vi "Dresden New Recipe(in).vi"() -> (0 "OKTO":bool, 1 "Data":string[][](array[string]))   [LabVIEW 2009]
uses:
  kernel32.dll
panel:
  out "Calculated_total_length_cmb":dbl
  out "Calculated_total_length_rf":dbl
  in  "Single_RF_power_power_tab":enum32{"Page 1", "Page 2"}(tab)
  in  "R Single RF  Step1 Coating Power":dbl caption="Watt"
  in  "R Single RF Step1 Coating Power Active":bool
  in  "R Single RF Step2 Coating Power":dbl caption="Watt"
  in  "R Single RF Step2 Coating Power Active":bool
  in  "R Single RF Step3 Coating Power":dbl caption="Watt"
  in  "R Single RF Step3 Coating Power Active":bool
  in  "R Single RF Step4 Coating Power":dbl caption="Watt"
  in  "R Single RF Step4 Coating Power Active":bool
  in  "R Single RF Step5 Coating Power":dbl caption="Watt"
  in  "R Single RF Step5 Coating Power Active":bool
  in  "R Single RF Interval length":dbl
  in  "R Single RF Interval length2":dbl
  in  "R Single RF Interval length3":dbl
  in  "R Single RF Interval length4":dbl
  in  "R Single RF Interval length5":dbl
  in  "R Single RF Step6 Coating Power":dbl caption="Watt"
  in  "R Single RF Step6 Coating Power Active":bool
  in  "R Single RF Interval length6":dbl
  in  "R Single RF Step7 Coating Power":dbl caption="Watt"
  in  "R Single RF Step7 Coating Power Active":bool
  in  "R Single RF Interval length7":dbl
  in  "R Single RF Step8 Coating Power":dbl caption="Watt"
  in  "R Single RF Step8 Coating Power Active":bool
  in  "R Single RF Interval length8":dbl
  in  "R Single RF Step9 Coating Power":dbl caption="Watt"
  in  "R Single RF Step9 Coating Power Active":bool
  in  "R Single RF Interval length9":dbl
  in  "R Single RF Step10 Coating Power":dbl caption="Watt"
  in  "R Single RF Step10 Coating Power Active":bool
  in  "R Single RF Interval length10":dbl
  in  "Single_DC_power_power_tab":enum32{"Page 1", "Page 2"}(tab)
  in  "R Single DC Interval length1":dbl
  in  "R Single DC Step1 Coating Power Active":bool
  in  "R Single DC Step1 Coating Power":dbl caption="Watt"
  in  "R Single DC Interval length2":dbl
  in  "R Single DC Step2 Coating Power Active":bool
  in  "R Single DC Step2 Coating Power":dbl caption="Watt"
  in  "R Single DC Step3 Coating Power Active":bool
  in  "R Single DC Step3 Coating Power":dbl caption="Watt"
  in  "R Single DC Interval length3":dbl
  in  "R Single DC Step4 Coating Power Active":bool
  in  "R Single DC Step4 Coating Power":dbl caption="Watt"
  in  "R Single DC Interval length4":dbl
  in  "R Single DC Step5 Coating Power Active":bool
  in  "R Single DC Step5 Coating Power":dbl caption="Watt"
  in  "R Single DC Interval length5":dbl
  in  "R Single DC Step6 Coating Power Active":bool
  in  "R Single DC Step6 Coating Power":dbl caption="Watt"
  in  "R Single DC Interval length6":dbl
  in  "R Single DC Step7 Coating Power Active":bool
  in  "R Single DC Step7 Coating Power":dbl caption="Watt"
  in  "R Single DC Interval length7":dbl
  in  "R Single DC Step8 Coating Power Active":bool
  in  "R Single DC Step8 Coating Power":dbl caption="Watt"
  in  "R Single DC Interval length8":dbl
  in  "R Single DC Step9 Coating Power Active":bool
  in  "R Single DC Step9 Coating Power":dbl caption="Watt"
  in  "R Single DC Interval length9":dbl
  in  "R Single DC Step10 Coating Power Active":bool
  in  "R Single DC Step10 Coating Power":dbl caption="Watt"
  in  "R Single DC Interval length10":dbl
  in  "Multilayer_power_tab":enum32{"Page 1", "Page 2"}(tab)
  in  "R Cmb Interval length 1":dbl
  in  "R Cmb Ch3 Step1 Coating Power":dbl caption="Watt"
  in  "R Cmb Step1 Coating Power Active":bool
  in  "R Cmb Ch2 Step1 Coating Power":dbl caption="Watt"
  in  "R Cmb Interval length 2":dbl
  in  "R Cmb Ch3 Step2 Coating Power":dbl caption="Watt"
  in  "R Cmb Step2 Coating Power Active":bool
  in  "R Cmb Ch2 Step2 Coating Power":dbl caption="Watt"
  in  "R Cmb Interval length 3":dbl
  in  "R Cmb Ch3 Step3 Coating Power":dbl caption="Watt"
  in  "R Cmb Step3 Coating Power Active":bool
  in  "R Cmb Ch2 Step3 Coating Power":dbl caption="Watt"
  in  "R Cmb Interval length 4":dbl
  in  "R Cmb Ch3 Step4 Coating Power":dbl caption="Watt"
  in  "R Cmb Step4 Coating Power Active":bool
  in  "R Cmb Ch2 Step4 Coating Power":dbl caption="Watt"
  in  "R Cmb Interval length 5":dbl
  in  "R Cmb Ch3 Step5 Coating Power":dbl caption="Watt"
  in  "R Cmb Step5 Coating Power Active":bool
  in  "R Cmb Ch2 Step5 Coating Power":dbl caption="Watt"
  in  "R Cmb Interval length 6":dbl
  in  "R Cmb Ch3 Step6 Coating Power":dbl caption="Watt"
  in  "R Cmb Step6 Coating Power Active":bool
  in  "R Cmb Ch2 Step6 Coating Power":dbl caption="Watt"
  in  "R Cmb Interval length 7":dbl
  in  "R Cmb Ch3 Step7 Coating Power":dbl caption="Watt"
  in  "R Cmb Step7 Coating Power Active":bool
  in  "R Cmb Ch2 Step7 Coating Power":dbl caption="Watt"
  in  "R Cmb Interval length 8":dbl
  in  "R Cmb Ch3 Step8 Coating Power":dbl caption="Watt"
  in  "R Cmb Step8 Coating Power Active":bool
  in  "R Cmb Ch2 Step8 Coating Power":dbl caption="Watt"
  in  "R Cmb Interval length 9":dbl
  in  "R Cmb Ch3 Step9 Coating Power":dbl caption="Watt"
  in  "R Cmb Step9 Coating Power Active":bool
  in  "R Cmb Ch2 Step9 Coating Power":dbl caption="Watt"
  in  "R Cmb Interval length 10":dbl
  in  "R Cmb Ch3 Step10 Coating Power":dbl caption="Watt"
  in  "R Cmb Step10 Coating Power Active":bool
  in  "R Cmb Ch2 Step10 Coating Power":dbl caption="Watt"
  out "error out":errorcluster
  out "Calculated_total_length_dc":dbl
  in  "Diameter":dbl
  out "Lap":dbl
  in  "R General_tab":enum32{"Page 1", "Page 2"}(tab)
  in  "Cancel":bool
  in  "Thickness_Monitor_Active":bool
  in  "Recipe_selection tab":T1(tab)
  in  "R_Simple_Coating Type Selection":T2(radio)
  in  "R_Single_Coating Type Selection_tab":T3(tab)
  in  "R_Single Microwave Time":dbl caption="sec"
  in  "R_Single Microwave Power":dbl=600.0 caption="Watt"
  in  "R Single Pass Number":dbl
  in  "R_Single DC_Material ok":bool
  in  "R_Single DC_Mat_sel":u64(ring) items=["Other", "Ag", "AgBr", "AgCl", "Al", "Al2O3", "As", "Au", "B", "Ba", "Be", "Bi", "Bi2O3", "C (Diamond)", "C (Graphite)", "Ca", "CaF", "Cd", "CdS", "CdSe", "CdTe", "CeF3", "CeO", "Cr", "Cr2O3", "Co", "Cu", "Cu2S (A)", "Cu2S (B)", "CuS", "Dy", "Er", "Fe", "Ga", "GaAs", "Gd", "Ge", "Hf", "HfO2", "Hg", "Ho", "In", "InSb", "In2O3", "Ir", "KCl", "La", "LaF3", "LaO3", "Li", "LiF", "Mg", "MgF2", "MgO", "Mn", "MnS", "Mo", "Na", "NaCl", "NdF3", "Nd2O3", "Ni", "Nb", "Nb2O5", "Pb", "PbS", "Pd", "Pt", "Re", "Rh", "Rb", "S", "Sb", "Sc", "Se", "Si", "SiO", "SiO2", "Sm", "Sn", "Ta", "Ta2O5", "Te", "Tb", "ThF4", "Ti", "TiO2", "TiO", "Tl", "U", "V", "W", "WC", "Y", "Y2O3", "Yb", "Zn", "ZnO", "ZnSe", "ZnS", "Zr", "ZrO2", "Si3N4", "ITO", "PbI2"]
  in  "R Single DC Target material":string
  in  "R_DC_Chamber_selection":enum32{"Chamber II", "Chamber III"}(radio)
  in  "Power_singledc_list_open":bool
  in  "R_Single RF Material ok":bool
  in  "R_Single RF_Mat_sel":u64(ring) items=["Other", "Ag", "AgBr", "AgCl", "Al", "Al2O3", "As", "Au", "B", "Ba", "Be", "Bi", "Bi2O3", "C (Diamond)", "C (Graphite)", "Ca", "CaF", "Cd", "CdS", "CdSe", "CdTe", "CeF3", "CeO", "Cr", "Cr2O3", "Co", "Cu", "Cu2S (A)", "Cu2S (B)", "CuS", "Dy", "Er", "Fe", "Ga", "GaAs", "Gd", "Ge", "Hf", "HfO2", "Hg", "Ho", "In", "InSb", "In2O3", "Ir", "KCl", "La", "LaF3", "LaO3", "Li", "LiF", "Mg", "MgF2", "MgO", "Mn", "MnS", "Mo", "Na", "NaCl", "NdF3", "Nd2O3", "Ni", "Nb", "Nb2O5", "Pb", "PbS", "Pd", "Pt", "Re", "Rh", "Rb", "S", "Sb", "Sc", "Se", "Si", "SiO", "SiO2", "Sm", "Sn", "Ta", "Ta2O5", "Te", "Tb", "ThF4", "Ti", "TiO2", "TiO", "Tl", "U", "V", "W", "WC", "Y", "Y2O3", "Yb", "Zn", "ZnO", "ZnSe", "ZnS", "Zr", "ZrO2", "Si3N4", "ITO", "PbI2"]
  in  "R Single RF Target material":string
  in  "R Single RF Ramp down":bool
  in  "R Single RF Ramp down Time":dbl caption="sec"
  in  "R Single RF Ramp up Time":dbl caption="sec"
  in  "R Single RF Ramp up":bool
  in  "Power_single_rf_list_open":bool
  in  "Power_list_open_multi":bool
  in  "R Cmb Ch3 Material ok":bool
  in  "R Cmb Ch3 Mat_sel":u64(ring) items=["Other", "Ag", "AgBr", "AgCl", "Al", "Al2O3", "As", "Au", "B", "Ba", "Be", "Bi", "Bi2O3", "C (Diamond)", "C (Graphite)", "Ca", "CaF", "Cd", "CdS", "CdSe", "CdTe", "CeF3", "CeO", "Cr", "Cr2O3", "Co", "Cu", "Cu2S (A)", "Cu2S (B)", "CuS", "Dy", "Er", "Fe", "Ga", "GaAs", "Gd", "Ge", "Hf", "HfO2", "Hg", "Ho", "In", "InSb", "In2O3", "Ir", "KCl", "La", "LaF3", "LaO3", "Li", "LiF", "Mg", "MgF2", "MgO", "Mn", "MnS", "Mo", "Na", "NaCl", "NdF3", "Nd2O3", "Ni", "Nb", "Nb2O5", "Pb", "PbS", "Pd", "Pt", "Re", "Rh", "Rb", "S", "Sb", "Sc", "Se", "Si", "SiO", "SiO2", "Sm", "Sn", "Ta", "Ta2O5", "Te", "Tb", "ThF4", "Ti", "TiO2", "TiO", "Tl", "U", "V", "W", "WC", "Y", "Y2O3", "Yb", "Zn", "ZnO", "ZnSe", "ZnS", "Zr", "ZrO2", "Si3N4", "ITO", "PbI2"]
  in  "R Cmb Ch3 Target material":string
  in  "R_Cmb Ch2_Material ok":bool
  in  "R_Cmb Ch2_Mat_sel":u64(ring) items=["Other", "Ag", "AgBr", "AgCl", "Al", "Al2O3", "As", "Au", "B", "Ba", "Be", "Bi", "Bi2O3", "C (Diamond)", "C (Graphite)", "Ca", "CaF", "Cd", "CdS", "CdSe", "CdTe", "CeF3", "CeO", "Cr", "Cr2O3", "Co", "Cu", "Cu2S (A)", "Cu2S (B)", "CuS", "Dy", "Er", "Fe", "Ga", "GaAs", "Gd", "Ge", "Hf", "HfO2", "Hg", "Ho", "In", "InSb", "In2O3", "Ir", "KCl", "La", "LaF3", "LaO3", "Li", "LiF", "Mg", "MgF2", "MgO", "Mn", "MnS", "Mo", "Na", "NaCl", "NdF3", "Nd2O3", "Ni", "Nb", "Nb2O5", "Pb", "PbS", "Pd", "Pt", "Re", "Rh", "Rb", "S", "Sb", "Sc", "Se", "Si", "SiO", "SiO2", "Sm", "Sn", "Ta", "Ta2O5", "Te", "Tb", "ThF4", "Ti", "TiO2", "TiO", "Tl", "U", "V", "W", "WC", "Y", "Y2O3", "Yb", "Zn", "ZnO", "ZnSe", "ZnS", "Zr", "ZrO2", "Si3N4", "ITO", "PbI2"]
  in  "R Cmb Ch2 Target material":string
  in  "R Cmb Number of cycle":dbl
  in  "R_First_stop_selection":enum32{"Chamber II", "Chamber III"}(radio)=enum."Chamber III"
  in  "R_Cmb_Ch2_Web_speed":dbl
  in  "R_Cmb_Ch3_Web_speed":dbl
  in  "Substrate Material":string
  in  "Recipe Name":string
  in  "R_Recipe_type_selection":enum32{"Single Recipe", "Combination Sputter"}(radio)
  in  "R_Web_selection":enum32{"Web", "Other"}(radio)=enum."Other"
  in  "Web_selection_tab":T4(tab)
  in  "R Web thickness":dbl
  in  "R Maximum diameter":dbl format="%.1f"
  in  "R Minimum diameter":dbl=93.0 format="%.1f"
  in  "R Web speed(cm/min)":dbl
  in  "R Tension Value":dbl=7.0
  out "R  Total length":dbl caption="cm" format="%.1f"
  in  "Calculate":bool
  in  "R_Thickness Selection":enum32{"Thickness", "Time"}(radio)
  in  "R_Target Thickness Value":dbl format="%.2f"
  in  "R_Duration":dbl caption="%"
  in  "R Argon Flow sccm":dbl caption="sccm"
  in  "R Z_factor":dbl format="%_3f"
  in  "R Material_density":dbl caption="g/cm3" format="%_3f"
  in  "OK":bool caption="OK2"
  in  "R Toooling_factor":dbl caption="%"
  in  "R Set Pressure mtorr":dbl=0.004 caption="mbar" format="%.1e"
  in  "Tab Control":enum32{"Page 1", "Page 2"}(tab)
  out "Process_flow":string
  in  "Tab Control 2":enum32{"Page 1", "Page 2"}(tab)
  out "Process_flow 2":string
  # "dc max:3000"
  # "rf max:2000"
  # "Steps List"
  # "Power(Watt)"
  # "Interval Length(cm)"
  # "Step 1    :"
  # "cm"
  # "Step 2    :"
  # "cm"
  # "Step 3    :"
  # "cm"
  # "Step 4    :"
  # "cm"
  # "Step 5    :"
  # "cm"
  # "Step 6    :"
  # "cm"
  # "Step 7    :"
  # "cm"
  # "Step 8    :"
  # "cm"
  # "Step 9    :"
  # "cm"
  # "Step 10  :"
  # "cm"
  # "Steps List"
  # "Power(Watt)"
  # "Interval Length(cm)"
  # "Step 1            :"
  # "cm"
  # "Step 2            :"
  # "cm"
  # "Step 3            :"
  # "cm"
  # "Step 4            :"
  # "cm"
  # "Step 5            :"
  # "cm"
  # "Step 6            :"
  # "cm"
  # "cm"
  # "Step 7            :"
  # "cm"
  # "Step 8            :"
  # "cm"
  # "Step 9            :"
  # "cm"
  # "Step 10          :"
  # "Steps List"
  # "CH2-Power(Watt)"
  # "CH3-Power(Watt)"
  # "Interval Length(cm)"
  # "Step 1:"
  # "cm"
  # "Step 2:"
  # "cm"
  # "Step 3:"
  # "cm"
  # "Step 4:"
  # "cm"
  # "Step 5:"
  # "cm"
  # "Step 6:"
  # "cm"
  # "cm"
  # "Step 7:"
  # "cm"
  # "Step 8:"
  # "cm"
  # "Step 9:"
  # "cm"
  # "Step 10:"
  # "Recipe  Selection"
  # "Web  Selection"
  # "Pressure Control Parameters"
  # "Thickness Monitor Parameters"
  # "Material Density       :"
  # "Argon Flow         :"
  # "Z factor                    :"
  # "Set Pressure        :"
  # "Tooling Factor         :"
  # "Single Process Selection"
  # "Power Value     :"
  # "Watt"
  # "Duration           :"
  # "sec"
  # "Pass Number    :"
  # "DCPS Parameters"
  # "Target material          :"
  # "RFPS Parameters"
  # "Target material          :"
  # "Ramp Up Time           :"
  # "Ramp Down Time      :"
  # "DCPS Parameters"
  # "Chamber II"
  # "Chamber III"
  # "Target material         :"
  # "Target material          :"
  # "Web Speed                :"
  # "cm/sec"
  # "Web Speed               :"
  # "cm/sec"
  # "Number of cycle:"
  # "First Stop :"
  # "Roll  Parameters"
  # "Minimum Diameter     :"
  # "mm"
  # "Web Speed              :"
  # "cm / min"
  # "Tension Value         :"
  # "Maximum Diameter     :"
  # "mm"
  # "N"
  # "Web Thickness            :"
  # "µm"
  # "Total Length           :"
  # "Other Parameters"
  # "Thickness Selection         :"
  # "Target Thickness Value   :"
  # "kA"
  # "min"
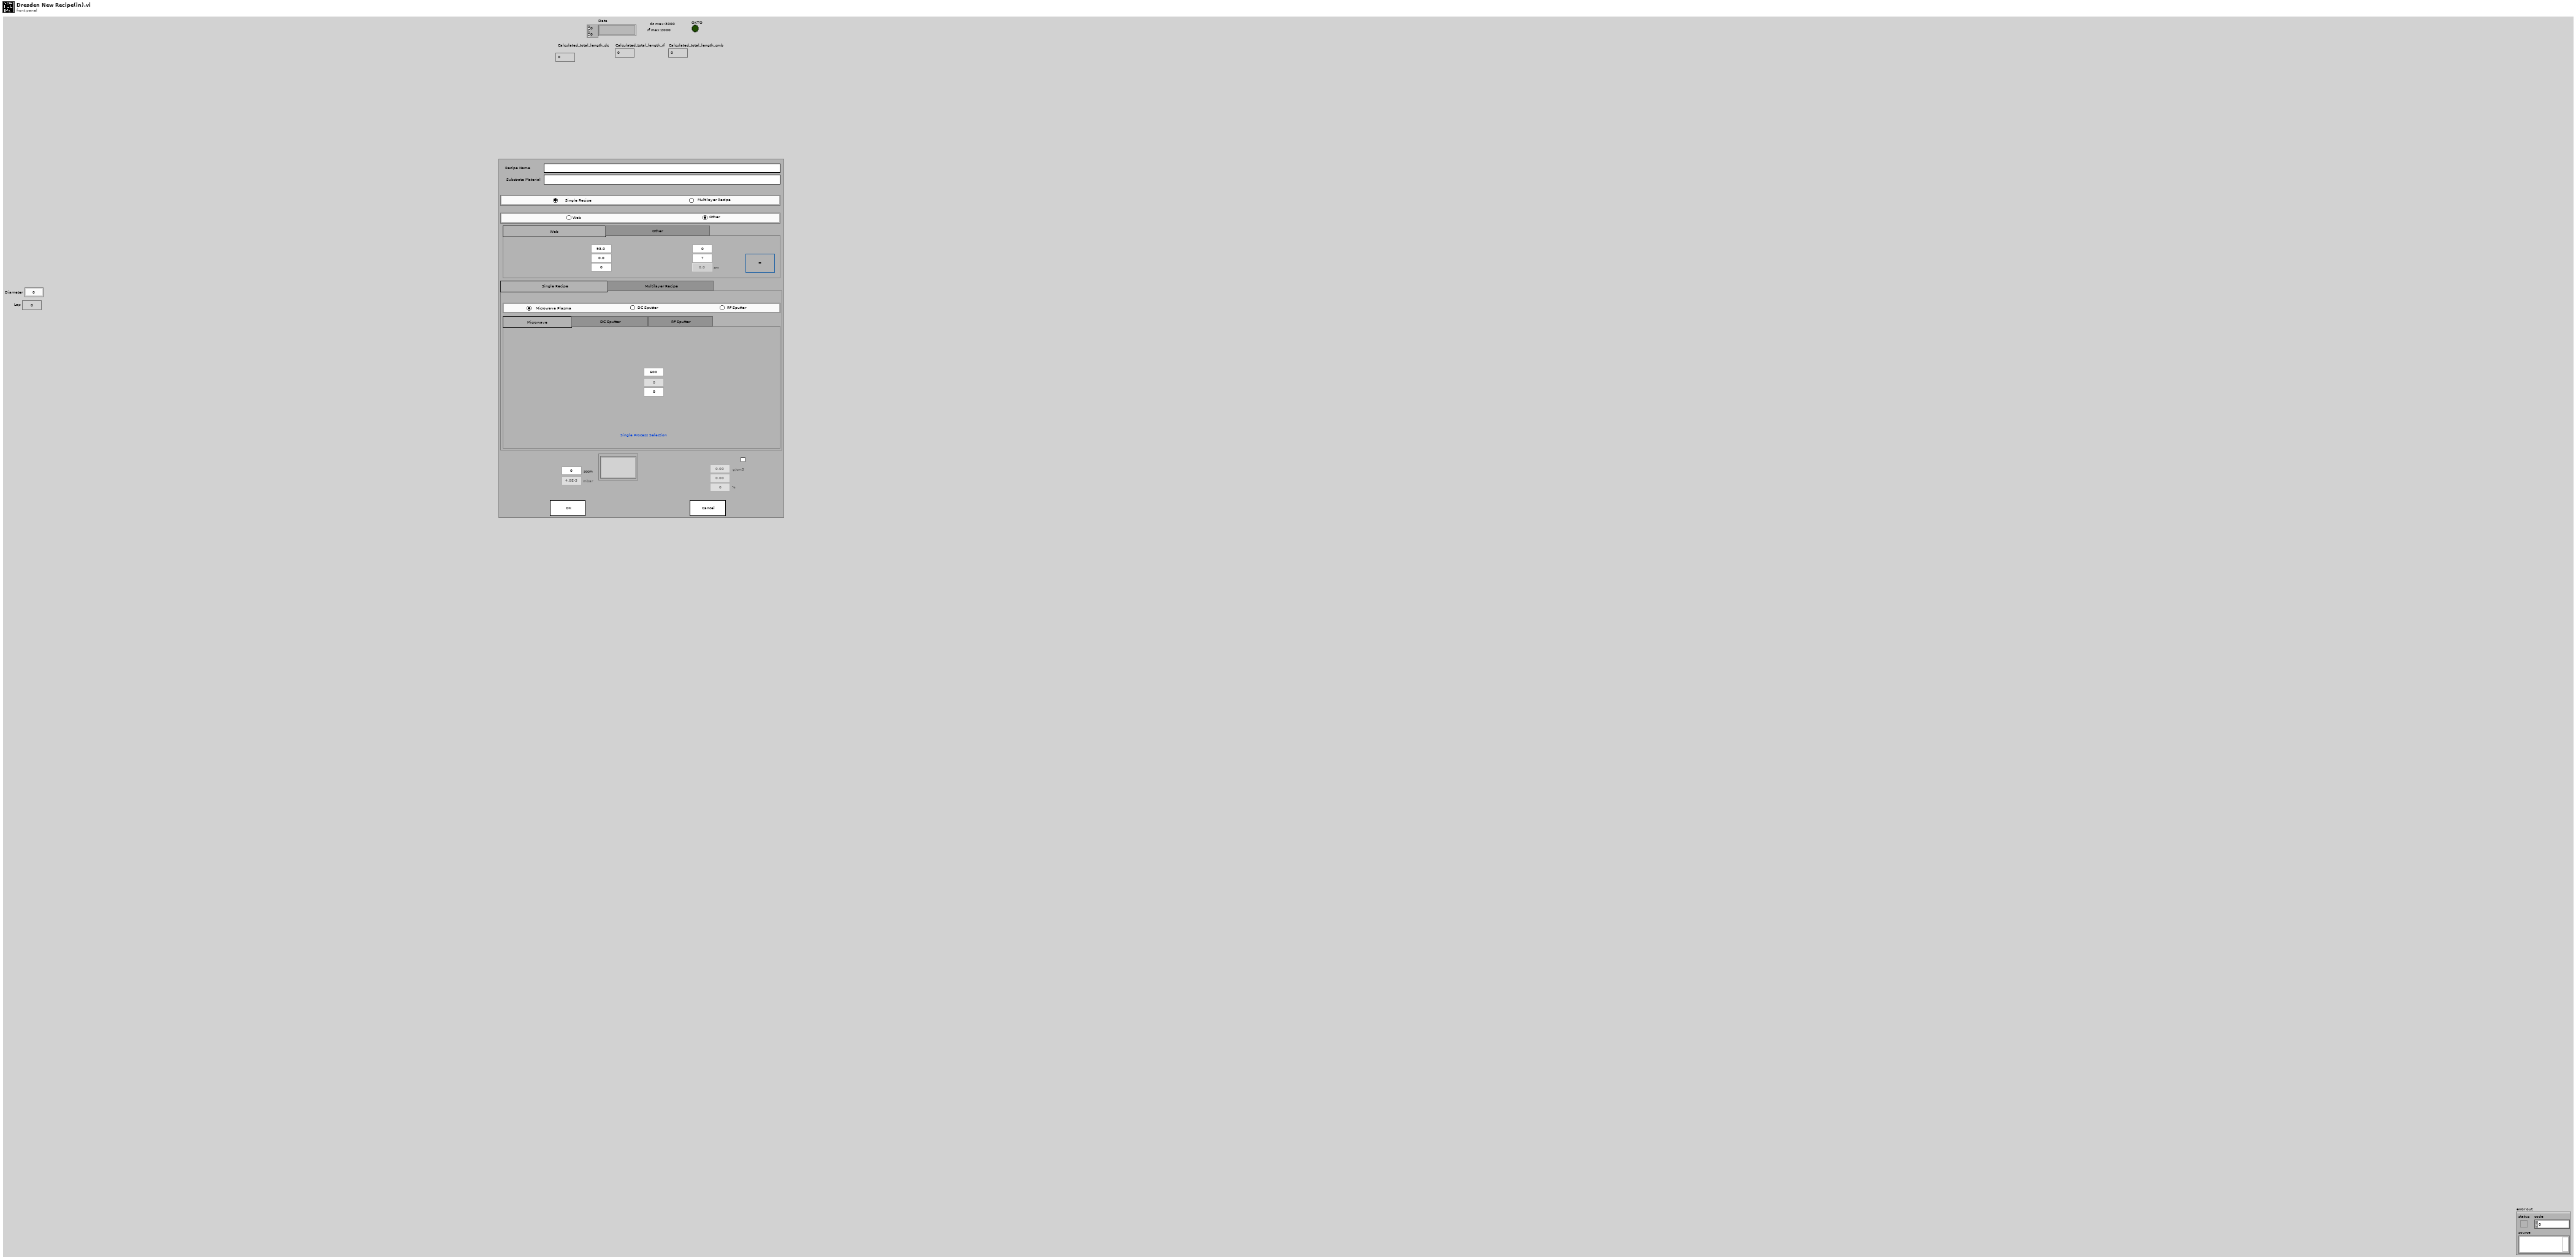
[diagram p1: front panel]
types:
  T1 = enum32{"Single Recipe                                                                         ", "Multilayer Recipe                                                                  "}
  T2 = enum32{"Microwave Plasma", "DC Sputter", "RF Sputter"}
  T3 = enum32{"Microwave                                          ", "DC Sputter                                                 ", "RF Sputter                                       "}
  T4 = enum32{"Web                                                                                    ", "Other                                                                                    "}
  T5 = enum8{"Enabled", "Disabled", "Disabled and Grayed Out"}
  T6 = enum16{"open", "replace", "create", "open or create", "replace or create", "replace or create with confirmation"}
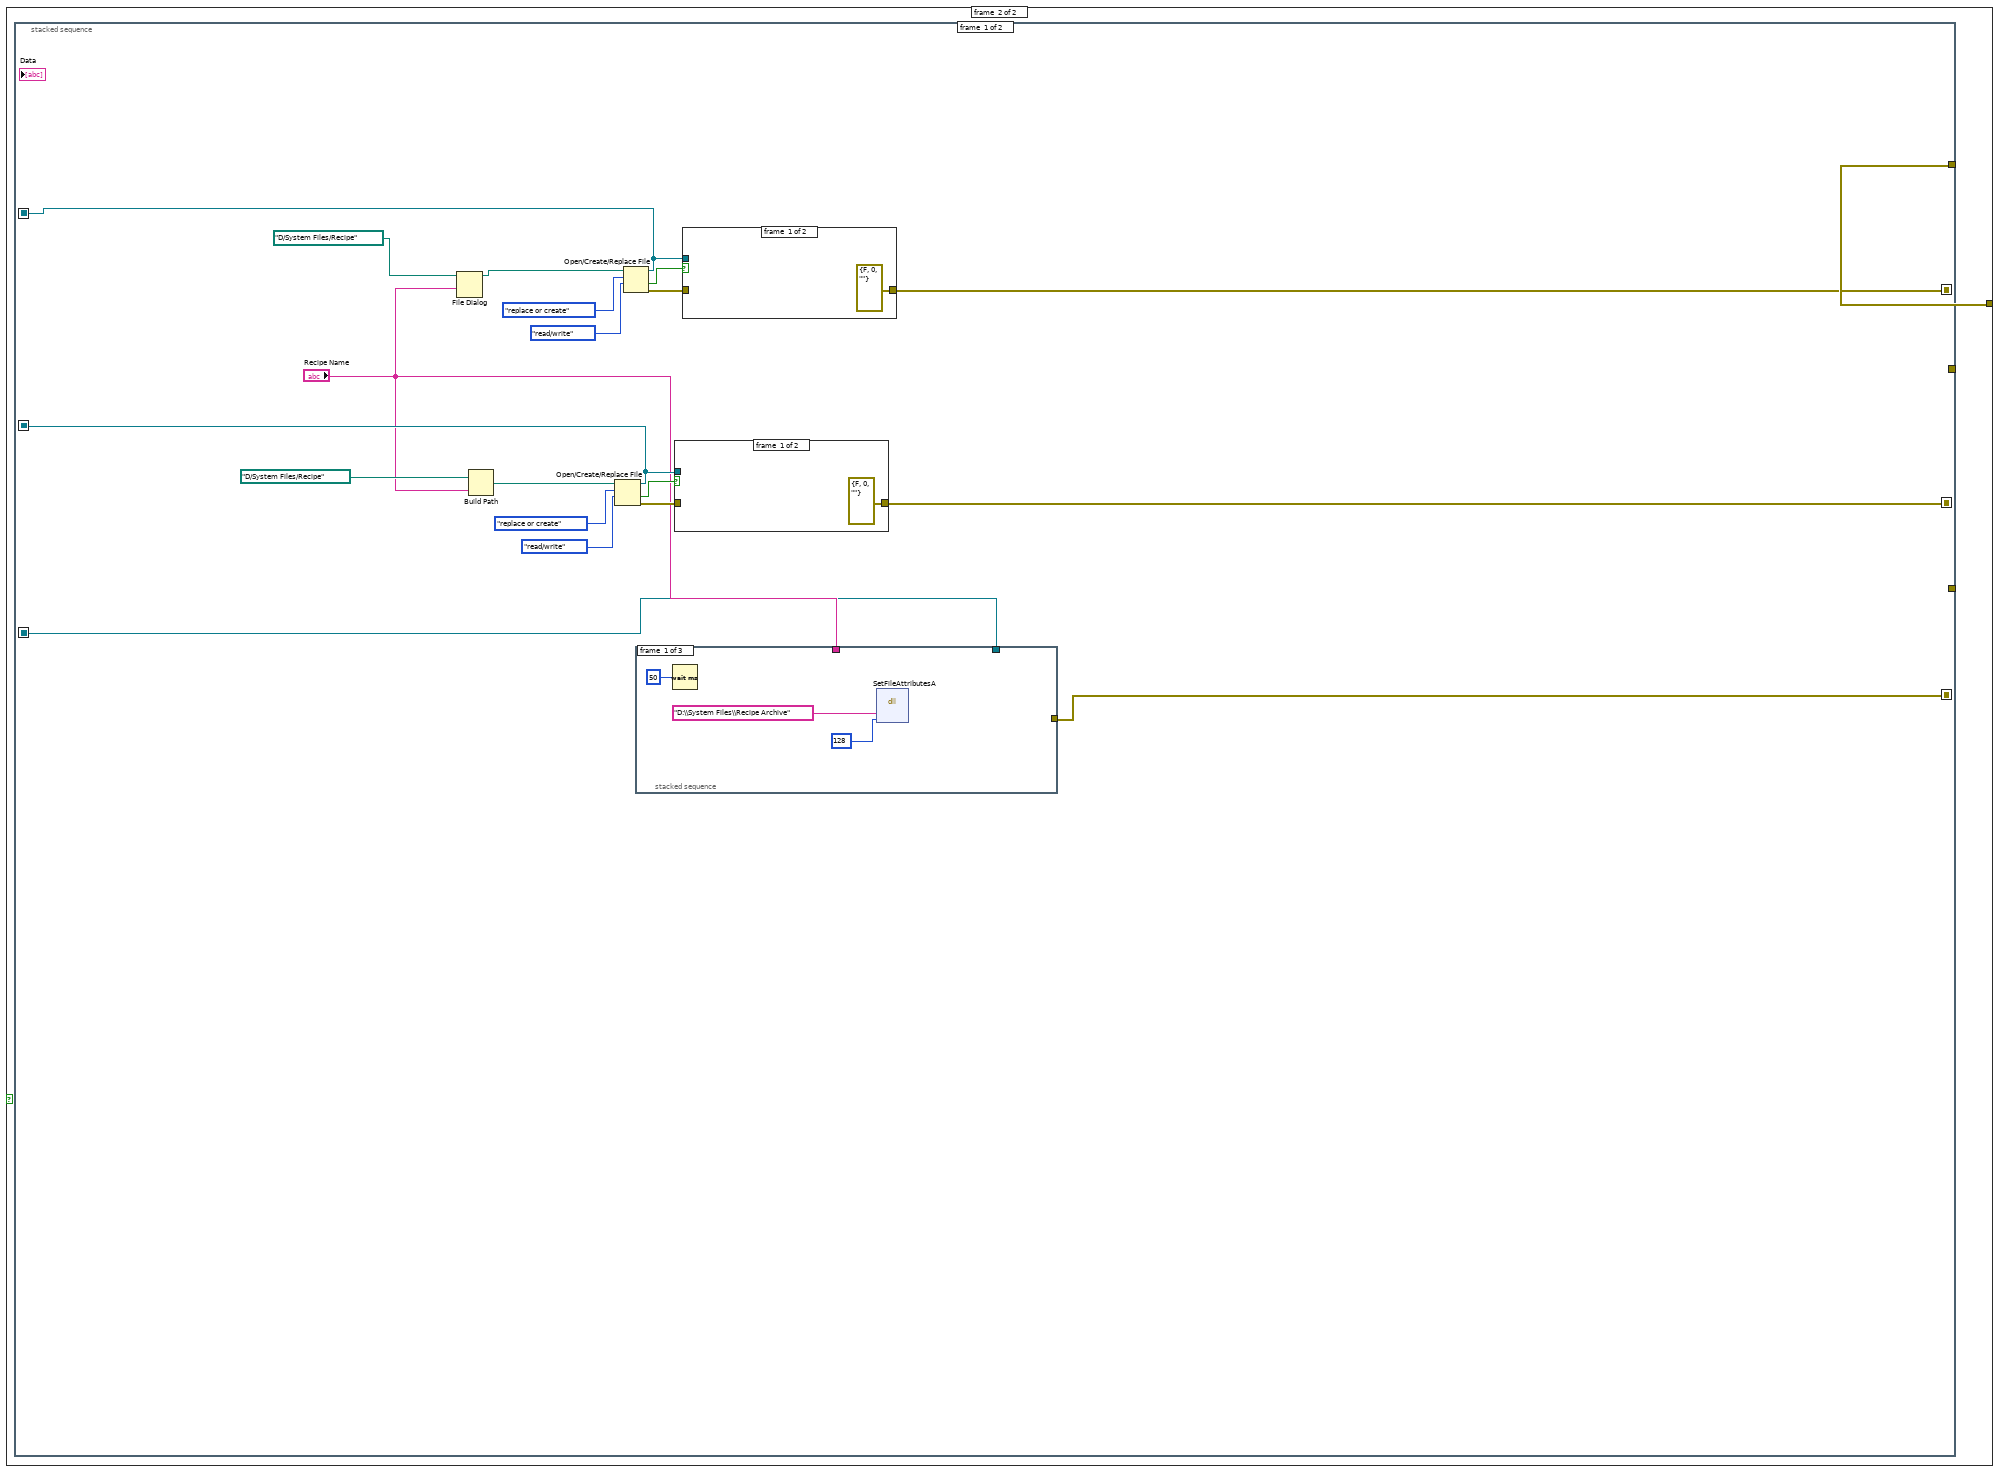
[diagram p2: hidden frame]
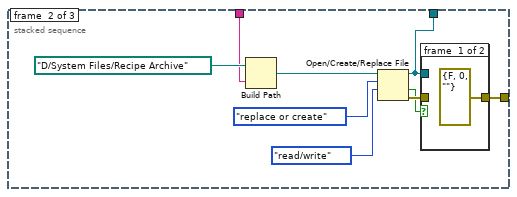
[diagram p3: hidden frame]
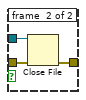
[diagram p4: hidden frame]
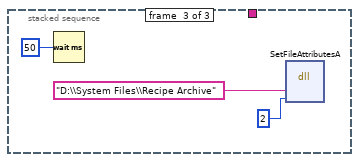
[diagram p5: hidden frame]
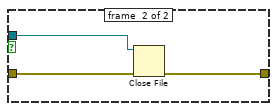
[diagram p6: hidden frame]
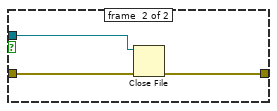
[diagram p7: hidden frame]
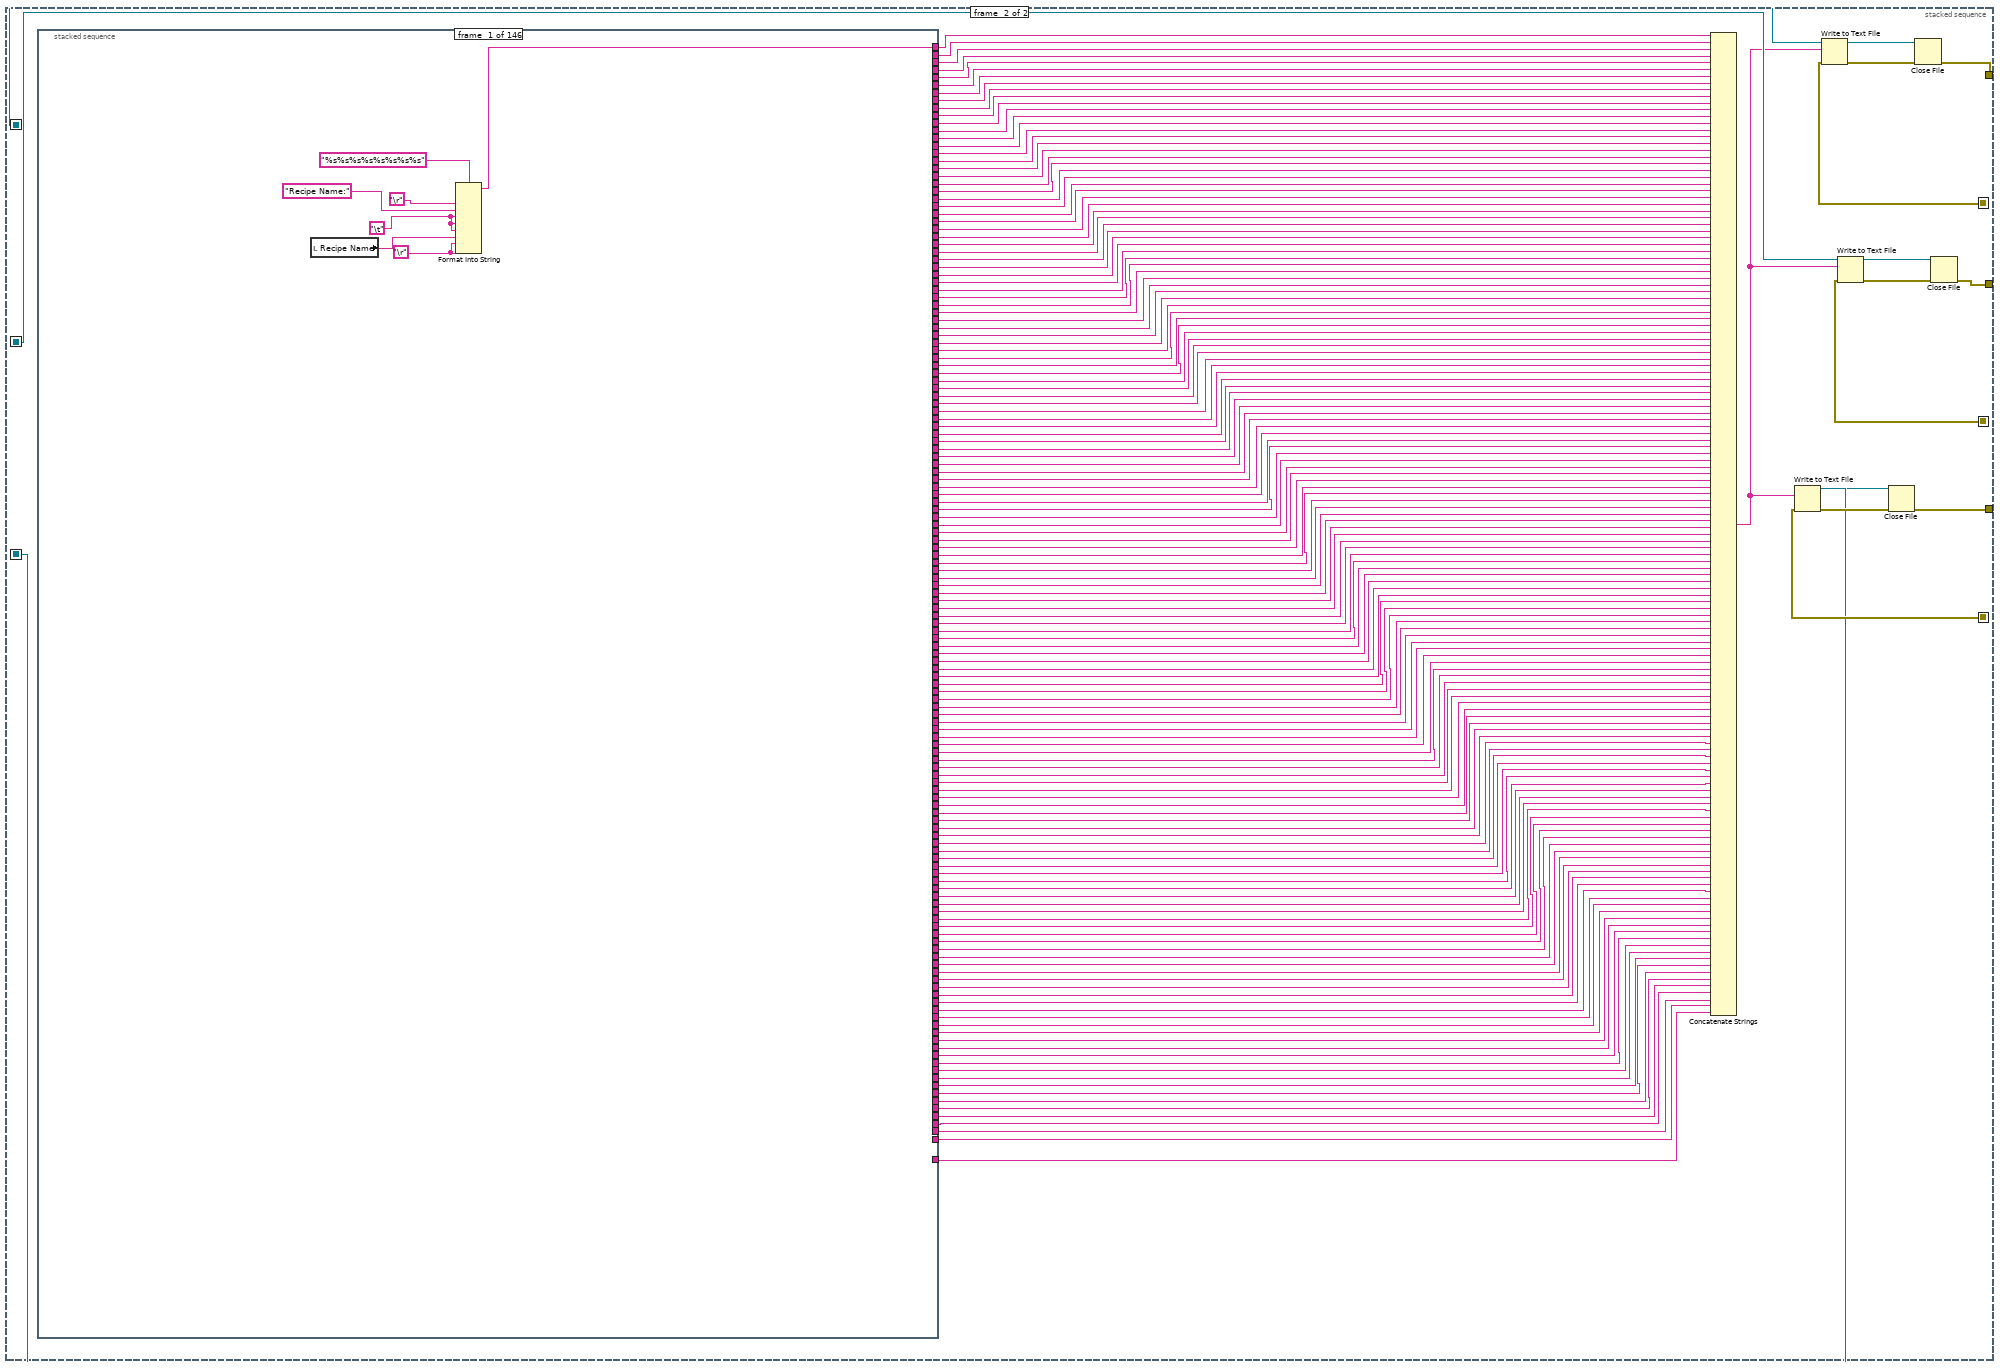
[diagram p8: hidden frame]
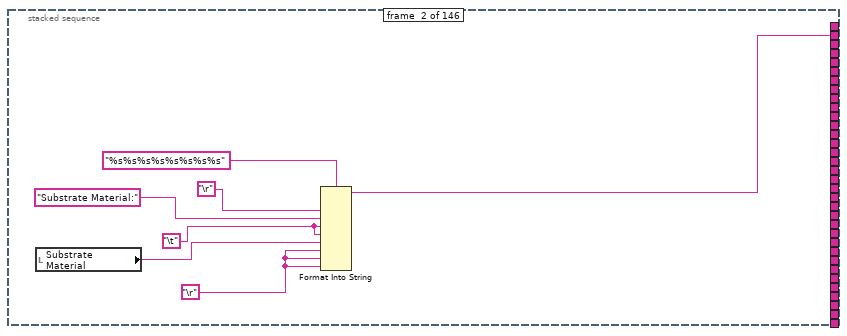
[diagram p9: hidden frame]
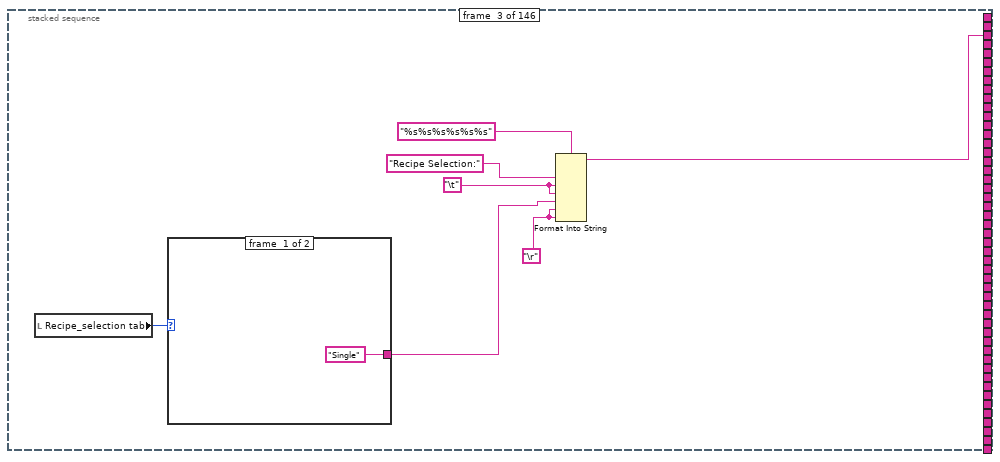
[diagram p10: hidden frame]
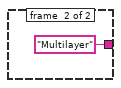
[diagram p11: hidden frame]
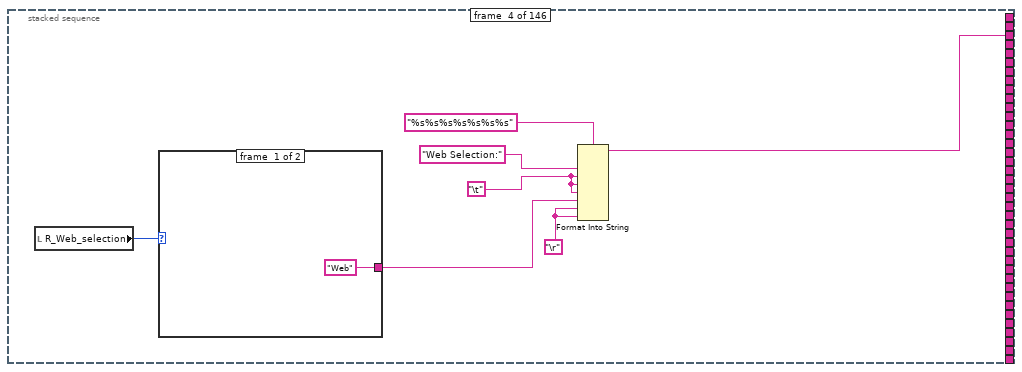
[diagram p12: hidden frame]
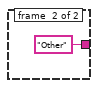
[diagram p13: hidden frame]
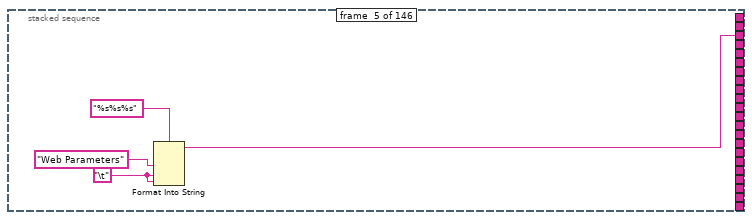
[diagram p14: hidden frame]
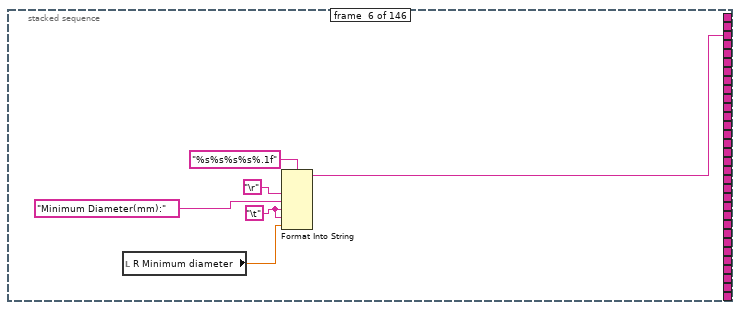
[diagram p15: hidden frame]
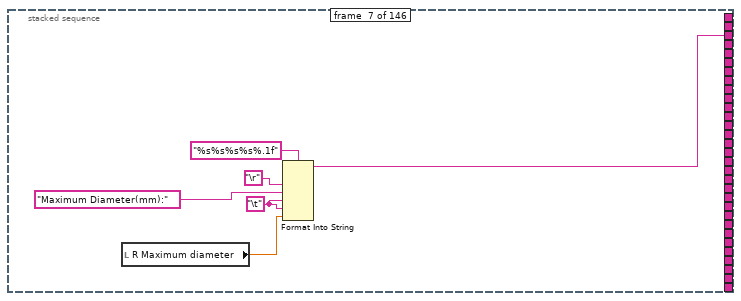
[diagram p16: hidden frame]
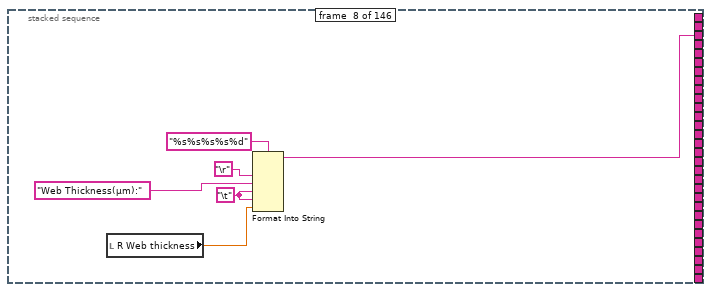
[diagram p17: hidden frame]
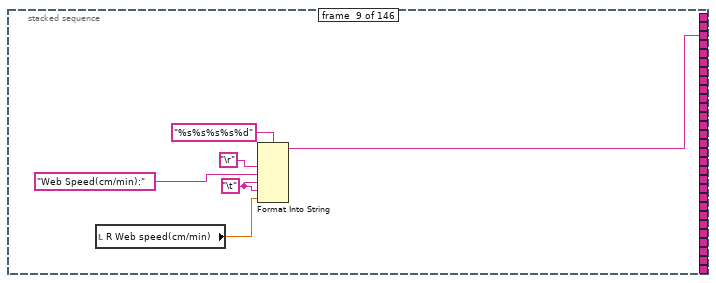
[diagram p18: hidden frame]
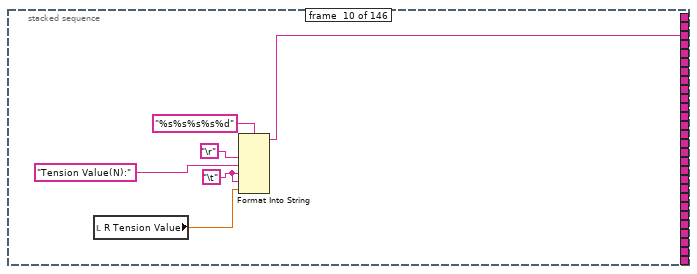
[diagram p19: hidden frame]
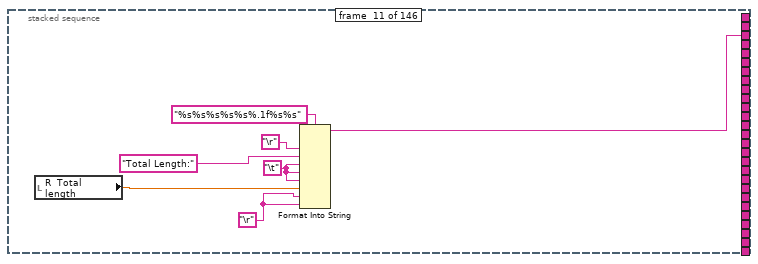
[diagram p20: hidden frame]
diagram:
  n1 = while {
    tunnel: [w36] -> w2
    stop <- w36 stop-if-true
    n2 = local read "R Single DC Step1 Coating Power Active"() -> (w35:bool)
    n3 = local read "R Single RF Step4 Coating Power Active"() -> (w23:bool)
    n4 = local read "R Single DC Step4 Coating Power Active"() -> (w32:bool)
    n5 = local read "R Single DC Step2 Coating Power Active"() -> (w34:bool)
    n6 = local read "R Single RF Step3 Coating Power Active"() -> (w24:bool)
    n7 = local read "R Single RF Step1 Coating Power Active"() -> (w26:bool)
    n8 = local read "R Single DC Step3 Coating Power Active"() -> (w33:bool)
    n9 = local read "R Single RF Step5 Coating Power Active"() -> (w22:bool)
    n10 = local read "R Single RF Step9 Coating Power Active"() -> (w21:bool)
    n11 = local read "R_Recipe_type_selection"() -> (w8:enum32{"Single Recipe", "Combination Sputter"})
    n12 = local read "R Single RF Step2 Coating Power Active"() -> (w25:bool)
    n13 = case shown="\"Combination Sputter\"" w8 {
      frame #0 {
        n14 = local read "Web_selection_tab"() -> (w204:T4)
        n15 = Equal?(x=w204, y=0) -> (x = y?=w203:bool)
        n16 = case shown="True" w203 {
          frame #0 {
          }
          frame #1 {
            w206 = T5."Enabled" ("Disabled")
            n17 = property on="R Minimum diameter" class="DigNum (strict)"("DisabledEnum"=w206) -> ()  [unwired: 2 in, 2 out]
            n18 = property on="R Maximum diameter" class="DigNum (strict)"("DisabledEnum"=w206) -> ()  [unwired: 2 in, 2 out]
            n19 = property on="R Web thickness" class="DigNum (strict)"("DisabledEnum"=w206) -> ()  [unwired: 2 in, 2 out]
            n20 = property on="R Web speed(cm/min)" class="DigNum (strict)"("DisabledEnum"=w206) -> ()  [unwired: 2 in, 2 out]
            n21 = property on="R Tension Value" class="DigNum (strict)"("DisabledEnum"=w206) -> ()  [unwired: 2 in, 2 out]
            n22 = property on="R_Single Microwave Time" class="DigNum (strict)"("DisabledEnum"=T5."Disabled and Grayed Out" ("Disabled")) -> ()  [unwired: 2 in, 2 out]
          }
        }
      }
      frame #1 {
        n23 = local read "R_Web_selection"() -> (w209:enum32{"Web", "Other"})
        n24 = Equal?(x=w209, y=0) -> (x = y?=w210:bool)
        n25 = case shown="True" w210 {
          frame #0 {
          }
          frame #1 {
            w212 = T5."Enabled" ("Disabled")
            n26 = local write "R Web speed(cm/min)"(0.0 ("R Web speed(cm/min)")) -> ()
            n27 = property on="R Tension Value" class="DigNum (strict)"("DisabledEnum"=w212) -> ()  [unwired: 2 in, 2 out]
            n28 = property on="R Minimum diameter" class="DigNum (strict)"("DisabledEnum"=w212) -> ()  [unwired: 2 in, 2 out]
            n29 = property on="R Maximum diameter" class="DigNum (strict)"("DisabledEnum"=w212) -> ()  [unwired: 2 in, 2 out]
            n30 = property on="R Web thickness" class="DigNum (strict)"("DisabledEnum"=w212) -> ()  [unwired: 2 in, 2 out]
            n31 = property on="R Web speed(cm/min)" class="DigNum (strict)"("DisabledEnum"=T5."Disabled and Grayed Out" ("Disabled")) -> ()  [unwired: 2 in, 2 out]
          }
        }
      }
    }
    n32 = case shown="True" w35 {
      frame #0 {
      }
      frame #1 {
        n33 = local read "R Single DC Step2 Coating Power Active"() -> (w342:bool)
        n34 = case shown="False" w342 {
          frame #0 {
            w343 = 0.0 ("Target Clean Power")
            w344 = T5."Disabled and Grayed Out" ("Disabled")
            n35 = local write "R Single DC Step2 Coating Power"(w343) -> ()
            n36 = local write "R Single DC Interval length2"(w343) -> ()
            n37 = property on="R Single DC Interval length2" class="DigNum (strict)"("DisabledEnum"=w344) -> ()  [unwired: 2 in, 2 out]
            n38 = property on="R Single DC Step2 Coating Power" class="DigNum (strict)"("DisabledEnum"=w344) -> ()  [unwired: 2 in, 2 out]
          }
          frame #1 {
            w345 = T5."Enabled" ("Disabled")
            n39 = property on="R Single DC Step2 Coating Power" class="DigNum (strict)"("DisabledEnum"=w345) -> ()  [unwired: 2 in, 2 out]
            n40 = property on="R Single DC Interval length2" class="DigNum (strict)"("DisabledEnum"=w345) -> ()  [unwired: 2 in, 2 out]
          }
        }
      }
    }
    n41 = local read "R_Recipe_type_selection"() -> (w174:enum32{"Single Recipe", "Combination Sputter"})
    n42 = case shown="False" w23 {
      frame #0 {
        w283 = FALSE ("R Single RF Step3 Coating Power Active")
        n43 = local write "R Single RF Step5 Coating Power Active"(w283) -> ()
        n44 = local write "R Single RF Step6 Coating Power Active"(w283) -> ()
        n45 = local write "R Single RF Step7 Coating Power Active"(w283) -> ()
        n46 = local write "R Single RF Step8 Coating Power Active"(w283) -> ()
        n47 = local write "R Single RF Step9 Coating Power Active"(w283) -> ()
        n48 = local write "R Single RF Step10 Coating Power Active"(w283) -> ()
      }
      frame #1 {
        n49 = local read "R Single RF Step5 Coating Power Active"() -> (w284:bool)
        n50 = case shown="False" w284 {
          frame #0 {
            w286 = T5."Disabled and Grayed Out" ("Disabled")
            w285 = 0.0 ("Target Clean Power")
            n51 = local write "R Single RF Step5 Coating Power"(w285) -> ()
            n52 = local write "R Single RF Interval length5"(w285) -> ()
            n53 = property on="R Single RF Interval length5" class="DigNum (strict)"("DisabledEnum"=w286) -> ()  [unwired: 2 in, 2 out]
            n54 = property on="R Single RF Step5 Coating Power" class="DigNum (strict)"("DisabledEnum"=w286) -> ()  [unwired: 2 in, 2 out]
          }
          frame #1 {
            w287 = T5."Enabled" ("Disabled")
            n55 = property on="R Single RF Step5 Coating Power" class="DigNum (strict)"("DisabledEnum"=w287) -> ()  [unwired: 2 in, 2 out]
            n56 = property on="R Single RF Interval length5" class="DigNum (strict)"("DisabledEnum"=w287) -> ()  [unwired: 2 in, 2 out]
          }
        }
      }
    }
    n57 = local read "R_Recipe_type_selection"() -> (w43:enum32{"Single Recipe", "Combination Sputter"})
    n58 = case shown="False" w24 {
      frame #0 {
        w288 = FALSE ("R Single RF Step3 Coating Power Active")
        n59 = local write "R Single RF Step4 Coating Power Active"(w288) -> ()
        n60 = local write "R Single RF Step5 Coating Power Active"(w288) -> ()
        n61 = local write "R Single RF Step6 Coating Power Active"(w288) -> ()
        n62 = local write "R Single RF Step7 Coating Power Active"(w288) -> ()
        n63 = local write "R Single RF Step8 Coating Power Active"(w288) -> ()
        n64 = local write "R Single RF Step9 Coating Power Active"(w288) -> ()
        n65 = local write "R Single RF Step10 Coating Power Active"(w288) -> ()
      }
      frame #1 {
        n66 = local read "R Single RF Step4 Coating Power Active"() -> (w289:bool)
        n67 = case shown="False" w289 {
          frame #0 {
            w291 = T5."Disabled and Grayed Out" ("Disabled")
            w290 = 0.0 ("Target Clean Power")
            n68 = local write "R Single RF Interval length4"(w290) -> ()
            n69 = local write "R Single RF Step4 Coating Power"(w290) -> ()
            n70 = property on="R Single RF Step4 Coating Power" class="DigNum (strict)"("DisabledEnum"=w291) -> ()  [unwired: 2 in, 2 out]
            n71 = property on="R Single RF Interval length4" class="DigNum (strict)"("DisabledEnum"=w291) -> ()  [unwired: 2 in, 2 out]
          }
          frame #1 {
            w292 = T5."Enabled" ("Disabled")
            n72 = property on="R Single RF Step4 Coating Power" class="DigNum (strict)"("DisabledEnum"=w292) -> ()  [unwired: 2 in, 2 out]
            n73 = property on="R Single RF Interval length4" class="DigNum (strict)"("DisabledEnum"=w292) -> ()  [unwired: 2 in, 2 out]
          }
        }
      }
    }
    n74 = case shown="False" w34 {
      frame #0 {
        w337 = FALSE ("R Single DC Step8 Coating Power Active")
        n75 = local write "R Single DC Step7 Coating Power Active"(w337) -> ()
        n76 = local write "R Single DC Step8 Coating Power Active"(w337) -> ()
        n77 = local write "R Single DC Step9 Coating Power Active"(w337) -> ()
        n78 = local write "R Single DC Step10 Coating Power Active"(w337) -> ()
        n79 = local write "R Single DC Step6 Coating Power Active"(w337) -> ()
        n80 = local write "R Single DC Step3 Coating Power Active"(w337) -> ()
        n81 = local write "R Single DC Step4 Coating Power Active"(w337) -> ()
        n82 = local write "R Single DC Step5 Coating Power Active"(w337) -> ()
      }
      frame #1 {
        n83 = local read "R Single DC Step3 Coating Power Active"() -> (w338:bool)
        n84 = case shown="False" w338 {
          frame #0 {
            w339 = 0.0 ("Target Clean Power")
            w340 = T5."Disabled and Grayed Out" ("Disabled")
            n85 = local write "R Single DC Step3 Coating Power"(w339) -> ()
            n86 = local write "R Single DC Interval length3"(w339) -> ()
            n87 = property on="R Single DC Interval length3" class="DigNum (strict)"("DisabledEnum"=w340) -> ()  [unwired: 2 in, 2 out]
            n88 = property on="R Single DC Step3 Coating Power" class="DigNum (strict)"("DisabledEnum"=w340) -> ()  [unwired: 2 in, 2 out]
          }
          frame #1 {
            w341 = T5."Enabled" ("Disabled")
            n89 = property on="R Single DC Step3 Coating Power" class="DigNum (strict)"("DisabledEnum"=w341) -> ()  [unwired: 2 in, 2 out]
            n90 = property on="R Single DC Interval length3" class="DigNum (strict)"("DisabledEnum"=w341) -> ()  [unwired: 2 in, 2 out]
          }
        }
      }
    }
    n91 = case shown="False" w32 {
      frame #0 {
        w327 = FALSE ("R Single DC Step8 Coating Power Active")
        n92 = local write "R Single DC Step7 Coating Power Active"(w327) -> ()
        n93 = local write "R Single DC Step8 Coating Power Active"(w327) -> ()
        n94 = local write "R Single DC Step9 Coating Power Active"(w327) -> ()
        n95 = local write "R Single DC Step10 Coating Power Active"(w327) -> ()
        n96 = local write "R Single DC Step5 Coating Power Active"(w327) -> ()
        n97 = local write "R Single DC Step6 Coating Power Active"(w327) -> ()
      }
      frame #1 {
        n98 = local read "R Single DC Step5 Coating Power Active"() -> (w328:bool)
        n99 = case shown="False" w328 {
          frame #0 {
            w329 = 0.0 ("Target Clean Power")
            w330 = T5."Disabled and Grayed Out" ("Disabled")
            n100 = local write "R Single DC Step5 Coating Power"(w329) -> ()
            n101 = local write "R Single DC Interval length5"(w329) -> ()
            n102 = property on="R Single DC Step5 Coating Power" class="DigNum (strict)"("DisabledEnum"=w330) -> ()  [unwired: 2 in, 2 out]
            n103 = property on="R Single DC Interval length5" class="DigNum (strict)"("DisabledEnum"=w330) -> ()  [unwired: 2 in, 2 out]
          }
          frame #1 {
            w331 = T5."Enabled" ("Disabled")
            n104 = property on="R Single DC Step5 Coating Power" class="DigNum (strict)"("DisabledEnum"=w331) -> ()  [unwired: 2 in, 2 out]
            n105 = property on="R Single DC Interval length5" class="DigNum (strict)"("DisabledEnum"=w331) -> ()  [unwired: 2 in, 2 out]
          }
        }
      }
    }
    n106 = case shown="False" w33 {
      frame #0 {
        w332 = FALSE ("R Single DC Step8 Coating Power Active")
        n107 = local write "R Single DC Step7 Coating Power Active"(w332) -> ()
        n108 = local write "R Single DC Step8 Coating Power Active"(w332) -> ()
        n109 = local write "R Single DC Step9 Coating Power Active"(w332) -> ()
        n110 = local write "R Single DC Step10 Coating Power Active"(w332) -> ()
        n111 = local write "R Single DC Step6 Coating Power Active"(w332) -> ()
        n112 = local write "R Single DC Step5 Coating Power Active"(w332) -> ()
        n113 = local write "R Single DC Step4 Coating Power Active"(w332) -> ()
      }
      frame #1 {
        n114 = local read "R Single DC Step4 Coating Power Active"() -> (w333:bool)
        n115 = case shown="False" w333 {
          frame #0 {
            w334 = 0.0 ("Target Clean Power")
            w335 = T5."Disabled and Grayed Out" ("Disabled")
            n116 = local write "R Single DC Step4 Coating Power"(w334) -> ()
            n117 = local write "R Single DC Interval length4"(w334) -> ()
            n118 = property on="R Single DC Step4 Coating Power" class="DigNum (strict)"("DisabledEnum"=w335) -> ()  [unwired: 2 in, 2 out]
            n119 = property on="R Single DC Interval length4" class="DigNum (strict)"("DisabledEnum"=w335) -> ()  [unwired: 2 in, 2 out]
          }
          frame #1 {
            w336 = T5."Enabled" ("Disabled")
            n120 = property on="R Single DC Step4 Coating Power" class="DigNum (strict)"("DisabledEnum"=w336) -> ()  [unwired: 2 in, 2 out]
            n121 = property on="R Single DC Interval length4" class="DigNum (strict)"("DisabledEnum"=w336) -> ()  [unwired: 2 in, 2 out]
          }
        }
      }
    }
    n122 = case shown="True" w26 {
      frame #0 {
      }
      frame #1 {
        n123 = local read "R Single RF Step2 Coating Power Active"() -> (w298:bool)
        n124 = case shown="False" w298 {
          frame #0 {
            w300 = T5."Disabled and Grayed Out" ("Disabled")
            w299 = 0.0 ("Target Clean Power")
            n125 = local write "R Single RF Step2 Coating Power"(w299) -> ()
            n126 = local write "R Single RF Interval length2"(w299) -> ()
            n127 = property on="R Single RF Step2 Coating Power" class="DigNum (strict)"("DisabledEnum"=w300) -> ()  [unwired: 2 in, 2 out]
            n128 = property on="R Single RF Interval length2" class="DigNum (strict)"("DisabledEnum"=w300) -> ()  [unwired: 2 in, 2 out]
          }
          frame #1 {
            w301 = T5."Enabled" ("Disabled")
            n129 = property on="R Single RF Step2 Coating Power" class="DigNum (strict)"("DisabledEnum"=w301) -> ()  [unwired: 2 in, 2 out]
            n130 = property on="R Single RF Interval length2" class="DigNum (strict)"("DisabledEnum"=w301) -> ()  [unwired: 2 in, 2 out]
          }
        }
      }
    }
    n131 = local read "R Single RF Step1 Coating Power Active"() -> (w182:bool)
    n132 = case shown="False" w25 {
      frame #0 {
        w293 = FALSE ("R Single RF Step3 Coating Power Active")
        n133 = local write "R Single RF Step3 Coating Power Active"(w293) -> ()
        n134 = local write "R Single RF Step4 Coating Power Active"(w293) -> ()
        n135 = local write "R Single RF Step5 Coating Power Active"(w293) -> ()
        n136 = local write "R Single RF Step6 Coating Power Active"(w293) -> ()
        n137 = local write "R Single RF Step7 Coating Power Active"(w293) -> ()
        n138 = local write "R Single RF Step8 Coating Power Active"(w293) -> ()
        n139 = local write "R Single RF Step9 Coating Power Active"(w293) -> ()
        n140 = local write "R Single RF Step10 Coating Power Active"(w293) -> ()
      }
      frame #1 {
        n141 = local read "R Single RF Step3 Coating Power Active"() -> (w294:bool)
        n142 = case shown="False" w294 {
          frame #0 {
            w296 = T5."Disabled and Grayed Out" ("Disabled")
            w295 = 0.0 ("Target Clean Power")
            n143 = local write "R Single RF Step3 Coating Power"(w295) -> ()
            n144 = local write "R Single RF Interval length3"(w295) -> ()
            n145 = property on="R Single RF Step3 Coating Power" class="DigNum (strict)"("DisabledEnum"=w296) -> ()  [unwired: 2 in, 2 out]
            n146 = property on="R Single RF Interval length3" class="DigNum (strict)"("DisabledEnum"=w296) -> ()  [unwired: 2 in, 2 out]
          }
          frame #1 {
            w297 = T5."Enabled" ("Disabled")
            n147 = property on="R Single RF Step3 Coating Power" class="DigNum (strict)"("DisabledEnum"=w297) -> ()  [unwired: 2 in, 2 out]
            n148 = property on="R Single RF Interval length3" class="DigNum (strict)"("DisabledEnum"=w297) -> ()  [unwired: 2 in, 2 out]
          }
        }
      }
    }
    n149 = case shown="False" w22 {
      frame #0 {
        w278 = FALSE ("R Single RF Step3 Coating Power Active")
        n150 = local write "R Single RF Step6 Coating Power Active"(w278) -> ()
        n151 = local write "R Single RF Step7 Coating Power Active"(w278) -> ()
        n152 = local write "R Single RF Step8 Coating Power Active"(w278) -> ()
        n153 = local write "R Single RF Step9 Coating Power Active"(w278) -> ()
        n154 = local write "R Single RF Step10 Coating Power Active"(w278) -> ()
      }
      frame #1 {
        n155 = local read "R Single RF Step6 Coating Power Active"() -> (w279:bool)
        n156 = case shown="False" w279 {
          frame #0 {
            w280 = 0.0 ("Target Clean Power")
            w281 = T5."Disabled and Grayed Out" ("Disabled")
            n157 = property on="R Single RF Interval length6" class="DigNum (strict)"("DisabledEnum"=w281) -> ()  [unwired: 2 in, 2 out]
            n158 = property on="R Single RF Step6 Coating Power" class="DigNum (strict)"("DisabledEnum"=w281) -> ()  [unwired: 2 in, 2 out]
            n159 = local write "R Single RF Step6 Coating Power"(w280) -> ()
            n160 = local write "R Single RF Interval length6"(w280) -> ()
          }
          frame #1 {
            w282 = T5."Enabled" ("Disabled")
            n161 = property on="R Single RF Step6 Coating Power" class="DigNum (strict)"("DisabledEnum"=w282) -> ()  [unwired: 2 in, 2 out]
            n162 = property on="R Single RF Interval length6" class="DigNum (strict)"("DisabledEnum"=w282) -> ()  [unwired: 2 in, 2 out]
          }
        }
      }
    }
    n163 = case shown="False" w21 {
      frame #0 {
        n164 = local write "R Single RF Step10 Coating Power Active"(FALSE ("R Single RF Step3 Coating Power Active")) -> ()
      }
      frame #1 {
        n165 = local read "R Single RF Step10 Coating Power Active"() -> (w274:bool)
        n166 = case shown="False" w274 {
          frame #0 {
            w275 = 0.0 ("Target Clean Power")
            w276 = T5."Disabled and Grayed Out" ("Disabled")
            n167 = local write "R Single RF Step10 Coating Power"(w275) -> ()
            n168 = local write "R Single RF Interval length10"(w275) -> ()
            n169 = property on="R Single RF Step10 Coating Power" class="DigNum (strict)"("DisabledEnum"=w276) -> ()  [unwired: 2 in, 2 out]
            n170 = property on="R Single RF Interval length10" class="DigNum (strict)"("DisabledEnum"=w276) -> ()  [unwired: 2 in, 2 out]
          }
          frame #1 {
            w277 = T5."Enabled" ("Disabled")
            n171 = property on="R Single RF Step10 Coating Power" class="DigNum (strict)"("DisabledEnum"=w277) -> ()  [unwired: 2 in, 2 out]
            n172 = property on="R Single RF Interval length10" class="DigNum (strict)"("DisabledEnum"=w277) -> ()  [unwired: 2 in, 2 out]
          }
        }
      }
    }
    n173 = local read "R_Simple_Coating Type Selection"() -> (w190:T2)
    n174 = local read "R Single DC Step1 Coating Power Active"() -> (w183:bool)
    n175 = local read "R_Web_selection"() -> (w195:enum32{"Web", "Other"})
    n176 = local read "R_Recipe_type_selection"() -> (w191:enum32{"Single Recipe", "Combination Sputter"})
    n177 = Wait Until Next ms Multiple(millisecond multiple=u32 50) -> ()  [unwired: 1 out]
    n178 = local read "R Single DC Step1 Coating Power Active"() -> (w166:bool)
    n179 = local read "R Single DC Step4 Coating Power Active"() -> (w158:bool)
    n180 = local read "R Single DC Step3 Coating Power Active"() -> (w160:bool)
    n181 = local read "R Single DC Step2 Coating Power Active"() -> (w164:bool)
    n182 = local read "R Single DC Step5 Coating Power Active"() -> (w150:bool)
    n183 = local read "R Single DC Step6 Coating Power Active"() -> (w149:bool)
    n184 = local read "R Single DC Step7 Coating Power Active"() -> (w148:bool)
    n185 = local read "R Single DC Step10 Coating Power Active"() -> (w145:bool)
    n186 = local read "R Single RF Step7 Coating Power Active"() -> (w110:bool)
    n187 = local read "R Single DC Step8 Coating Power Active"() -> (w147:bool)
    n188 = local read "R Single DC Step9 Coating Power Active"() -> (w146:bool)
    n189 = local read "R Single RF Step9 Coating Power Active"() -> (w108:bool)
    n190 = local read "R Single RF Step10 Coating Power Active"() -> (w107:bool)
    n191 = local read "R Single RF Ramp up"() -> (w180:bool)
    n192 = local read "R Single RF Step1 Coating Power Active"() -> (w125:bool)
    n193 = local read "R Single RF Step2 Coating Power Active"() -> (w115:bool)
    n194 = local read "R Single RF Step3 Coating Power Active"() -> (w114:bool)
    n195 = local read "R Single RF Step4 Coating Power Active"() -> (w113:bool)
    n196 = local read "R Single RF Step5 Coating Power Active"() -> (w112:bool)
    n197 = local read "R Single RF Step6 Coating Power Active"() -> (w111:bool)
    n198 = local read "R Single RF Step8 Coating Power Active"() -> (w109:bool)
    n199 = local read "R Single RF Ramp down"() -> (w181:bool)
    n200 = Equal?(x=w174, y=0) -> (x = y?=w44:bool)
    n201 = Equal?(x=w43, y=1) -> (x = y?=w41:bool)
    n202 = case shown="True" "OK" {
      tunnel: [FALSE w495] -> w38
      frame #0 {
      }
      frame #1 {
        # "TENSION IS NOT LOWER THAN 5\nTENSION IS NOT BIGGER THAN10"
        # "92"
        # "91"
        # "2"
        # "1"
        n203 = local read "R_Web_selection"() -> (w491:enum32{"Web", "Other"})
        n204 = local read "R_Recipe_type_selection"() -> (w513:enum32{"Single Recipe", "Combination Sputter"})
        n205 = local read "R_Recipe_type_selection"() -> (w528:enum32{"Single Recipe", "Combination Sputter"})
        n206 = local read "R_Recipe_type_selection"() -> (w525:enum32{"Single Recipe", "Combination Sputter"})
        n207 = local read "Substrate Material"() -> (w533:string)
        n208 = local read "Recipe Name"() -> (w532:string)
        n209 = Equal?(x=w491, y=1) -> (x = y?=w489:bool)
        n210 = Equal?(x=w533, y="") -> (x = y?=w499:bool)
        n211 = Equal?(x=w513, y=0) -> (x = y?=w515:bool)
        n212 = Equal?(x=w532, y="") -> (x = y?=w534:bool)
        n213 = Equal?(x=w528, y=0) -> (x = y?=w527:bool)
        n214 = Equal?(x=w525, y=0) -> (x = y?=w523:bool)
        n215 = case shown="True" w489 {
          tunnel: [FALSE w724] -> w488
          frame #0 {
          }
          frame #1 {
            n216 = local read "R_Simple_Coating Type Selection"() -> (w725:T2)
            n217 = Equal?(x=w725, y=0) -> (x = y?=w724:bool)
          }
        }
        n218 = case shown="True" w515 {
          tunnel: [FALSE w825] -> w516
          frame #0 {
          }
          frame #1 {
            n219 = local read "R_Simple_Coating Type Selection"() -> (w826:T2)
            n220 = Equal?(x=w826, y=2) -> (x = y?=w825:bool)
          }
        }
        n221 = case shown="True" w527 {
          tunnel: [FALSE w876] -> w526
          frame #0 {
          }
          frame #1 {
            n222 = local read "R_Simple_Coating Type Selection"() -> (w877:T2)
            n223 = Equal?(x=w877, y=0) -> (x = y?=w876:bool)
          }
        }
        n224 = case shown="True" w523 {
          tunnel: [FALSE w866] -> w522
          frame #0 {
          }
          frame #1 {
            n225 = local read "R_Simple_Coating Type Selection"() -> (w867:T2)
            n226 = Equal?(x=w867, y=1) -> (x = y?=w866:bool)
          }
        }
        n227 = local read "R Single RF Step1 Coating Power Active"() -> (w511:bool)
        n228 = local read "R Single RF Step4 Coating Power Active"() -> (w493:bool)
        n229 = local read "R Single RF Step2 Coating Power Active"() -> (w510:bool)
        n230 = local read "R Single DC Step6 Coating Power Active"() -> (w487:bool)
        n231 = local read "R Single DC Step5 Coating Power Active"() -> (w517:bool)
        n232 = local read "R Single DC Step8 Coating Power Active"() -> (w485:bool)
        n233 = local read "R Single RF Step3 Coating Power Active"() -> (w494:bool)
        n234 = local read "R Single DC Step2 Coating Power Active"() -> (w520:bool)
        n235 = local read "R Single DC Step4 Coating Power Active"() -> (w518:bool)
        n236 = local read "R Single DC Step1 Coating Power Active"() -> (w521:bool)
        n237 = local read "R Single DC Step7 Coating Power Active"() -> (w486:bool)
        n238 = local read "R Single DC Step10 Coating Power Active"() -> (w363:bool)
        n239 = local read "R Single RF Step6 Coating Power Active"() -> (w483:bool)
        n240 = local read "R Single RF Step7 Coating Power Active"() -> (w482:bool)
        n241 = local read "R Single DC Step3 Coating Power Active"() -> (w519:bool)
        n242 = local read "R Single RF Step5 Coating Power Active"() -> (w509:bool)
        n243 = local read "R Single DC Step9 Coating Power Active"() -> (w484:bool)
        n244 = local read "R Single RF Step8 Coating Power Active"() -> (w481:bool)
        n245 = local read "R Single RF Ramp up"() -> (w512:bool)
        n246 = case shown="True" w517 {
          tunnel: [FALSE w833] -> w454
          tunnel: [FALSE w830] -> w453
          frame #0 {
          }
          frame #1 {
            # "17"
            # "16"
            n247 = local read "R Single DC Step5 Coating Power"() -> (w832:dbl)
            n248 = local read "R Single DC Interval length5"() -> (w831:dbl)
            n249 = Equal To 0?(x=w832) -> (x = 0?=w833:bool)
            n250 = Equal To 0?(x=w831) -> (x = 0?=w830:bool)
          }
        }
        n251 = case shown="True" w484 {
          tunnel: [FALSE w701] -> w446
          tunnel: [FALSE w700] -> w445
          frame #0 {
          }
          frame #1 {
            # "25"
            # "24"
            n252 = local read "R Single DC Step9 Coating Power"() -> (w699:dbl)
            n253 = local read "R Single DC Interval length9"() -> (w698:dbl)
            n254 = Equal To 0?(x=w699) -> (x = 0?=w701:bool)
            n255 = Equal To 0?(x=w698) -> (x = 0?=w700:bool)
          }
        }
        n256 = case shown="True" w518 {
          tunnel: [FALSE w839] -> w456
          tunnel: [FALSE w836] -> w455
          frame #0 {
          }
          frame #1 {
            # "15"
            # "14"
            n257 = local read "R Single DC Step4 Coating Power"() -> (w838:dbl)
            n258 = local read "R Single DC Interval length4"() -> (w837:dbl)
            n259 = Equal To 0?(x=w838) -> (x = 0?=w839:bool)
            n260 = Equal To 0?(x=w837) -> (x = 0?=w836:bool)
          }
        }
        n261 = case shown="True" w487 {
          tunnel: [FALSE w718] -> w452
          tunnel: [FALSE w716] -> w451
          frame #0 {
          }
          frame #1 {
            # "19"
            # "18"
            n262 = local read "R Single DC Step6 Coating Power"() -> (w719:dbl)
            n263 = local read "R Single DC Interval length6"() -> (w717:dbl)
            n264 = Equal To 0?(x=w719) -> (x = 0?=w718:bool)
            n265 = Equal To 0?(x=w717) -> (x = 0?=w716:bool)
          }
        }
        n266 = case shown="True" w511 {
          tunnel: [FALSE w813] -> w436
          tunnel: [FALSE w810] -> w435
          frame #0 {
          }
          frame #1 {
            # "32"
            # "31"
            n267 = local read "R Single RF  Step1 Coating Power"() -> (w812:dbl)
            n268 = local read "R Single RF Interval length"() -> (w811:dbl)
            n269 = Equal To 0?(x=w811) -> (x = 0?=w810:bool)
            n270 = Equal To 0?(x=w812) -> (x = 0?=w813:bool)
          }
        }
        n271 = case shown="True" w510 {
          tunnel: [FALSE w807] -> w434
          tunnel: [FALSE w804] -> w433
          frame #0 {
          }
          frame #1 {
            # "34"
            # "33"
            n272 = local read "R Single RF Step2 Coating Power"() -> (w806:dbl)
            n273 = local read "R Single RF Interval length2"() -> (w805:dbl)
            n274 = Equal To 0?(x=w806) -> (x = 0?=w807:bool)
            n275 = Equal To 0?(x=w805) -> (x = 0?=w804:bool)
          }
        }
        n276 = case shown="True" w493 {
          tunnel: [FALSE w795] -> w430
          tunnel: [FALSE w792] -> w429
          frame #0 {
          }
          frame #1 {
            # "38"
            # "37"
            n277 = local read "R Single RF Step4 Coating Power"() -> (w794:dbl)
            n278 = local read "R Single RF Interval length4"() -> (w793:dbl)
            n279 = Equal To 0?(x=w794) -> (x = 0?=w795:bool)
            n280 = Equal To 0?(x=w793) -> (x = 0?=w792:bool)
          }
        }
        n281 = case shown="True" w483 {
          tunnel: [FALSE w687] -> w426
          tunnel: [FALSE w686] -> w425
          frame #0 {
          }
          frame #1 {
            # "42"
            # "41"
            n282 = local read "R Single RF Step6 Coating Power"() -> (w689:dbl)
            n283 = local read "R Single RF Interval length6"() -> (w688:dbl)
            n284 = Equal To 0?(x=w689) -> (x = 0?=w687:bool)
            n285 = Equal To 0?(x=w688) -> (x = 0?=w686:bool)
          }
        }
        n286 = case shown="True" w482 {
          tunnel: [FALSE w681] -> w424
          tunnel: [FALSE w680] -> w422
          frame #0 {
          }
          frame #1 {
            # "44"
            # "43"
            n287 = local read "R Single RF Step7 Coating Power"() -> (w683:dbl)
            n288 = local read "R Single RF Interval length7"() -> (w682:dbl)
            n289 = Equal To 0?(x=w683) -> (x = 0?=w681:bool)
            n290 = Equal To 0?(x=w682) -> (x = 0?=w680:bool)
          }
        }
        n291 = case shown="True" w481 {
          tunnel: [FALSE w675] -> w423
          tunnel: [FALSE w674] -> _
          frame #0 {
          }
          frame #1 {
            # "46"
            # "45"
            n292 = local read "R Single RF Step8 Coating Power"() -> (w677:dbl)
            n293 = local read "R Single RF Interval length8"() -> (w676:dbl)
            n294 = Equal To 0?(x=w677) -> (x = 0?=w675:bool)
            n295 = Equal To 0?(x=w676) -> (x = 0?=w674:bool)
          }
        }
        n296 = case shown="True" w521 {
          tunnel: [FALSE w857] -> w462
          tunnel: [FALSE w854] -> w461
          frame #0 {
          }
          frame #1 {
            # "9"
            # "8"
            n297 = local read "R Single DC Step1 Coating Power"() -> (w856:dbl)
            n298 = local read "R Single DC Interval length1"() -> (w855:dbl)
            n299 = Equal To 0?(x=w856) -> (x = 0?=w857:bool)
            n300 = Equal To 0?(x=w855) -> (x = 0?=w854:bool)
          }
        }
        n301 = case shown="True" w520 {
          tunnel: [FALSE w851] -> w460
          tunnel: [FALSE w848] -> w459
          frame #0 {
          }
          frame #1 {
            # "11"
            # "10"
            n302 = local read "R Single DC Step2 Coating Power"() -> (w850:dbl)
            n303 = local read "R Single DC Interval length2"() -> (w849:dbl)
            n304 = Equal To 0?(x=w849) -> (x = 0?=w848:bool)
            n305 = Equal To 0?(x=w850) -> (x = 0?=w851:bool)
          }
        }
        n306 = case shown="True" w485 {
          tunnel: [FALSE w705] -> w448
          tunnel: [FALSE w704] -> w447
          frame #0 {
          }
          frame #1 {
            # "23"
            # "22"
            n307 = local read "R Single DC Step8 Coating Power"() -> (w707:dbl)
            n308 = local read "R Single DC Interval length8"() -> (w706:dbl)
            n309 = Equal To 0?(x=w707) -> (x = 0?=w705:bool)
            n310 = Equal To 0?(x=w706) -> (x = 0?=w704:bool)
          }
        }
        n311 = case shown="True" w509 {
          tunnel: [FALSE w789] -> w428
          tunnel: [FALSE w786] -> w427
          frame #0 {
          }
          frame #1 {
            # "40"
            # "39"
            n312 = local read "R Single RF Step5 Coating Power"() -> (w788:dbl)
            n313 = local read "R Single RF Interval length5"() -> (w787:dbl)
            n314 = Equal To 0?(x=w788) -> (x = 0?=w789:bool)
            n315 = Equal To 0?(x=w787) -> (x = 0?=w786:bool)
          }
        }
        n316 = case shown="True" w519 {
          tunnel: [FALSE w845] -> w458
          tunnel: [FALSE w843] -> w457
          frame #0 {
          }
          frame #1 {
            # "13"
            # "12"
            n317 = local read "R Single DC Step3 Coating Power"() -> (w844:dbl)
            n318 = local read "R Single DC Interval length3"() -> (w842:dbl)
            n319 = Equal To 0?(x=w844) -> (x = 0?=w845:bool)
            n320 = Equal To 0?(x=w842) -> (x = 0?=w843:bool)
          }
        }
        n321 = case shown="True" w486 {
          tunnel: [FALSE w713] -> w450
          tunnel: [FALSE w712] -> w449
          frame #0 {
          }
          frame #1 {
            # "21"
            # "20"
            n322 = local read "R Single DC Step7 Coating Power"() -> (w711:dbl)
            n323 = local read "R Single DC Interval length7"() -> (w710:dbl)
            n324 = Equal To 0?(x=w711) -> (x = 0?=w713:bool)
            n325 = Equal To 0?(x=w710) -> (x = 0?=w712:bool)
          }
        }
        n326 = case shown="True" w494 {
          tunnel: [FALSE w801] -> w432
          tunnel: [FALSE w798] -> w431
          frame #0 {
          }
          frame #1 {
            # "36"
            # "35"
            n327 = local read "R Single RF Step3 Coating Power"() -> (w800:dbl)
            n328 = local read "R Single RF Interval length3"() -> (w799:dbl)
            n329 = Equal To 0?(x=w799) -> (x = 0?=w798:bool)
            n330 = Equal To 0?(x=w800) -> (x = 0?=w801:bool)
          }
        }
        n331 = case shown="True" w512 {
          tunnel: [FALSE w816] -> w437
          frame #0 {
          }
          frame #1 {
            # "30"
            n332 = local read "R Single RF Ramp up Time"() -> (w815:dbl)
            n333 = Equal To 0?(x=w815) -> (x = 0?=w816:bool)
          }
        }
        n334 = case shown="True" w363 {
          tunnel: [FALSE w693] -> w444
          tunnel: [FALSE w692] -> w443
          frame #0 {
          }
          frame #1 {
            # "27"
            # "26"
            n335 = local read "R Single DC Step10 Coating Power"() -> (w695:dbl)
            n336 = local read "R Single DC Interval length10"() -> (w694:dbl)
            n337 = Equal To 0?(x=w695) -> (x = 0?=w693:bool)
            n338 = Equal To 0?(x=w694) -> (x = 0?=w692:bool)
          }
        }
        n339 = case shown="True" w516 {
          tunnel: [FALSE w823] -> w442
          tunnel: [FALSE w819] -> w441
          frame #0 {
          }
          frame #1 {
            # "29"
            # "28"
            n340 = local read "R Single RF Target material"() -> (w821:string)
            n341 = local read "Power_single_rf_list_open"() -> (w820:bool)
            n342 = Not(x=w820) -> (.not. x?=w819:bool)
            n343 = Equal?(x=w821, y="") -> (x = y?=w823:bool)
          }
        }
        n344 = case shown="True" w526 {
          tunnel: [FALSE w873] -> w502
          tunnel: [FALSE w871] -> w501
          frame #0 {
          }
          frame #1 {
            # "4"
            # "3"
            n345 = local read "R_Single Microwave Power"() -> (w874:dbl)
            n346 = local read "R Single Pass Number"() -> (w872:dbl)
            n347 = Equal To 0?(x=w874) -> (x = 0?=w873:bool)
            n348 = Equal To 0?(x=w872) -> (x = 0?=w871:bool)
          }
        }
        n349 = case shown="True" w488 {
          tunnel: [FALSE w721] -> w492
          frame #0 {
          }
          frame #1 {
            # "5"
            n350 = local read "R_Single Microwave Time"() -> (w722:dbl)
            n351 = Equal To 0?(x=w722) -> (x = 0?=w721:bool)
          }
        }
        n352 = case shown="True" w522 {
          tunnel: [FALSE w863] -> w500
          tunnel: [FALSE ("Power_singledc_list_open") w860] -> w463
          frame #0 {
            (unwired) FALSE
          }
          frame #1 {
            # "7"
            # "6"
            n353 = local read "R Single DC Target material"() -> (w864:string)
            n354 = local read "Power_singledc_list_open"() -> (w861:bool)
            n355 = Not(x=w861) -> (.not. x?=w860:bool)
            n356 = Equal?(x=w864, y="") -> (x = y?=w863:bool)
          }
        }
        n357 = local read "R_Recipe_type_selection"() -> (w467:enum32{"Single Recipe", "Combination Sputter"})
        n358 = local read "R_Recipe_type_selection"() -> (w347:enum32{"Single Recipe", "Combination Sputter"})
        n359 = Equal?(x=w467, y=0) -> (x = y?=w465:bool)
        n360 = case shown="True" w465 {
          tunnel: [FALSE w585] -> w361
          frame #0 {
          }
          frame #1 {
            n361 = local read "R_Simple_Coating Type Selection"() -> (w586:T2)
            n362 = Equal?(x=w586, y=1) -> (x = y?=w585:bool)
          }
        }
        n363 = local read "R_Web_selection"() -> (w350:enum32{"Web", "Other"})
        n364 = local read "R_Web_selection"() -> (w531:enum32{"Web", "Other"})
        n365 = local read "Web_selection_tab"() -> (w359:T4)
        n366 = local read "Web_selection_tab"() -> (w357:T4)
        n367 = Equal?(x=w347, y=0) -> (x = y?=w348:bool)
        n368 = Equal?(x=w350, y=0) -> (x = y?=w349:bool)
        n369 = Equal?(x=w531, y=0) -> (x = y?=w354:bool)
        n370 = case shown="True" w348 {
          tunnel: [FALSE w552] -> w352
          frame #0 {
          }
          frame #1 {
            n371 = local read "R_Web_selection"() -> (w551:enum32{"Web", "Other"})
            n372 = Equal?(x=w551, y=0) -> (x = y?=w552:bool)
          }
        }
        n373 = Equal?(x=w359, y=0) -> (x = y?=w358:bool)
        n374 = Equal?(x=w357, y=0) -> (x = y?=w355:bool)
        n375 = local read "R_Web_selection"() -> (w496:enum32{"Web", "Other"})
        n376 = local read "R Single RF Step9 Coating Power Active"() -> (w480:bool)
        n377 = case shown="True" w354 {
          tunnel: [FALSE w559] -> w373
          tunnel: [FALSE w558] -> w372
          frame #0 {
          }
          frame #1 {
            # "96"
            # "95"
            n378 = local read "R Maximum diameter"() -> (w556:dbl)
            n379 = local read "R Minimum diameter"() -> (w557:dbl)
            n380 = Equal To 0?(x=w557) -> (x = 0?=w559:bool)
            n381 = Equal To 0?(x=w556) -> (x = 0?=w558:bool)
          }
        }
        n382 = local read "R Single RF Step10 Coating Power Active"() -> (w479:bool)
        n383 = local read "R Cmb Step1 Coating Power Active"() -> (w477:bool)
        n384 = local read "R Cmb Step4 Coating Power Active"() -> (w474:bool)
        n385 = local read "R Cmb Step3 Coating Power Active"() -> (w475:bool)
        n386 = local read "R Cmb Step2 Coating Power Active"() -> (w476:bool)
        n387 = local read "R Cmb Step5 Coating Power Active"() -> (w473:bool)
        n388 = local read "R Cmb Step7 Coating Power Active"() -> (w471:bool)
        n389 = local read "R Cmb Step6 Coating Power Active"() -> (w472:bool)
        n390 = local read "R Cmb Step10 Coating Power Active"() -> (w468:bool)
        n391 = local read "R Cmb Step8 Coating Power Active"() -> (w470:bool)
        n392 = local read "R_Recipe_type_selection"() -> (w478:enum32{"Single Recipe", "Combination Sputter"})
        n393 = local read "R Cmb Step9 Coating Power Active"() -> (w469:bool)
        n394 = case shown="True" w358 {
          tunnel: [FALSE w567] -> w364
          frame #0 {
          }
          frame #1 {
            n395 = local read "R_Simple_Coating Type Selection"() -> (w565:T2)
            n396 = Equal?(x=w565, y=2) -> (x = y?=w567:bool)
          }
        }
        n397 = case shown="False" w355 {
          tunnel: [FALSE w561] -> w464
          frame #0 {
          }
          frame #1 {
            n398 = local read "R_Recipe_type_selection"() -> (w563:enum32{"Single Recipe", "Combination Sputter"})
            n399 = Equal?(x=w563, y=1) -> (x = y?=w561:bool)
          }
        }
        n400 = case shown="True" w361 {
          tunnel: [FALSE w569] -> w362
          frame #0 {
          }
          frame #1 {
            n401 = local read "Web_selection_tab"() -> (w570:T4)
            n402 = Equal?(x=w570, y=0) -> (x = y?=w569:bool)
          }
        }
        n403 = local read "R Single RF Ramp down"() -> (w508:bool)
        n404 = local read "Thickness_Monitor_Active"() -> (w505:bool)
        n405 = Equal?(x=w496, y=1) -> (x = y?=w498:bool)
        n406 = case shown="True" w498 {
          tunnel: [FALSE w730] -> w375
          tunnel: [FALSE w729] -> w374
          frame #0 {
          }
          frame #1 {
            # "94"
            # "93"
            n407 = local read "R_Thickness Selection"() -> (w736:enum32{"Thickness", "Time"})
            n408 = local read "R_Thickness Selection"() -> (w733:enum32{"Thickness", "Time"})
            n409 = Equal?(x=w736, y=0) -> (x = y?=w732:bool)
            n410 = Equal?(x=w733, y=1) -> (x = y?=w731:bool)
            n411 = case shown="True" w732 {
              tunnel: [FALSE w741] -> w730
              frame #0 {
              }
              frame #1 {
                n412 = local read "R_Target Thickness Value"() -> (w742:dbl)
                n413 = Equal To 0?(x=w742) -> (x = 0?=w741:bool)
              }
            }
            n414 = case shown="True" w731 {
              tunnel: [FALSE w738] -> w729
              frame #0 {
              }
              frame #1 {
                n415 = local read "R_Duration"() -> (w739:dbl)
                n416 = Equal To 0?(x=w739) -> (x = 0?=w738:bool)
              }
            }
          }
        }
        n417 = case shown="True" w352 {
          tunnel: [FALSE w549] -> w371
          frame #0 {
          }
          frame #1 {
            # "97"
            n418 = local read "R Web speed(cm/min)"() -> (w548:dbl)
            n419 = Equal To 0?(x=w548) -> (x = 0?=w549:bool)
          }
        }
        n420 = case shown="True" w349 {
          tunnel: [FALSE w546] -> w370
          tunnel: [FALSE w545] -> w369
          tunnel: [FALSE w544] -> w368
          frame #0 {
          }
          frame #1 {
            # "100"
            # "99"
            # "98"
            n421 = local read "R Web thickness"() -> (w541:dbl)
            n422 = local read "R Tension Value"() -> (w543:dbl)
            n423 = local read "R  Total length"() -> (w542:dbl)
            n424 = Equal To 0?(x=w541) -> (x = 0?=w546:bool)
            n425 = Equal To 0?(x=w543) -> (x = 0?=w545:bool)
            n426 = Equal To 0?(x=w542) -> (x = 0?=w544:bool)
          }
        }
        n427 = Equal?(x=w478, y=1) -> (x = y?=w506:bool)
        n428 = case shown="True" w470 {
          tunnel: [FALSE w614] -> w389
          tunnel: [FALSE w613] -> w388
          tunnel: [FALSE w612] -> w387
          frame #0 {
          }
          frame #1 {
            # "81"
            # "80"
            # "79"
            n429 = local read "R Cmb Ch2 Step8 Coating Power"() -> (w611:dbl)
            n430 = local read "R Cmb Ch3 Step8 Coating Power"() -> (w610:dbl)
            n431 = local read "R Cmb Interval length 8"() -> (w609:dbl)
            n432 = Equal To 0?(x=w611) -> (x = 0?=w614:bool)
            n433 = Equal To 0?(x=w610) -> (x = 0?=w613:bool)
            n434 = Equal To 0?(x=w609) -> (x = 0?=w612:bool)
          }
        }
        n435 = case shown="True" w506 {
          tunnel: [FALSE w776] -> w416
          tunnel: [FALSE w775] -> w414
          tunnel: [FALSE w772] -> w415
          tunnel: [FALSE w771] -> w413
          tunnel: [FALSE w769] -> w411
          tunnel: [FALSE ("Power_list_open") w767] -> w412
          frame #0 {
          }
          frame #1 {
            # "57"
            # "56"
            # "55"
            # "54"
            # "53"
            # "52"
            n436 = local read "R Cmb Ch2 Target material"() -> (w779:string)
            n437 = local read "R Cmb Ch3 Target material"() -> (w777:string)
            n438 = local read "R Cmb Number of cycle"() -> (w770:dbl)
            n439 = local read "R_Cmb_Ch2_Web_speed"() -> (w774:dbl)
            n440 = local read "R_Cmb_Ch3_Web_speed"() -> (w773:dbl)
            n441 = local read "Power_list_open_multi"() -> (w768:bool)
            n442 = Equal?(x=w777, y="") -> (x = y?=w775:bool)
            n443 = Equal?(x=w779, y="") -> (x = y?=w776:bool)
            n444 = Equal To 0?(x=w774) -> (x = 0?=w772:bool)
            n445 = Equal To 0?(x=w773) -> (x = 0?=w771:bool)
            n446 = Equal To 0?(x=w770) -> (x = 0?=w769:bool)
            n447 = Not(x=w768) -> (.not. x?=w767:bool)
          }
        }
        n448 = case shown="True" w480 {
          tunnel: [FALSE w670] -> w421
          tunnel: [FALSE w668] -> w420
          frame #0 {
          }
          frame #1 {
            # "48"
            # "47"
            n449 = local read "R Single RF Step9 Coating Power"() -> (w671:dbl)
            n450 = local read "R Single RF Interval length9"() -> (w669:dbl)
            n451 = Equal To 0?(x=w669) -> (x = 0?=w668:bool)
            n452 = Equal To 0?(x=w671) -> (x = 0?=w670:bool)
          }
        }
        n453 = case shown="True" w479 {
          tunnel: [FALSE w663] -> w419
          tunnel: [FALSE w662] -> w418
          frame #0 {
          }
          frame #1 {
            # "50"
            # "49"
            n454 = local read "R Single RF Step10 Coating Power"() -> (w665:dbl)
            n455 = local read "R Single RF Interval length10"() -> (w664:dbl)
            n456 = Equal To 0?(x=w664) -> (x = 0?=w662:bool)
            n457 = Equal To 0?(x=w665) -> (x = 0?=w663:bool)
          }
        }
        n458 = case shown="True" w508 {
          tunnel: [FALSE w782] -> w417
          frame #0 {
          }
          frame #1 {
            # "51"
            n459 = local read "R Single RF Ramp down Time"() -> (w783:dbl)
            n460 = Equal To 0?(x=w783) -> (x = 0?=w782:bool)
          }
        }
        n461 = case shown="True" w468 {
          tunnel: [FALSE w596] -> w383
          tunnel: [FALSE w595] -> w382
          tunnel: [FALSE w594] -> w381
          frame #0 {
          }
          frame #1 {
            # "87"
            # "86"
            # "85"
            n462 = local read "R Cmb Ch2 Step10 Coating Power"() -> (w593:dbl)
            n463 = local read "R Cmb Ch3 Step10 Coating Power"() -> (w592:dbl)
            n464 = local read "R Cmb Interval length 10"() -> (w591:dbl)
            n465 = Equal To 0?(x=w593) -> (x = 0?=w596:bool)
            n466 = Equal To 0?(x=w592) -> (x = 0?=w595:bool)
            n467 = Equal To 0?(x=w591) -> (x = 0?=w594:bool)
          }
        }
        n468 = case shown="True" w472 {
          tunnel: [FALSE w632] -> w395
          tunnel: [FALSE w631] -> w394
          tunnel: [FALSE w630] -> w393
          frame #0 {
          }
          frame #1 {
            # "75"
            # "74"
            # "73"
            n469 = local read "R Cmb Ch2 Step6 Coating Power"() -> (w629:dbl)
            n470 = local read "R Cmb Ch3 Step6 Coating Power"() -> (w628:dbl)
            n471 = local read "R Cmb Interval length 6"() -> (w627:dbl)
            n472 = Equal To 0?(x=w629) -> (x = 0?=w632:bool)
            n473 = Equal To 0?(x=w628) -> (x = 0?=w631:bool)
            n474 = Equal To 0?(x=w627) -> (x = 0?=w630:bool)
          }
        }
        n475 = case shown="True" w469 {
          tunnel: [FALSE w605] -> w386
          tunnel: [FALSE w604] -> w385
          tunnel: [FALSE w603] -> w384
          frame #0 {
          }
          frame #1 {
            # "84"
            # "83"
            # "82"
            n476 = local read "R Cmb Ch2 Step9 Coating Power"() -> (w602:dbl)
            n477 = local read "R Cmb Ch3 Step9 Coating Power"() -> (w601:dbl)
            n478 = local read "R Cmb Interval length 9"() -> (w600:dbl)
            n479 = Equal To 0?(x=w602) -> (x = 0?=w605:bool)
            n480 = Equal To 0?(x=w601) -> (x = 0?=w604:bool)
            n481 = Equal To 0?(x=w600) -> (x = 0?=w603:bool)
          }
        }
        n482 = case shown="True" w471 {
          tunnel: [FALSE w623] -> w392
          tunnel: [FALSE w622] -> w391
          tunnel: [FALSE w621] -> w390
          frame #0 {
          }
          frame #1 {
            # "78"
            # "77"
            # "76"
            n483 = local read "R Cmb Ch2 Step7 Coating Power"() -> (w620:dbl)
            n484 = local read "R Cmb Ch3 Step7 Coating Power"() -> (w619:dbl)
            n485 = local read "R Cmb Interval length 7"() -> (w618:dbl)
            n486 = Equal To 0?(x=w620) -> (x = 0?=w623:bool)
            n487 = Equal To 0?(x=w619) -> (x = 0?=w622:bool)
            n488 = Equal To 0?(x=w618) -> (x = 0?=w621:bool)
          }
        }
        n489 = case shown="True" w477 {
          tunnel: [FALSE w760] -> w410
          tunnel: [FALSE w759] -> w409
          tunnel: [FALSE w758] -> w408
          frame #0 {
          }
          frame #1 {
            # "60"
            # "59"
            # "58"
            n490 = local read "R Cmb Ch2 Step1 Coating Power"() -> (w756:dbl)
            n491 = local read "R Cmb Ch3 Step1 Coating Power"() -> (w755:dbl)
            n492 = local read "R Cmb Interval length 1"() -> (w757:dbl)
            n493 = Equal To 0?(x=w756) -> (x = 0?=w760:bool)
            n494 = Equal To 0?(x=w755) -> (x = 0?=w759:bool)
            n495 = Equal To 0?(x=w757) -> (x = 0?=w758:bool)
          }
        }
        n496 = case shown="True" w476 {
          tunnel: [FALSE w751] -> w407
          tunnel: [FALSE w750] -> w406
          tunnel: [FALSE w749] -> w405
          frame #0 {
          }
          frame #1 {
            # "63"
            # "62"
            # "61"
            n497 = local read "R Cmb Ch2 Step2 Coating Power"() -> (w748:dbl)
            n498 = local read "R Cmb Ch3 Step2 Coating Power"() -> (w747:dbl)
            n499 = local read "R Cmb Interval length 2"() -> (w746:dbl)
            n500 = Equal To 0?(x=w748) -> (x = 0?=w751:bool)
            n501 = Equal To 0?(x=w747) -> (x = 0?=w750:bool)
            n502 = Equal To 0?(x=w746) -> (x = 0?=w749:bool)
          }
        }
        n503 = case shown="True" w475 {
          tunnel: [FALSE w659] -> w404
          tunnel: [FALSE w658] -> w403
          tunnel: [FALSE w657] -> w402
          frame #0 {
          }
          frame #1 {
            # "66"
            # "65"
            # "64"
            n504 = local read "R Cmb Ch3 Step3 Coating Power"() -> (w655:dbl)
            n505 = local read "R Cmb Ch2 Step3 Coating Power"() -> (w656:dbl)
            n506 = local read "R Cmb Interval length 3"() -> (w654:dbl)
            n507 = Equal To 0?(x=w656) -> (x = 0?=w659:bool)
            n508 = Equal To 0?(x=w655) -> (x = 0?=w658:bool)
            n509 = Equal To 0?(x=w654) -> (x = 0?=w657:bool)
          }
        }
        n510 = case shown="True" w474 {
          tunnel: [FALSE w650] -> w401
          tunnel: [FALSE w649] -> w400
          tunnel: [FALSE w648] -> w399
          frame #0 {
          }
          frame #1 {
            # "69"
            # "68"
            # "67"
            n511 = local read "R Cmb Ch3 Step4 Coating Power"() -> (w646:dbl)
            n512 = local read "R Cmb Ch2 Step4 Coating Power"() -> (w647:dbl)
            n513 = local read "R Cmb Interval length 4"() -> (w645:dbl)
            n514 = Equal To 0?(x=w647) -> (x = 0?=w650:bool)
            n515 = Equal To 0?(x=w646) -> (x = 0?=w649:bool)
            n516 = Equal To 0?(x=w645) -> (x = 0?=w648:bool)
          }
        }
        n517 = case shown="True" w473 {
          tunnel: [FALSE w641] -> w398
          tunnel: [FALSE w640] -> w397
          tunnel: [FALSE w639] -> w396
          frame #0 {
          }
          frame #1 {
            # "72"
            # "71"
            # "70"
            n518 = local read "R Cmb Ch2 Step5 Coating Power"() -> (w638:dbl)
            n519 = local read "R Cmb Ch3 Step5 Coating Power"() -> (w637:dbl)
            n520 = local read "R Cmb Interval length 5"() -> (w636:dbl)
            n521 = Equal To 0?(x=w638) -> (x = 0?=w641:bool)
            n522 = Equal To 0?(x=w637) -> (x = 0?=w640:bool)
            n523 = Equal To 0?(x=w636) -> (x = 0?=w639:bool)
          }
        }
        n524 = case shown="True" w505 {
          tunnel: [FALSE w885] -> w380
          tunnel: [FALSE w884] -> w379
          tunnel: [FALSE w882] -> w378
          frame #0 {
          }
          frame #1 {
            # "90"
            # "89"
            # "88"
            n525 = local read "R Toooling_factor"() -> (w883:dbl)
            n526 = local read "R Material_density"() -> (w887:dbl)
            n527 = local read "R Z_factor"() -> (w886:dbl)
            n528 = Equal To 0?(x=w883) -> (x = 0?=w882:bool)
            n529 = Equal To 0?(x=w886) -> (x = 0?=w884:bool)
            n530 = Equal To 0?(x=w887) -> (x = 0?=w885:bool)
          }
        }
        n531 = local read "R Set Pressure mtorr"() -> (w503:dbl)
        n532 = local read "R Argon Flow sccm"() -> (w504:dbl)
        n533 = case shown="True" w362 {
          tunnel: [FALSE w581] -> w367
          frame #0 {
          }
          frame #1 {
            # "101"
            n534 = local read "Calculated_total_length_dc"() -> (w583:dbl)
            n535 = local read "R  Total length"() -> (w582:dbl)
            n536 = Less?(x=w582, y=w583) -> (x < y?=w581:bool)
          }
        }
        n537 = case shown="True" w464 {
          tunnel: [FALSE w573] -> w365
          frame #0 {
          }
          frame #1 {
            # "103"
            n538 = local read "Calculated_total_length_cmb"() -> (w575:dbl)
            n539 = local read "R  Total length"() -> (w574:dbl)
            n540 = Less?(x=w574, y=w575) -> (x < y?=w573:bool)
          }
        }
        n541 = case shown="True" w364 {
          tunnel: [FALSE w577] -> w366
          frame #0 {
          }
          frame #1 {
            # "102"
            n542 = local read "Calculated_total_length_rf"() -> (w579:dbl)
            n543 = local read "R  Total length"() -> (w578:dbl)
            n544 = Less?(x=w578, y=w579) -> (x < y?=w577:bool)
          }
        }
        n545 = Equal To 0?(x=w503) -> (x = 0?=w376:bool)
        n546 = Equal To 0?(x=w504) -> (x = 0?=w377:bool)
        n547 = Build Array(FALSE, w534, w499, w502, w501, w492, w500, w463, w462, w461, w460, w459, w458, w457, w456, w455, w454, w453, w452, w451, w450, w449, w448, w447, w446, w445, w444, w443, w442, w441, w437, w436, w435, w434, w433, w432, w431, w430, w429, w428, w427, w426, w425, w424, w423, w422, w421, w420, w419, w418, w417, w416, w415, w414, w413, w412, w411, w410, w409, w408, w407, w406, w405, w404, w403, w402, w401, w400, w399, w398, w397, w396, w395, w394, w393, w392, w391, w390, w389, w388, w387, w386, w385, w384, w383, w382, w381, w380, w379, w378, w377, w376, w375, w374, w373, w372, w371, w370, w369, w368, w367, w366, w365) -> (w440:bool[])
        n548 = Boolean To (0,1)(Boolean=w440) -> (0, 1=w439:i16[])
        n549 = Array Max & Min(array=w439) -> (max index (indices)=w438:i32)  [unwired: 3 out]
        n550 = case shown="91" w438 {
          tunnel: [TRUE FALSE FALSE FALSE FALSE FALSE FALSE FALSE FALSE FALSE FALSE FALSE FALSE FALSE FALSE FALSE FALSE FALSE FALSE FALSE FALSE FALSE FALSE FALSE FALSE FALSE FALSE FALSE FALSE FALSE FALSE FALSE FALSE FALSE FALSE FALSE FALSE FALSE FALSE FALSE FALSE FALSE FALSE FALSE FALSE FALSE FALSE FALSE FALSE FALSE FALSE FALSE FALSE FALSE FALSE FALSE FALSE FALSE FALSE FALSE FALSE FALSE FALSE FALSE FALSE FALSE FALSE FALSE FALSE FALSE FALSE FALSE FALSE FALSE FALSE FALSE FALSE FALSE FALSE FALSE FALSE FALSE FALSE FALSE FALSE FALSE FALSE FALSE FALSE FALSE FALSE TRUE FALSE FALSE FALSE FALSE FALSE FALSE FALSE FALSE FALSE FALSE FALSE FALSE] -> w495
          frame #0 {
          }
          frame #1 {
            n551 = One Button Dialog(message="Please enter the Recipe name !") -> ()  [unwired: 1 in, 1 out]
          }
          frame #2 {
            n552 = One Button Dialog(message="Please enter the Substrate Material name !") -> ()  [unwired: 1 in, 1 out]
          }
          frame #3 {
            n553 = One Button Dialog(message="Please enter Microwave Power!") -> ()  [unwired: 1 in, 1 out]
          }
          frame #4 {
            n554 = One Button Dialog(message="Please enter Pass Number !") -> ()  [unwired: 1 in, 1 out]
          }
          frame #5 {
            n555 = One Button Dialog(message="Please enter Microwave Duration !") -> ()  [unwired: 1 in, 1 out]
          }
          frame #6 {
            n556 = One Button Dialog(message="Please enter DC Target Material name !") -> ()  [unwired: 1 in, 1 out]
          }
          frame #7 {
            n557 = One Button Dialog(message="Please click Process List!") -> ()  [unwired: 1 in, 1 out]
          }
          frame #8 {
            n558 = One Button Dialog(message="Please enter DC Coating Power!") -> ()  [unwired: 1 in, 1 out]
          }
          frame #9 {
            n559 = One Button Dialog(message="Please enter interval length!") -> ()  [unwired: 1 in, 1 out]
          }
          frame #10 {
            n560 = One Button Dialog(message="Please enter DC Coating Power!") -> ()  [unwired: 1 in, 1 out]
          }
          frame #11 {
            n561 = One Button Dialog(message="Please enter interval length!") -> ()  [unwired: 1 in, 1 out]
          }
          frame #12 {
            n562 = One Button Dialog(message="Please enter DC Coating Power !") -> ()  [unwired: 1 in, 1 out]
          }
          frame #13 {
            n563 = One Button Dialog(message="Please enter interval length!") -> ()  [unwired: 1 in, 1 out]
          }
          frame #14 {
            n564 = One Button Dialog(message="Please enter DC Coating Power!") -> ()  [unwired: 1 in, 1 out]
          }
          frame #15 {
            n565 = One Button Dialog(message="Please enter interval length!") -> ()  [unwired: 1 in, 1 out]
          }
          frame #16 {
            n566 = One Button Dialog(message="Please enter DC Coating Power !") -> ()  [unwired: 1 in, 1 out]
          }
          frame #17 {
            n567 = One Button Dialog(message="Please enter interval length!") -> ()  [unwired: 1 in, 1 out]
          }
          frame #18 {
            n568 = One Button Dialog(message="Please enter DC Coating Power !") -> ()  [unwired: 1 in, 1 out]
          }
          frame #19 {
            n569 = One Button Dialog(message="Please enter interval length!") -> ()  [unwired: 1 in, 1 out]
          }
          frame #20 {
            n570 = One Button Dialog(message="Please enter DC Coating Power !") -> ()  [unwired: 1 in, 1 out]
          }
          frame #21 {
            n571 = One Button Dialog(message="Please enter interval length!") -> ()  [unwired: 1 in, 1 out]
          }
          frame #22 {
            n572 = One Button Dialog(message="Please enter DC Coating Power !") -> ()  [unwired: 1 in, 1 out]
          }
          frame #23 {
            n573 = One Button Dialog(message="Please enter interval length!") -> ()  [unwired: 1 in, 1 out]
          }
          frame #24 {
            n574 = One Button Dialog(message="Please enter DC Coating Power !") -> ()  [unwired: 1 in, 1 out]
          }
          frame #25 {
            n575 = One Button Dialog(message="Please enter interval length!") -> ()  [unwired: 1 in, 1 out]
          }
          frame #26 {
            n576 = One Button Dialog(message="Please enter DC Coating Power !") -> ()  [unwired: 1 in, 1 out]
          }
          frame #27 {
            n577 = One Button Dialog(message="Please enter interval length!") -> ()  [unwired: 1 in, 1 out]
          }
          frame #28 {
            n578 = One Button Dialog(message="Please enter RF Target Material !") -> ()  [unwired: 1 in, 1 out]
          }
          frame #29 {
            n579 = One Button Dialog(message="Please click Process List!") -> ()  [unwired: 1 in, 1 out]
          }
          frame #30 {
            n580 = One Button Dialog(message="Please enter RF Ramp Up Time!") -> ()  [unwired: 1 in, 1 out]
          }
          frame #31 {
            n581 = One Button Dialog(message="Please enter RF Coating Power  !") -> ()  [unwired: 1 in, 1 out]
          }
          frame #32 {
            n582 = One Button Dialog(message="Please enter interval length !") -> ()  [unwired: 1 in, 1 out]
          }
          frame #33 {
            n583 = One Button Dialog(message="Please enter RF Coating Power  !") -> ()  [unwired: 1 in, 1 out]
          }
          frame #34 {
            n584 = One Button Dialog(message="Please enter interval length!") -> ()  [unwired: 1 in, 1 out]
          }
          frame #35 {
            n585 = One Button Dialog(message="Please enter RF Coating Power  !") -> ()  [unwired: 1 in, 1 out]
          }
          frame #36 {
            n586 = One Button Dialog(message="Please enter interval length!") -> ()  [unwired: 1 in, 1 out]
          }
          frame #37 {
            n587 = One Button Dialog(message="Please enter RF Coating Power !") -> ()  [unwired: 1 in, 1 out]
          }
          frame #38 {
            n588 = One Button Dialog(message="Please enter interval length!") -> ()  [unwired: 1 in, 1 out]
          }
          frame #39 {
            n589 = One Button Dialog(message="Please enter RF Coating Power !") -> ()  [unwired: 1 in, 1 out]
          }
          frame #40 {
            n590 = One Button Dialog(message="Please enter interval length!") -> ()  [unwired: 1 in, 1 out]
          }
          frame #41 {
            n591 = One Button Dialog(message="Please enter RF Coating Power !") -> ()  [unwired: 1 in, 1 out]
          }
          frame #42 {
            n592 = One Button Dialog(message="Please enter interval length!") -> ()  [unwired: 1 in, 1 out]
          }
          frame #43 {
            n593 = One Button Dialog(message="Please enter RF Coating Power !") -> ()  [unwired: 1 in, 1 out]
          }
          frame #44 {
            n594 = One Button Dialog(message="Please enter interval length!") -> ()  [unwired: 1 in, 1 out]
          }
          frame #45 {
            n595 = One Button Dialog(message="Please enter RF Coating Power !") -> ()  [unwired: 1 in, 1 out]
          }
          frame #46 {
            n596 = One Button Dialog(message="Please enter interval length!") -> ()  [unwired: 1 in, 1 out]
          }
          frame #47 {
            n597 = One Button Dialog(message="Please enter RF Coating Power !") -> ()  [unwired: 1 in, 1 out]
          }
          frame #48 {
            n598 = One Button Dialog(message="Please enter interval length!") -> ()  [unwired: 1 in, 1 out]
          }
          frame #49 {
            n599 = One Button Dialog(message="Please enter RF Coating Power !") -> ()  [unwired: 1 in, 1 out]
          }
          frame #50 {
            n600 = One Button Dialog(message="Please enter interval length!") -> ()  [unwired: 1 in, 1 out]
          }
          frame #51 {
            n601 = One Button Dialog(message="Please enter RF Ramp Down Time  !") -> ()  [unwired: 1 in, 1 out]
          }
          frame #52 {
            n602 = One Button Dialog(message="Please enter Chamber II\nTarget Material name!") -> ()  [unwired: 1 in, 1 out]
          }
          frame #53 {
            n603 = One Button Dialog(message="Please enter web speed!") -> ()  [unwired: 1 in, 1 out]
          }
          frame #54 {
            n604 = One Button Dialog(message="Please enter Chamber III Target Material \nName !") -> ()  [unwired: 1 in, 1 out]
          }
          frame #55 {
            n605 = One Button Dialog(message="Please enter Web Speed !") -> ()  [unwired: 1 in, 1 out]
          }
          frame #56 {
            n606 = One Button Dialog(message="Please click process list !") -> ()  [unwired: 1 in, 1 out]
          }
          frame #57 {
            n607 = One Button Dialog(message="Please enter Number of Cycle !") -> ()  [unwired: 1 in, 1 out]
          }
          frame #58 {
            n608 = One Button Dialog(message="Please enter Chamber II  Coating Power !") -> ()  [unwired: 1 in, 1 out]
          }
          frame #59 {
            n609 = One Button Dialog(message="Please enter Chamber III  Coating Power !") -> ()  [unwired: 1 in, 1 out]
          }
          frame #60 {
            n610 = One Button Dialog(message="Please enter interval length!") -> ()  [unwired: 1 in, 1 out]
          }
          frame #61 {
            n611 = One Button Dialog(message="Please enter Chamber II  Coating Power !") -> ()  [unwired: 1 in, 1 out]
          }
          frame #62 {
            n612 = One Button Dialog(message="Please enter Chamber III  Coating Power !") -> ()  [unwired: 1 in, 1 out]
          }
          frame #63 {
            n613 = One Button Dialog(message="Please enter interval length!") -> ()  [unwired: 1 in, 1 out]
          }
          frame #64 {
            n614 = One Button Dialog(message="Please enter Chamber II  Coating Power !") -> ()  [unwired: 1 in, 1 out]
          }
          frame #65 {
            n615 = One Button Dialog(message="Please enter Chamber III Coating Power !") -> ()  [unwired: 1 in, 1 out]
          }
          frame #66 {
            n616 = One Button Dialog(message="Please enter interval length!") -> ()  [unwired: 1 in, 1 out]
          }
          frame #67 {
            n617 = One Button Dialog(message="Please enter Chamber II  Coating Power !") -> ()  [unwired: 1 in, 1 out]
          }
          frame #68 {
            n618 = One Button Dialog(message="Please enter Chamber III  Coating Power !") -> ()  [unwired: 1 in, 1 out]
          }
          frame #69 {
            n619 = One Button Dialog(message="Please enter interval length!") -> ()  [unwired: 1 in, 1 out]
          }
          frame #70 {
            n620 = One Button Dialog(message="Please enter Chamber II  Coating Power !") -> ()  [unwired: 1 in, 1 out]
          }
          frame #71 {
            n621 = One Button Dialog(message="Please enter Chamber III  Coating Power !") -> ()  [unwired: 1 in, 1 out]
          }
          frame #72 {
            n622 = One Button Dialog(message="Please enter interval length!") -> ()  [unwired: 1 in, 1 out]
          }
          frame #73 {
            n623 = One Button Dialog(message="Please enter Chamber II  Coating Power !") -> ()  [unwired: 1 in, 1 out]
          }
          frame #74 {
            n624 = One Button Dialog(message="Please enter Chamber III  Coating Power !") -> ()  [unwired: 1 in, 1 out]
          }
          frame #75 {
            n625 = One Button Dialog(message="Please enter interval length!") -> ()  [unwired: 1 in, 1 out]
          }
          frame #76 {
            n626 = One Button Dialog(message="Please enter Chamber II  Coating Power !") -> ()  [unwired: 1 in, 1 out]
          }
          frame #77 {
            n627 = One Button Dialog(message="Please enter Chamber III  Coating Power !") -> ()  [unwired: 1 in, 1 out]
          }
          frame #78 {
            n628 = One Button Dialog(message="Please enter interval length!") -> ()  [unwired: 1 in, 1 out]
          }
          frame #79 {
            n629 = One Button Dialog(message="Please enter Chamber II  Coating Power !") -> ()  [unwired: 1 in, 1 out]
          }
          frame #80 {
            n630 = One Button Dialog(message="Please enter Chamber III  Coating Power !") -> ()  [unwired: 1 in, 1 out]
          }
          frame #81 {
            n631 = One Button Dialog(message="Please enter interval length!") -> ()  [unwired: 1 in, 1 out]
          }
          frame #82 {
            n632 = One Button Dialog(message="Please enter Chamber II  Coating Power !") -> ()  [unwired: 1 in, 1 out]
          }
          frame #83 {
            n633 = One Button Dialog(message="Please enter Chamber III  Coating Power !") -> ()  [unwired: 1 in, 1 out]
          }
          frame #84 {
            n634 = One Button Dialog(message="Please enter interval length!") -> ()  [unwired: 1 in, 1 out]
          }
          frame #85 {
            n635 = One Button Dialog(message="Please enter Chamber II  Coating Power !") -> ()  [unwired: 1 in, 1 out]
          }
          frame #86 {
            n636 = One Button Dialog(message="Please enter Chamber III  Coating Power !") -> ()  [unwired: 1 in, 1 out]
          }
          frame #87 {
            n637 = One Button Dialog(message="Please enter interval length!") -> ()  [unwired: 1 in, 1 out]
          }
          frame #88 {
            n638 = One Button Dialog(message="Please enter Material Density !") -> ()  [unwired: 1 in, 1 out]
          }
          frame #89 {
            n639 = One Button Dialog(message="Please enter Z factor !") -> ()  [unwired: 1 in, 1 out]
          }
          frame #90 {
            n640 = One Button Dialog(message="Please enter Tooling Factor !") -> ()  [unwired: 1 in, 1 out]
          }
          frame #91 {
            n641 = disable-structure shown="Disabled" {
              frame #0 {
                n642 = One Button Dialog(message="Please enter Argon Flow !") -> ()  [unwired: 1 in, 1 out]
              }
              frame #1 {
              }
            }
          }
          frame #92 {
            n643 = One Button Dialog(message="Please enter Set Pressure !") -> ()  [unwired: 1 in, 1 out]
          }
          frame #93 {
            n644 = One Button Dialog(message="Please enter Target thickness Value!") -> ()  [unwired: 1 in, 1 out]
          }
          frame #94 {
            n645 = One Button Dialog(message="Please enter Duration!") -> ()  [unwired: 1 in, 1 out]
          }
          frame #95 {
            n646 = One Button Dialog(message="Please enter Minimum Diameter !") -> ()  [unwired: 1 in, 1 out]
          }
          frame #96 {
            n647 = One Button Dialog(message="Please enter Maximum Diameter !") -> ()  [unwired: 1 in, 1 out]
          }
          frame #97 {
            n648 = One Button Dialog(message="Please enter Web Speed !") -> ()  [unwired: 1 in, 1 out]
          }
          frame #98 {
            n649 = One Button Dialog(message="Please enter Web Thickness !") -> ()  [unwired: 1 in, 1 out]
          }
          frame #99 {
            n650 = One Button Dialog(message="Please enter Tension Value !") -> ()  [unwired: 1 in, 1 out]
          }
          frame #100 {
            n651 = One Button Dialog(message="Please click equal sign!") -> ()  [unwired: 1 in, 1 out]
          }
          frame #101 {
            n652 = One Button Dialog(message="Total length is not enough for process !") -> ()  [unwired: 1 in, 1 out]
          }
          frame #102 {
            n653 = One Button Dialog(message="Total length is not enough for process !") -> ()  [unwired: 1 in, 1 out]
          }
          frame #103 {
            n654 = One Button Dialog(message="Total length is not enough for process !") -> ()  [unwired: 1 in, 1 out]
          }
        }
      }
    }
    n655 = case shown="True" w44 {
      frame #0 {
      }
      frame #1 {
        n656 = local read "R_Thickness Selection"() -> (w1100:enum32{"Thickness", "Time"})
        n657 = case shown="\"Thickness\", Default" w1100 {
          frame #0 {
            n658 = local write "R_Duration"(0.0 ("R_Duration")) -> ()
            n659 = property on="R_Target Thickness Value" class="DigNum (strict)"("DisabledEnum"=T5."Enabled" ("Disabled")) -> ()  [unwired: 2 in, 2 out]
            n660 = property on="R_Duration" class="DigNum (strict)"("DisabledEnum"=T5."Disabled and Grayed Out" ("Disabled")) -> ()  [unwired: 2 in, 2 out]
          }
          frame #1 {
            n661 = local write "R_Target Thickness Value"(0.0 ("R_Target Thickness Value")) -> ()
            n662 = property on="R_Target Thickness Value" class="DigNum (strict)"("DisabledEnum"=T5."Disabled and Grayed Out" ("Disabled")) -> ()  [unwired: 2 in, 2 out]
            n663 = property on="R_Duration" class="DigNum (strict)"("DisabledEnum"=T5."Enabled" ("Disabled")) -> ()  [unwired: 2 in, 2 out]
          }
        }
      }
    }
    n664 = case shown="True" w41 {
      frame #0 {
        n665 = property on="R_Thickness Selection" class="RadioBtnsControl (strict)"("DisabledEnum"=T5."Enabled" ("Disabled")) -> ()  [unwired: 2 in, 2 out]
      }
      frame #1 {
        w1098 = T5."Disabled and Grayed Out" ("Disabled")
        n666 = local write "R_Duration"(0.0 ("R_Duration")) -> ()
        n667 = local write "R_Target Thickness Value"(0.0 ("R_Target Thickness Value")) -> ()
        n668 = property on="R_Target Thickness Value" class="DigNum (strict)"("DisabledEnum"=T5."Disabled and Grayed Out" ("Disabled")) -> ()  [unwired: 2 in, 2 out]
        n669 = property on="R_Thickness Selection" class="RadioBtnsControl (strict)"("DisabledEnum"=w1098) -> ()  [unwired: 2 in, 2 out]
        n670 = property on="R_Duration" class="DigNum (strict)"("DisabledEnum"=w1098) -> ()  [unwired: 2 in, 2 out]
      }
    }
    n671 = case shown="False" w181 {
      frame #0 {
        n672 = local write "R Single RF Ramp down Time"(0.0 ("Target Clean Power")) -> ()
        n673 = property on="R Single RF Ramp down Time" class="DigNum (strict)"("DisabledEnum"=T5."Disabled and Grayed Out" ("Disabled")) -> ()  [unwired: 2 in, 2 out]
      }
      frame #1 {
        n674 = property on="R Single RF Ramp down Time" class="DigNum (strict)"("DisabledEnum"=T5."Enabled" ("Disabled")) -> ()  [unwired: 2 in, 2 out]
      }
    }
    n675 = case shown="\"Combination Sputter\"" w191 {
      frame #0 {
        n676 = local write "Recipe_selection tab"(0) -> ()
      }
      frame #1 {
        n677 = local write "Recipe_selection tab"(1) -> ()
      }
    }
    n678 = case shown="\"Other\"" w195 {
      frame #0 {
        n679 = local write "Web_selection_tab"(0) -> ()
      }
      frame #1 {
        n680 = local write "Web_selection_tab"(1) -> ()
      }
    }
    n681 = case shown="\"RF Sputter\"" w190 {
      frame #0 {
        n682 = local write "R_Single_Coating Type Selection_tab"(0) -> ()
      }
      frame #1 {
        n683 = local write "R_Single_Coating Type Selection_tab"(1) -> ()
      }
      frame #2 {
        n684 = local write "R_Single_Coating Type Selection_tab"(2) -> ()
      }
    }
    n685 = case shown="False" w182 {
      frame #0 {
        w1643 = T5."Disabled and Grayed Out" ("Disabled")
        w1642 = 0.0 ("Target Clean Power")
        n686 = local write "R Single RF  Step1 Coating Power"(w1642) -> ()
        n687 = local write "R Single RF Interval length"(w1642) -> ()
        n688 = property on="R Single RF  Step1 Coating Power" class="DigNum (strict)"("DisabledEnum"=w1643) -> ()  [unwired: 2 in, 2 out]
        n689 = property on="R Single RF Interval length" class="DigNum (strict)"("DisabledEnum"=w1643) -> ()  [unwired: 2 in, 2 out]
      }
      frame #1 {
        w1644 = T5."Enabled" ("Disabled")
        n690 = property on="R Single RF  Step1 Coating Power" class="DigNum (strict)"("DisabledEnum"=w1644) -> ()  [unwired: 2 in, 2 out]
        n691 = property on="R Single RF Interval length" class="DigNum (strict)"("DisabledEnum"=w1644) -> ()  [unwired: 2 in, 2 out]
      }
    }
    n692 = case shown="True" w180 {
      frame #0 {
        n693 = local write "R Single RF Ramp up Time"(0.0 ("Target Clean Power")) -> ()
        n694 = property on="R Single RF Ramp up Time" class="DigNum (strict)"("DisabledEnum"=T5."Disabled and Grayed Out" ("Disabled")) -> ()  [unwired: 2 in, 2 out]
      }
      frame #1 {
        n695 = property on="R Single RF Ramp up Time" class="DigNum (strict)"("DisabledEnum"=T5."Enabled" ("Disabled")) -> ()  [unwired: 2 in, 2 out]
      }
    }
    n696 = case shown="False" w183 {
      frame #0 {
        w1648 = 0.0 ("Ramp up Time")
        w1649 = T5."Disabled and Grayed Out" ("Disabled")
        n697 = local write "R Single DC Step1 Coating Power"(w1648) -> ()
        n698 = local write "R Single DC Interval length1"(w1648) -> ()
        n699 = property on="R Single DC Step1 Coating Power" class="DigNum (strict)"("DisabledEnum"=w1649) -> ()  [unwired: 2 in, 2 out]
        n700 = property on="R Single DC Interval length1" class="DigNum (strict)"("DisabledEnum"=w1649) -> ()  [unwired: 2 in, 2 out]
      }
      frame #1 {
        w1650 = T5."Enabled" ("Disabled")
        n701 = property on="R Single DC Interval length1" class="DigNum (strict)"("DisabledEnum"=w1650) -> ()  [unwired: 2 in, 2 out]
        n702 = property on="R Single DC Step1 Coating Power" class="DigNum (strict)"("DisabledEnum"=w1650) -> ()  [unwired: 2 in, 2 out]
      }
    }
    n703 = local read "R Single DC Interval length1"() -> (w144:dbl)
    n704 = Boolean To (0,1)(Boolean=w158) -> (0, 1=w157:i16)
    n705 = Boolean To (0,1)(Boolean=w166) -> (0, 1=w165:i16)
    n706 = Boolean To (0,1)(Boolean=w164) -> (0, 1=w163:i16)
    n707 = local read "R Single DC Interval length2"() -> (w143:dbl)
    n708 = Boolean To (0,1)(Boolean=w150) -> (0, 1=w156:i16)
    n709 = Boolean To (0,1)(Boolean=w149) -> (0, 1=w155:i16)
    n710 = Boolean To (0,1)(Boolean=w160) -> (0, 1=w159:i16)
    n711 = local read "R Single DC Interval length3"() -> (w142:dbl)
    n712 = Boolean To (0,1)(Boolean=w148) -> (0, 1=w154:i16)
    n713 = Boolean To (0,1)(Boolean=w147) -> (0, 1=w153:i16)
    n714 = local read "R Single DC Interval length4"() -> (w141:dbl)
    n715 = local read "R Single DC Interval length5"() -> (w140:dbl)
    n716 = Boolean To (0,1)(Boolean=w146) -> (0, 1=w152:i16)
    n717 = local read "R Single DC Interval length6"() -> (w139:dbl)
    n718 = local read "R Single DC Interval length8"() -> (w137:dbl)
    n719 = local read "R Single DC Interval length7"() -> (w138:dbl)
    n720 = Boolean To (0,1)(Boolean=w145) -> (0, 1=w151:i16)
    n721 = local read "R Single DC Interval length9"() -> (w136:dbl)
    n722 = local read "R Single DC Interval length10"() -> (w135:dbl)
    n723 = local read "R Single RF Interval length2"() -> (w105:dbl)
    n724 = local read "R Single RF Interval length3"() -> (w104:dbl)
    n725 = local read "R Single RF Interval length"() -> (w106:dbl)
    n726 = Boolean To (0,1)(Boolean=w115) -> (0, 1=w124:i16)
    n727 = local read "R Single RF Interval length4"() -> (w103:dbl)
    n728 = Boolean To (0,1)(Boolean=w112) -> (0, 1=w121:i16)
    n729 = Boolean To (0,1)(Boolean=w111) -> (0, 1=w120:i16)
    n730 = Boolean To (0,1)(Boolean=w110) -> (0, 1=w119:i16)
    n731 = Boolean To (0,1)(Boolean=w114) -> (0, 1=w123:i16)
    n732 = local read "R Single RF Interval length5"() -> (w102:dbl)
    n733 = local read "R Single RF Interval length8"() -> (w99:dbl)
    n734 = Boolean To (0,1)(Boolean=w113) -> (0, 1=w122:i16)
    n735 = Boolean To (0,1)(Boolean=w108) -> (0, 1=w117:i16)
    n736 = Boolean To (0,1)(Boolean=w109) -> (0, 1=w118:i16)
    n737 = local read "R Single RF Interval length7"() -> (w100:dbl)
    n738 = Boolean To (0,1)(Boolean=w107) -> (0, 1=w116:i16)
    n739 = local read "R Single RF Interval length10"() -> (w97:dbl)
    n740 = local read "R Single RF Interval length6"() -> (w101:dbl)
    n741 = Boolean To (0,1)(Boolean=w125) -> (0, 1=w126:i16)
    n742 = local read "R Single RF Interval length9"() -> (w98:dbl)
    n743 = Multiply(x=w165, y=w144) -> (x*y=w162:dbl)
    n744 = Multiply(x=w163, y=w143) -> (x*y=w161:dbl)
    n745 = Multiply(x=w159, y=w142) -> (x*y=w134:dbl)
    n746 = Multiply(x=w157, y=w141) -> (x*y=w133:dbl)
    n747 = Multiply(x=w156, y=w140) -> (x*y=w132:dbl)
    n748 = Multiply(x=w155, y=w139) -> (x*y=w130:dbl)
    n749 = Multiply(x=w154, y=w138) -> (x*y=w131:dbl)
    n750 = Multiply(x=w153, y=w137) -> (x*y=w129:dbl)
    n751 = Multiply(x=w124, y=w105) -> (x*y=w95:dbl)
    n752 = Multiply(x=w121, y=w102) -> (x*y=w92:dbl)
    n753 = Multiply(x=w120, y=w101) -> (x*y=w91:dbl)
    n754 = Multiply(x=w119, y=w100) -> (x*y=w90:dbl)
    n755 = Multiply(x=w123, y=w104) -> (x*y=w94:dbl)
    n756 = Multiply(x=w152, y=w136) -> (x*y=w128:dbl)
    n757 = Multiply(x=w122, y=w103) -> (x*y=w93:dbl)
    n758 = Multiply(x=w117, y=w98) -> (x*y=w88:dbl)
    n759 = Multiply(x=w118, y=w99) -> (x*y=w89:dbl)
    n760 = Multiply(x=w116, y=w97) -> (x*y=w87:dbl)
    n761 = Multiply(x=w151, y=w135) -> (x*y=w127:dbl)
    n762 = Multiply(x=w126, y=w106) -> (x*y=w96:dbl)
    n763 = local read "R_Simple_Coating Type Selection"() -> (w189:T2)
    n764 = local read "R_Simple_Coating Type Selection"() -> (w188:T2)
    n765 = Compound Arithmetic op=ADD(w162, w161, w134, w133, w132, w130, w131, w129, w128, w127) -> (→"Calculated_total_length_dc":dbl)
    n766 = Compound Arithmetic op=ADD(w96, w95, w94, w93, w92, w91, w90, w89, w88, w87) -> (→"Calculated_total_length_rf":dbl)
    n767 = local read "R Single DC Step9 Coating Power Active"() -> (w27:bool)
    n768 = local read "R Single DC Step8 Coating Power Active"() -> (w28:bool)
    n769 = local read "R Cmb Step1 Coating Power Active"() -> (w75:bool)
    n770 = local read "R_Simple_Coating Type Selection"() -> (w187:T2)
    n771 = local read "R_Recipe_type_selection"() -> (w186:enum32{"Single Recipe", "Combination Sputter"})
    n772 = Equal?(x=w189, y=0) -> (x = y?=w201:bool)
    n773 = Equal?(x=w187, y=2) -> (x = y?=w196:bool)
    n774 = Equal?(x=w188, y=1) -> (x = y?=w198:bool)
    n775 = local read "Thickness_Monitor_Active"() -> (w173:bool)
    n776 = local read "R Cmb Step2 Coating Power Active"() -> (w73:bool)
    n777 = local read "R Cmb Step3 Coating Power Active"() -> (w71:bool)
    n778 = local read "R Cmb Step4 Coating Power Active"() -> (w70:bool)
    n779 = local read "R Cmb Step5 Coating Power Active"() -> (w69:bool)
    n780 = local read "R Cmb Step6 Coating Power Active"() -> (w68:bool)
    n781 = local read "R Cmb Step7 Coating Power Active"() -> (w67:bool)
    n782 = local read "R Cmb Step8 Coating Power Active"() -> (w66:bool)
    n783 = local read "R Cmb Step9 Coating Power Active"() -> (w65:bool)
    n784 = local read "R Cmb Step10 Coating Power Active"() -> (w64:bool)
    n785 = local read "R Single RF Step6 Coating Power Active"() -> (w20:bool)
    n786 = local read "R Cmb Interval length 1"() -> (w74:dbl)
    n787 = Equal?(x=w186, y=1) -> (x = y?=w184:bool)
    n788 = case shown="True" w184 {
      frame #0 {
        w1651 = T5."Disabled and Grayed Out" ("Disabled")
        w1652 = 0.0 ("R Cmb Ch2 DC Ignition Power")
        w1653 = FALSE ("R Cmb Ch2 DC Target Clean Power Active")
        w1654 = ""
        n789 = local write "R Cmb Number of cycle"(w1652) -> ()
        n790 = local write "R Cmb Interval length 6"(w1652) -> ()
        n791 = local write "R Cmb Interval length 7"(w1652) -> ()
        n792 = local write "R Cmb Interval length 8"(w1652) -> ()
        n793 = local write "R Cmb Interval length 9"(w1652) -> ()
        n794 = local write "R Cmb Interval length 10"(w1652) -> ()
        n795 = local write "R Cmb Ch2 Step6 Coating Power"(w1652) -> ()
        n796 = local write "R Cmb Ch2 Step7 Coating Power"(w1652) -> ()
        n797 = local write "R Cmb Ch2 Step8 Coating Power"(w1652) -> ()
        n798 = local write "R Cmb Ch2 Step9 Coating Power"(w1652) -> ()
        n799 = local write "R Cmb Ch2 Step10 Coating Power"(w1652) -> ()
        n800 = local write "R Cmb Interval length 6"(w1652) -> ()
        n801 = local write "R Cmb Interval length 7"(w1652) -> ()
        n802 = local write "R Cmb Interval length 8"(w1652) -> ()
        n803 = local write "R Cmb Interval length 9"(w1652) -> ()
        n804 = local write "R Cmb Interval length 10"(w1652) -> ()
        n805 = local write "R Cmb Interval length 1"(w1652) -> ()
        n806 = local write "R Cmb Interval length 2"(w1652) -> ()
        n807 = local write "R Cmb Interval length 3"(w1652) -> ()
        n808 = local write "R Cmb Interval length 4"(w1652) -> ()
        n809 = local write "R Cmb Interval length 5"(w1652) -> ()
        n810 = local write "R Cmb Interval length 2"(w1652) -> ()
        n811 = local write "R Cmb Interval length 3"(w1652) -> ()
        n812 = local write "R Cmb Interval length 4"(w1652) -> ()
        n813 = local write "R Cmb Interval length 5"(w1652) -> ()
        n814 = local write "R Cmb Ch2 Step1 Coating Power"(w1652) -> ()
        n815 = local write "R Cmb Ch2 Step2 Coating Power"(w1652) -> ()
        n816 = local write "R Cmb Ch2 Step3 Coating Power"(w1652) -> ()
        n817 = local write "R Cmb Ch2 Step4 Coating Power"(w1652) -> ()
        n818 = local write "R Cmb Ch2 Step5 Coating Power"(w1652) -> ()
        n819 = local write "R Cmb Ch3 Step1 Coating Power"(w1652) -> ()
        n820 = local write "R Cmb Step6 Coating Power Active"(w1653) -> ()
        n821 = local write "R Cmb Step7 Coating Power Active"(w1653) -> ()
        n822 = local write "R Cmb Step8 Coating Power Active"(w1653) -> ()
        n823 = local write "R Cmb Step9 Coating Power Active"(w1653) -> ()
        n824 = local write "R Cmb Step10 Coating Power Active"(w1653) -> ()
        n825 = local write "R Cmb Step1 Coating Power Active"(w1653) -> ()
        n826 = local write "R Cmb Step2 Coating Power Active"(w1653) -> ()
        n827 = local write "R Cmb Step3 Coating Power Active"(w1653) -> ()
        n828 = local write "R Cmb Step4 Coating Power Active"(w1653) -> ()
        n829 = local write "R Cmb Step5 Coating Power Active"(w1653) -> ()
        n830 = local write "R Cmb Ch2 Target material"(w1654) -> ()
        n831 = local write "R Cmb Ch3 Target material"(w1654) -> ()
        n832 = property on="R Cmb Number of cycle" class="DigNum (strict)"("DisabledEnum"=w1651) -> ()  [unwired: 2 in, 2 out]
        n833 = property on="R Cmb Ch2 Step1 Coating Power" class="DigNum (strict)"("DisabledEnum"=w1651) -> ()  [unwired: 2 in, 2 out]
        n834 = property on="R Cmb Ch2 Step2 Coating Power" class="DigNum (strict)"("DisabledEnum"=w1651) -> ()  [unwired: 2 in, 2 out]
        n835 = property on="R Cmb Ch2 Step3 Coating Power" class="DigNum (strict)"("DisabledEnum"=w1651) -> ()  [unwired: 2 in, 2 out]
        n836 = property on="R Cmb Ch2 Step4 Coating Power" class="DigNum (strict)"("DisabledEnum"=w1651) -> ()  [unwired: 2 in, 2 out]
        n837 = property on="R Cmb Ch2 Step5 Coating Power" class="DigNum (strict)"("DisabledEnum"=w1651) -> ()  [unwired: 2 in, 2 out]
        n838 = property on="R Cmb Ch2 Step6 Coating Power" class="DigNum (strict)"("DisabledEnum"=w1651) -> ()  [unwired: 2 in, 2 out]
        n839 = property on="R Cmb Ch2 Step7 Coating Power" class="DigNum (strict)"("DisabledEnum"=w1651) -> ()  [unwired: 2 in, 2 out]
        n840 = property on="R Cmb Ch2 Step8 Coating Power" class="DigNum (strict)"("DisabledEnum"=w1651) -> ()  [unwired: 2 in, 2 out]
        n841 = property on="R Cmb Ch2 Step9 Coating Power" class="DigNum (strict)"("DisabledEnum"=w1651) -> ()  [unwired: 2 in, 2 out]
        n842 = property on="R Cmb Ch2 Step10 Coating Power" class="DigNum (strict)"("DisabledEnum"=w1651) -> ()  [unwired: 2 in, 2 out]
        n843 = property on="R Cmb Ch3 Step1 Coating Power" class="DigNum (strict)"("DisabledEnum"=w1651) -> ()  [unwired: 2 in, 2 out]
        n844 = property on="R Cmb Ch3 Step2 Coating Power" class="DigNum (strict)"("DisabledEnum"=w1651) -> ()  [unwired: 2 in, 2 out]
        n845 = property on="R Cmb Ch3 Step3 Coating Power" class="DigNum (strict)"("DisabledEnum"=w1651) -> ()  [unwired: 2 in, 2 out]
        n846 = property on="R Cmb Ch3 Step4 Coating Power" class="DigNum (strict)"("DisabledEnum"=w1651) -> ()  [unwired: 2 in, 2 out]
        n847 = property on="R Cmb Ch3 Step5 Coating Power" class="DigNum (strict)"("DisabledEnum"=w1651) -> ()  [unwired: 2 in, 2 out]
        n848 = property on="R Cmb Ch3 Step6 Coating Power" class="DigNum (strict)"("DisabledEnum"=w1651) -> ()  [unwired: 2 in, 2 out]
        n849 = property on="R Cmb Ch3 Step7 Coating Power" class="DigNum (strict)"("DisabledEnum"=w1651) -> ()  [unwired: 2 in, 2 out]
        n850 = property on="R Cmb Ch3 Step8 Coating Power" class="DigNum (strict)"("DisabledEnum"=w1651) -> ()  [unwired: 2 in, 2 out]
        n851 = property on="R Cmb Ch3 Step9 Coating Power" class="DigNum (strict)"("DisabledEnum"=w1651) -> ()  [unwired: 2 in, 2 out]
        n852 = property on="R Cmb Ch3 Step10 Coating Power" class="DigNum (strict)"("DisabledEnum"=w1651) -> ()  [unwired: 2 in, 2 out]
        n853 = property on="R Cmb Interval length 10" class="DigNum (strict)"("DisabledEnum"=w1651) -> ()  [unwired: 2 in, 2 out]
        n854 = property on="R Cmb Interval length 6" class="DigNum (strict)"("DisabledEnum"=w1651) -> ()  [unwired: 2 in, 2 out]
        n855 = property on="R Cmb Interval length 7" class="DigNum (strict)"("DisabledEnum"=w1651) -> ()  [unwired: 2 in, 2 out]
        n856 = property on="R Cmb Interval length 8" class="DigNum (strict)"("DisabledEnum"=w1651) -> ()  [unwired: 2 in, 2 out]
        n857 = property on="R Cmb Interval length 9" class="DigNum (strict)"("DisabledEnum"=w1651) -> ()  [unwired: 2 in, 2 out]
        n858 = property on="R Cmb Interval length 1" class="DigNum (strict)"("DisabledEnum"=w1651) -> ()  [unwired: 2 in, 2 out]
        n859 = property on="R Cmb Interval length 2" class="DigNum (strict)"("DisabledEnum"=w1651) -> ()  [unwired: 2 in, 2 out]
        n860 = property on="R Cmb Interval length 3" class="DigNum (strict)"("DisabledEnum"=w1651) -> ()  [unwired: 2 in, 2 out]
        n861 = property on="R Cmb Interval length 4" class="DigNum (strict)"("DisabledEnum"=w1651) -> ()  [unwired: 2 in, 2 out]
        n862 = property on="R Cmb Interval length 5" class="DigNum (strict)"("DisabledEnum"=w1651) -> ()  [unwired: 2 in, 2 out]
      }
      frame #1 {
        w1656 = T5."Disabled and Grayed Out" ("Disabled")
        n863 = property on="R Single DC Interval length1" class="DigNum (strict)"("DisabledEnum"=w1656) -> ()  [unwired: 2 in, 2 out]
        n864 = property on="R Single DC Step1 Coating Power" class="DigNum (strict)"("DisabledEnum"=w1656) -> ()  [unwired: 2 in, 2 out]
        n865 = property on="R Cmb Number of cycle" class="DigNum (strict)"("DisabledEnum"=T5."Enabled" ("Disabled")) -> ()  [unwired: 2 in, 2 out]
        n866 = local write "R Single DC Step1 Coating Power Active"(FALSE ("R Single DC Step1 Coating Power Active")) -> ()
        n867 = local write "R Cmb Step1 Coating Power Active"(TRUE ("R Cmb Ch2 Step1 Coating Power Active")) -> ()
        n868 = property on="R Single DC Target material" class="Str"("DisabledEnum"=T5."Disabled and Grayed Out" ("Disabled")) -> ()  [unwired: 2 in, 2 out]
      }
    }
    n869 = case shown="True" w196 {
      frame #0 {
        w1681 = T5."Disabled and Grayed Out" ("Disabled")
        w1680 = 0.0 ("R DC Ignition Power")
        w1679 = FALSE ("R DC Target Clean")
        n870 = local write "R Single RF Interval length10"(w1680) -> ()
        n871 = local write "R Single RF Interval length"(w1680) -> ()
        n872 = local write "R Single RF Ramp up Time"(w1680) -> ()
        n873 = local write "R Single RF  Step1 Coating Power"(w1680) -> ()
        n874 = local write "R Single RF Step2 Coating Power"(w1680) -> ()
        n875 = local write "R Single RF Step3 Coating Power"(w1680) -> ()
        n876 = local write "R Single RF Step4 Coating Power"(w1680) -> ()
        n877 = local write "R Single RF Step5 Coating Power"(w1680) -> ()
        n878 = local write "R Single RF Ramp down Time"(w1680) -> ()
        n879 = local write "R Single RF Interval length9"(w1680) -> ()
        n880 = local write "R Single RF Interval length6"(w1680) -> ()
        n881 = local write "R Single RF Target material"("") -> ()
        n882 = local write "R Single RF Ramp up"(w1679) -> ()
        n883 = local write "R Single RF Ramp down"(w1679) -> ()
        n884 = local write "R Single RF Step1 Coating Power Active"(w1679) -> ()
        n885 = local write "R Single RF Step2 Coating Power Active"(w1679) -> ()
        n886 = local write "R Single RF Step3 Coating Power Active"(w1679) -> ()
        n887 = local write "R Single RF Step4 Coating Power Active"(w1679) -> ()
        n888 = local write "R Single RF Step5 Coating Power Active"(w1679) -> ()
        n889 = local write "R Single RF Interval length8"(w1680) -> ()
        n890 = local write "R Single RF Interval length7"(w1680) -> ()
        n891 = local write "R Single RF Step6 Coating Power"(w1680) -> ()
        n892 = local write "R Single RF Step7 Coating Power"(w1680) -> ()
        n893 = local write "R Single RF Step8 Coating Power"(w1680) -> ()
        n894 = local write "R Single RF Step9 Coating Power"(w1680) -> ()
        n895 = local write "R Single RF Step10 Coating Power"(w1680) -> ()
        n896 = local write "R Single RF Interval length2"(w1680) -> ()
        n897 = local write "R Single RF Interval length3"(w1680) -> ()
        n898 = local write "R Single RF Interval length4"(w1680) -> ()
        n899 = local write "R Single RF Interval length5"(w1680) -> ()
        n900 = local write "R Single RF Step6 Coating Power Active"(w1679) -> ()
        n901 = local write "R Single RF Step7 Coating Power Active"(w1679) -> ()
        n902 = local write "R Single RF Step8 Coating Power Active"(w1679) -> ()
        n903 = local write "R Single RF Step9 Coating Power Active"(w1679) -> ()
        n904 = local write "R Single RF Step10 Coating Power Active"(w1679) -> ()
        n905 = property on="R Single RF Interval length" class="DigNum (strict)"("DisabledEnum"=w1681) -> ()  [unwired: 2 in, 2 out]
        n906 = property on="R Single RF Step6 Coating Power" class="DigNum (strict)"("DisabledEnum"=w1681) -> ()  [unwired: 2 in, 2 out]
        n907 = property on="R Single RF Step7 Coating Power" class="DigNum (strict)"("DisabledEnum"=w1681) -> ()  [unwired: 2 in, 2 out]
        n908 = property on="R Single RF Step8 Coating Power" class="DigNum (strict)"("DisabledEnum"=w1681) -> ()  [unwired: 2 in, 2 out]
        n909 = property on="R Single RF Step9 Coating Power" class="DigNum (strict)"("DisabledEnum"=w1681) -> ()  [unwired: 2 in, 2 out]
        n910 = property on="R Single RF Step10 Coating Power" class="DigNum (strict)"("DisabledEnum"=w1681) -> ()  [unwired: 2 in, 2 out]
        n911 = property on="R Single RF Interval length2" class="DigNum (strict)"("DisabledEnum"=w1681) -> ()  [unwired: 2 in, 2 out]
        n912 = property on="R Single RF Interval length3" class="DigNum (strict)"("DisabledEnum"=w1681) -> ()  [unwired: 2 in, 2 out]
        n913 = property on="R Single RF Interval length4" class="DigNum (strict)"("DisabledEnum"=w1681) -> ()  [unwired: 2 in, 2 out]
        n914 = property on="R Single RF Interval length5" class="DigNum (strict)"("DisabledEnum"=w1681) -> ()  [unwired: 2 in, 2 out]
        n915 = property on="R Single RF Interval length6" class="DigNum (strict)"("DisabledEnum"=w1681) -> ()  [unwired: 2 in, 2 out]
        n916 = property on="R Single RF Ramp up Time" class="DigNum (strict)"("DisabledEnum"=w1681) -> ()  [unwired: 2 in, 2 out]
        n917 = property on="R Single RF  Step1 Coating Power" class="DigNum (strict)"("DisabledEnum"=w1681) -> ()  [unwired: 2 in, 2 out]
        n918 = property on="R Single RF Step2 Coating Power" class="DigNum (strict)"("DisabledEnum"=w1681) -> ()  [unwired: 2 in, 2 out]
        n919 = property on="R Single RF Step3 Coating Power" class="DigNum (strict)"("DisabledEnum"=w1681) -> ()  [unwired: 2 in, 2 out]
        n920 = property on="R Single RF Step4 Coating Power" class="DigNum (strict)"("DisabledEnum"=w1681) -> ()  [unwired: 2 in, 2 out]
        n921 = property on="R Single RF Step5 Coating Power" class="DigNum (strict)"("DisabledEnum"=w1681) -> ()  [unwired: 2 in, 2 out]
        n922 = property on="R Single RF Ramp down Time" class="DigNum (strict)"("DisabledEnum"=w1681) -> ()  [unwired: 2 in, 2 out]
        n923 = property on="R Single RF Interval length10" class="DigNum (strict)"("DisabledEnum"=w1681) -> ()  [unwired: 2 in, 2 out]
        n924 = property on="R Single RF Interval length9" class="DigNum (strict)"("DisabledEnum"=w1681) -> ()  [unwired: 2 in, 2 out]
        n925 = property on="R Single RF Interval length7" class="DigNum (strict)"("DisabledEnum"=w1681) -> ()  [unwired: 2 in, 2 out]
        n926 = property on="R Single RF Interval length8" class="DigNum (strict)"("DisabledEnum"=w1681) -> ()  [unwired: 2 in, 2 out]
      }
      frame #1 {
        n927 = local write "R Single RF Step1 Coating Power Active"(TRUE ("R Single RF Step1 Coating Power Active")) -> ()
        n928 = local write "R Set Pressure mtorr"(0.001 ("R Set Pressure mtorr")) -> ()
        n929 = property on="Tab Control 2" class="TabCtl (strict)"("Visible"=FALSE) -> ()  [unwired: 2 in, 2 out]
        n930 = property on="Tab Control" class="TabCtl (strict)"("Visible"=TRUE) -> ()  [unwired: 2 in, 2 out]
      }
    }
    n931 = local read "R Single DC Step5 Coating Power Active"() -> (w31:bool)
    n932 = case shown="True" w201 {
      frame #0 {
        w1687 = 0.0 ("R_Microwave Power")
        w1688 = T5."Enabled" ("Disabled")
        n933 = property on="R Argon Flow sccm" class="DigNum (strict)"("DisabledEnum"=w1688) -> ()  [unwired: 2 in, 2 out]
        n934 = property on="R Set Pressure mtorr" class="DigNum (strict)"("DisabledEnum"=w1688) -> ()  [unwired: 2 in, 2 out]
        n935 = local write "R_Single Microwave Power"(w1687) -> ()
        n936 = local write "R_Single Microwave Time"(w1687) -> ()
        n937 = property on="R_Single Microwave Power" class="DigNum (strict)"("DisabledEnum"=T5."Disabled and Grayed Out" ("Disabled")) -> ()  [unwired: 2 in, 2 out]
        n938 = local write "R Single Pass Number"(w1687) -> ()
      }
      frame #1 {
        n939 = property on="R Set Pressure mtorr" class="DigNum (strict)"("DisabledEnum"=T5."Disabled and Grayed Out" ("Disabled")) -> ()  [unwired: 2 in, 2 out]
        n940 = local write "R Argon Flow sccm"(200.0 ("R Argon Flow sccm")) -> ()
        n941 = property on="R_Single Microwave Power" class="DigNum (strict)"("DisabledEnum"=T5."Enabled" ("Disabled")) -> ()  [unwired: 2 in, 2 out]
        n942 = local read "R Single Pass Number"() -> (w1698:dbl)
        n943 = property on="Tab Control" class="TabCtl (strict)"("Visible"=FALSE) -> ()  [unwired: 2 in, 2 out]
        n944 = Less Or Equal?(x=w1698, y=1.5) -> (x <= y?=w1696:bool)
        n945 = local write "R Set Pressure mtorr"(0.0 ("R Set Pressure mtorr")) -> ()
        n946 = Select(t=1, s=w1696, f=2) -> (s? t:f=w1693:i32)
        n947 = property on="Tab Control 2" class="TabCtl (strict)"("Visible"=TRUE) -> ()  [unwired: 2 in, 2 out]
        n948 = local write "R Single Pass Number"(w1693) -> ()
      }
    }
    n949 = case shown="True" w198 {
      frame #0 {
        w1672 = T5."Disabled and Grayed Out" ("Disabled")
        w1673 = 0.0 ("R DC Ignition Power")
        w1674 = FALSE ("R DC Target Clean")
        n950 = local write "R Single DC Step1 Coating Power Active"(w1674) -> ()
        n951 = local write "R Single DC Step2 Coating Power Active"(w1674) -> ()
        n952 = local write "R Single DC Step3 Coating Power Active"(w1674) -> ()
        n953 = local write "R Single DC Step4 Coating Power Active"(w1674) -> ()
        n954 = local write "R Single DC Step5 Coating Power Active"(w1674) -> ()
        n955 = local write "R Single DC Step6 Coating Power Active"(w1674) -> ()
        n956 = local write "R Single DC Step7 Coating Power Active"(w1674) -> ()
        n957 = local write "R Single DC Step8 Coating Power Active"(w1674) -> ()
        n958 = local write "R Single DC Step9 Coating Power Active"(w1674) -> ()
        n959 = local write "R Single DC Step10 Coating Power Active"(w1674) -> ()
        n960 = local write "R_Single DC_Material ok"(w1674) -> ()
        n961 = local write "R Single DC Target material"("") -> ()
        n962 = local write "R Single DC Interval length1"(w1673) -> ()
        n963 = local write "R Single DC Step1 Coating Power"(w1673) -> ()
        n964 = local write "R Single DC Step2 Coating Power"(w1673) -> ()
        n965 = local write "R Single DC Step3 Coating Power"(w1673) -> ()
        n966 = local write "R Single DC Step4 Coating Power"(w1673) -> ()
        n967 = local write "R Single DC Step5 Coating Power"(w1673) -> ()
        n968 = local write "R Single DC Interval length2"(w1673) -> ()
        n969 = local write "R Single DC Interval length3"(w1673) -> ()
        n970 = local write "R Single DC Interval length4"(w1673) -> ()
        n971 = local write "R Single DC Interval length5"(w1673) -> ()
        n972 = local write "R Single DC Interval length6"(w1673) -> ()
        n973 = local write "R Single DC Interval length7"(w1673) -> ()
        n974 = local write "R Single DC Interval length8"(w1673) -> ()
        n975 = local write "R Single DC Interval length9"(w1673) -> ()
        n976 = local write "R Single DC Interval length10"(w1673) -> ()
        n977 = property on="R Single DC Step6 Coating Power" class="DigNum (strict)"("DisabledEnum"=w1672) -> ()  [unwired: 2 in, 2 out]
        n978 = property on="R Single DC Step7 Coating Power" class="DigNum (strict)"("DisabledEnum"=w1672) -> ()  [unwired: 2 in, 2 out]
        n979 = property on="R Single DC Interval length6" class="DigNum (strict)"("DisabledEnum"=w1672) -> ()  [unwired: 2 in, 2 out]
        n980 = property on="R Single DC Step1 Coating Power" class="DigNum (strict)"("DisabledEnum"=w1672) -> ()  [unwired: 2 in, 2 out]
        n981 = property on="R Single DC Step2 Coating Power" class="DigNum (strict)"("DisabledEnum"=w1672) -> ()  [unwired: 2 in, 2 out]
        n982 = property on="R Single DC Step3 Coating Power" class="DigNum (strict)"("DisabledEnum"=w1672) -> ()  [unwired: 2 in, 2 out]
        n983 = property on="R Single DC Step4 Coating Power" class="DigNum (strict)"("DisabledEnum"=w1672) -> ()  [unwired: 2 in, 2 out]
        n984 = property on="R Single DC Step5 Coating Power" class="DigNum (strict)"("DisabledEnum"=w1672) -> ()  [unwired: 2 in, 2 out]
        n985 = property on="R Single DC Interval length1" class="DigNum (strict)"("DisabledEnum"=w1672) -> ()  [unwired: 2 in, 2 out]
        n986 = property on="R Single DC Step8 Coating Power" class="DigNum (strict)"("DisabledEnum"=w1672) -> ()  [unwired: 2 in, 2 out]
        n987 = property on="R Single DC Step9 Coating Power" class="DigNum (strict)"("DisabledEnum"=w1672) -> ()  [unwired: 2 in, 2 out]
        n988 = property on="R Single DC Step10 Coating Power" class="DigNum (strict)"("DisabledEnum"=w1672) -> ()  [unwired: 2 in, 2 out]
        n989 = property on="R Single DC Interval length2" class="DigNum (strict)"("DisabledEnum"=w1672) -> ()  [unwired: 2 in, 2 out]
        n990 = property on="R Single DC Interval length3" class="DigNum (strict)"("DisabledEnum"=w1672) -> ()  [unwired: 2 in, 2 out]
        n991 = property on="R Single DC Interval length4" class="DigNum (strict)"("DisabledEnum"=w1672) -> ()  [unwired: 2 in, 2 out]
        n992 = property on="R Single DC Interval length5" class="DigNum (strict)"("DisabledEnum"=w1672) -> ()  [unwired: 2 in, 2 out]
        n993 = property on="R Single DC Interval length7" class="DigNum (strict)"("DisabledEnum"=w1672) -> ()  [unwired: 2 in, 2 out]
        n994 = property on="R Single DC Interval length6" class="DigNum (strict)"("DisabledEnum"=w1672) -> ()  [unwired: 2 in, 2 out]
        n995 = property on="R Single DC Interval length8" class="DigNum (strict)"("DisabledEnum"=w1672) -> ()  [unwired: 2 in, 2 out]
        n996 = property on="R Single DC Interval length9" class="DigNum (strict)"("DisabledEnum"=w1672) -> ()  [unwired: 2 in, 2 out]
        n997 = property on="R Single DC Interval length10" class="DigNum (strict)"("DisabledEnum"=w1672) -> ()  [unwired: 2 in, 2 out]
      }
      frame #1 {
        n998 = local write "R Single DC Step1 Coating Power Active"(TRUE ("R Single DC Step1 Coating Power Active")) -> ()
        n999 = local write "R Set Pressure mtorr"(0.004 ("R Set Pressure mtorr")) -> ()
        n1000 = property on="Tab Control" class="TabCtl (strict)"("Visible"=TRUE) -> ()  [unwired: 2 in, 2 out]
      }
    }
    n1001 = local read "R Single RF Step7 Coating Power Active"() -> (w19:bool)
    n1002 = local read "R Single DC Step6 Coating Power Active"() -> (w30:bool)
    n1003 = stacked-sequence {
      frame #0 {
      }
    }
    n1004 = Boolean To (0,1)(Boolean=w75) -> (0, 1=w85:i16)
    n1005 = case shown="False" w27 {
      frame #0 {
        n1006 = local write "R Single DC Step10 Coating Power Active"(FALSE ("R Single DC Step8 Coating Power Active")) -> ()
      }
      frame #1 {
        n1007 = local read "R Single DC Step10 Coating Power Active"() -> (w303:bool)
        n1008 = case shown="False" w303 {
          frame #0 {
            w304 = 0.0 ("R Single DC Step10 Coating Power")
            w305 = T5."Disabled and Grayed Out" ("Disabled")
            n1009 = local write "R Single DC Step10 Coating Power"(w304) -> ()
            n1010 = local write "R Single DC Interval length10"(w304) -> ()
            n1011 = property on="R Single DC Step10 Coating Power" class="DigNum (strict)"("DisabledEnum"=w305) -> ()  [unwired: 2 in, 2 out]
            n1012 = property on="R Single DC Interval length10" class="DigNum (strict)"("DisabledEnum"=w305) -> ()  [unwired: 2 in, 2 out]
          }
          frame #1 {
            w306 = T5."Enabled" ("Disabled")
            n1013 = property on="R Single DC Step10 Coating Power" class="DigNum (strict)"("DisabledEnum"=w306) -> ()  [unwired: 2 in, 2 out]
            n1014 = property on="R Single DC Interval length10" class="DigNum (strict)"("DisabledEnum"=w306) -> ()  [unwired: 2 in, 2 out]
          }
        }
      }
    }
    n1015 = case shown="False" w28 {
      frame #0 {
        w307 = FALSE ("R Single DC Step8 Coating Power Active")
        n1016 = local write "R Single DC Step10 Coating Power Active"(w307) -> ()
        n1017 = local write "R Single DC Step9 Coating Power Active"(w307) -> ()
      }
      frame #1 {
        n1018 = local read "R Single DC Step9 Coating Power Active"() -> (w308:bool)
        n1019 = case shown="False" w308 {
          frame #0 {
            w309 = 0.0 ("R Single DC Step9 Coating Power")
            w310 = T5."Disabled and Grayed Out" ("Disabled")
            n1020 = property on="R Single DC Step9 Coating Power" class="DigNum (strict)"("DisabledEnum"=w310) -> ()  [unwired: 2 in, 2 out]
            n1021 = property on="R Single DC Interval length9" class="DigNum (strict)"("DisabledEnum"=w310) -> ()  [unwired: 2 in, 2 out]
            n1022 = local write "R Single DC Step9 Coating Power"(w309) -> ()
            n1023 = local write "R Single DC Interval length9"(w309) -> ()
          }
          frame #1 {
            w311 = T5."Enabled" ("Disabled")
            n1024 = property on="R Single DC Interval length9" class="DigNum (strict)"("DisabledEnum"=w311) -> ()  [unwired: 2 in, 2 out]
            n1025 = property on="R Single DC Step9 Coating Power" class="DigNum (strict)"("DisabledEnum"=w311) -> ()  [unwired: 2 in, 2 out]
          }
        }
      }
    }
    n1026 = local read "R Cmb Interval length 9"() -> (w57:dbl)
    n1027 = local read "R Cmb Interval length 3"() -> (w63:dbl)
    n1028 = local read "R Cmb Interval length 4"() -> (w62:dbl)
    n1029 = local read "R Cmb Interval length 10"() -> (w56:dbl)
    n1030 = local read "R Cmb Interval length 2"() -> (w72:dbl)
    n1031 = local read "R Cmb Interval length 5"() -> (w61:dbl)
    n1032 = case shown="True" w173 {
      frame #0 {
        w1136 = T5."Disabled and Grayed Out" ("Disabled")
        n1033 = property on="R Material_density" class="DigNum (strict)"("DisabledEnum"=w1136) -> ()  [unwired: 2 in, 2 out]
        n1034 = property on="R Z_factor" class="DigNum (strict)"("DisabledEnum"=w1136) -> ()  [unwired: 2 in, 2 out]
        n1035 = property on="R Toooling_factor" class="DigNum (strict)"("DisabledEnum"=w1136) -> ()  [unwired: 2 in, 2 out]
      }
      frame #1 {
        w1137 = T5."Enabled" ("Disabled")
        n1036 = property on="R Material_density" class="DigNum (strict)"("DisabledEnum"=w1137) -> ()  [unwired: 2 in, 2 out]
        n1037 = property on="R Z_factor" class="DigNum (strict)"("DisabledEnum"=w1137) -> ()  [unwired: 2 in, 2 out]
        n1038 = property on="R Toooling_factor" class="DigNum (strict)"("DisabledEnum"=w1137) -> ()  [unwired: 2 in, 2 out]
      }
    }
    n1039 = local read "R Cmb Interval length 6"() -> (w59:dbl)
    n1040 = local read "R Cmb Interval length 8"() -> (w58:dbl)
    n1041 = local read "R Cmb Interval length 7"() -> (w60:dbl)
    n1042 = Multiply(x=w85, y=w74) -> (x*y=w54:dbl)
    n1043 = local read "R Single DC Step7 Coating Power Active"() -> (w29:bool)
    n1044 = Boolean To (0,1)(Boolean=w73) -> (0, 1=w84:i16)
    n1045 = Boolean To (0,1)(Boolean=w71) -> (0, 1=w83:i16)
    n1046 = Boolean To (0,1)(Boolean=w70) -> (0, 1=w82:i16)
    n1047 = Boolean To (0,1)(Boolean=w68) -> (0, 1=w80:i16)
    n1048 = Boolean To (0,1)(Boolean=w66) -> (0, 1=w78:i16)
    n1049 = Boolean To (0,1)(Boolean=w69) -> (0, 1=w81:i16)
    n1050 = Boolean To (0,1)(Boolean=w65) -> (0, 1=w77:i16)
    n1051 = Boolean To (0,1)(Boolean=w64) -> (0, 1=w76:i16)
    n1052 = Boolean To (0,1)(Boolean=w67) -> (0, 1=w79:i16)
    n1053 = case shown="False" w20 {
      frame #0 {
        w268 = FALSE ("R Single RF Step3 Coating Power Active")
        n1054 = local write "R Single RF Step7 Coating Power Active"(w268) -> ()
        n1055 = local write "R Single RF Step8 Coating Power Active"(w268) -> ()
        n1056 = local write "R Single RF Step9 Coating Power Active"(w268) -> ()
        n1057 = local write "R Single RF Step10 Coating Power Active"(w268) -> ()
      }
      frame #1 {
        n1058 = local read "R Single RF Step7 Coating Power Active"() -> (w269:bool)
        n1059 = case shown="False" w269 {
          frame #0 {
            w270 = 0.0 ("Target Clean Power")
            w271 = T5."Disabled and Grayed Out" ("Disabled")
            n1060 = local write "R Single RF Step7 Coating Power"(w270) -> ()
            n1061 = local write "R Single RF Interval length7"(w270) -> ()
            n1062 = property on="R Single RF Step7 Coating Power" class="DigNum (strict)"("DisabledEnum"=w271) -> ()  [unwired: 2 in, 2 out]
            n1063 = property on="R Single RF Interval length7" class="DigNum (strict)"("DisabledEnum"=w271) -> ()  [unwired: 2 in, 2 out]
          }
          frame #1 {
            w272 = T5."Enabled" ("Disabled")
            n1064 = property on="R Single RF Step7 Coating Power" class="DigNum (strict)"("DisabledEnum"=w272) -> ()  [unwired: 2 in, 2 out]
            n1065 = property on="R Single RF Interval length7" class="DigNum (strict)"("DisabledEnum"=w272) -> ()  [unwired: 2 in, 2 out]
          }
        }
      }
    }
    n1066 = Multiply(x=w84, y=w72) -> (x*y=w53:dbl)
    n1067 = Multiply(x=w83, y=w63) -> (x*y=w52:dbl)
    n1068 = Multiply(x=w82, y=w62) -> (x*y=w51:dbl)
    n1069 = case shown="False" w19 {
      frame #0 {
        w263 = FALSE ("R Single RF Step3 Coating Power Active")
        n1070 = local write "R Single RF Step8 Coating Power Active"(w263) -> ()
        n1071 = local write "R Single RF Step9 Coating Power Active"(w263) -> ()
        n1072 = local write "R Single RF Step10 Coating Power Active"(w263) -> ()
      }
      frame #1 {
        n1073 = local read "R Single RF Step8 Coating Power Active"() -> (w264:bool)
        n1074 = case shown="False" w264 {
          frame #0 {
            w265 = 0.0 ("Target Clean Power")
            w266 = T5."Disabled and Grayed Out" ("Disabled")
            n1075 = local write "R Single RF Step8 Coating Power"(w265) -> ()
            n1076 = local write "R Single RF Interval length8"(w265) -> ()
            n1077 = property on="R Single RF Step8 Coating Power" class="DigNum (strict)"("DisabledEnum"=w266) -> ()  [unwired: 2 in, 2 out]
            n1078 = property on="R Single RF Interval length8" class="DigNum (strict)"("DisabledEnum"=w266) -> ()  [unwired: 2 in, 2 out]
          }
          frame #1 {
            w267 = T5."Enabled" ("Disabled")
            n1079 = property on="R Single RF Step8 Coating Power" class="DigNum (strict)"("DisabledEnum"=w267) -> ()  [unwired: 2 in, 2 out]
            n1080 = property on="R Single RF Interval length8" class="DigNum (strict)"("DisabledEnum"=w267) -> ()  [unwired: 2 in, 2 out]
          }
        }
      }
    }
    n1081 = Multiply(x=w80, y=w59) -> (x*y=w49:dbl)
    n1082 = Multiply(x=w78, y=w58) -> (x*y=w47:dbl)
    n1083 = Multiply(x=w81, y=w61) -> (x*y=w50:dbl)
    n1084 = Multiply(x=w77, y=w57) -> (x*y=w46:dbl)
    n1085 = case shown="False" w31 {
      frame #0 {
        w322 = FALSE ("R Single DC Step8 Coating Power Active")
        n1086 = local write "R Single DC Step7 Coating Power Active"(w322) -> ()
        n1087 = local write "R Single DC Step8 Coating Power Active"(w322) -> ()
        n1088 = local write "R Single DC Step9 Coating Power Active"(w322) -> ()
        n1089 = local write "R Single DC Step10 Coating Power Active"(w322) -> ()
        n1090 = local write "R Single DC Step6 Coating Power Active"(w322) -> ()
      }
      frame #1 {
        n1091 = local read "R Single DC Step6 Coating Power Active"() -> (w323:bool)
        n1092 = case shown="False" w323 {
          frame #0 {
            w324 = 0.0 ("Target Clean Power")
            w325 = T5."Disabled and Grayed Out" ("Disabled")
            n1093 = local write "R Single DC Step6 Coating Power"(w324) -> ()
            n1094 = local write "R Single DC Interval length6"(w324) -> ()
            n1095 = property on="R Single DC Step6 Coating Power" class="DigNum (strict)"("DisabledEnum"=w325) -> ()  [unwired: 2 in, 2 out]
            n1096 = property on="R Single DC Interval length6" class="DigNum (strict)"("DisabledEnum"=w325) -> ()  [unwired: 2 in, 2 out]
          }
          frame #1 {
            w326 = T5."Enabled" ("Disabled")
            n1097 = property on="R Single DC Step6 Coating Power" class="DigNum (strict)"("DisabledEnum"=w326) -> ()  [unwired: 2 in, 2 out]
            n1098 = property on="R Single DC Interval length6" class="DigNum (strict)"("DisabledEnum"=w326) -> ()  [unwired: 2 in, 2 out]
          }
        }
      }
    }
    n1099 = Multiply(x=w76, y=w56) -> (x*y=w45:dbl)
    n1100 = Multiply(x=w79, y=w60) -> (x*y=w48:dbl)
    n1101 = case shown="False" w30 {
      frame #0 {
        w317 = FALSE ("R Single DC Step8 Coating Power Active")
        n1102 = local write "R Single DC Step10 Coating Power Active"(w317) -> ()
        n1103 = local write "R Single DC Step9 Coating Power Active"(w317) -> ()
        n1104 = local write "R Single DC Step8 Coating Power Active"(w317) -> ()
        n1105 = local write "R Single DC Step7 Coating Power Active"(w317) -> ()
      }
      frame #1 {
        n1106 = local read "R Single DC Step7 Coating Power Active"() -> (w318:bool)
        n1107 = case shown="False" w318 {
          frame #0 {
            w319 = 0.0 ("Target Clean Power")
            w320 = T5."Disabled and Grayed Out" ("Disabled")
            n1108 = local write "R Single DC Step7 Coating Power"(w319) -> ()
            n1109 = local write "R Single DC Interval length7"(w319) -> ()
            n1110 = property on="R Single DC Step7 Coating Power" class="DigNum (strict)"("DisabledEnum"=w320) -> ()  [unwired: 2 in, 2 out]
            n1111 = property on="R Single DC Interval length7" class="DigNum (strict)"("DisabledEnum"=w320) -> ()  [unwired: 2 in, 2 out]
          }
          frame #1 {
            w321 = T5."Enabled" ("Disabled")
            n1112 = property on="R Single DC Step7 Coating Power" class="DigNum (strict)"("DisabledEnum"=w321) -> ()  [unwired: 2 in, 2 out]
            n1113 = property on="R Single DC Interval length7" class="DigNum (strict)"("DisabledEnum"=w321) -> ()  [unwired: 2 in, 2 out]
          }
        }
      }
    }
    n1114 = Compound Arithmetic op=ADD(w54, w53, w52, w51, w50, w49, w48, w47, w46, w45) -> (→"Calculated_total_length_cmb":dbl)
    n1115 = case shown="False" w29 {
      frame #0 {
        w312 = FALSE ("R Single DC Step8 Coating Power Active")
        n1116 = local write "R Single DC Step10 Coating Power Active"(w312) -> ()
        n1117 = local write "R Single DC Step9 Coating Power Active"(w312) -> ()
        n1118 = local write "R Single DC Step8 Coating Power Active"(w312) -> ()
      }
      frame #1 {
        n1119 = local read "R Single DC Step8 Coating Power Active"() -> (w313:bool)
        n1120 = case shown="False" w313 {
          frame #0 {
            w314 = 0.0 ("R Single DC Step8 Coating Power")
            w315 = T5."Disabled and Grayed Out" ("Disabled")
            n1121 = local write "R Single DC Step8 Coating Power"(w314) -> ()
            n1122 = local write "R Single DC Interval length8"(w314) -> ()
            n1123 = property on="R Single DC Step8 Coating Power" class="DigNum (strict)"("DisabledEnum"=w315) -> ()  [unwired: 2 in, 2 out]
            n1124 = property on="R Single DC Interval length8" class="DigNum (strict)"("DisabledEnum"=w315) -> ()  [unwired: 2 in, 2 out]
          }
          frame #1 {
            w316 = T5."Enabled" ("Disabled")
            n1125 = property on="R Single DC Step8 Coating Power" class="DigNum (strict)"("DisabledEnum"=w316) -> ()  [unwired: 2 in, 2 out]
            n1126 = property on="R Single DC Interval length8" class="DigNum (strict)"("DisabledEnum"=w316) -> ()  [unwired: 2 in, 2 out]
          }
        }
      }
    }
    n1127 = stacked-sequence {
      frame #0 {
      }
    }
    n1128 = case shown="True" "Power_list_open_multi" {
      frame #0 {
        n1129 = property on="Multilayer_power_tab" class="TabCtl (strict)"("Visible"=FALSE) -> ()  [unwired: 2 in, 2 out]
      }
      frame #1 {
        n1130 = property on="Multilayer_power_tab" class="TabCtl (strict)"("Visible"=TRUE) -> ()  [unwired: 2 in, 2 out]
      }
    }
    n1131 = stacked-sequence {
      frame #0 {
        # "Thickness Monitor Parameters Set"
        n1132 = local read "R_Single DC_Material ok"() -> (w1145:bool)
        n1133 = local read "R_Single RF Material ok"() -> (w1144:bool)
        n1134 = local read "R_Cmb Ch2_Material ok"() -> (w1143:bool)
        n1135 = local read "R Cmb Ch3 Material ok"() -> (w1142:bool)
        n1136 = Build Array(FALSE, w1145, w1144, w1143, w1142) -> (w1163:bool[])
        n1137 = Boolean Array To Number(Boolean array=w1163) -> (number=w1162:u32)
        n1138 = Mantissa & Exponent(0:w1162) -> (2:w1160:dbl)  [unwired: 1 out]
        n1139 = case shown="0, Default" w1160 {
          tunnel: ["" ("Evs_1_mat") w1215 w1217 w1219 w1221] -> w1153
          frame #0 {
          }
          frame #1 {
            n1140 = local read "R Single DC Target material"() -> (w1215:string)
            n1141 = local write "R_Single DC_Material ok"(FALSE ("R_Single DC_Material ok")) -> ()
          }
          frame #2 {
            n1142 = local read "R Single RF Target material"() -> (w1217:string)
            n1143 = local write "R_Single RF Material ok"(FALSE ("R_Single RF Material ok")) -> ()
          }
          frame #3 {
            n1144 = local read "R Cmb Ch2 Target material"() -> (w1219:string)
            n1145 = local write "R_Cmb Ch2_Material ok"(FALSE ("R_Cmb Ch2_Material ok")) -> ()
          }
          frame #4 {
            n1146 = local read "R Cmb Ch3 Target material"() -> (w1221:string)
            n1147 = local write "R Cmb Ch3 Material ok"(FALSE ("R Cmb Ch3 Material ok")) -> ()
          }
        }
        n1148 = local read "R_Single DC_Material ok"() -> (w1141:bool)
        n1149 = local read "R_Single RF Material ok"() -> (w1140:bool)
        n1150 = local read "R_Cmb Ch2_Material ok"() -> (w1139:bool)
        n1151 = local read "R Cmb Ch3 Material ok"() -> (w1138:bool)
        n1152 = Read from Text File(file (use dialog)=path "D:/VK1701/Material Data/Material Properties.txt") -> (text=w1158:string)  [unwired: 3 in, 3 out]
        n1153 = Match Pattern(string=w1158, regular expression=w1153) -> (after substring=w1159:string)  [unwired: 1 in, 3 out]
        n1154 = String Length(string=w1153) -> (length=w1154:i32)
        n1155 = Build Array(FALSE, w1141, w1140, w1139, w1138) -> (w1150:bool[])
        n1156 = Match Pattern(string=w1159, regular expression="=") -> (after substring=w1157:string)  [unwired: 1 in, 3 out]
        n1157 = Boolean Array To Number(Boolean array=w1150) -> (number=w1151:u32)
        n1158 = Not Equal To 0?(x=w1154) -> (x != 0?=w1148:bool)
        n1159 = Match Pattern(string=w1157, regular expression="***") -> (before substring=w1147:string)  [unwired: 1 in, 3 out]
        n1160 = Mantissa & Exponent(0:w1151) -> (2:w1146:dbl)  [unwired: 1 out]
        n1161 = case shown="True" w1148 {
          tunnel: w1147 -> [_ w1164]
          tunnel: w1146 -> [_ w1165]
          frame #0 {
          }
          frame #1 {
            n1162 = case shown="3" w1165 {
              tunnel: w1164 -> [_ w1166 w1178 w1190 w1202]
              frame #0 {
              }
              frame #1 {
                n1163 = String Subset(string=w1166, offset (0)=4, length (rest)=5 ("length (rest)")) -> (substring=w1177:string)
                n1164 = String Subset(string=w1166, offset (0)=0, length (rest)=4 ("length (rest)")) -> (substring=w1175:string)
                n1165 = Scan Value(string=w1177, format string="%.3f") -> (value=w1167:dbl)  [unwired: 1 in, 1 out]
                n1166 = Scan Value(string=w1175, format string="%.2f") -> (value=w1169:dbl)  [unwired: 1 in, 1 out]
                n1167 = local write "R Z_factor"(w1167) -> ()
                n1168 = local write "R Material_density"(w1169) -> ()
                n1169 = local write "R Toooling_factor"(0.0 ("R Toooling_factor")) -> ()
              }
              frame #2 {
                n1170 = String Subset(string=w1178, offset (0)=4, length (rest)=5 ("length (rest)")) -> (substring=w1189:string)
                n1171 = String Subset(string=w1178, offset (0)=0, length (rest)=4 ("length (rest)")) -> (substring=w1187:string)
                n1172 = Scan Value(string=w1189, format string="%.3f") -> (value=w1179:dbl)  [unwired: 1 in, 1 out]
                n1173 = Scan Value(string=w1187, format string="%.2f") -> (value=w1181:dbl)  [unwired: 1 in, 1 out]
                n1174 = local write "R Z_factor"(w1179) -> ()
                n1175 = local write "R Material_density"(w1181) -> ()
                n1176 = local write "R Toooling_factor"(0.0 ("R Toooling_factor")) -> ()
              }
              frame #3 {
                n1177 = String Subset(string=w1190, offset (0)=4, length (rest)=5 ("length (rest)")) -> (substring=w1201:string)
                n1178 = String Subset(string=w1190, offset (0)=0, length (rest)=4 ("length (rest)")) -> (substring=w1199:string)
                n1179 = Scan Value(string=w1201, format string="%.3f") -> (value=w1191:dbl)  [unwired: 1 in, 1 out]
                n1180 = Scan Value(string=w1199, format string="%.2f") -> (value=w1193:dbl)  [unwired: 1 in, 1 out]
                n1181 = local write "R Z_factor"(w1191) -> ()
                n1182 = local write "R Material_density"(w1193) -> ()
                n1183 = local write "R Toooling_factor"(0.0 ("R Toooling_factor")) -> ()
              }
              frame #4 {
                n1184 = String Subset(string=w1202, offset (0)=4, length (rest)=5 ("length (rest)")) -> (substring=w1213:string)
                n1185 = String Subset(string=w1202, offset (0)=0, length (rest)=4 ("length (rest)")) -> (substring=w1211:string)
                n1186 = Scan Value(string=w1213, format string="%.3f") -> (value=w1203:dbl)  [unwired: 1 in, 1 out]
                n1187 = Scan Value(string=w1211, format string="%.2f") -> (value=w1205:dbl)  [unwired: 1 in, 1 out]
                n1188 = local write "R Z_factor"(w1203) -> ()
                n1189 = local write "R Material_density"(w1205) -> ()
                n1190 = local write "R Toooling_factor"(0.0 ("R Toooling_factor")) -> ()
              }
            }
          }
        }
      }
    }
    n1191 = local read "R Cmb Step2 Coating Power Active"() -> (w16:bool)
    n1192 = local read "R Cmb Step1 Coating Power Active"() -> (w17:bool)
    n1193 = local read "R Cmb Step4 Coating Power Active"() -> (w14:bool)
    n1194 = local read "Recipe_selection tab"() -> (w171:T1)
    n1195 = local read "R Cmb Step3 Coating Power Active"() -> (w15:bool)
    n1196 = case shown="100" "R_Single DC_Mat_sel" {
      frame #0 {
      }
      frame #1 {
        n1197 = local write "R Single DC Target material"("Ag" ("R DC Target material")) -> ()
      }
      frame #2 {
        n1198 = local write "R Single DC Target material"("AgBr" ("R DC Target material")) -> ()
      }
      frame #3 {
        n1199 = local write "R Single DC Target material"("AgCl" ("R DC Target material")) -> ()
      }
      frame #4 {
        n1200 = local write "R Single DC Target material"("Al" ("R DC Target material")) -> ()
      }
      frame #5 {
        n1201 = local write "R Single DC Target material"("Al2O3" ("R DC Target material")) -> ()
      }
      frame #6 {
        n1202 = local write "R Single DC Target material"("As" ("R DC Target material")) -> ()
      }
      frame #7 {
        n1203 = local write "R Single DC Target material"("Au" ("R DC Target material")) -> ()
      }
      frame #8 {
        n1204 = local write "R Single DC Target material"("B" ("R DC Target material")) -> ()
      }
      frame #9 {
        n1205 = local write "R Single DC Target material"("Ba" ("R DC Target material")) -> ()
      }
      frame #10 {
        n1206 = local write "R Single DC Target material"("Be" ("R DC Target material")) -> ()
      }
      frame #11 {
        n1207 = local write "R Single DC Target material"("Bi" ("R DC Target material")) -> ()
      }
      frame #12 {
        n1208 = local write "R Single DC Target material"("Bi2O3" ("R DC Target material")) -> ()
      }
      frame #13 {
        n1209 = local write "R Single DC Target material"("C (Diamond)" ("R DC Target material")) -> ()
      }
      frame #14 {
        n1210 = local write "R Single DC Target material"("C (Graphite)" ("R DC Target material")) -> ()
      }
      frame #15 {
        n1211 = local write "R Single DC Target material"("Ca" ("R DC Target material")) -> ()
      }
      frame #16 {
        n1212 = local write "R Single DC Target material"("CaF" ("R DC Target material")) -> ()
      }
      frame #17 {
        n1213 = local write "R Single DC Target material"("Cd" ("R DC Target material")) -> ()
      }
      frame #18 {
        n1214 = local write "R Single DC Target material"("CdS" ("R DC Target material")) -> ()
      }
      frame #19 {
        n1215 = local write "R Single DC Target material"("CdSe" ("R DC Target material")) -> ()
      }
      frame #20 {
        n1216 = local write "R Single DC Target material"("CdTe" ("R DC Target material")) -> ()
      }
      frame #21 {
        n1217 = local write "R Single DC Target material"("CeF3" ("R DC Target material")) -> ()
      }
      frame #22 {
        n1218 = local write "R Single DC Target material"("CeO" ("R DC Target material")) -> ()
      }
      frame #23 {
        n1219 = local write "R Single DC Target material"("Cr" ("R DC Target material")) -> ()
      }
      frame #24 {
        n1220 = local write "R Single DC Target material"("Cr2O3" ("R DC Target material")) -> ()
      }
      frame #25 {
        n1221 = local write "R Single DC Target material"("Co" ("R DC Target material")) -> ()
      }
      frame #26 {
        n1222 = local write "R Single DC Target material"("Cu" ("R DC Target material")) -> ()
      }
      frame #27 {
        n1223 = local write "R Single DC Target material"("Cu2S (A)" ("R DC Target material")) -> ()
      }
      frame #28 {
        n1224 = local write "R Single DC Target material"("Cu2S (B)" ("R DC Target material")) -> ()
      }
      frame #29 {
        n1225 = local write "R Single DC Target material"("CuS" ("R DC Target material")) -> ()
      }
      frame #30 {
        n1226 = local write "R Single DC Target material"("Dy" ("R DC Target material")) -> ()
      }
      frame #31 {
        n1227 = local write "R Single DC Target material"("Er" ("R DC Target material")) -> ()
      }
      frame #32 {
        n1228 = local write "R Single DC Target material"("Fe" ("R DC Target material")) -> ()
      }
      frame #33 {
        n1229 = local write "R Single DC Target material"("Ga" ("R DC Target material")) -> ()
      }
      frame #34 {
        n1230 = local write "R Single DC Target material"("GaAs" ("R DC Target material")) -> ()
      }
      frame #35 {
        n1231 = local write "R Single DC Target material"("Gd" ("R DC Target material")) -> ()
      }
      frame #36 {
        n1232 = local write "R Single DC Target material"("Ge" ("R DC Target material")) -> ()
      }
      frame #37 {
        n1233 = local write "R Single DC Target material"("Hf" ("R DC Target material")) -> ()
      }
      frame #38 {
        n1234 = local write "R Single DC Target material"("HfO2" ("R DC Target material")) -> ()
      }
      frame #39 {
        n1235 = local write "R Single DC Target material"("Hg" ("R DC Target material")) -> ()
      }
      frame #40 {
        n1236 = local write "R Single DC Target material"("Ho" ("R DC Target material")) -> ()
      }
      frame #41 {
        n1237 = local write "R Single DC Target material"("In" ("R DC Target material")) -> ()
      }
      frame #42 {
        n1238 = local write "R Single DC Target material"("InSb" ("R DC Target material")) -> ()
      }
      frame #43 {
        n1239 = local write "R Single DC Target material"("In2O3" ("R DC Target material")) -> ()
      }
      frame #44 {
        n1240 = local write "R Single DC Target material"("Ir" ("R DC Target material")) -> ()
      }
      frame #45 {
        n1241 = local write "R Single DC Target material"("KCl" ("R DC Target material")) -> ()
      }
      frame #46 {
        n1242 = local write "R Single DC Target material"("La" ("R DC Target material")) -> ()
      }
      frame #47 {
        n1243 = local write "R Single DC Target material"("LaF3" ("R DC Target material")) -> ()
      }
      frame #48 {
        n1244 = local write "R Single DC Target material"("LaO3" ("R DC Target material")) -> ()
      }
      frame #49 {
        n1245 = local write "R Single DC Target material"("Li" ("R DC Target material")) -> ()
      }
      frame #50 {
        n1246 = local write "R Single DC Target material"("LiF" ("R DC Target material")) -> ()
      }
      frame #51 {
        n1247 = local write "R Single DC Target material"("Mg" ("R DC Target material")) -> ()
      }
      frame #52 {
        n1248 = local write "R Single DC Target material"("MgF2" ("R DC Target material")) -> ()
      }
      frame #53 {
        n1249 = local write "R Single DC Target material"("MgO" ("R DC Target material")) -> ()
      }
      frame #54 {
        n1250 = local write "R Single DC Target material"("Mn" ("R DC Target material")) -> ()
      }
      frame #55 {
        n1251 = local write "R Single DC Target material"("MnS" ("R DC Target material")) -> ()
      }
      frame #56 {
        n1252 = local write "R Single DC Target material"("Mo" ("R DC Target material")) -> ()
      }
      frame #57 {
        n1253 = local write "R Single DC Target material"("Na" ("R DC Target material")) -> ()
      }
      frame #58 {
        n1254 = local write "R Single DC Target material"("NaCl" ("R DC Target material")) -> ()
      }
      frame #59 {
        n1255 = local write "R Single DC Target material"("NdF3" ("R DC Target material")) -> ()
      }
      frame #60 {
        n1256 = local write "R Single DC Target material"("Nd2O3" ("R DC Target material")) -> ()
      }
      frame #61 {
        n1257 = local write "R Single DC Target material"("Ni" ("R DC Target material")) -> ()
      }
      frame #62 {
        n1258 = local write "R Single DC Target material"("Nb" ("R DC Target material")) -> ()
      }
      frame #63 {
        n1259 = local write "R Single DC Target material"("Nb2O5" ("R DC Target material")) -> ()
      }
      frame #64 {
        n1260 = local write "R Single DC Target material"("Pb" ("R DC Target material")) -> ()
      }
      frame #65 {
        n1261 = local write "R Single DC Target material"("PbS" ("R DC Target material")) -> ()
      }
      frame #66 {
        n1262 = local write "R Single DC Target material"("Pd" ("R DC Target material")) -> ()
      }
      frame #67 {
        n1263 = local write "R Single DC Target material"("Pt" ("R DC Target material")) -> ()
      }
      frame #68 {
        n1264 = local write "R Single DC Target material"("Re" ("R DC Target material")) -> ()
      }
      frame #69 {
        n1265 = local write "R Single DC Target material"("Rh" ("R DC Target material")) -> ()
      }
      frame #70 {
        n1266 = local write "R Single DC Target material"("Rb" ("R DC Target material")) -> ()
      }
      frame #71 {
        n1267 = local write "R Single DC Target material"("S" ("R DC Target material")) -> ()
      }
      frame #72 {
        n1268 = local write "R Single DC Target material"("Sb" ("R DC Target material")) -> ()
      }
      frame #73 {
        n1269 = local write "R Single DC Target material"("Sc" ("R DC Target material")) -> ()
      }
      frame #74 {
        n1270 = local write "R Single DC Target material"("Se" ("R DC Target material")) -> ()
      }
      frame #75 {
        n1271 = local write "R Single DC Target material"("Si" ("R DC Target material")) -> ()
      }
      frame #76 {
        n1272 = local write "R Single DC Target material"("SiO" ("R DC Target material")) -> ()
      }
      frame #77 {
        n1273 = local write "R Single DC Target material"("SiO2" ("R DC Target material")) -> ()
      }
      frame #78 {
        n1274 = local write "R Single DC Target material"("Sm" ("R DC Target material")) -> ()
      }
      frame #79 {
        n1275 = local write "R Single DC Target material"("Sn" ("R DC Target material")) -> ()
      }
      frame #80 {
        n1276 = local write "R Single DC Target material"("Ta" ("R DC Target material")) -> ()
      }
      frame #81 {
        n1277 = local write "R Single DC Target material"("Ta2O5" ("R DC Target material")) -> ()
      }
      frame #82 {
        n1278 = local write "R Single DC Target material"("Te" ("R DC Target material")) -> ()
      }
      frame #83 {
        n1279 = local write "R Single DC Target material"("Tb" ("R DC Target material")) -> ()
      }
      frame #84 {
        n1280 = local write "R Single DC Target material"("ThF4" ("R DC Target material")) -> ()
      }
      frame #85 {
        n1281 = local write "R Single DC Target material"("Ti" ("R DC Target material")) -> ()
      }
      frame #86 {
        n1282 = local write "R Single DC Target material"("TiO2" ("R DC Target material")) -> ()
      }
      frame #87 {
        n1283 = local write "R Single DC Target material"("TiO" ("R DC Target material")) -> ()
      }
      frame #88 {
        n1284 = local write "R Single DC Target material"("Tl" ("R DC Target material")) -> ()
      }
      frame #89 {
        n1285 = local write "R Single DC Target material"("U" ("R DC Target material")) -> ()
      }
      frame #90 {
        n1286 = local write "R Single DC Target material"("V" ("R DC Target material")) -> ()
      }
      frame #91 {
        n1287 = local write "R Single DC Target material"("W" ("R DC Target material")) -> ()
      }
      frame #92 {
        n1288 = local write "R Single DC Target material"("WC" ("R DC Target material")) -> ()
      }
      frame #93 {
        n1289 = local write "R Single DC Target material"("Y" ("R DC Target material")) -> ()
      }
      frame #94 {
        n1290 = local write "R Single DC Target material"("Y2O3" ("R DC Target material")) -> ()
      }
      frame #95 {
        n1291 = local write "R Single DC Target material"("Yb" ("R DC Target material")) -> ()
      }
      frame #96 {
        n1292 = local write "R Single DC Target material"("Zn" ("R DC Target material")) -> ()
      }
      frame #97 {
        n1293 = local write "R Single DC Target material"("ZnO" ("R DC Target material")) -> ()
      }
      frame #98 {
        n1294 = local write "R Single DC Target material"("ZnSe" ("R DC Target material")) -> ()
      }
      frame #99 {
        n1295 = local write "R Single DC Target material"("ZnS" ("R DC Target material")) -> ()
      }
      frame #100 {
        n1296 = local write "R Single DC Target material"("Zr" ("R DC Target material")) -> ()
      }
      frame #101 {
        n1297 = local write "R Single DC Target material"("ZrO2" ("R DC Target material")) -> ()
      }
      frame #102 {
        n1298 = local write "R Single DC Target material"("Si3N4" ("R DC Target material")) -> ()
      }
      frame #103 {
        n1299 = local write "R Single DC Target material"("ITO" ("R DC Target material")) -> ()
      }
      frame #104 {
        n1300 = local write "R Single DC Target material"("PbI2" ("R DC Target material")) -> ()
      }
    }
    n1301 = case shown="1" "R_Cmb Ch2_Mat_sel" {
      frame #0 {
      }
      frame #1 {
        n1302 = local write "R Cmb Ch2 Target material"("Ag" ("R DC Target material")) -> ()
      }
      frame #2 {
        n1303 = local write "R Cmb Ch2 Target material"("AgBr" ("R DC Target material")) -> ()
      }
      frame #3 {
        n1304 = local write "R Cmb Ch2 Target material"("AgCl" ("R DC Target material")) -> ()
      }
      frame #4 {
        n1305 = local write "R Cmb Ch2 Target material"("Al" ("R DC Target material")) -> ()
      }
      frame #5 {
        n1306 = local write "R Cmb Ch2 Target material"("Al2O3" ("R DC Target material")) -> ()
      }
      frame #6 {
        n1307 = local write "R Cmb Ch2 Target material"("As" ("R DC Target material")) -> ()
      }
      frame #7 {
        n1308 = local write "R Cmb Ch2 Target material"("Au" ("R DC Target material")) -> ()
      }
      frame #8 {
        n1309 = local write "R Single DC Target material"("B" ("R DC Target material")) -> ()
      }
      frame #9 {
        n1310 = local write "R Cmb Ch2 Target material"("Ba" ("R DC Target material")) -> ()
      }
      frame #10 {
        n1311 = local write "R Cmb Ch2 Target material"("Be" ("R DC Target material")) -> ()
      }
      frame #11 {
        n1312 = local write "R Cmb Ch2 Target material"("Bi" ("R DC Target material")) -> ()
      }
      frame #12 {
        n1313 = local write "R Cmb Ch2 Target material"("Bi2O3" ("R DC Target material")) -> ()
      }
      frame #13 {
        n1314 = local write "R Cmb Ch2 Target material"("C (Diamond)" ("R DC Target material")) -> ()
      }
      frame #14 {
        n1315 = local write "R Cmb Ch2 Target material"("C (Graphite)" ("R DC Target material")) -> ()
      }
      frame #15 {
        n1316 = local write "R Cmb Ch2 Target material"("Ca" ("R DC Target material")) -> ()
      }
      frame #16 {
        n1317 = local write "R Cmb Ch2 Target material"("CaF" ("R DC Target material")) -> ()
      }
      frame #17 {
        n1318 = local write "R Cmb Ch2 Target material"("Cd" ("R DC Target material")) -> ()
      }
      frame #18 {
        n1319 = local write "R Cmb Ch2 Target material"("CdS" ("R DC Target material")) -> ()
      }
      frame #19 {
        n1320 = local write "R Cmb Ch2 Target material"("CdSe" ("R DC Target material")) -> ()
      }
      frame #20 {
        n1321 = local write "R Cmb Ch2 Target material"("CdTe" ("R DC Target material")) -> ()
      }
      frame #21 {
        n1322 = local write "R Cmb Ch2 Target material"("CeF3" ("R DC Target material")) -> ()
      }
      frame #22 {
        n1323 = local write "R Cmb Ch2 Target material"("CeO" ("R DC Target material")) -> ()
      }
      frame #23 {
        n1324 = local write "R Cmb Ch2 Target material"("Cr" ("R DC Target material")) -> ()
      }
      frame #24 {
        n1325 = local write "R Cmb Ch2 Target material"("Cr2O3" ("R DC Target material")) -> ()
      }
      frame #25 {
        n1326 = local write "R Cmb Ch2 Target material"("Co" ("R DC Target material")) -> ()
      }
      frame #26 {
        n1327 = local write "R Cmb Ch2 Target material"("Cu" ("R DC Target material")) -> ()
      }
      frame #27 {
        n1328 = local write "R Cmb Ch2 Target material"("Cu2S (A)" ("R DC Target material")) -> ()
      }
      frame #28 {
        n1329 = local write "R Cmb Ch2 Target material"("Cu2S (B)" ("R DC Target material")) -> ()
      }
      frame #29 {
        n1330 = local write "R Cmb Ch2 Target material"("CuS" ("R DC Target material")) -> ()
      }
      frame #30 {
        n1331 = local write "R Cmb Ch2 Target material"("Dy" ("R DC Target material")) -> ()
      }
      frame #31 {
        n1332 = local write "R Cmb Ch2 Target material"("Er" ("R DC Target material")) -> ()
      }
      frame #32 {
        n1333 = local write "R Cmb Ch2 Target material"("Fe" ("R DC Target material")) -> ()
      }
      frame #33 {
        n1334 = local write "R Cmb Ch2 Target material"("Ga" ("R DC Target material")) -> ()
      }
      frame #34 {
        n1335 = local write "R Cmb Ch2 Target material"("GaAs" ("R DC Target material")) -> ()
      }
      frame #35 {
        n1336 = local write "R Cmb Ch2 Target material"("Gd" ("R DC Target material")) -> ()
      }
      frame #36 {
        n1337 = local write "R Cmb Ch2 Target material"("Ge" ("R DC Target material")) -> ()
      }
      frame #37 {
        n1338 = local write "R Cmb Ch2 Target material"("Hf" ("R DC Target material")) -> ()
      }
      frame #38 {
        n1339 = local write "R Cmb Ch2 Target material"("HfO2" ("R DC Target material")) -> ()
      }
      frame #39 {
        n1340 = local write "R Cmb Ch2 Target material"("Hg" ("R DC Target material")) -> ()
      }
      frame #40 {
        n1341 = local write "R Cmb Ch2 Target material"("Ho" ("R DC Target material")) -> ()
      }
      frame #41 {
        n1342 = local write "R Cmb Ch2 Target material"("In" ("R DC Target material")) -> ()
      }
      frame #42 {
        n1343 = local write "R Cmb Ch2 Target material"("InSb" ("R DC Target material")) -> ()
      }
      frame #43 {
        n1344 = local write "R Cmb Ch2 Target material"("In2O3" ("R DC Target material")) -> ()
      }
      frame #44 {
        n1345 = local write "R Cmb Ch2 Target material"("Ir" ("R DC Target material")) -> ()
      }
      frame #45 {
        n1346 = local write "R Cmb Ch2 Target material"("KCl" ("R DC Target material")) -> ()
      }
      frame #46 {
        n1347 = local write "R Cmb Ch2 Target material"("La" ("R DC Target material")) -> ()
      }
      frame #47 {
        n1348 = local write "R Cmb Ch2 Target material"("LaF3" ("R DC Target material")) -> ()
      }
      frame #48 {
        n1349 = local write "R Cmb Ch2 Target material"("LaO3" ("R DC Target material")) -> ()
      }
      frame #49 {
        n1350 = local write "R Cmb Ch2 Target material"("Li" ("R DC Target material")) -> ()
      }
      frame #50 {
        n1351 = local write "R Cmb Ch2 Target material"("LiF" ("R DC Target material")) -> ()
      }
      frame #51 {
        n1352 = local write "R Cmb Ch2 Target material"("Mg" ("R DC Target material")) -> ()
      }
      frame #52 {
        n1353 = local write "R Cmb Ch2 Target material"("MgF2" ("R DC Target material")) -> ()
      }
      frame #53 {
        n1354 = local write "R Cmb Ch2 Target material"("MgO" ("R DC Target material")) -> ()
      }
      frame #54 {
        n1355 = local write "R Cmb Ch2 Target material"("Mn" ("R DC Target material")) -> ()
      }
      frame #55 {
        n1356 = local write "R Cmb Ch2 Target material"("MnS" ("R DC Target material")) -> ()
      }
      frame #56 {
        n1357 = local write "R Cmb Ch2 Target material"("Mo" ("R DC Target material")) -> ()
      }
      frame #57 {
        n1358 = local write "R Cmb Ch2 Target material"("Na" ("R DC Target material")) -> ()
      }
      frame #58 {
        n1359 = local write "R Cmb Ch2 Target material"("NaCl" ("R DC Target material")) -> ()
      }
      frame #59 {
        n1360 = local write "R Cmb Ch2 Target material"("NdF3" ("R DC Target material")) -> ()
      }
      frame #60 {
        n1361 = local write "R Cmb Ch2 Target material"("Nd2O3" ("R DC Target material")) -> ()
      }
      frame #61 {
        n1362 = local write "R Cmb Ch2 Target material"("Ni" ("R DC Target material")) -> ()
      }
      frame #62 {
        n1363 = local write "R Cmb Ch2 Target material"("Nb" ("R DC Target material")) -> ()
      }
      frame #63 {
        n1364 = local write "R Cmb Ch2 Target material"("Nb2O5" ("R DC Target material")) -> ()
      }
      frame #64 {
        n1365 = local write "R Cmb Ch2 Target material"("Pb" ("R DC Target material")) -> ()
      }
      frame #65 {
        n1366 = local write "R Cmb Ch2 Target material"("PbS" ("R DC Target material")) -> ()
      }
      frame #66 {
        n1367 = local write "R Cmb Ch2 Target material"("Pd" ("R DC Target material")) -> ()
      }
      frame #67 {
        n1368 = local write "R Cmb Ch2 Target material"("Pt" ("R DC Target material")) -> ()
      }
      frame #68 {
        n1369 = local write "R Cmb Ch2 Target material"("Re" ("R DC Target material")) -> ()
      }
      frame #69 {
        n1370 = local write "R Cmb Ch2 Target material"("Rh" ("R DC Target material")) -> ()
      }
      frame #70 {
        n1371 = local write "R Cmb Ch2 Target material"("Rb" ("R DC Target material")) -> ()
      }
      frame #71 {
        n1372 = local write "R Cmb Ch2 Target material"("S" ("R DC Target material")) -> ()
      }
      frame #72 {
        n1373 = local write "R Cmb Ch2 Target material"("Sb" ("R DC Target material")) -> ()
      }
      frame #73 {
        n1374 = local write "R Cmb Ch2 Target material"("Sc" ("R DC Target material")) -> ()
      }
      frame #74 {
        n1375 = local write "R Cmb Ch2 Target material"("Se" ("R DC Target material")) -> ()
      }
      frame #75 {
        n1376 = local write "R Cmb Ch2 Target material"("Si" ("R DC Target material")) -> ()
      }
      frame #76 {
        n1377 = local write "R Cmb Ch2 Target material"("SiO" ("R DC Target material")) -> ()
      }
      frame #77 {
        n1378 = local write "R Cmb Ch2 Target material"("SiO2" ("R DC Target material")) -> ()
      }
      frame #78 {
        n1379 = local write "R Cmb Ch2 Target material"("Sm" ("R DC Target material")) -> ()
      }
      frame #79 {
        n1380 = local write "R Cmb Ch2 Target material"("Sn" ("R DC Target material")) -> ()
      }
      frame #80 {
        n1381 = local write "R Cmb Ch2 Target material"("Ta" ("R DC Target material")) -> ()
      }
      frame #81 {
        n1382 = local write "R Cmb Ch2 Target material"("Ta2O5" ("R DC Target material")) -> ()
      }
      frame #82 {
        n1383 = local write "R Cmb Ch2 Target material"("Te" ("R DC Target material")) -> ()
      }
      frame #83 {
        n1384 = local write "R Cmb Ch2 Target material"("Tb" ("R DC Target material")) -> ()
      }
      frame #84 {
        n1385 = local write "R Cmb Ch2 Target material"("ThF4" ("R DC Target material")) -> ()
      }
      frame #85 {
        n1386 = local write "R Cmb Ch2 Target material"("Ti" ("R DC Target material")) -> ()
      }
      frame #86 {
        n1387 = local write "R Cmb Ch2 Target material"("TiO2" ("R DC Target material")) -> ()
      }
      frame #87 {
        n1388 = local write "R Cmb Ch2 Target material"("TiO" ("R DC Target material")) -> ()
      }
      frame #88 {
        n1389 = local write "R Cmb Ch2 Target material"("Tl" ("R DC Target material")) -> ()
      }
      frame #89 {
        n1390 = local write "R Cmb Ch2 Target material"("U" ("R DC Target material")) -> ()
      }
      frame #90 {
        n1391 = local write "R Cmb Ch2 Target material"("V" ("R DC Target material")) -> ()
      }
      frame #91 {
        n1392 = local write "R Cmb Ch2 Target material"("W" ("R DC Target material")) -> ()
      }
      frame #92 {
        n1393 = local write "R Cmb Ch2 Target material"("WC" ("R DC Target material")) -> ()
      }
      frame #93 {
        n1394 = local write "R Cmb Ch2 Target material"("Y" ("R DC Target material")) -> ()
      }
      frame #94 {
        n1395 = local write "R Cmb Ch2 Target material"("Y2O3" ("R DC Target material")) -> ()
      }
      frame #95 {
        n1396 = local write "R Cmb Ch2 Target material"("Yb" ("R DC Target material")) -> ()
      }
      frame #96 {
        n1397 = local write "R Cmb Ch2 Target material"("Zn" ("R DC Target material")) -> ()
      }
      frame #97 {
        n1398 = local write "R Cmb Ch2 Target material"("ZnO" ("R DC Target material")) -> ()
      }
      frame #98 {
        n1399 = local write "R Cmb Ch2 Target material"("ZnSe" ("R DC Target material")) -> ()
      }
      frame #99 {
        n1400 = local write "R Cmb Ch2 Target material"("ZnS" ("R DC Target material")) -> ()
      }
      frame #100 {
        n1401 = local write "R Cmb Ch2 Target material"("Zr" ("R DC Target material")) -> ()
      }
      frame #101 {
        n1402 = local write "R Cmb Ch2 Target material"("ZrO2" ("R DC Target material")) -> ()
      }
      frame #102 {
        n1403 = local write "R Cmb Ch2 Target material"("Si3N4" ("R DC Target material")) -> ()
      }
      frame #103 {
        n1404 = local write "R Cmb Ch2 Target material"("ITO" ("R DC Target material")) -> ()
      }
      frame #104 {
        n1405 = local write "R Cmb Ch2 Target material"("PbI2" ("R DC Target material")) -> ()
      }
    }
    n1406 = local read "Web_selection_tab"() -> (w194:T4)
    n1407 = case shown="\"Multilayer Recipe                                                                  \"" w171 {
      frame #0 {
      }
      frame #1 {
        n1408 = local write "R_Simple_Coating Type Selection"(T2."DC Sputter" ("R_Simple_Coating Type Selection")) -> ()
      }
    }
    n1409 = local read "R Single RF Step8 Coating Power Active"() -> (w18:bool)
    n1410 = case shown="True" w17 {
      frame #0 {
      }
      frame #1 {
        n1411 = local read "R Cmb Step2 Coating Power Active"() -> (w254:bool)
        n1412 = case shown="False" w254 {
          frame #0 {
            w255 = 0.0 ("R Cmb Ch2 Step2 Coating Power")
            w256 = T5."Disabled and Grayed Out" ("Disabled")
            n1413 = local write "R Cmb Ch3 Step2 Coating Power"(w255) -> ()
            n1414 = local write "R Cmb Ch2 Step2 Coating Power"(w255) -> ()
            n1415 = local write "R Cmb Interval length 2"(w255) -> ()
            n1416 = property on="R Cmb Ch2 Step2 Coating Power" class="DigNum (strict)"("DisabledEnum"=w256) -> ()  [unwired: 2 in, 2 out]
            n1417 = property on="R Cmb Ch3 Step2 Coating Power" class="DigNum (strict)"("DisabledEnum"=w256) -> ()  [unwired: 2 in, 2 out]
            n1418 = property on="R Cmb Interval length 2" class="DigNum (strict)"("DisabledEnum"=w256) -> ()  [unwired: 2 in, 2 out]
          }
          frame #1 {
            w257 = T5."Enabled" ("Disabled")
            n1419 = property on="R Cmb Ch2 Step2 Coating Power" class="DigNum (strict)"("DisabledEnum"=w257) -> ()  [unwired: 2 in, 2 out]
            n1420 = property on="R Cmb Ch3 Step2 Coating Power" class="DigNum (strict)"("DisabledEnum"=w257) -> ()  [unwired: 2 in, 2 out]
            n1421 = property on="R Cmb Interval length 2" class="DigNum (strict)"("DisabledEnum"=w257) -> ()  [unwired: 2 in, 2 out]
          }
        }
      }
    }
    n1422 = case shown="True" w16 {
      frame #0 {
        w249 = FALSE ("R Cmb Step3 Coating Power Active")
        n1423 = local write "R Cmb Step3 Coating Power Active"(w249) -> ()
        n1424 = local write "R Cmb Step4 Coating Power Active"(w249) -> ()
        n1425 = local write "R Cmb Step5 Coating Power Active"(w249) -> ()
        n1426 = local write "R Cmb Step6 Coating Power Active"(w249) -> ()
        n1427 = local write "R Cmb Step7 Coating Power Active"(w249) -> ()
        n1428 = local write "R Cmb Step8 Coating Power Active"(w249) -> ()
        n1429 = local write "R Cmb Step9 Coating Power Active"(w249) -> ()
        n1430 = local write "R Cmb Step10 Coating Power Active"(w249) -> ()
      }
      frame #1 {
        n1431 = local read "R Cmb Step3 Coating Power Active"() -> (w250:bool)
        n1432 = case shown="False" w250 {
          frame #0 {
            w251 = 0.0 ("R Cmb Ch2 Step3 Coating Power")
            w252 = T5."Disabled and Grayed Out" ("Disabled")
            n1433 = local write "R Cmb Ch2 Step3 Coating Power"(w251) -> ()
            n1434 = local write "R Cmb Ch3 Step3 Coating Power"(w251) -> ()
            n1435 = local write "R Cmb Interval length 3"(w251) -> ()
            n1436 = property on="R Cmb Ch3 Step3 Coating Power" class="DigNum (strict)"("DisabledEnum"=w252) -> ()  [unwired: 2 in, 2 out]
            n1437 = property on="R Cmb Interval length 3" class="DigNum (strict)"("DisabledEnum"=w252) -> ()  [unwired: 2 in, 2 out]
            n1438 = property on="R Cmb Ch2 Step3 Coating Power" class="DigNum (strict)"("DisabledEnum"=w252) -> ()  [unwired: 2 in, 2 out]
          }
          frame #1 {
            w253 = T5."Enabled" ("Disabled")
            n1439 = property on="R Cmb Ch3 Step3 Coating Power" class="DigNum (strict)"("DisabledEnum"=w253) -> ()  [unwired: 2 in, 2 out]
            n1440 = property on="R Cmb Interval length 3" class="DigNum (strict)"("DisabledEnum"=w253) -> ()  [unwired: 2 in, 2 out]
            n1441 = property on="R Cmb Ch2 Step3 Coating Power" class="DigNum (strict)"("DisabledEnum"=w253) -> ()  [unwired: 2 in, 2 out]
          }
        }
      }
    }
    n1442 = case shown="False" w14 {
      frame #0 {
        w239 = FALSE ("R Cmb Step3 Coating Power Active")
        n1443 = local write "R Cmb Step5 Coating Power Active"(w239) -> ()
        n1444 = local write "R Cmb Step6 Coating Power Active"(w239) -> ()
        n1445 = local write "R Cmb Step7 Coating Power Active"(w239) -> ()
        n1446 = local write "R Cmb Step8 Coating Power Active"(w239) -> ()
        n1447 = local write "R Cmb Step9 Coating Power Active"(w239) -> ()
        n1448 = local write "R Cmb Step10 Coating Power Active"(w239) -> ()
      }
      frame #1 {
        n1449 = local read "R Cmb Step5 Coating Power Active"() -> (w240:bool)
        n1450 = case shown="False" w240 {
          frame #0 {
            w241 = 0.0 ("R Cmb Ch2 Step5 Coating Power")
            w242 = T5."Disabled and Grayed Out" ("Disabled")
            n1451 = local write "R Cmb Ch2 Step5 Coating Power"(w241) -> ()
            n1452 = local write "R Cmb Ch3 Step5 Coating Power"(w241) -> ()
            n1453 = local write "R Cmb Interval length 5"(w241) -> ()
            n1454 = property on="R Cmb Ch3 Step5 Coating Power" class="DigNum (strict)"("DisabledEnum"=w242) -> ()  [unwired: 2 in, 2 out]
            n1455 = property on="R Cmb Interval length 5" class="DigNum (strict)"("DisabledEnum"=w242) -> ()  [unwired: 2 in, 2 out]
            n1456 = property on="R Cmb Ch2 Step5 Coating Power" class="DigNum (strict)"("DisabledEnum"=w242) -> ()  [unwired: 2 in, 2 out]
          }
          frame #1 {
            w243 = T5."Enabled" ("Disabled")
            n1457 = property on="R Cmb Ch3 Step5 Coating Power" class="DigNum (strict)"("DisabledEnum"=w243) -> ()  [unwired: 2 in, 2 out]
            n1458 = property on="R Cmb Interval length 5" class="DigNum (strict)"("DisabledEnum"=w243) -> ()  [unwired: 2 in, 2 out]
            n1459 = property on="R Cmb Ch2 Step5 Coating Power" class="DigNum (strict)"("DisabledEnum"=w243) -> ()  [unwired: 2 in, 2 out]
          }
        }
      }
    }
    n1460 = case shown="True" w15 {
      frame #0 {
        w244 = FALSE ("R Cmb Step3 Coating Power Active")
        n1461 = local write "R Cmb Step4 Coating Power Active"(w244) -> ()
        n1462 = local write "R Cmb Step5 Coating Power Active"(w244) -> ()
        n1463 = local write "R Cmb Step6 Coating Power Active"(w244) -> ()
        n1464 = local write "R Cmb Step7 Coating Power Active"(w244) -> ()
        n1465 = local write "R Cmb Step8 Coating Power Active"(w244) -> ()
        n1466 = local write "R Cmb Step9 Coating Power Active"(w244) -> ()
        n1467 = local write "R Cmb Step10 Coating Power Active"(w244) -> ()
      }
      frame #1 {
        n1468 = local read "R Cmb Step4 Coating Power Active"() -> (w245:bool)
        n1469 = case shown="False" w245 {
          frame #0 {
            w246 = 0.0 ("R Cmb Ch2 Step4 Coating Power")
            w247 = T5."Disabled and Grayed Out" ("Disabled")
            n1470 = local write "R Cmb Ch2 Step4 Coating Power"(w246) -> ()
            n1471 = local write "R Cmb Ch3 Step4 Coating Power"(w246) -> ()
            n1472 = local write "R Cmb Interval length 4"(w246) -> ()
            n1473 = property on="R Cmb Ch2 Step4 Coating Power" class="DigNum (strict)"("DisabledEnum"=w247) -> ()  [unwired: 2 in, 2 out]
            n1474 = property on="R Cmb Ch3 Step4 Coating Power" class="DigNum (strict)"("DisabledEnum"=w247) -> ()  [unwired: 2 in, 2 out]
            n1475 = property on="R Cmb Interval length 4" class="DigNum (strict)"("DisabledEnum"=w247) -> ()  [unwired: 2 in, 2 out]
          }
          frame #1 {
            w248 = T5."Enabled" ("Disabled")
            n1476 = property on="R Cmb Ch2 Step4 Coating Power" class="DigNum (strict)"("DisabledEnum"=w248) -> ()  [unwired: 2 in, 2 out]
            n1477 = property on="R Cmb Ch3 Step4 Coating Power" class="DigNum (strict)"("DisabledEnum"=w248) -> ()  [unwired: 2 in, 2 out]
            n1478 = property on="R Cmb Interval length 4" class="DigNum (strict)"("DisabledEnum"=w248) -> ()  [unwired: 2 in, 2 out]
          }
        }
      }
    }
    n1479 = local read "R Cmb Step1 Coating Power Active"() -> (w169:bool)
    n1480 = case shown="True" "Power_singledc_list_open" {
      frame #0 {
        n1481 = property on="Single_DC_power_power_tab" class="TabCtl (strict)"("Visible"=FALSE) -> ()  [unwired: 2 in, 2 out]
      }
      frame #1 {
        n1482 = property on="Single_DC_power_power_tab" class="TabCtl (strict)"("Visible"=TRUE) -> ()  [unwired: 2 in, 2 out]
      }
    }
    n1483 = Equal?(x=w194, y=1) -> (x = y?=w192:bool)
    n1484 = case shown="True" w192 {
      frame #0 {
        n1485 = property on="R_Single Microwave Time" class="DigNum (strict)"("DisabledEnum"=T5."Disabled and Grayed Out" ("Disabled")) -> ()  [unwired: 2 in, 2 out]
      }
      frame #1 {
        w1668 = 0.0 ("R Single DC Step2 Coating Power")
        w1666 = T5."Disabled and Grayed Out" ("Disabled")
        w1667 = FALSE ("R Single DC Step2 Coating Power Active")
        n1486 = local write "R Single RF Step2 Coating Power Active"(w1667) -> ()
        n1487 = local write "R Single RF Step3 Coating Power Active"(w1667) -> ()
        n1488 = local write "R Single RF Step4 Coating Power Active"(w1667) -> ()
        n1489 = local write "R Single RF Step5 Coating Power Active"(w1667) -> ()
        n1490 = local write "R Single RF Step6 Coating Power Active"(w1667) -> ()
        n1491 = local write "R Single RF Step7 Coating Power Active"(w1667) -> ()
        n1492 = local write "R Single RF Step8 Coating Power Active"(w1667) -> ()
        n1493 = local write "R Single RF Step9 Coating Power Active"(w1667) -> ()
        n1494 = local write "R Single RF Step10 Coating Power Active"(w1667) -> ()
        n1495 = local write "R Single DC Step2 Coating Power Active"(w1667) -> ()
        n1496 = local write "R Single DC Step3 Coating Power Active"(w1667) -> ()
        n1497 = local write "R Single DC Step4 Coating Power Active"(w1667) -> ()
        n1498 = local write "R Single DC Step5 Coating Power Active"(w1667) -> ()
        n1499 = local write "R Single DC Step6 Coating Power Active"(w1667) -> ()
        n1500 = local write "R Single DC Step7 Coating Power Active"(w1667) -> ()
        n1501 = local write "R Single DC Step8 Coating Power Active"(w1667) -> ()
        n1502 = local write "R Single DC Step9 Coating Power Active"(w1667) -> ()
        n1503 = local write "R Single DC Step10 Coating Power Active"(w1667) -> ()
        n1504 = local write "R Single DC Step2 Coating Power"(w1668) -> ()
        n1505 = local write "R Single DC Step3 Coating Power"(w1668) -> ()
        n1506 = local write "R Single DC Step4 Coating Power"(w1668) -> ()
        n1507 = local write "R Single DC Step5 Coating Power"(w1668) -> ()
        n1508 = local write "R Single RF Step2 Coating Power"(w1668) -> ()
        n1509 = local write "R Single RF Step3 Coating Power"(w1668) -> ()
        n1510 = local write "R Single RF Step4 Coating Power"(w1668) -> ()
        n1511 = local write "R Single RF Step5 Coating Power"(w1668) -> ()
        n1512 = local write "R Single DC Step6 Coating Power"(w1668) -> ()
        n1513 = local write "R Single DC Step7 Coating Power"(w1668) -> ()
        n1514 = local write "R Single DC Step8 Coating Power"(w1668) -> ()
        n1515 = local write "R Single DC Step9 Coating Power"(w1668) -> ()
        n1516 = local write "R Single DC Step10 Coating Power"(w1668) -> ()
        n1517 = local write "R Single RF Step6 Coating Power"(w1668) -> ()
        n1518 = local write "R Single RF Step7 Coating Power"(w1668) -> ()
        n1519 = local write "R Single RF Step8 Coating Power"(w1668) -> ()
        n1520 = local write "R Single RF Step9 Coating Power"(w1668) -> ()
        n1521 = local write "R Single RF Step10 Coating Power"(w1668) -> ()
        n1522 = property on="R_Single Microwave Time" class="DigNum (strict)"("DisabledEnum"=T5."Enabled" ("Disabled")) -> ()  [unwired: 2 in, 2 out]
        n1523 = property on="R Single DC Step2 Coating Power" class="DigNum (strict)"("DisabledEnum"=w1666) -> ()  [unwired: 2 in, 2 out]
        n1524 = property on="R Single DC Step3 Coating Power" class="DigNum (strict)"("DisabledEnum"=w1666) -> ()  [unwired: 2 in, 2 out]
        n1525 = property on="R Single DC Step4 Coating Power" class="DigNum (strict)"("DisabledEnum"=w1666) -> ()  [unwired: 2 in, 2 out]
        n1526 = property on="R Single DC Step5 Coating Power" class="DigNum (strict)"("DisabledEnum"=w1666) -> ()  [unwired: 2 in, 2 out]
        n1527 = property on="R Single RF Step2 Coating Power" class="DigNum (strict)"("DisabledEnum"=w1666) -> ()  [unwired: 2 in, 2 out]
        n1528 = property on="R Single RF Step3 Coating Power" class="DigNum (strict)"("DisabledEnum"=w1666) -> ()  [unwired: 2 in, 2 out]
        n1529 = property on="R Single RF Step4 Coating Power" class="DigNum (strict)"("DisabledEnum"=w1666) -> ()  [unwired: 2 in, 2 out]
        n1530 = property on="R Single RF Step5 Coating Power" class="DigNum (strict)"("DisabledEnum"=w1666) -> ()  [unwired: 2 in, 2 out]
        n1531 = property on="R Single RF Step6 Coating Power" class="DigNum (strict)"("DisabledEnum"=w1666) -> ()  [unwired: 2 in, 2 out]
        n1532 = property on="R Single RF Step7 Coating Power" class="DigNum (strict)"("DisabledEnum"=w1666) -> ()  [unwired: 2 in, 2 out]
        n1533 = property on="R Single RF Step8 Coating Power" class="DigNum (strict)"("DisabledEnum"=w1666) -> ()  [unwired: 2 in, 2 out]
        n1534 = property on="R Single RF Step9 Coating Power" class="DigNum (strict)"("DisabledEnum"=w1666) -> ()  [unwired: 2 in, 2 out]
        n1535 = property on="R Single RF Step10 Coating Power" class="DigNum (strict)"("DisabledEnum"=w1666) -> ()  [unwired: 2 in, 2 out]
        n1536 = local write "R Single DC Interval length2"(w1668) -> ()
        n1537 = local write "R Single DC Interval length3"(w1668) -> ()
        n1538 = local write "R Single DC Interval length4"(w1668) -> ()
        n1539 = local write "R Single DC Interval length5"(w1668) -> ()
        n1540 = local write "R Single DC Interval length6"(w1668) -> ()
        n1541 = local write "R Single DC Interval length7"(w1668) -> ()
        n1542 = local write "R Single DC Interval length8"(w1668) -> ()
        n1543 = local write "R Single DC Interval length9"(w1668) -> ()
        n1544 = local write "R Single DC Interval length10"(w1668) -> ()
        n1545 = local write "R Single RF Interval length2"(w1668) -> ()
        n1546 = local write "R Single RF Interval length3"(w1668) -> ()
        n1547 = local write "R Single RF Interval length4"(w1668) -> ()
        n1548 = local write "R Single RF Interval length5"(w1668) -> ()
        n1549 = local write "R Single RF Interval length6"(w1668) -> ()
        n1550 = local write "R Single RF Interval length7"(w1668) -> ()
        n1551 = local write "R Single RF Interval length8"(w1668) -> ()
        n1552 = local write "R Single RF Interval length9"(w1668) -> ()
        n1553 = local write "R Single RF Interval length10"(w1668) -> ()
        n1554 = property on="R Single DC Interval length6" class="DigNum (strict)"("DisabledEnum"=w1666) -> ()  [unwired: 2 in, 2 out]
        n1555 = property on="R Single DC Interval length7" class="DigNum (strict)"("DisabledEnum"=w1666) -> ()  [unwired: 2 in, 2 out]
        n1556 = property on="R Single DC Interval length8" class="DigNum (strict)"("DisabledEnum"=w1666) -> ()  [unwired: 2 in, 2 out]
        n1557 = property on="R Single DC Interval length9" class="DigNum (strict)"("DisabledEnum"=w1666) -> ()  [unwired: 2 in, 2 out]
        n1558 = property on="R Single DC Interval length10" class="DigNum (strict)"("DisabledEnum"=w1666) -> ()  [unwired: 2 in, 2 out]
        n1559 = property on="R Single RF Interval length2" class="DigNum (strict)"("DisabledEnum"=w1666) -> ()  [unwired: 2 in, 2 out]
        n1560 = property on="R Single RF Interval length3" class="DigNum (strict)"("DisabledEnum"=w1666) -> ()  [unwired: 2 in, 2 out]
        n1561 = property on="R Single RF Interval length4" class="DigNum (strict)"("DisabledEnum"=w1666) -> ()  [unwired: 2 in, 2 out]
        n1562 = property on="R Single RF Interval length5" class="DigNum (strict)"("DisabledEnum"=w1666) -> ()  [unwired: 2 in, 2 out]
        n1563 = property on="R Single RF Interval length6" class="DigNum (strict)"("DisabledEnum"=w1666) -> ()  [unwired: 2 in, 2 out]
        n1564 = property on="R Single RF Interval length7" class="DigNum (strict)"("DisabledEnum"=w1666) -> ()  [unwired: 2 in, 2 out]
        n1565 = property on="R Single RF Interval length8" class="DigNum (strict)"("DisabledEnum"=w1666) -> ()  [unwired: 2 in, 2 out]
        n1566 = property on="R Single RF Interval length9" class="DigNum (strict)"("DisabledEnum"=w1666) -> ()  [unwired: 2 in, 2 out]
        n1567 = property on="R Single RF Interval length10" class="DigNum (strict)"("DisabledEnum"=w1666) -> ()  [unwired: 2 in, 2 out]
        n1568 = property on="R Single DC Step6 Coating Power" class="DigNum (strict)"("DisabledEnum"=w1666) -> ()  [unwired: 2 in, 2 out]
        n1569 = property on="R Single DC Step7 Coating Power" class="DigNum (strict)"("DisabledEnum"=w1666) -> ()  [unwired: 2 in, 2 out]
        n1570 = property on="R Single DC Step8 Coating Power" class="DigNum (strict)"("DisabledEnum"=w1666) -> ()  [unwired: 2 in, 2 out]
        n1571 = property on="R Single DC Step9 Coating Power" class="DigNum (strict)"("DisabledEnum"=w1666) -> ()  [unwired: 2 in, 2 out]
        n1572 = property on="R Single DC Step10 Coating Power" class="DigNum (strict)"("DisabledEnum"=w1666) -> ()  [unwired: 2 in, 2 out]
        n1573 = property on="R Single DC Interval length2" class="DigNum (strict)"("DisabledEnum"=w1666) -> ()  [unwired: 2 in, 2 out]
        n1574 = property on="R Single DC Interval length3" class="DigNum (strict)"("DisabledEnum"=w1666) -> ()  [unwired: 2 in, 2 out]
        n1575 = property on="R Single DC Interval length4" class="DigNum (strict)"("DisabledEnum"=w1666) -> ()  [unwired: 2 in, 2 out]
        n1576 = property on="R Single DC Interval length5" class="DigNum (strict)"("DisabledEnum"=w1666) -> ()  [unwired: 2 in, 2 out]
      }
    }
    n1577 = case shown="False" w18 {
      frame #0 {
        w258 = FALSE ("R Single RF Step3 Coating Power Active")
        n1578 = local write "R Single RF Step9 Coating Power Active"(w258) -> ()
        n1579 = local write "R Single RF Step10 Coating Power Active"(w258) -> ()
      }
      frame #1 {
        n1580 = local read "R Single RF Step9 Coating Power Active"() -> (w259:bool)
        n1581 = case shown="False" w259 {
          frame #0 {
            w260 = 0.0 ("Target Clean Power")
            w261 = T5."Disabled and Grayed Out" ("Disabled")
            n1582 = local write "R Single RF Step9 Coating Power"(w260) -> ()
            n1583 = local write "R Single RF Interval length9"(w260) -> ()
            n1584 = property on="R Single RF Step9 Coating Power" class="DigNum (strict)"("DisabledEnum"=w261) -> ()  [unwired: 2 in, 2 out]
            n1585 = property on="R Single RF Interval length9" class="DigNum (strict)"("DisabledEnum"=w261) -> ()  [unwired: 2 in, 2 out]
          }
          frame #1 {
            w262 = T5."Enabled" ("Disabled")
            n1586 = property on="R Single RF Step9 Coating Power" class="DigNum (strict)"("DisabledEnum"=w262) -> ()  [unwired: 2 in, 2 out]
            n1587 = property on="R Single RF Interval length9" class="DigNum (strict)"("DisabledEnum"=w262) -> ()  [unwired: 2 in, 2 out]
          }
        }
      }
    }
    n1588 = stacked-sequence {
      frame #0 {
      }
    }
    n1589 = case shown="False" w169 {
      frame #0 {
        w1111 = 0.0 ("R Cmb Ch2 Step1 Coating Power")
        w1112 = T5."Disabled and Grayed Out" ("Disabled")
        n1590 = local write "R Cmb Ch2 Step1 Coating Power"(w1111) -> ()
        n1591 = local write "R Cmb Ch3 Step1 Coating Power"(w1111) -> ()
        n1592 = local write "R Cmb Interval length 1"(w1111) -> ()
        n1593 = property on="R Cmb Ch3 Step1 Coating Power" class="DigNum (strict)"("DisabledEnum"=w1112) -> ()  [unwired: 2 in, 2 out]
        n1594 = property on="R Cmb Ch2 Step1 Coating Power" class="DigNum (strict)"("DisabledEnum"=w1112) -> ()  [unwired: 2 in, 2 out]
        n1595 = property on="R Cmb Interval length 1" class="DigNum (strict)"("DisabledEnum"=w1112) -> ()  [unwired: 2 in, 2 out]
      }
      frame #1 {
        w1113 = T5."Enabled" ("Disabled")
        n1596 = property on="R Cmb Ch3 Step1 Coating Power" class="DigNum (strict)"("DisabledEnum"=w1113) -> ()  [unwired: 2 in, 2 out]
        n1597 = property on="R Cmb Ch2 Step1 Coating Power" class="DigNum (strict)"("DisabledEnum"=w1113) -> ()  [unwired: 2 in, 2 out]
        n1598 = property on="R Cmb Interval length 1" class="DigNum (strict)"("DisabledEnum"=w1113) -> ()  [unwired: 2 in, 2 out]
      }
    }
    n1599 = case shown="True" "Calculate" {
      frame #0 {
      }
      frame #1 {
        n1600 = stacked-sequence {
          frame #0 {
            w1117 = 0.0 ("Lap")
            n1601 = local read "R Minimum diameter"() -> (w1118:dbl)
            n1602 = local write "Diameter"(w1118) -> ()
            n1603 = local write "Lap"(w1117) -> ()
            n1604 = local write "R  Total length"(w1117) -> ()
          }
          frame #1 {
            n1605 = while {
              stop <- w1121 stop-if-true
              n1606 = local read "R Web thickness"() -> (w1131:dbl)
              n1607 = Wait Until Next ms Multiple(millisecond multiple=u32 10) -> ()  [unwired: 1 out]
              n1608 = Multiply(x=w1131, y=0.002) -> (x*y=w1130:dbl)
              n1609 = local read "Lap"() -> (w1134:dbl)
              n1610 = Increment(x=w1134) -> (x+1=→"Lap":dbl)
              n1611 = Add(x="Diameter", y=w1130) -> (x+y=w1129:dbl)
              n1612 = local write "Diameter"(w1129) -> ()
              n1613 = local read "R Maximum diameter"() -> (w1122:dbl)
              n1614 = local read "Diameter"() -> (w1119:dbl)
              n1615 = Greater Or Equal?(x=w1119, y=w1122) -> (x >= y?=w1121:bool)
              n1616 = local read "R  Total length"() -> (w1120:dbl)
              n1617 = Multiply(x=w1119, y=3.141592653589793) -> (x*y=w1128:dbl)
              n1618 = Divide(x=w1128, y=10.0) -> (x/y=w1125:dbl)
              n1619 = Add(x=w1125, y=w1120) -> (x+y=→"R  Total length":dbl)
            }
          }
        }
      }
    }
    n1620 = case shown="False" "Power_single_rf_list_open" {
      frame #0 {
        n1621 = property on="Single_RF_power_power_tab" class="TabCtl (strict)"("Visible"=FALSE) -> ()  [unwired: 2 in, 2 out]
      }
      frame #1 {
        n1622 = property on="Single_RF_power_power_tab" class="TabCtl (strict)"("Visible"=TRUE) -> ()  [unwired: 2 in, 2 out]
      }
    }
    n1623 = local read "R Cmb Step6 Coating Power Active"() -> (w12:bool)
    n1624 = local read "R Cmb Step5 Coating Power Active"() -> (w13:bool)
    n1625 = local read "R Cmb Step7 Coating Power Active"() -> (w11:bool)
    n1626 = case shown="23" "R_Single RF_Mat_sel" {
      frame #0 {
      }
      frame #1 {
        n1627 = local write "R Single RF Target material"("Ag" ("R DC Target material")) -> ()
      }
      frame #2 {
        n1628 = local write "R Single RF Target material"("AgBr" ("R DC Target material")) -> ()
      }
      frame #3 {
        n1629 = local write "R Single RF Target material"("AgCl" ("R DC Target material")) -> ()
      }
      frame #4 {
        n1630 = local write "R Single RF Target material"("Al" ("R DC Target material")) -> ()
      }
      frame #5 {
        n1631 = local write "R Single RF Target material"("Al2O3" ("R DC Target material")) -> ()
      }
      frame #6 {
        n1632 = local write "R Single RF Target material"("As" ("R DC Target material")) -> ()
      }
      frame #7 {
        n1633 = local write "R Single RF Target material"("Au" ("R DC Target material")) -> ()
      }
      frame #8 {
        n1634 = local write "R Single RF Target material"("B" ("R DC Target material")) -> ()
      }
      frame #9 {
        n1635 = local write "R Single RF Target material"("Ba" ("R DC Target material")) -> ()
      }
      frame #10 {
        n1636 = local write "R Single RF Target material"("Be" ("R DC Target material")) -> ()
      }
      frame #11 {
        n1637 = local write "R Single RF Target material"("Bi" ("R DC Target material")) -> ()
      }
      frame #12 {
        n1638 = local write "R Single RF Target material"("Bi2O3" ("R DC Target material")) -> ()
      }
      frame #13 {
        n1639 = local write "R Single RF Target material"("C (Diamond)" ("R DC Target material")) -> ()
      }
      frame #14 {
        n1640 = local write "R Single RF Target material"("C (Graphite)" ("R DC Target material")) -> ()
      }
      frame #15 {
        n1641 = local write "R Single RF Target material"("Ca" ("R DC Target material")) -> ()
      }
      frame #16 {
        n1642 = local write "R Single RF Target material"("CaF" ("R DC Target material")) -> ()
      }
      frame #17 {
        n1643 = local write "R Single RF Target material"("Cd" ("R DC Target material")) -> ()
      }
      frame #18 {
        n1644 = local write "R Single RF Target material"("CdS" ("R DC Target material")) -> ()
      }
      frame #19 {
        n1645 = local write "R Single RF Target material"("CdSe" ("R DC Target material")) -> ()
      }
      frame #20 {
        n1646 = local write "R Single RF Target material"("CdTe" ("R DC Target material")) -> ()
      }
      frame #21 {
        n1647 = local write "R Single RF Target material"("CeF3" ("R DC Target material")) -> ()
      }
      frame #22 {
        n1648 = local write "R Single RF Target material"("CeO" ("R DC Target material")) -> ()
      }
      frame #23 {
        n1649 = local write "R Single RF Target material"("Cr" ("R DC Target material")) -> ()
      }
      frame #24 {
        n1650 = local write "R Single RF Target material"("Cr2O3" ("R DC Target material")) -> ()
      }
      frame #25 {
        n1651 = local write "R Single RF Target material"("Co" ("R DC Target material")) -> ()
      }
      frame #26 {
        n1652 = local write "R Single RF Target material"("Cu" ("R DC Target material")) -> ()
      }
      frame #27 {
        n1653 = local write "R Single RF Target material"("Cu2S (A)" ("R DC Target material")) -> ()
      }
      frame #28 {
        n1654 = local write "R Single RF Target material"("Cu2S (B)" ("R DC Target material")) -> ()
      }
      frame #29 {
        n1655 = local write "R Single RF Target material"("CuS" ("R DC Target material")) -> ()
      }
      frame #30 {
        n1656 = local write "R Single RF Target material"("Dy" ("R DC Target material")) -> ()
      }
      frame #31 {
        n1657 = local write "R Single RF Target material"("Er" ("R DC Target material")) -> ()
      }
      frame #32 {
        n1658 = local write "R Single RF Target material"("Fe" ("R DC Target material")) -> ()
      }
      frame #33 {
        n1659 = local write "R Single RF Target material"("Ga" ("R DC Target material")) -> ()
      }
      frame #34 {
        n1660 = local write "R Single RF Target material"("GaAs" ("R DC Target material")) -> ()
      }
      frame #35 {
        n1661 = local write "R Single RF Target material"("Gd" ("R DC Target material")) -> ()
      }
      frame #36 {
        n1662 = local write "R Single RF Target material"("Ge" ("R DC Target material")) -> ()
      }
      frame #37 {
        n1663 = local write "R Single RF Target material"("Hf" ("R DC Target material")) -> ()
      }
      frame #38 {
        n1664 = local write "R Single RF Target material"("HfO2" ("R DC Target material")) -> ()
      }
      frame #39 {
        n1665 = local write "R Single RF Target material"("Hg" ("R DC Target material")) -> ()
      }
      frame #40 {
        n1666 = local write "R Single RF Target material"("Ho" ("R DC Target material")) -> ()
      }
      frame #41 {
        n1667 = local write "R Single RF Target material"("In" ("R DC Target material")) -> ()
      }
      frame #42 {
        n1668 = local write "R Single RF Target material"("InSb" ("R DC Target material")) -> ()
      }
      frame #43 {
        n1669 = local write "R Single RF Target material"("In2O3" ("R DC Target material")) -> ()
      }
      frame #44 {
        n1670 = local write "R Single RF Target material"("Ir" ("R DC Target material")) -> ()
      }
      frame #45 {
        n1671 = local write "R Single RF Target material"("KCl" ("R DC Target material")) -> ()
      }
      frame #46 {
        n1672 = local write "R Single RF Target material"("La" ("R DC Target material")) -> ()
      }
      frame #47 {
        n1673 = local write "R Single RF Target material"("LaF3" ("R DC Target material")) -> ()
      }
      frame #48 {
        n1674 = local write "R Single RF Target material"("LaO3" ("R DC Target material")) -> ()
      }
      frame #49 {
        n1675 = local write "R Single RF Target material"("Li" ("R DC Target material")) -> ()
      }
      frame #50 {
        n1676 = local write "R Single RF Target material"("LiF" ("R DC Target material")) -> ()
      }
      frame #51 {
        n1677 = local write "R Single RF Target material"("Mg" ("R DC Target material")) -> ()
      }
      frame #52 {
        n1678 = local write "R Single RF Target material"("MgF2" ("R DC Target material")) -> ()
      }
      frame #53 {
        n1679 = local write "R Single RF Target material"("MgO" ("R DC Target material")) -> ()
      }
      frame #54 {
        n1680 = local write "R Single RF Target material"("Mn" ("R DC Target material")) -> ()
      }
      frame #55 {
        n1681 = local write "R Single RF Target material"("MnS" ("R DC Target material")) -> ()
      }
      frame #56 {
        n1682 = local write "R Single RF Target material"("Mo" ("R DC Target material")) -> ()
      }
      frame #57 {
        n1683 = local write "R Single RF Target material"("Na" ("R DC Target material")) -> ()
      }
      frame #58 {
        n1684 = local write "R Single RF Target material"("NaCl" ("R DC Target material")) -> ()
      }
      frame #59 {
        n1685 = local write "R Single RF Target material"("NdF3" ("R DC Target material")) -> ()
      }
      frame #60 {
        n1686 = local write "R Single RF Target material"("Nd2O3" ("R DC Target material")) -> ()
      }
      frame #61 {
        n1687 = local write "R Single RF Target material"("Ni" ("R DC Target material")) -> ()
      }
      frame #62 {
        n1688 = local write "R Single RF Target material"("Nb" ("R DC Target material")) -> ()
      }
      frame #63 {
        n1689 = local write "R Single RF Target material"("Nb2O5" ("R DC Target material")) -> ()
      }
      frame #64 {
        n1690 = local write "R Single RF Target material"("Pb" ("R DC Target material")) -> ()
      }
      frame #65 {
        n1691 = local write "R Single RF Target material"("PbS" ("R DC Target material")) -> ()
      }
      frame #66 {
        n1692 = local write "R Single RF Target material"("Pd" ("R DC Target material")) -> ()
      }
      frame #67 {
        n1693 = local write "R Single RF Target material"("Pt" ("R DC Target material")) -> ()
      }
      frame #68 {
        n1694 = local write "R Single RF Target material"("Re" ("R DC Target material")) -> ()
      }
      frame #69 {
        n1695 = local write "R Single RF Target material"("Rh" ("R DC Target material")) -> ()
      }
      frame #70 {
        n1696 = local write "R Single RF Target material"("Rb" ("R DC Target material")) -> ()
      }
      frame #71 {
        n1697 = local write "R Single RF Target material"("S" ("R DC Target material")) -> ()
      }
      frame #72 {
        n1698 = local write "R Single RF Target material"("Sb" ("R DC Target material")) -> ()
      }
      frame #73 {
        n1699 = local write "R Single RF Target material"("Sc" ("R DC Target material")) -> ()
      }
      frame #74 {
        n1700 = local write "R Single RF Target material"("Se" ("R DC Target material")) -> ()
      }
      frame #75 {
        n1701 = local write "R Single RF Target material"("Si" ("R DC Target material")) -> ()
      }
      frame #76 {
        n1702 = local write "R Single RF Target material"("SiO" ("R DC Target material")) -> ()
      }
      frame #77 {
        n1703 = local write "R Single RF Target material"("SiO2" ("R DC Target material")) -> ()
      }
      frame #78 {
        n1704 = local write "R Single RF Target material"("Sm" ("R DC Target material")) -> ()
      }
      frame #79 {
        n1705 = local write "R Single RF Target material"("Sn" ("R DC Target material")) -> ()
      }
      frame #80 {
        n1706 = local write "R Single RF Target material"("Ta" ("R DC Target material")) -> ()
      }
      frame #81 {
        n1707 = local write "R Single RF Target material"("Ta2O5" ("R DC Target material")) -> ()
      }
      frame #82 {
        n1708 = local write "R Single RF Target material"("Te" ("R DC Target material")) -> ()
      }
      frame #83 {
        n1709 = local write "R Single RF Target material"("Tb" ("R DC Target material")) -> ()
      }
      frame #84 {
        n1710 = local write "R Single RF Target material"("ThF4" ("R DC Target material")) -> ()
      }
      frame #85 {
        n1711 = local write "R Single RF Target material"("Ti" ("R DC Target material")) -> ()
      }
      frame #86 {
        n1712 = local write "R Single RF Target material"("TiO2" ("R DC Target material")) -> ()
      }
      frame #87 {
        n1713 = local write "R Single RF Target material"("TiO" ("R DC Target material")) -> ()
      }
      frame #88 {
        n1714 = local write "R Single RF Target material"("Tl" ("R DC Target material")) -> ()
      }
      frame #89 {
        n1715 = local write "R Single RF Target material"("U" ("R DC Target material")) -> ()
      }
      frame #90 {
        n1716 = local write "R Single RF Target material"("V" ("R DC Target material")) -> ()
      }
      frame #91 {
        n1717 = local write "R Single RF Target material"("W" ("R DC Target material")) -> ()
      }
      frame #92 {
        n1718 = local write "R Single RF Target material"("WC" ("R DC Target material")) -> ()
      }
      frame #93 {
        n1719 = local write "R Single RF Target material"("Y" ("R DC Target material")) -> ()
      }
      frame #94 {
        n1720 = local write "R Single RF Target material"("Y2O3" ("R DC Target material")) -> ()
      }
      frame #95 {
        n1721 = local write "R Single RF Target material"("Yb" ("R DC Target material")) -> ()
      }
      frame #96 {
        n1722 = local write "R Single RF Target material"("Zn" ("R DC Target material")) -> ()
      }
      frame #97 {
        n1723 = local write "R Single RF Target material"("ZnO" ("R DC Target material")) -> ()
      }
      frame #98 {
        n1724 = local write "R Single RF Target material"("ZnSe" ("R DC Target material")) -> ()
      }
      frame #99 {
        n1725 = local write "R Single RF Target material"("ZnS" ("R DC Target material")) -> ()
      }
      frame #100 {
        n1726 = local write "R Single RF Target material"("Zr" ("R DC Target material")) -> ()
      }
      frame #101 {
        n1727 = local write "R Single RF Target material"("ZrO2" ("R DC Target material")) -> ()
      }
      frame #102 {
        n1728 = local write "R Single RF Target material"("Si3N4" ("R DC Target material")) -> ()
      }
      frame #103 {
        n1729 = local write "R Single RF Target material"("ITO" ("R DC Target material")) -> ()
      }
      frame #104 {
        n1730 = local write "R Single RF Target material"("PbI2" ("R DC Target material")) -> ()
      }
    }
    n1731 = case shown="104" "R Cmb Ch3 Mat_sel" {
      frame #0 {
      }
      frame #1 {
        n1732 = local write "R Cmb Ch3 Target material"("Ag" ("R DC Target material")) -> ()
      }
      frame #2 {
        n1733 = local write "R Cmb Ch3 Target material"("AgBr" ("R DC Target material")) -> ()
      }
      frame #3 {
        n1734 = local write "R Cmb Ch3 Target material"("AgCl" ("R DC Target material")) -> ()
      }
      frame #4 {
        n1735 = local write "R Cmb Ch3 Target material"("Al" ("R DC Target material")) -> ()
      }
      frame #5 {
        n1736 = local write "R Cmb Ch3 Target material"("Al2O3" ("R DC Target material")) -> ()
      }
      frame #6 {
        n1737 = local write "R Cmb Ch3 Target material"("As" ("R DC Target material")) -> ()
      }
      frame #7 {
        n1738 = local write "R Cmb Ch3 Target material"("Au" ("R DC Target material")) -> ()
      }
      frame #8 {
        n1739 = local write "R Cmb Ch3 Target material"("B" ("R DC Target material")) -> ()
      }
      frame #9 {
        n1740 = local write "R Cmb Ch3 Target material"("Ba" ("R DC Target material")) -> ()
      }
      frame #10 {
        n1741 = local write "R Cmb Ch3 Target material"("Be" ("R DC Target material")) -> ()
      }
      frame #11 {
        n1742 = local write "R Cmb Ch3 Target material"("Bi" ("R DC Target material")) -> ()
      }
      frame #12 {
        n1743 = local write "R Cmb Ch3 Target material"("Bi2O3" ("R DC Target material")) -> ()
      }
      frame #13 {
        n1744 = local write "R Cmb Ch3 Target material"("C (Diamond)" ("R DC Target material")) -> ()
      }
      frame #14 {
        n1745 = local write "R Cmb Ch3 Target material"("C (Graphite)" ("R DC Target material")) -> ()
      }
      frame #15 {
        n1746 = local write "R Cmb Ch3 Target material"("Ca" ("R DC Target material")) -> ()
      }
      frame #16 {
        n1747 = local write "R Cmb Ch3 Target material"("CaF" ("R DC Target material")) -> ()
      }
      frame #17 {
        n1748 = local write "R Cmb Ch3 Target material"("Cd" ("R DC Target material")) -> ()
      }
      frame #18 {
        n1749 = local write "R Cmb Ch3 Target material"("CdS" ("R DC Target material")) -> ()
      }
      frame #19 {
        n1750 = local write "R Cmb Ch3 Target material"("CdSe" ("R DC Target material")) -> ()
      }
      frame #20 {
        n1751 = local write "R Cmb Ch3 Target material"("CdTe" ("R DC Target material")) -> ()
      }
      frame #21 {
        n1752 = local write "R Cmb Ch3 Target material"("CeF3" ("R DC Target material")) -> ()
      }
      frame #22 {
        n1753 = local write "R Cmb Ch3 Target material"("CeO" ("R DC Target material")) -> ()
      }
      frame #23 {
        n1754 = local write "R Cmb Ch3 Target material"("Cr" ("R DC Target material")) -> ()
      }
      frame #24 {
        n1755 = local write "R Cmb Ch3 Target material"("Cr2O3" ("R DC Target material")) -> ()
      }
      frame #25 {
        n1756 = local write "R Cmb Ch3 Target material"("Co" ("R DC Target material")) -> ()
      }
      frame #26 {
        n1757 = local write "R Cmb Ch3 Target material"("Cu" ("R DC Target material")) -> ()
      }
      frame #27 {
        n1758 = local write "R Cmb Ch3 Target material"("Cu2S (A)" ("R DC Target material")) -> ()
      }
      frame #28 {
        n1759 = local write "R Cmb Ch3 Target material"("Cu2S (B)" ("R DC Target material")) -> ()
      }
      frame #29 {
        n1760 = local write "R Cmb Ch3 Target material"("CuS" ("R DC Target material")) -> ()
      }
      frame #30 {
        n1761 = local write "R Cmb Ch3 Target material"("Dy" ("R DC Target material")) -> ()
      }
      frame #31 {
        n1762 = local write "R Cmb Ch3 Target material"("Er" ("R DC Target material")) -> ()
      }
      frame #32 {
        n1763 = local write "R Cmb Ch3 Target material"("Fe" ("R DC Target material")) -> ()
      }
      frame #33 {
        n1764 = local write "R Cmb Ch3 Target material"("Ga" ("R DC Target material")) -> ()
      }
      frame #34 {
        n1765 = local write "R Cmb Ch3 Target material"("GaAs" ("R DC Target material")) -> ()
      }
      frame #35 {
        n1766 = local write "R Cmb Ch3 Target material"("Gd" ("R DC Target material")) -> ()
      }
      frame #36 {
        n1767 = local write "R Cmb Ch3 Target material"("Ge" ("R DC Target material")) -> ()
      }
      frame #37 {
        n1768 = local write "R Cmb Ch3 Target material"("Hf" ("R DC Target material")) -> ()
      }
      frame #38 {
        n1769 = local write "R Cmb Ch3 Target material"("HfO2" ("R DC Target material")) -> ()
      }
      frame #39 {
        n1770 = local write "R Cmb Ch3 Target material"("Hg" ("R DC Target material")) -> ()
      }
      frame #40 {
        n1771 = local write "R Cmb Ch3 Target material"("Ho" ("R DC Target material")) -> ()
      }
      frame #41 {
        n1772 = local write "R Cmb Ch3 Target material"("In" ("R DC Target material")) -> ()
      }
      frame #42 {
        n1773 = local write "R Cmb Ch3 Target material"("InSb" ("R DC Target material")) -> ()
      }
      frame #43 {
        n1774 = local write "R Cmb Ch3 Target material"("In2O3" ("R DC Target material")) -> ()
      }
      frame #44 {
        n1775 = local write "R Cmb Ch3 Target material"("Ir" ("R DC Target material")) -> ()
      }
      frame #45 {
        n1776 = local write "R Cmb Ch3 Target material"("KCl" ("R DC Target material")) -> ()
      }
      frame #46 {
        n1777 = local write "R Cmb Ch3 Target material"("La" ("R DC Target material")) -> ()
      }
      frame #47 {
        n1778 = local write "R Cmb Ch3 Target material"("LaF3" ("R DC Target material")) -> ()
      }
      frame #48 {
        n1779 = local write "R Cmb Ch3 Target material"("LaO3" ("R DC Target material")) -> ()
      }
      frame #49 {
        n1780 = local write "R Cmb Ch3 Target material"("Li" ("R DC Target material")) -> ()
      }
      frame #50 {
        n1781 = local write "R Cmb Ch3 Target material"("LiF" ("R DC Target material")) -> ()
      }
      frame #51 {
        n1782 = local write "R Cmb Ch3 Target material"("Mg" ("R DC Target material")) -> ()
      }
      frame #52 {
        n1783 = local write "R Cmb Ch3 Target material"("MgF2" ("R DC Target material")) -> ()
      }
      frame #53 {
        n1784 = local write "R Cmb Ch3 Target material"("MgO" ("R DC Target material")) -> ()
      }
      frame #54 {
        n1785 = local write "R Cmb Ch3 Target material"("Mn" ("R DC Target material")) -> ()
      }
      frame #55 {
        n1786 = local write "R Cmb Ch3 Target material"("MnS" ("R DC Target material")) -> ()
      }
      frame #56 {
        n1787 = local write "R Cmb Ch3 Target material"("Mo" ("R DC Target material")) -> ()
      }
      frame #57 {
        n1788 = local write "R Cmb Ch3 Target material"("Na" ("R DC Target material")) -> ()
      }
      frame #58 {
        n1789 = local write "R Cmb Ch3 Target material"("NaCl" ("R DC Target material")) -> ()
      }
      frame #59 {
        n1790 = local write "R Cmb Ch3 Target material"("NdF3" ("R DC Target material")) -> ()
      }
      frame #60 {
        n1791 = local write "R Cmb Ch3 Target material"("Nd2O3" ("R DC Target material")) -> ()
      }
      frame #61 {
        n1792 = local write "R Cmb Ch3 Target material"("Ni" ("R DC Target material")) -> ()
      }
      frame #62 {
        n1793 = local write "R Cmb Ch3 Target material"("Nb" ("R DC Target material")) -> ()
      }
      frame #63 {
        n1794 = local write "R Cmb Ch3 Target material"("Nb2O5" ("R DC Target material")) -> ()
      }
      frame #64 {
        n1795 = local write "R Cmb Ch3 Target material"("Pb" ("R DC Target material")) -> ()
      }
      frame #65 {
        n1796 = local write "R Cmb Ch3 Target material"("PbS" ("R DC Target material")) -> ()
      }
      frame #66 {
        n1797 = local write "R Cmb Ch3 Target material"("Pd" ("R DC Target material")) -> ()
      }
      frame #67 {
        n1798 = local write "R Cmb Ch3 Target material"("Pt" ("R DC Target material")) -> ()
      }
      frame #68 {
        n1799 = local write "R Cmb Ch3 Target material"("Re" ("R DC Target material")) -> ()
      }
      frame #69 {
        n1800 = local write "R Cmb Ch3 Target material"("Rh" ("R DC Target material")) -> ()
      }
      frame #70 {
        n1801 = local write "R Cmb Ch3 Target material"("Rb" ("R DC Target material")) -> ()
      }
      frame #71 {
        n1802 = local write "R Cmb Ch3 Target material"("S" ("R DC Target material")) -> ()
      }
      frame #72 {
        n1803 = local write "R Cmb Ch3 Target material"("Sb" ("R DC Target material")) -> ()
      }
      frame #73 {
        n1804 = local write "R Cmb Ch3 Target material"("Sc" ("R DC Target material")) -> ()
      }
      frame #74 {
        n1805 = local write "R Cmb Ch3 Target material"("Se" ("R DC Target material")) -> ()
      }
      frame #75 {
        n1806 = local write "R Cmb Ch3 Target material"("Si" ("R DC Target material")) -> ()
      }
      frame #76 {
        n1807 = local write "R Cmb Ch3 Target material"("SiO" ("R DC Target material")) -> ()
      }
      frame #77 {
        n1808 = local write "R Cmb Ch3 Target material"("SiO2" ("R DC Target material")) -> ()
      }
      frame #78 {
        n1809 = local write "R Cmb Ch3 Target material"("Sm" ("R DC Target material")) -> ()
      }
      frame #79 {
        n1810 = local write "R Cmb Ch3 Target material"("Sn" ("R DC Target material")) -> ()
      }
      frame #80 {
        n1811 = local write "R Cmb Ch3 Target material"("Ta" ("R DC Target material")) -> ()
      }
      frame #81 {
        n1812 = local write "R Cmb Ch3 Target material"("Ta2O5" ("R DC Target material")) -> ()
      }
      frame #82 {
        n1813 = local write "R Cmb Ch3 Target material"("Te" ("R DC Target material")) -> ()
      }
      frame #83 {
        n1814 = local write "R Cmb Ch3 Target material"("Tb" ("R DC Target material")) -> ()
      }
      frame #84 {
        n1815 = local write "R Cmb Ch3 Target material"("ThF4" ("R DC Target material")) -> ()
      }
      frame #85 {
        n1816 = local write "R Cmb Ch3 Target material"("Ti" ("R DC Target material")) -> ()
      }
      frame #86 {
        n1817 = local write "R Cmb Ch3 Target material"("TiO2" ("R DC Target material")) -> ()
      }
      frame #87 {
        n1818 = local write "R Cmb Ch3 Target material"("TiO" ("R DC Target material")) -> ()
      }
      frame #88 {
        n1819 = local write "R Cmb Ch3 Target material"("Tl" ("R DC Target material")) -> ()
      }
      frame #89 {
        n1820 = local write "R Cmb Ch3 Target material"("U" ("R DC Target material")) -> ()
      }
      frame #90 {
        n1821 = local write "R Cmb Ch3 Target material"("V" ("R DC Target material")) -> ()
      }
      frame #91 {
        n1822 = local write "R Cmb Ch3 Target material"("W" ("R DC Target material")) -> ()
      }
      frame #92 {
        n1823 = local write "R Cmb Ch3 Target material"("WC" ("R DC Target material")) -> ()
      }
      frame #93 {
        n1824 = local write "R Cmb Ch3 Target material"("Y" ("R DC Target material")) -> ()
      }
      frame #94 {
        n1825 = local write "R Cmb Ch3 Target material"("Y2O3" ("R DC Target material")) -> ()
      }
      frame #95 {
        n1826 = local write "R Cmb Ch3 Target material"("Yb" ("R DC Target material")) -> ()
      }
      frame #96 {
        n1827 = local write "R Cmb Ch3 Target material"("Zn" ("R DC Target material")) -> ()
      }
      frame #97 {
        n1828 = local write "R Cmb Ch3 Target material"("ZnO" ("R DC Target material")) -> ()
      }
      frame #98 {
        n1829 = local write "R Cmb Ch3 Target material"("ZnSe" ("R DC Target material")) -> ()
      }
      frame #99 {
        n1830 = local write "R Cmb Ch3 Target material"("ZnS" ("R DC Target material")) -> ()
      }
      frame #100 {
        n1831 = local write "R Cmb Ch3 Target material"("Zr" ("R DC Target material")) -> ()
      }
      frame #101 {
        n1832 = local write "R Cmb Ch3 Target material"("ZrO2" ("R DC Target material")) -> ()
      }
      frame #102 {
        n1833 = local write "R Cmb Ch3 Target material"("Si3N4" ("R DC Target material")) -> ()
      }
      frame #103 {
        n1834 = local write "R Cmb Ch3 Target material"("ITO" ("R DC Target material")) -> ()
      }
      frame #104 {
        n1835 = local write "R Cmb Ch3 Target material"("PbI2" ("R DC Target material")) -> ()
      }
    }
    n1836 = local read "R Cmb Step9 Coating Power Active"() -> (w9:bool)
    n1837 = local read "R Cmb Step8 Coating Power Active"() -> (w10:bool)
    n1838 = case shown="True" w12 {
      frame #0 {
        w229 = FALSE ("R Cmb Step3 Coating Power Active")
        n1839 = local write "R Cmb Step7 Coating Power Active"(w229) -> ()
        n1840 = local write "R Cmb Step8 Coating Power Active"(w229) -> ()
        n1841 = local write "R Cmb Step9 Coating Power Active"(w229) -> ()
        n1842 = local write "R Cmb Step10 Coating Power Active"(w229) -> ()
      }
      frame #1 {
        n1843 = local read "R Cmb Step7 Coating Power Active"() -> (w230:bool)
        n1844 = case shown="False" w230 {
          frame #0 {
            w231 = 0.0 ("R Cmb Ch2 Step7 Coating Power")
            w232 = T5."Disabled and Grayed Out" ("Disabled")
            n1845 = local write "R Cmb Ch3 Step7 Coating Power"(w231) -> ()
            n1846 = local write "R Cmb Ch2 Step7 Coating Power"(w231) -> ()
            n1847 = local write "R Cmb Interval length 7"(w231) -> ()
            n1848 = property on="R Cmb Ch3 Step7 Coating Power" class="DigNum (strict)"("DisabledEnum"=w232) -> ()  [unwired: 2 in, 2 out]
            n1849 = property on="R Cmb Interval length 7" class="DigNum (strict)"("DisabledEnum"=w232) -> ()  [unwired: 2 in, 2 out]
            n1850 = property on="R Cmb Ch2 Step7 Coating Power" class="DigNum (strict)"("DisabledEnum"=w232) -> ()  [unwired: 2 in, 2 out]
          }
          frame #1 {
            w233 = T5."Enabled" ("Disabled")
            n1851 = property on="R Cmb Ch3 Step7 Coating Power" class="DigNum (strict)"("DisabledEnum"=w233) -> ()  [unwired: 2 in, 2 out]
            n1852 = property on="R Cmb Interval length 7" class="DigNum (strict)"("DisabledEnum"=w233) -> ()  [unwired: 2 in, 2 out]
            n1853 = property on="R Cmb Ch2 Step7 Coating Power" class="DigNum (strict)"("DisabledEnum"=w233) -> ()  [unwired: 2 in, 2 out]
          }
        }
      }
    }
    n1854 = case shown="True" w11 {
      frame #0 {
        w224 = FALSE ("R Cmb Step3 Coating Power Active")
        n1855 = local write "R Cmb Step8 Coating Power Active"(w224) -> ()
        n1856 = local write "R Cmb Step9 Coating Power Active"(w224) -> ()
        n1857 = local write "R Cmb Step10 Coating Power Active"(w224) -> ()
      }
      frame #1 {
        n1858 = local read "R Cmb Step8 Coating Power Active"() -> (w225:bool)
        n1859 = case shown="False" w225 {
          frame #0 {
            w226 = 0.0 ("R Cmb Ch2 Step8 Coating Power")
            w227 = T5."Disabled and Grayed Out" ("Disabled")
            n1860 = local write "R Cmb Ch3 Step8 Coating Power"(w226) -> ()
            n1861 = local write "R Cmb Ch2 Step8 Coating Power"(w226) -> ()
            n1862 = local write "R Cmb Interval length 8"(w226) -> ()
            n1863 = property on="R Cmb Ch2 Step8 Coating Power" class="DigNum (strict)"("DisabledEnum"=w227) -> ()  [unwired: 2 in, 2 out]
            n1864 = property on="R Cmb Ch3 Step8 Coating Power" class="DigNum (strict)"("DisabledEnum"=w227) -> ()  [unwired: 2 in, 2 out]
            n1865 = property on="R Cmb Interval length 8" class="DigNum (strict)"("DisabledEnum"=w227) -> ()  [unwired: 2 in, 2 out]
          }
          frame #1 {
            w228 = T5."Enabled" ("Disabled")
            n1866 = property on="R Cmb Ch2 Step8 Coating Power" class="DigNum (strict)"("DisabledEnum"=w228) -> ()  [unwired: 2 in, 2 out]
            n1867 = property on="R Cmb Ch3 Step8 Coating Power" class="DigNum (strict)"("DisabledEnum"=w228) -> ()  [unwired: 2 in, 2 out]
            n1868 = property on="R Cmb Interval length 8" class="DigNum (strict)"("DisabledEnum"=w228) -> ()  [unwired: 2 in, 2 out]
          }
        }
      }
    }
    n1869 = case shown="True" w13 {
      frame #0 {
        w234 = FALSE ("R Cmb Step3 Coating Power Active")
        n1870 = local write "R Cmb Step6 Coating Power Active"(w234) -> ()
        n1871 = local write "R Cmb Step7 Coating Power Active"(w234) -> ()
        n1872 = local write "R Cmb Step8 Coating Power Active"(w234) -> ()
        n1873 = local write "R Cmb Step9 Coating Power Active"(w234) -> ()
        n1874 = local write "R Cmb Step10 Coating Power Active"(w234) -> ()
      }
      frame #1 {
        n1875 = local read "R Cmb Step6 Coating Power Active"() -> (w235:bool)
        n1876 = case shown="False" w235 {
          frame #0 {
            w236 = 0.0 ("R Cmb Ch2 Step6 Coating Power")
            w237 = T5."Disabled and Grayed Out" ("Disabled")
            n1877 = local write "R Cmb Ch2 Step6 Coating Power"(w236) -> ()
            n1878 = local write "R Cmb Ch3 Step6 Coating Power"(w236) -> ()
            n1879 = local write "R Cmb Interval length 6"(w236) -> ()
            n1880 = property on="R Cmb Ch2 Step6 Coating Power" class="DigNum (strict)"("DisabledEnum"=w237) -> ()  [unwired: 2 in, 2 out]
            n1881 = property on="R Cmb Ch3 Step6 Coating Power" class="DigNum (strict)"("DisabledEnum"=w237) -> ()  [unwired: 2 in, 2 out]
            n1882 = property on="R Cmb Interval length 6" class="DigNum (strict)"("DisabledEnum"=w237) -> ()  [unwired: 2 in, 2 out]
          }
          frame #1 {
            w238 = T5."Enabled" ("Disabled")
            n1883 = property on="R Cmb Ch2 Step6 Coating Power" class="DigNum (strict)"("DisabledEnum"=w238) -> ()  [unwired: 2 in, 2 out]
            n1884 = property on="R Cmb Ch3 Step6 Coating Power" class="DigNum (strict)"("DisabledEnum"=w238) -> ()  [unwired: 2 in, 2 out]
            n1885 = property on="R Cmb Interval length 6" class="DigNum (strict)"("DisabledEnum"=w238) -> ()  [unwired: 2 in, 2 out]
          }
        }
      }
    }
    n1886 = case shown="True" w9 {
      frame #0 {
        n1887 = local write "R Cmb Step10 Coating Power Active"(FALSE ("R Cmb Step3 Coating Power Active")) -> ()
      }
      frame #1 {
        n1888 = local read "R Cmb Step10 Coating Power Active"() -> (w220:bool)
        n1889 = case shown="False" w220 {
          frame #0 {
            w221 = 0.0 ("R Cmb Ch2 Step10 Coating Power")
            w222 = T5."Disabled and Grayed Out" ("Disabled")
            n1890 = local write "R Cmb Ch2 Step10 Coating Power"(w221) -> ()
            n1891 = local write "R Cmb Ch3 Step10 Coating Power"(w221) -> ()
            n1892 = local write "R Cmb Interval length 10"(w221) -> ()
            n1893 = property on="R Cmb Ch2 Step10 Coating Power" class="DigNum (strict)"("DisabledEnum"=w222) -> ()  [unwired: 2 in, 2 out]
            n1894 = property on="R Cmb Ch3 Step10 Coating Power" class="DigNum (strict)"("DisabledEnum"=w222) -> ()  [unwired: 2 in, 2 out]
            n1895 = property on="R Cmb Interval length 10" class="DigNum (strict)"("DisabledEnum"=w222) -> ()  [unwired: 2 in, 2 out]
          }
          frame #1 {
            w223 = T5."Enabled" ("Disabled")
            n1896 = property on="R Cmb Ch2 Step10 Coating Power" class="DigNum (strict)"("DisabledEnum"=w223) -> ()  [unwired: 2 in, 2 out]
            n1897 = property on="R Cmb Ch3 Step10 Coating Power" class="DigNum (strict)"("DisabledEnum"=w223) -> ()  [unwired: 2 in, 2 out]
            n1898 = property on="R Cmb Interval length 10" class="DigNum (strict)"("DisabledEnum"=w223) -> ()  [unwired: 2 in, 2 out]
          }
        }
      }
    }
    n1899 = case shown="True" w10 {
      frame #0 {
        w214 = FALSE ("R Cmb Step3 Coating Power Active")
        n1900 = local write "R Cmb Step9 Coating Power Active"(w214) -> ()
        n1901 = local write "R Cmb Step10 Coating Power Active"(w214) -> ()
      }
      frame #1 {
        n1902 = local read "R Cmb Step9 Coating Power Active"() -> (w215:bool)
        n1903 = case shown="False" w215 {
          frame #0 {
            w216 = 0.0 ("R Cmb Ch2 Step9 Coating Power")
            w217 = T5."Disabled and Grayed Out" ("Disabled")
            n1904 = local write "R Cmb Ch3 Step9 Coating Power"(w216) -> ()
            n1905 = local write "R Cmb Ch2 Step9 Coating Power"(w216) -> ()
            n1906 = local write "R Cmb Interval length 9"(w216) -> ()
            n1907 = property on="R Cmb Ch2 Step9 Coating Power" class="DigNum (strict)"("DisabledEnum"=w217) -> ()  [unwired: 2 in, 2 out]
            n1908 = property on="R Cmb Ch3 Step9 Coating Power" class="DigNum (strict)"("DisabledEnum"=w217) -> ()  [unwired: 2 in, 2 out]
            n1909 = property on="R Cmb Interval length 9" class="DigNum (strict)"("DisabledEnum"=w217) -> ()  [unwired: 2 in, 2 out]
          }
          frame #1 {
            w218 = T5."Enabled" ("Disabled")
            n1910 = property on="R Cmb Ch2 Step9 Coating Power" class="DigNum (strict)"("DisabledEnum"=w218) -> ()  [unwired: 2 in, 2 out]
            n1911 = property on="R Cmb Ch3 Step9 Coating Power" class="DigNum (strict)"("DisabledEnum"=w218) -> ()  [unwired: 2 in, 2 out]
            n1912 = property on="R Cmb Interval length 9" class="DigNum (strict)"("DisabledEnum"=w218) -> ()  [unwired: 2 in, 2 out]
          }
        }
      }
    }
    n1913 = Or(x=w38, y="Cancel") -> (x .or. y?=w36:bool)
    n1914 = stacked-sequence {
      frame #0 {
        # "Recipe Parameters"
      }
    }
    "Process_flow" <- "Recommended Ar  Value is  20 sccm !" ("Process_flow")
    "Process_flow 2" <- "Recommended Ar  Value is  200 sccm !" ("Process_flow")
  }
  "OKTO" <- w2
  n1915 = invoke class="VI" method="Default Vals.Reinit All"() -> (error out=w4:errorcluster)  [unwired: 3 in, 2 out]
  n1916 = property on="Recipe Name" class="Str"(error in=w4, "Key Focus"=TRUE) -> ()  [unwired: 1 in, 2 out]
  n1917 = case shown="True" w2 {
    tunnel: [errorcluster {"status"=FALSE, "code"=0, "source"=""} ("error out") w1703] -> w1
    frame #0 {
    }
    frame #1 {
      n1918 = stacked-sequence {
        seq-local: [w1710 _] -> [_ w1907]
        seq-local: [w1709 _] -> [_ w1903]
        seq-local: [w1708 _] -> [_ w1909]
        seq-local: [w1707 _] -> [_ w1904]
        seq-local: [w1705 _] -> [_ w1897]
        seq-local: [w1704 _] -> [_ w1900]
        tunnel: [_ w1908] -> w1703
        tunnel: [_ w1902] -> _
        tunnel: [_ w1899] -> _
        frame #0 {
          n1919 = File Dialog(9:"Recipe Name", 11:path "D:/System Files/Recipe" ("start path")) -> (3:w1717:path)  [unwired: 2 in, 6 out]
          n1920 = Build Path(base path=path "D:/System Files/Recipe" ("start path"), name or relative path="Recipe Name") -> (appended path=w1716:path)
          n1921 = Open/Create/Replace File(file path (use dialog)=w1716, operation (0:open)=T6."replace or create", access (0:read/write)=enum16{"read/write", "read-only", "write-only"}."read/write") -> (refnum out=w1707:refnum<file>, cancelled=w1714:bool, error out=w1712:errorcluster)  [unwired: 3 in]
          n1922 = Open/Create/Replace File(file path (use dialog)=w1717, operation (0:open)=T6."replace or create", access (0:read/write)=enum16{"read/write", "read-only", "write-only"}."read/write") -> (refnum out=w1708:refnum<file>, cancelled=w1720:bool, error out=w1722:errorcluster)  [unwired: 3 in]
          n1923 = stacked-sequence {
            tunnel: "Recipe Name" -> [_ w1728 _]
            tunnel: [_ w1727 _] -> w1705
            tunnel: [_ w1726 _] -> w1704
            frame #0 {
              n1924 = Wait (ms)(milliseconds to wait=u32 50) -> ()  [unwired: 1 out]
              n1925 = dll-call lib="kernel32.dll" fn="SetFileAttributesA"("lpFileName"="D:\\System Files\\Recipe Archive", "dwFileAttributes"=u32 128) -> ()  [unwired: 6 in, 2 out]
            }
            frame #1 {
              n1926 = Build Path(base path=path "D:/System Files/Recipe Archive" ("start path"), name or relative path=w1728) -> (appended path=w1729:path)
              n1927 = Open/Create/Replace File(file path (use dialog)=w1729, operation (0:open)=T6."replace or create", access (0:read/write)=enum16{"read/write", "read-only", "write-only"}."read/write") -> (refnum out=w1727:refnum<file>, cancelled=w1731:bool, error out=w1733:errorcluster)  [unwired: 3 in]
              n1928 = case shown="True" w1731 {
                tunnel: w1727 -> [_ w1738]
                tunnel: w1733 -> [_ w1737]
                tunnel: [errorcluster {"status"=FALSE, "code"=0, "source"=""} ("error out") w1736] -> w1726
                frame #0 {
                }
                frame #1 {
                  n1929 = Close File(refnum=w1738, error in=w1737) -> (error out=w1736:errorcluster)  [unwired: 1 out]
                }
              }
            }
            frame #2 {
              n1930 = Wait (ms)(milliseconds to wait=u32 50) -> ()  [unwired: 1 out]
              n1931 = dll-call lib="kernel32.dll" fn="SetFileAttributesA"("lpFileName"="D:\\System Files\\Recipe Archive", "dwFileAttributes"=u32 2) -> ()  [unwired: 6 in, 2 out]
            }
          }
          n1932 = case shown="False" w1714 {
            tunnel: w1707 -> [_ w1745]
            tunnel: w1712 -> [_ w1744]
            tunnel: [errorcluster {"status"=FALSE, "code"=0, "source"=""} ("error out") w1743] -> w1709
            frame #0 {
            }
            frame #1 {
              n1933 = Close File(refnum=w1745, error in=w1744) -> (error out=w1743:errorcluster)  [unwired: 1 out]
            }
          }
          n1934 = case shown="True" w1720 {
            tunnel: w1708 -> [_ w1749]
            tunnel: w1722 -> [_ w1748]
            tunnel: [errorcluster {"status"=FALSE, "code"=0, "source"=""} ("error out") w1747] -> w1710
            frame #0 {
            }
            frame #1 {
              n1935 = Close File(refnum=w1749, error in=w1748) -> (error out=w1747:errorcluster)  [unwired: 1 out]
            }
          }
        }
        frame #1 {
          n1936 = stacked-sequence {
            tunnel: [w1912 _ _ _ _ _ _ _ _ _ _ _ _ _ _ _ _ _ _ _ _ _ _ _ _ _ _ _ _ _ _ _ _ _ _ _ _ _ _ _ _ _ _ _ _ _ _ _ _ _ _ _ _ _ _ _ _ _ _ _ _ _ _ _ _ _ _ _ _ _ _ _ _ _ _ _ _ _ _ _ _ _ _ _ _ _ _ _ _ _ _ _ _ _ _ _ _ _ _ _ _ _ _ _ _ _ _ _ _ _ _ _ _ _ _ _ _ _ _ _ _ _ _ _ _ _ _ _ _ _ _ _ _ _ _ _ _ _ _ _ _ _ _ _ _ _] -> w1895
            tunnel: [_ w1919 _ _ _ _ _ _ _ _ _ _ _ _ _ _ _ _ _ _ _ _ _ _ _ _ _ _ _ _ _ _ _ _ _ _ _ _ _ _ _ _ _ _ _ _ _ _ _ _ _ _ _ _ _ _ _ _ _ _ _ _ _ _ _ _ _ _ _ _ _ _ _ _ _ _ _ _ _ _ _ _ _ _ _ _ _ _ _ _ _ _ _ _ _ _ _ _ _ _ _ _ _ _ _ _ _ _ _ _ _ _ _ _ _ _ _ _ _ _ _ _ _ _ _ _ _ _ _ _ _ _ _ _ _ _ _ _ _ _ _ _ _ _ _ _] -> w1894
            tunnel: [_ _ w1926 _ _ _ _ _ _ _ _ _ _ _ _ _ _ _ _ _ _ _ _ _ _ _ _ _ _ _ _ _ _ _ _ _ _ _ _ _ _ _ _ _ _ _ _ _ _ _ _ _ _ _ _ _ _ _ _ _ _ _ _ _ _ _ _ _ _ _ _ _ _ _ _ _ _ _ _ _ _ _ _ _ _ _ _ _ _ _ _ _ _ _ _ _ _ _ _ _ _ _ _ _ _ _ _ _ _ _ _ _ _ _ _ _ _ _ _ _ _ _ _ _ _ _ _ _ _ _ _ _ _ _ _ _ _ _ _ _ _ _ _ _ _ _] -> w1893
            tunnel: [_ _ _ w1935 _ _ _ _ _ _ _ _ _ _ _ _ _ _ _ _ _ _ _ _ _ _ _ _ _ _ _ _ _ _ _ _ _ _ _ _ _ _ _ _ _ _ _ _ _ _ _ _ _ _ _ _ _ _ _ _ _ _ _ _ _ _ _ _ _ _ _ _ _ _ _ _ _ _ _ _ _ _ _ _ _ _ _ _ _ _ _ _ _ _ _ _ _ _ _ _ _ _ _ _ _ _ _ _ _ _ _ _ _ _ _ _ _ _ _ _ _ _ _ _ _ _ _ _ _ _ _ _ _ _ _ _ _ _ _ _ _ _ _ _ _ _] -> w1892
            tunnel: [_ _ _ _ w1944 _ _ _ _ _ _ _ _ _ _ _ _ _ _ _ _ _ _ _ _ _ _ _ _ _ _ _ _ _ _ _ _ _ _ _ _ _ _ _ _ _ _ _ _ _ _ _ _ _ _ _ _ _ _ _ _ _ _ _ _ _ _ _ _ _ _ _ _ _ _ _ _ _ _ _ _ _ _ _ _ _ _ _ _ _ _ _ _ _ _ _ _ _ _ _ _ _ _ _ _ _ _ _ _ _ _ _ _ _ _ _ _ _ _ _ _ _ _ _ _ _ _ _ _ _ _ _ _ _ _ _ _ _ _ _ _ _ _ _ _ _] -> w1891
            tunnel: [_ _ _ _ _ w1948 _ _ _ _ _ _ _ _ _ _ _ _ _ _ _ _ _ _ _ _ _ _ _ _ _ _ _ _ _ _ _ _ _ _ _ _ _ _ _ _ _ _ _ _ _ _ _ _ _ _ _ _ _ _ _ _ _ _ _ _ _ _ _ _ _ _ _ _ _ _ _ _ _ _ _ _ _ _ _ _ _ _ _ _ _ _ _ _ _ _ _ _ _ _ _ _ _ _ _ _ _ _ _ _ _ _ _ _ _ _ _ _ _ _ _ _ _ _ _ _ _ _ _ _ _ _ _ _ _ _ _ _ _ _ _ _ _ _ _ _] -> w1890
            tunnel: [_ _ _ _ _ _ w1954 _ _ _ _ _ _ _ _ _ _ _ _ _ _ _ _ _ _ _ _ _ _ _ _ _ _ _ _ _ _ _ _ _ _ _ _ _ _ _ _ _ _ _ _ _ _ _ _ _ _ _ _ _ _ _ _ _ _ _ _ _ _ _ _ _ _ _ _ _ _ _ _ _ _ _ _ _ _ _ _ _ _ _ _ _ _ _ _ _ _ _ _ _ _ _ _ _ _ _ _ _ _ _ _ _ _ _ _ _ _ _ _ _ _ _ _ _ _ _ _ _ _ _ _ _ _ _ _ _ _ _ _ _ _ _ _ _ _ _] -> w1889
            tunnel: [_ _ _ _ _ _ _ w1960 _ _ _ _ _ _ _ _ _ _ _ _ _ _ _ _ _ _ _ _ _ _ _ _ _ _ _ _ _ _ _ _ _ _ _ _ _ _ _ _ _ _ _ _ _ _ _ _ _ _ _ _ _ _ _ _ _ _ _ _ _ _ _ _ _ _ _ _ _ _ _ _ _ _ _ _ _ _ _ _ _ _ _ _ _ _ _ _ _ _ _ _ _ _ _ _ _ _ _ _ _ _ _ _ _ _ _ _ _ _ _ _ _ _ _ _ _ _ _ _ _ _ _ _ _ _ _ _ _ _ _ _ _ _ _ _ _ _] -> w1888
            tunnel: [_ _ _ _ _ _ _ _ w1966 _ _ _ _ _ _ _ _ _ _ _ _ _ _ _ _ _ _ _ _ _ _ _ _ _ _ _ _ _ _ _ _ _ _ _ _ _ _ _ _ _ _ _ _ _ _ _ _ _ _ _ _ _ _ _ _ _ _ _ _ _ _ _ _ _ _ _ _ _ _ _ _ _ _ _ _ _ _ _ _ _ _ _ _ _ _ _ _ _ _ _ _ _ _ _ _ _ _ _ _ _ _ _ _ _ _ _ _ _ _ _ _ _ _ _ _ _ _ _ _ _ _ _ _ _ _ _ _ _ _ _ _ _ _ _ _ _] -> w1887
            tunnel: [_ _ _ _ _ _ _ _ _ w1972 _ _ _ _ _ _ _ _ _ _ _ _ _ _ _ _ _ _ _ _ _ _ _ _ _ _ _ _ _ _ _ _ _ _ _ _ _ _ _ _ _ _ _ _ _ _ _ _ _ _ _ _ _ _ _ _ _ _ _ _ _ _ _ _ _ _ _ _ _ _ _ _ _ _ _ _ _ _ _ _ _ _ _ _ _ _ _ _ _ _ _ _ _ _ _ _ _ _ _ _ _ _ _ _ _ _ _ _ _ _ _ _ _ _ _ _ _ _ _ _ _ _ _ _ _ _ _ _ _ _ _ _ _ _ _ _] -> w1886
            tunnel: [_ _ _ _ _ _ _ _ _ _ w1978 _ _ _ _ _ _ _ _ _ _ _ _ _ _ _ _ _ _ _ _ _ _ _ _ _ _ _ _ _ _ _ _ _ _ _ _ _ _ _ _ _ _ _ _ _ _ _ _ _ _ _ _ _ _ _ _ _ _ _ _ _ _ _ _ _ _ _ _ _ _ _ _ _ _ _ _ _ _ _ _ _ _ _ _ _ _ _ _ _ _ _ _ _ _ _ _ _ _ _ _ _ _ _ _ _ _ _ _ _ _ _ _ _ _ _ _ _ _ _ _ _ _ _ _ _ _ _ _ _ _ _ _ _ _ _] -> w1885
            tunnel: [_ _ _ _ _ _ _ _ _ _ _ w1985 _ _ _ _ _ _ _ _ _ _ _ _ _ _ _ _ _ _ _ _ _ _ _ _ _ _ _ _ _ _ _ _ _ _ _ _ _ _ _ _ _ _ _ _ _ _ _ _ _ _ _ _ _ _ _ _ _ _ _ _ _ _ _ _ _ _ _ _ _ _ _ _ _ _ _ _ _ _ _ _ _ _ _ _ _ _ _ _ _ _ _ _ _ _ _ _ _ _ _ _ _ _ _ _ _ _ _ _ _ _ _ _ _ _ _ _ _ _ _ _ _ _ _ _ _ _ _ _ _ _ _ _ _ _] -> w1884
            tunnel: [_ _ _ _ _ _ _ _ _ _ _ _ w1990 _ _ _ _ _ _ _ _ _ _ _ _ _ _ _ _ _ _ _ _ _ _ _ _ _ _ _ _ _ _ _ _ _ _ _ _ _ _ _ _ _ _ _ _ _ _ _ _ _ _ _ _ _ _ _ _ _ _ _ _ _ _ _ _ _ _ _ _ _ _ _ _ _ _ _ _ _ _ _ _ _ _ _ _ _ _ _ _ _ _ _ _ _ _ _ _ _ _ _ _ _ _ _ _ _ _ _ _ _ _ _ _ _ _ _ _ _ _ _ _ _ _ _ _ _ _ _ _ _ _ _ _ _] -> w1883
            tunnel: [_ _ _ _ _ _ _ _ _ _ _ _ _ w1998 _ _ _ _ _ _ _ _ _ _ _ _ _ _ _ _ _ _ _ _ _ _ _ _ _ _ _ _ _ _ _ _ _ _ _ _ _ _ _ _ _ _ _ _ _ _ _ _ _ _ _ _ _ _ _ _ _ _ _ _ _ _ _ _ _ _ _ _ _ _ _ _ _ _ _ _ _ _ _ _ _ _ _ _ _ _ _ _ _ _ _ _ _ _ _ _ _ _ _ _ _ _ _ _ _ _ _ _ _ _ _ _ _ _ _ _ _ _ _ _ _ _ _ _ _ _ _ _ _ _ _ _] -> w1882
            tunnel: [_ _ _ _ _ _ _ _ _ _ _ _ _ _ w2004 _ _ _ _ _ _ _ _ _ _ _ _ _ _ _ _ _ _ _ _ _ _ _ _ _ _ _ _ _ _ _ _ _ _ _ _ _ _ _ _ _ _ _ _ _ _ _ _ _ _ _ _ _ _ _ _ _ _ _ _ _ _ _ _ _ _ _ _ _ _ _ _ _ _ _ _ _ _ _ _ _ _ _ _ _ _ _ _ _ _ _ _ _ _ _ _ _ _ _ _ _ _ _ _ _ _ _ _ _ _ _ _ _ _ _ _ _ _ _ _ _ _ _ _ _ _ _ _ _ _ _] -> w1881
            tunnel: [_ _ _ _ _ _ _ _ _ _ _ _ _ _ _ w2011 _ _ _ _ _ _ _ _ _ _ _ _ _ _ _ _ _ _ _ _ _ _ _ _ _ _ _ _ _ _ _ _ _ _ _ _ _ _ _ _ _ _ _ _ _ _ _ _ _ _ _ _ _ _ _ _ _ _ _ _ _ _ _ _ _ _ _ _ _ _ _ _ _ _ _ _ _ _ _ _ _ _ _ _ _ _ _ _ _ _ _ _ _ _ _ _ _ _ _ _ _ _ _ _ _ _ _ _ _ _ _ _ _ _ _ _ _ _ _ _ _ _ _ _ _ _ _ _ _ _] -> w1880
            tunnel: [_ _ _ _ _ _ _ _ _ _ _ _ _ _ _ _ w2018 _ _ _ _ _ _ _ _ _ _ _ _ _ _ _ _ _ _ _ _ _ _ _ _ _ _ _ _ _ _ _ _ _ _ _ _ _ _ _ _ _ _ _ _ _ _ _ _ _ _ _ _ _ _ _ _ _ _ _ _ _ _ _ _ _ _ _ _ _ _ _ _ _ _ _ _ _ _ _ _ _ _ _ _ _ _ _ _ _ _ _ _ _ _ _ _ _ _ _ _ _ _ _ _ _ _ _ _ _ _ _ _ _ _ _ _ _ _ _ _ _ _ _ _ _ _ _ _ _] -> w1879
            tunnel: [_ _ _ _ _ _ _ _ _ _ _ _ _ _ _ _ _ w2026 _ _ _ _ _ _ _ _ _ _ _ _ _ _ _ _ _ _ _ _ _ _ _ _ _ _ _ _ _ _ _ _ _ _ _ _ _ _ _ _ _ _ _ _ _ _ _ _ _ _ _ _ _ _ _ _ _ _ _ _ _ _ _ _ _ _ _ _ _ _ _ _ _ _ _ _ _ _ _ _ _ _ _ _ _ _ _ _ _ _ _ _ _ _ _ _ _ _ _ _ _ _ _ _ _ _ _ _ _ _ _ _ _ _ _ _ _ _ _ _ _ _ _ _ _ _ _ _] -> w1878
            tunnel: [_ _ _ _ _ _ _ _ _ _ _ _ _ _ _ _ _ _ w2030 _ _ _ _ _ _ _ _ _ _ _ _ _ _ _ _ _ _ _ _ _ _ _ _ _ _ _ _ _ _ _ _ _ _ _ _ _ _ _ _ _ _ _ _ _ _ _ _ _ _ _ _ _ _ _ _ _ _ _ _ _ _ _ _ _ _ _ _ _ _ _ _ _ _ _ _ _ _ _ _ _ _ _ _ _ _ _ _ _ _ _ _ _ _ _ _ _ _ _ _ _ _ _ _ _ _ _ _ _ _ _ _ _ _ _ _ _ _ _ _ _ _ _ _ _ _ _] -> w1877
            tunnel: [_ _ _ _ _ _ _ _ _ _ _ _ _ _ _ _ _ _ _ w2036 _ _ _ _ _ _ _ _ _ _ _ _ _ _ _ _ _ _ _ _ _ _ _ _ _ _ _ _ _ _ _ _ _ _ _ _ _ _ _ _ _ _ _ _ _ _ _ _ _ _ _ _ _ _ _ _ _ _ _ _ _ _ _ _ _ _ _ _ _ _ _ _ _ _ _ _ _ _ _ _ _ _ _ _ _ _ _ _ _ _ _ _ _ _ _ _ _ _ _ _ _ _ _ _ _ _ _ _ _ _ _ _ _ _ _ _ _ _ _ _ _ _ _ _ _ _] -> w1876
            tunnel: [_ _ _ _ _ _ _ _ _ _ _ _ _ _ _ _ _ _ _ _ w2044 _ _ _ _ _ _ _ _ _ _ _ _ _ _ _ _ _ _ _ _ _ _ _ _ _ _ _ _ _ _ _ _ _ _ _ _ _ _ _ _ _ _ _ _ _ _ _ _ _ _ _ _ _ _ _ _ _ _ _ _ _ _ _ _ _ _ _ _ _ _ _ _ _ _ _ _ _ _ _ _ _ _ _ _ _ _ _ _ _ _ _ _ _ _ _ _ _ _ _ _ _ _ _ _ _ _ _ _ _ _ _ _ _ _ _ _ _ _ _ _ _ _ _ _ _] -> w1875
            tunnel: [_ _ _ _ _ _ _ _ _ _ _ _ _ _ _ _ _ _ _ _ _ w2049 _ _ _ _ _ _ _ _ _ _ _ _ _ _ _ _ _ _ _ _ _ _ _ _ _ _ _ _ _ _ _ _ _ _ _ _ _ _ _ _ _ _ _ _ _ _ _ _ _ _ _ _ _ _ _ _ _ _ _ _ _ _ _ _ _ _ _ _ _ _ _ _ _ _ _ _ _ _ _ _ _ _ _ _ _ _ _ _ _ _ _ _ _ _ _ _ _ _ _ _ _ _ _ _ _ _ _ _ _ _ _ _ _ _ _ _ _ _ _ _ _ _ _ _] -> w1874
            tunnel: [_ _ _ _ _ _ _ _ _ _ _ _ _ _ _ _ _ _ _ _ _ _ w2054 _ _ _ _ _ _ _ _ _ _ _ _ _ _ _ _ _ _ _ _ _ _ _ _ _ _ _ _ _ _ _ _ _ _ _ _ _ _ _ _ _ _ _ _ _ _ _ _ _ _ _ _ _ _ _ _ _ _ _ _ _ _ _ _ _ _ _ _ _ _ _ _ _ _ _ _ _ _ _ _ _ _ _ _ _ _ _ _ _ _ _ _ _ _ _ _ _ _ _ _ _ _ _ _ _ _ _ _ _ _ _ _ _ _ _ _ _ _ _ _ _ _ _] -> w1873
            tunnel: [_ _ _ _ _ _ _ _ _ _ _ _ _ _ _ _ _ _ _ _ _ _ _ w2064 _ _ _ _ _ _ _ _ _ _ _ _ _ _ _ _ _ _ _ _ _ _ _ _ _ _ _ _ _ _ _ _ _ _ _ _ _ _ _ _ _ _ _ _ _ _ _ _ _ _ _ _ _ _ _ _ _ _ _ _ _ _ _ _ _ _ _ _ _ _ _ _ _ _ _ _ _ _ _ _ _ _ _ _ _ _ _ _ _ _ _ _ _ _ _ _ _ _ _ _ _ _ _ _ _ _ _ _ _ _ _ _ _ _ _ _ _ _ _ _ _ _] -> w1872
            tunnel: [_ _ _ _ _ _ _ _ _ _ _ _ _ _ _ _ _ _ _ _ _ _ _ _ w2069 _ _ _ _ _ _ _ _ _ _ _ _ _ _ _ _ _ _ _ _ _ _ _ _ _ _ _ _ _ _ _ _ _ _ _ _ _ _ _ _ _ _ _ _ _ _ _ _ _ _ _ _ _ _ _ _ _ _ _ _ _ _ _ _ _ _ _ _ _ _ _ _ _ _ _ _ _ _ _ _ _ _ _ _ _ _ _ _ _ _ _ _ _ _ _ _ _ _ _ _ _ _ _ _ _ _ _ _ _ _ _ _ _ _ _ _ _ _ _ _ _] -> w1871
            tunnel: [_ _ _ _ _ _ _ _ _ _ _ _ _ _ _ _ _ _ _ _ _ _ _ _ _ w2078 _ _ _ _ _ _ _ _ _ _ _ _ _ _ _ _ _ _ _ _ _ _ _ _ _ _ _ _ _ _ _ _ _ _ _ _ _ _ _ _ _ _ _ _ _ _ _ _ _ _ _ _ _ _ _ _ _ _ _ _ _ _ _ _ _ _ _ _ _ _ _ _ _ _ _ _ _ _ _ _ _ _ _ _ _ _ _ _ _ _ _ _ _ _ _ _ _ _ _ _ _ _ _ _ _ _ _ _ _ _ _ _ _ _ _ _ _ _ _ _] -> w1870
            tunnel: [_ _ _ _ _ _ _ _ _ _ _ _ _ _ _ _ _ _ _ _ _ _ _ _ _ _ w2084 _ _ _ _ _ _ _ _ _ _ _ _ _ _ _ _ _ _ _ _ _ _ _ _ _ _ _ _ _ _ _ _ _ _ _ _ _ _ _ _ _ _ _ _ _ _ _ _ _ _ _ _ _ _ _ _ _ _ _ _ _ _ _ _ _ _ _ _ _ _ _ _ _ _ _ _ _ _ _ _ _ _ _ _ _ _ _ _ _ _ _ _ _ _ _ _ _ _ _ _ _ _ _ _ _ _ _ _ _ _ _ _ _ _ _ _ _ _ _] -> w1869
            tunnel: [_ _ _ _ _ _ _ _ _ _ _ _ _ _ _ _ _ _ _ _ _ _ _ _ _ _ _ w2090 _ _ _ _ _ _ _ _ _ _ _ _ _ _ _ _ _ _ _ _ _ _ _ _ _ _ _ _ _ _ _ _ _ _ _ _ _ _ _ _ _ _ _ _ _ _ _ _ _ _ _ _ _ _ _ _ _ _ _ _ _ _ _ _ _ _ _ _ _ _ _ _ _ _ _ _ _ _ _ _ _ _ _ _ _ _ _ _ _ _ _ _ _ _ _ _ _ _ _ _ _ _ _ _ _ _ _ _ _ _ _ _ _ _ _ _ _ _] -> w1868
            tunnel: [_ _ _ _ _ _ _ _ _ _ _ _ _ _ _ _ _ _ _ _ _ _ _ _ _ _ _ _ w2099 _ _ _ _ _ _ _ _ _ _ _ _ _ _ _ _ _ _ _ _ _ _ _ _ _ _ _ _ _ _ _ _ _ _ _ _ _ _ _ _ _ _ _ _ _ _ _ _ _ _ _ _ _ _ _ _ _ _ _ _ _ _ _ _ _ _ _ _ _ _ _ _ _ _ _ _ _ _ _ _ _ _ _ _ _ _ _ _ _ _ _ _ _ _ _ _ _ _ _ _ _ _ _ _ _ _ _ _ _ _ _ _ _ _ _ _ _] -> w1867
            tunnel: [_ _ _ _ _ _ _ _ _ _ _ _ _ _ _ _ _ _ _ _ _ _ _ _ _ _ _ _ _ w2105 _ _ _ _ _ _ _ _ _ _ _ _ _ _ _ _ _ _ _ _ _ _ _ _ _ _ _ _ _ _ _ _ _ _ _ _ _ _ _ _ _ _ _ _ _ _ _ _ _ _ _ _ _ _ _ _ _ _ _ _ _ _ _ _ _ _ _ _ _ _ _ _ _ _ _ _ _ _ _ _ _ _ _ _ _ _ _ _ _ _ _ _ _ _ _ _ _ _ _ _ _ _ _ _ _ _ _ _ _ _ _ _ _ _ _ _] -> w1866
            tunnel: [_ _ _ _ _ _ _ _ _ _ _ _ _ _ _ _ _ _ _ _ _ _ _ _ _ _ _ _ _ _ w2111 _ _ _ _ _ _ _ _ _ _ _ _ _ _ _ _ _ _ _ _ _ _ _ _ _ _ _ _ _ _ _ _ _ _ _ _ _ _ _ _ _ _ _ _ _ _ _ _ _ _ _ _ _ _ _ _ _ _ _ _ _ _ _ _ _ _ _ _ _ _ _ _ _ _ _ _ _ _ _ _ _ _ _ _ _ _ _ _ _ _ _ _ _ _ _ _ _ _ _ _ _ _ _ _ _ _ _ _ _ _ _ _ _ _ _] -> w1865
            tunnel: [_ _ _ _ _ _ _ _ _ _ _ _ _ _ _ _ _ _ _ _ _ _ _ _ _ _ _ _ _ _ _ w2121 _ _ _ _ _ _ _ _ _ _ _ _ _ _ _ _ _ _ _ _ _ _ _ _ _ _ _ _ _ _ _ _ _ _ _ _ _ _ _ _ _ _ _ _ _ _ _ _ _ _ _ _ _ _ _ _ _ _ _ _ _ _ _ _ _ _ _ _ _ _ _ _ _ _ _ _ _ _ _ _ _ _ _ _ _ _ _ _ _ _ _ _ _ _ _ _ _ _ _ _ _ _ _ _ _ _ _ _ _ _ _ _ _ _] -> w1864
            tunnel: [_ _ _ _ _ _ _ _ _ _ _ _ _ _ _ _ _ _ _ _ _ _ _ _ _ _ _ _ _ _ _ _ w2126 _ _ _ _ _ _ _ _ _ _ _ _ _ _ _ _ _ _ _ _ _ _ _ _ _ _ _ _ _ _ _ _ _ _ _ _ _ _ _ _ _ _ _ _ _ _ _ _ _ _ _ _ _ _ _ _ _ _ _ _ _ _ _ _ _ _ _ _ _ _ _ _ _ _ _ _ _ _ _ _ _ _ _ _ _ _ _ _ _ _ _ _ _ _ _ _ _ _ _ _ _ _ _ _ _ _ _ _ _ _ _ _ _] -> w1863
            tunnel: [_ _ _ _ _ _ _ _ _ _ _ _ _ _ _ _ _ _ _ _ _ _ _ _ _ _ _ _ _ _ _ _ _ w2132 _ _ _ _ _ _ _ _ _ _ _ _ _ _ _ _ _ _ _ _ _ _ _ _ _ _ _ _ _ _ _ _ _ _ _ _ _ _ _ _ _ _ _ _ _ _ _ _ _ _ _ _ _ _ _ _ _ _ _ _ _ _ _ _ _ _ _ _ _ _ _ _ _ _ _ _ _ _ _ _ _ _ _ _ _ _ _ _ _ _ _ _ _ _ _ _ _ _ _ _ _ _ _ _ _ _ _ _ _ _ _ _] -> w1862
            tunnel: [_ _ _ _ _ _ _ _ _ _ _ _ _ _ _ _ _ _ _ _ _ _ _ _ _ _ _ _ _ _ _ _ _ _ w2142 _ _ _ _ _ _ _ _ _ _ _ _ _ _ _ _ _ _ _ _ _ _ _ _ _ _ _ _ _ _ _ _ _ _ _ _ _ _ _ _ _ _ _ _ _ _ _ _ _ _ _ _ _ _ _ _ _ _ _ _ _ _ _ _ _ _ _ _ _ _ _ _ _ _ _ _ _ _ _ _ _ _ _ _ _ _ _ _ _ _ _ _ _ _ _ _ _ _ _ _ _ _ _ _ _ _ _ _ _ _ _] -> w1861
            tunnel: [_ _ _ _ _ _ _ _ _ _ _ _ _ _ _ _ _ _ _ _ _ _ _ _ _ _ _ _ _ _ _ _ _ _ _ w2147 _ _ _ _ _ _ _ _ _ _ _ _ _ _ _ _ _ _ _ _ _ _ _ _ _ _ _ _ _ _ _ _ _ _ _ _ _ _ _ _ _ _ _ _ _ _ _ _ _ _ _ _ _ _ _ _ _ _ _ _ _ _ _ _ _ _ _ _ _ _ _ _ _ _ _ _ _ _ _ _ _ _ _ _ _ _ _ _ _ _ _ _ _ _ _ _ _ _ _ _ _ _ _ _ _ _ _ _ _ _] -> w1860
            tunnel: [_ _ _ _ _ _ _ _ _ _ _ _ _ _ _ _ _ _ _ _ _ _ _ _ _ _ _ _ _ _ _ _ _ _ _ _ w2153 _ _ _ _ _ _ _ _ _ _ _ _ _ _ _ _ _ _ _ _ _ _ _ _ _ _ _ _ _ _ _ _ _ _ _ _ _ _ _ _ _ _ _ _ _ _ _ _ _ _ _ _ _ _ _ _ _ _ _ _ _ _ _ _ _ _ _ _ _ _ _ _ _ _ _ _ _ _ _ _ _ _ _ _ _ _ _ _ _ _ _ _ _ _ _ _ _ _ _ _ _ _ _ _ _ _ _ _ _] -> w1859
            tunnel: [_ _ _ _ _ _ _ _ _ _ _ _ _ _ _ _ _ _ _ _ _ _ _ _ _ _ _ _ _ _ _ _ _ _ _ _ _ w2163 _ _ _ _ _ _ _ _ _ _ _ _ _ _ _ _ _ _ _ _ _ _ _ _ _ _ _ _ _ _ _ _ _ _ _ _ _ _ _ _ _ _ _ _ _ _ _ _ _ _ _ _ _ _ _ _ _ _ _ _ _ _ _ _ _ _ _ _ _ _ _ _ _ _ _ _ _ _ _ _ _ _ _ _ _ _ _ _ _ _ _ _ _ _ _ _ _ _ _ _ _ _ _ _ _ _ _ _] -> w1858
            tunnel: [_ _ _ _ _ _ _ _ _ _ _ _ _ _ _ _ _ _ _ _ _ _ _ _ _ _ _ _ _ _ _ _ _ _ _ _ _ _ w2168 _ _ _ _ _ _ _ _ _ _ _ _ _ _ _ _ _ _ _ _ _ _ _ _ _ _ _ _ _ _ _ _ _ _ _ _ _ _ _ _ _ _ _ _ _ _ _ _ _ _ _ _ _ _ _ _ _ _ _ _ _ _ _ _ _ _ _ _ _ _ _ _ _ _ _ _ _ _ _ _ _ _ _ _ _ _ _ _ _ _ _ _ _ _ _ _ _ _ _ _ _ _ _ _ _ _ _] -> w1857
            tunnel: [_ _ _ _ _ _ _ _ _ _ _ _ _ _ _ _ _ _ _ _ _ _ _ _ _ _ _ _ _ _ _ _ _ _ _ _ _ _ _ w2174 _ _ _ _ _ _ _ _ _ _ _ _ _ _ _ _ _ _ _ _ _ _ _ _ _ _ _ _ _ _ _ _ _ _ _ _ _ _ _ _ _ _ _ _ _ _ _ _ _ _ _ _ _ _ _ _ _ _ _ _ _ _ _ _ _ _ _ _ _ _ _ _ _ _ _ _ _ _ _ _ _ _ _ _ _ _ _ _ _ _ _ _ _ _ _ _ _ _ _ _ _ _ _ _ _ _] -> w1856
            tunnel: [_ _ _ _ _ _ _ _ _ _ _ _ _ _ _ _ _ _ _ _ _ _ _ _ _ _ _ _ _ _ _ _ _ _ _ _ _ _ _ _ w2184 _ _ _ _ _ _ _ _ _ _ _ _ _ _ _ _ _ _ _ _ _ _ _ _ _ _ _ _ _ _ _ _ _ _ _ _ _ _ _ _ _ _ _ _ _ _ _ _ _ _ _ _ _ _ _ _ _ _ _ _ _ _ _ _ _ _ _ _ _ _ _ _ _ _ _ _ _ _ _ _ _ _ _ _ _ _ _ _ _ _ _ _ _ _ _ _ _ _ _ _ _ _ _ _ _] -> w1855
            tunnel: [_ _ _ _ _ _ _ _ _ _ _ _ _ _ _ _ _ _ _ _ _ _ _ _ _ _ _ _ _ _ _ _ _ _ _ _ _ _ _ _ _ w2189 _ _ _ _ _ _ _ _ _ _ _ _ _ _ _ _ _ _ _ _ _ _ _ _ _ _ _ _ _ _ _ _ _ _ _ _ _ _ _ _ _ _ _ _ _ _ _ _ _ _ _ _ _ _ _ _ _ _ _ _ _ _ _ _ _ _ _ _ _ _ _ _ _ _ _ _ _ _ _ _ _ _ _ _ _ _ _ _ _ _ _ _ _ _ _ _ _ _ _ _ _ _ _ _] -> w1854
            tunnel: [_ _ _ _ _ _ _ _ _ _ _ _ _ _ _ _ _ _ _ _ _ _ _ _ _ _ _ _ _ _ _ _ _ _ _ _ _ _ _ _ _ _ w2195 _ _ _ _ _ _ _ _ _ _ _ _ _ _ _ _ _ _ _ _ _ _ _ _ _ _ _ _ _ _ _ _ _ _ _ _ _ _ _ _ _ _ _ _ _ _ _ _ _ _ _ _ _ _ _ _ _ _ _ _ _ _ _ _ _ _ _ _ _ _ _ _ _ _ _ _ _ _ _ _ _ _ _ _ _ _ _ _ _ _ _ _ _ _ _ _ _ _ _ _ _ _ _] -> w1853
            tunnel: [_ _ _ _ _ _ _ _ _ _ _ _ _ _ _ _ _ _ _ _ _ _ _ _ _ _ _ _ _ _ _ _ _ _ _ _ _ _ _ _ _ _ _ w2205 _ _ _ _ _ _ _ _ _ _ _ _ _ _ _ _ _ _ _ _ _ _ _ _ _ _ _ _ _ _ _ _ _ _ _ _ _ _ _ _ _ _ _ _ _ _ _ _ _ _ _ _ _ _ _ _ _ _ _ _ _ _ _ _ _ _ _ _ _ _ _ _ _ _ _ _ _ _ _ _ _ _ _ _ _ _ _ _ _ _ _ _ _ _ _ _ _ _ _ _ _ _] -> w1852
            tunnel: [_ _ _ _ _ _ _ _ _ _ _ _ _ _ _ _ _ _ _ _ _ _ _ _ _ _ _ _ _ _ _ _ _ _ _ _ _ _ _ _ _ _ _ _ w2210 _ _ _ _ _ _ _ _ _ _ _ _ _ _ _ _ _ _ _ _ _ _ _ _ _ _ _ _ _ _ _ _ _ _ _ _ _ _ _ _ _ _ _ _ _ _ _ _ _ _ _ _ _ _ _ _ _ _ _ _ _ _ _ _ _ _ _ _ _ _ _ _ _ _ _ _ _ _ _ _ _ _ _ _ _ _ _ _ _ _ _ _ _ _ _ _ _ _ _ _ _] -> w1851
            tunnel: [_ _ _ _ _ _ _ _ _ _ _ _ _ _ _ _ _ _ _ _ _ _ _ _ _ _ _ _ _ _ _ _ _ _ _ _ _ _ _ _ _ _ _ _ _ w2216 _ _ _ _ _ _ _ _ _ _ _ _ _ _ _ _ _ _ _ _ _ _ _ _ _ _ _ _ _ _ _ _ _ _ _ _ _ _ _ _ _ _ _ _ _ _ _ _ _ _ _ _ _ _ _ _ _ _ _ _ _ _ _ _ _ _ _ _ _ _ _ _ _ _ _ _ _ _ _ _ _ _ _ _ _ _ _ _ _ _ _ _ _ _ _ _ _ _ _ _] -> w1850
            tunnel: [_ _ _ _ _ _ _ _ _ _ _ _ _ _ _ _ _ _ _ _ _ _ _ _ _ _ _ _ _ _ _ _ _ _ _ _ _ _ _ _ _ _ _ _ _ _ w2226 _ _ _ _ _ _ _ _ _ _ _ _ _ _ _ _ _ _ _ _ _ _ _ _ _ _ _ _ _ _ _ _ _ _ _ _ _ _ _ _ _ _ _ _ _ _ _ _ _ _ _ _ _ _ _ _ _ _ _ _ _ _ _ _ _ _ _ _ _ _ _ _ _ _ _ _ _ _ _ _ _ _ _ _ _ _ _ _ _ _ _ _ _ _ _ _ _ _ _] -> w1849
            tunnel: [_ _ _ _ _ _ _ _ _ _ _ _ _ _ _ _ _ _ _ _ _ _ _ _ _ _ _ _ _ _ _ _ _ _ _ _ _ _ _ _ _ _ _ _ _ _ _ w2231 _ _ _ _ _ _ _ _ _ _ _ _ _ _ _ _ _ _ _ _ _ _ _ _ _ _ _ _ _ _ _ _ _ _ _ _ _ _ _ _ _ _ _ _ _ _ _ _ _ _ _ _ _ _ _ _ _ _ _ _ _ _ _ _ _ _ _ _ _ _ _ _ _ _ _ _ _ _ _ _ _ _ _ _ _ _ _ _ _ _ _ _ _ _ _ _ _ _] -> w1848
            tunnel: [_ _ _ _ _ _ _ _ _ _ _ _ _ _ _ _ _ _ _ _ _ _ _ _ _ _ _ _ _ _ _ _ _ _ _ _ _ _ _ _ _ _ _ _ _ _ _ _ w2237 _ _ _ _ _ _ _ _ _ _ _ _ _ _ _ _ _ _ _ _ _ _ _ _ _ _ _ _ _ _ _ _ _ _ _ _ _ _ _ _ _ _ _ _ _ _ _ _ _ _ _ _ _ _ _ _ _ _ _ _ _ _ _ _ _ _ _ _ _ _ _ _ _ _ _ _ _ _ _ _ _ _ _ _ _ _ _ _ _ _ _ _ _ _ _ _ _] -> w1847
            tunnel: [_ _ _ _ _ _ _ _ _ _ _ _ _ _ _ _ _ _ _ _ _ _ _ _ _ _ _ _ _ _ _ _ _ _ _ _ _ _ _ _ _ _ _ _ _ _ _ _ _ w2246 _ _ _ _ _ _ _ _ _ _ _ _ _ _ _ _ _ _ _ _ _ _ _ _ _ _ _ _ _ _ _ _ _ _ _ _ _ _ _ _ _ _ _ _ _ _ _ _ _ _ _ _ _ _ _ _ _ _ _ _ _ _ _ _ _ _ _ _ _ _ _ _ _ _ _ _ _ _ _ _ _ _ _ _ _ _ _ _ _ _ _ _ _ _ _ _] -> w1846
            tunnel: [_ _ _ _ _ _ _ _ _ _ _ _ _ _ _ _ _ _ _ _ _ _ _ _ _ _ _ _ _ _ _ _ _ _ _ _ _ _ _ _ _ _ _ _ _ _ _ _ _ _ w2252 _ _ _ _ _ _ _ _ _ _ _ _ _ _ _ _ _ _ _ _ _ _ _ _ _ _ _ _ _ _ _ _ _ _ _ _ _ _ _ _ _ _ _ _ _ _ _ _ _ _ _ _ _ _ _ _ _ _ _ _ _ _ _ _ _ _ _ _ _ _ _ _ _ _ _ _ _ _ _ _ _ _ _ _ _ _ _ _ _ _ _ _ _ _ _] -> w1845
            tunnel: [_ _ _ _ _ _ _ _ _ _ _ _ _ _ _ _ _ _ _ _ _ _ _ _ _ _ _ _ _ _ _ _ _ _ _ _ _ _ _ _ _ _ _ _ _ _ _ _ _ _ _ w2258 _ _ _ _ _ _ _ _ _ _ _ _ _ _ _ _ _ _ _ _ _ _ _ _ _ _ _ _ _ _ _ _ _ _ _ _ _ _ _ _ _ _ _ _ _ _ _ _ _ _ _ _ _ _ _ _ _ _ _ _ _ _ _ _ _ _ _ _ _ _ _ _ _ _ _ _ _ _ _ _ _ _ _ _ _ _ _ _ _ _ _ _ _ _] -> w1844
            tunnel: [_ _ _ _ _ _ _ _ _ _ _ _ _ _ _ _ _ _ _ _ _ _ _ _ _ _ _ _ _ _ _ _ _ _ _ _ _ _ _ _ _ _ _ _ _ _ _ _ _ _ _ _ w2268 _ _ _ _ _ _ _ _ _ _ _ _ _ _ _ _ _ _ _ _ _ _ _ _ _ _ _ _ _ _ _ _ _ _ _ _ _ _ _ _ _ _ _ _ _ _ _ _ _ _ _ _ _ _ _ _ _ _ _ _ _ _ _ _ _ _ _ _ _ _ _ _ _ _ _ _ _ _ _ _ _ _ _ _ _ _ _ _ _ _ _ _ _] -> w1843
            tunnel: [_ _ _ _ _ _ _ _ _ _ _ _ _ _ _ _ _ _ _ _ _ _ _ _ _ _ _ _ _ _ _ _ _ _ _ _ _ _ _ _ _ _ _ _ _ _ _ _ _ _ _ _ _ w2273 _ _ _ _ _ _ _ _ _ _ _ _ _ _ _ _ _ _ _ _ _ _ _ _ _ _ _ _ _ _ _ _ _ _ _ _ _ _ _ _ _ _ _ _ _ _ _ _ _ _ _ _ _ _ _ _ _ _ _ _ _ _ _ _ _ _ _ _ _ _ _ _ _ _ _ _ _ _ _ _ _ _ _ _ _ _ _ _ _ _ _ _] -> w1842
            tunnel: [_ _ _ _ _ _ _ _ _ _ _ _ _ _ _ _ _ _ _ _ _ _ _ _ _ _ _ _ _ _ _ _ _ _ _ _ _ _ _ _ _ _ _ _ _ _ _ _ _ _ _ _ _ _ w2280 _ _ _ _ _ _ _ _ _ _ _ _ _ _ _ _ _ _ _ _ _ _ _ _ _ _ _ _ _ _ _ _ _ _ _ _ _ _ _ _ _ _ _ _ _ _ _ _ _ _ _ _ _ _ _ _ _ _ _ _ _ _ _ _ _ _ _ _ _ _ _ _ _ _ _ _ _ _ _ _ _ _ _ _ _ _ _ _ _ _ _] -> w1841
            tunnel: [_ _ _ _ _ _ _ _ _ _ _ _ _ _ _ _ _ _ _ _ _ _ _ _ _ _ _ _ _ _ _ _ _ _ _ _ _ _ _ _ _ _ _ _ _ _ _ _ _ _ _ _ _ _ _ w2284 _ _ _ _ _ _ _ _ _ _ _ _ _ _ _ _ _ _ _ _ _ _ _ _ _ _ _ _ _ _ _ _ _ _ _ _ _ _ _ _ _ _ _ _ _ _ _ _ _ _ _ _ _ _ _ _ _ _ _ _ _ _ _ _ _ _ _ _ _ _ _ _ _ _ _ _ _ _ _ _ _ _ _ _ _ _ _ _ _ _] -> w1840
            tunnel: [_ _ _ _ _ _ _ _ _ _ _ _ _ _ _ _ _ _ _ _ _ _ _ _ _ _ _ _ _ _ _ _ _ _ _ _ _ _ _ _ _ _ _ _ _ _ _ _ _ _ _ _ _ _ _ _ w2290 _ _ _ _ _ _ _ _ _ _ _ _ _ _ _ _ _ _ _ _ _ _ _ _ _ _ _ _ _ _ _ _ _ _ _ _ _ _ _ _ _ _ _ _ _ _ _ _ _ _ _ _ _ _ _ _ _ _ _ _ _ _ _ _ _ _ _ _ _ _ _ _ _ _ _ _ _ _ _ _ _ _ _ _ _ _ _ _ _] -> w1839
            tunnel: [_ _ _ _ _ _ _ _ _ _ _ _ _ _ _ _ _ _ _ _ _ _ _ _ _ _ _ _ _ _ _ _ _ _ _ _ _ _ _ _ _ _ _ _ _ _ _ _ _ _ _ _ _ _ _ _ _ w2299 _ _ _ _ _ _ _ _ _ _ _ _ _ _ _ _ _ _ _ _ _ _ _ _ _ _ _ _ _ _ _ _ _ _ _ _ _ _ _ _ _ _ _ _ _ _ _ _ _ _ _ _ _ _ _ _ _ _ _ _ _ _ _ _ _ _ _ _ _ _ _ _ _ _ _ _ _ _ _ _ _ _ _ _ _ _ _ _] -> w1838
            tunnel: [_ _ _ _ _ _ _ _ _ _ _ _ _ _ _ _ _ _ _ _ _ _ _ _ _ _ _ _ _ _ _ _ _ _ _ _ _ _ _ _ _ _ _ _ _ _ _ _ _ _ _ _ _ _ _ _ _ _ w2305 _ _ _ _ _ _ _ _ _ _ _ _ _ _ _ _ _ _ _ _ _ _ _ _ _ _ _ _ _ _ _ _ _ _ _ _ _ _ _ _ _ _ _ _ _ _ _ _ _ _ _ _ _ _ _ _ _ _ _ _ _ _ _ _ _ _ _ _ _ _ _ _ _ _ _ _ _ _ _ _ _ _ _ _ _ _ _] -> w1837
            tunnel: [_ _ _ _ _ _ _ _ _ _ _ _ _ _ _ _ _ _ _ _ _ _ _ _ _ _ _ _ _ _ _ _ _ _ _ _ _ _ _ _ _ _ _ _ _ _ _ _ _ _ _ _ _ _ _ _ _ _ _ w2314 _ _ _ _ _ _ _ _ _ _ _ _ _ _ _ _ _ _ _ _ _ _ _ _ _ _ _ _ _ _ _ _ _ _ _ _ _ _ _ _ _ _ _ _ _ _ _ _ _ _ _ _ _ _ _ _ _ _ _ _ _ _ _ _ _ _ _ _ _ _ _ _ _ _ _ _ _ _ _ _ _ _ _ _ _ _] -> w1836
            tunnel: [_ _ _ _ _ _ _ _ _ _ _ _ _ _ _ _ _ _ _ _ _ _ _ _ _ _ _ _ _ _ _ _ _ _ _ _ _ _ _ _ _ _ _ _ _ _ _ _ _ _ _ _ _ _ _ _ _ _ _ _ w2320 _ _ _ _ _ _ _ _ _ _ _ _ _ _ _ _ _ _ _ _ _ _ _ _ _ _ _ _ _ _ _ _ _ _ _ _ _ _ _ _ _ _ _ _ _ _ _ _ _ _ _ _ _ _ _ _ _ _ _ _ _ _ _ _ _ _ _ _ _ _ _ _ _ _ _ _ _ _ _ _ _ _ _ _ _] -> w1835
            tunnel: [_ _ _ _ _ _ _ _ _ _ _ _ _ _ _ _ _ _ _ _ _ _ _ _ _ _ _ _ _ _ _ _ _ _ _ _ _ _ _ _ _ _ _ _ _ _ _ _ _ _ _ _ _ _ _ _ _ _ _ _ _ w2326 _ _ _ _ _ _ _ _ _ _ _ _ _ _ _ _ _ _ _ _ _ _ _ _ _ _ _ _ _ _ _ _ _ _ _ _ _ _ _ _ _ _ _ _ _ _ _ _ _ _ _ _ _ _ _ _ _ _ _ _ _ _ _ _ _ _ _ _ _ _ _ _ _ _ _ _ _ _ _ _ _ _ _ _] -> w1834
            tunnel: [_ _ _ _ _ _ _ _ _ _ _ _ _ _ _ _ _ _ _ _ _ _ _ _ _ _ _ _ _ _ _ _ _ _ _ _ _ _ _ _ _ _ _ _ _ _ _ _ _ _ _ _ _ _ _ _ _ _ _ _ _ _ w2336 _ _ _ _ _ _ _ _ _ _ _ _ _ _ _ _ _ _ _ _ _ _ _ _ _ _ _ _ _ _ _ _ _ _ _ _ _ _ _ _ _ _ _ _ _ _ _ _ _ _ _ _ _ _ _ _ _ _ _ _ _ _ _ _ _ _ _ _ _ _ _ _ _ _ _ _ _ _ _ _ _ _ _] -> w1833
            tunnel: [_ _ _ _ _ _ _ _ _ _ _ _ _ _ _ _ _ _ _ _ _ _ _ _ _ _ _ _ _ _ _ _ _ _ _ _ _ _ _ _ _ _ _ _ _ _ _ _ _ _ _ _ _ _ _ _ _ _ _ _ _ _ _ w2341 _ _ _ _ _ _ _ _ _ _ _ _ _ _ _ _ _ _ _ _ _ _ _ _ _ _ _ _ _ _ _ _ _ _ _ _ _ _ _ _ _ _ _ _ _ _ _ _ _ _ _ _ _ _ _ _ _ _ _ _ _ _ _ _ _ _ _ _ _ _ _ _ _ _ _ _ _ _ _ _ _ _] -> w1832
            tunnel: [_ _ _ _ _ _ _ _ _ _ _ _ _ _ _ _ _ _ _ _ _ _ _ _ _ _ _ _ _ _ _ _ _ _ _ _ _ _ _ _ _ _ _ _ _ _ _ _ _ _ _ _ _ _ _ _ _ _ _ _ _ _ _ _ w2347 _ _ _ _ _ _ _ _ _ _ _ _ _ _ _ _ _ _ _ _ _ _ _ _ _ _ _ _ _ _ _ _ _ _ _ _ _ _ _ _ _ _ _ _ _ _ _ _ _ _ _ _ _ _ _ _ _ _ _ _ _ _ _ _ _ _ _ _ _ _ _ _ _ _ _ _ _ _ _ _ _] -> w1831
            tunnel: [_ _ _ _ _ _ _ _ _ _ _ _ _ _ _ _ _ _ _ _ _ _ _ _ _ _ _ _ _ _ _ _ _ _ _ _ _ _ _ _ _ _ _ _ _ _ _ _ _ _ _ _ _ _ _ _ _ _ _ _ _ _ _ _ _ w2357 _ _ _ _ _ _ _ _ _ _ _ _ _ _ _ _ _ _ _ _ _ _ _ _ _ _ _ _ _ _ _ _ _ _ _ _ _ _ _ _ _ _ _ _ _ _ _ _ _ _ _ _ _ _ _ _ _ _ _ _ _ _ _ _ _ _ _ _ _ _ _ _ _ _ _ _ _ _ _ _] -> w1830
            tunnel: [_ _ _ _ _ _ _ _ _ _ _ _ _ _ _ _ _ _ _ _ _ _ _ _ _ _ _ _ _ _ _ _ _ _ _ _ _ _ _ _ _ _ _ _ _ _ _ _ _ _ _ _ _ _ _ _ _ _ _ _ _ _ _ _ _ _ w2362 _ _ _ _ _ _ _ _ _ _ _ _ _ _ _ _ _ _ _ _ _ _ _ _ _ _ _ _ _ _ _ _ _ _ _ _ _ _ _ _ _ _ _ _ _ _ _ _ _ _ _ _ _ _ _ _ _ _ _ _ _ _ _ _ _ _ _ _ _ _ _ _ _ _ _ _ _ _ _] -> w1829
            tunnel: [_ _ _ _ _ _ _ _ _ _ _ _ _ _ _ _ _ _ _ _ _ _ _ _ _ _ _ _ _ _ _ _ _ _ _ _ _ _ _ _ _ _ _ _ _ _ _ _ _ _ _ _ _ _ _ _ _ _ _ _ _ _ _ _ _ _ _ w2368 _ _ _ _ _ _ _ _ _ _ _ _ _ _ _ _ _ _ _ _ _ _ _ _ _ _ _ _ _ _ _ _ _ _ _ _ _ _ _ _ _ _ _ _ _ _ _ _ _ _ _ _ _ _ _ _ _ _ _ _ _ _ _ _ _ _ _ _ _ _ _ _ _ _ _ _ _ _] -> w1828
            tunnel: [_ _ _ _ _ _ _ _ _ _ _ _ _ _ _ _ _ _ _ _ _ _ _ _ _ _ _ _ _ _ _ _ _ _ _ _ _ _ _ _ _ _ _ _ _ _ _ _ _ _ _ _ _ _ _ _ _ _ _ _ _ _ _ _ _ _ _ _ w2378 _ _ _ _ _ _ _ _ _ _ _ _ _ _ _ _ _ _ _ _ _ _ _ _ _ _ _ _ _ _ _ _ _ _ _ _ _ _ _ _ _ _ _ _ _ _ _ _ _ _ _ _ _ _ _ _ _ _ _ _ _ _ _ _ _ _ _ _ _ _ _ _ _ _ _ _ _] -> w1827
            tunnel: [_ _ _ _ _ _ _ _ _ _ _ _ _ _ _ _ _ _ _ _ _ _ _ _ _ _ _ _ _ _ _ _ _ _ _ _ _ _ _ _ _ _ _ _ _ _ _ _ _ _ _ _ _ _ _ _ _ _ _ _ _ _ _ _ _ _ _ _ _ w2383 _ _ _ _ _ _ _ _ _ _ _ _ _ _ _ _ _ _ _ _ _ _ _ _ _ _ _ _ _ _ _ _ _ _ _ _ _ _ _ _ _ _ _ _ _ _ _ _ _ _ _ _ _ _ _ _ _ _ _ _ _ _ _ _ _ _ _ _ _ _ _ _ _ _ _ _] -> w1826
            tunnel: [_ _ _ _ _ _ _ _ _ _ _ _ _ _ _ _ _ _ _ _ _ _ _ _ _ _ _ _ _ _ _ _ _ _ _ _ _ _ _ _ _ _ _ _ _ _ _ _ _ _ _ _ _ _ _ _ _ _ _ _ _ _ _ _ _ _ _ _ _ _ w2389 _ _ _ _ _ _ _ _ _ _ _ _ _ _ _ _ _ _ _ _ _ _ _ _ _ _ _ _ _ _ _ _ _ _ _ _ _ _ _ _ _ _ _ _ _ _ _ _ _ _ _ _ _ _ _ _ _ _ _ _ _ _ _ _ _ _ _ _ _ _ _ _ _ _ _] -> w1825
            tunnel: [_ _ _ _ _ _ _ _ _ _ _ _ _ _ _ _ _ _ _ _ _ _ _ _ _ _ _ _ _ _ _ _ _ _ _ _ _ _ _ _ _ _ _ _ _ _ _ _ _ _ _ _ _ _ _ _ _ _ _ _ _ _ _ _ _ _ _ _ _ _ _ w2399 _ _ _ _ _ _ _ _ _ _ _ _ _ _ _ _ _ _ _ _ _ _ _ _ _ _ _ _ _ _ _ _ _ _ _ _ _ _ _ _ _ _ _ _ _ _ _ _ _ _ _ _ _ _ _ _ _ _ _ _ _ _ _ _ _ _ _ _ _ _ _ _ _ _] -> w1824
            tunnel: [_ _ _ _ _ _ _ _ _ _ _ _ _ _ _ _ _ _ _ _ _ _ _ _ _ _ _ _ _ _ _ _ _ _ _ _ _ _ _ _ _ _ _ _ _ _ _ _ _ _ _ _ _ _ _ _ _ _ _ _ _ _ _ _ _ _ _ _ _ _ _ _ w2404 _ _ _ _ _ _ _ _ _ _ _ _ _ _ _ _ _ _ _ _ _ _ _ _ _ _ _ _ _ _ _ _ _ _ _ _ _ _ _ _ _ _ _ _ _ _ _ _ _ _ _ _ _ _ _ _ _ _ _ _ _ _ _ _ _ _ _ _ _ _ _ _ _] -> w1823
            tunnel: [_ _ _ _ _ _ _ _ _ _ _ _ _ _ _ _ _ _ _ _ _ _ _ _ _ _ _ _ _ _ _ _ _ _ _ _ _ _ _ _ _ _ _ _ _ _ _ _ _ _ _ _ _ _ _ _ _ _ _ _ _ _ _ _ _ _ _ _ _ _ _ _ _ w2410 _ _ _ _ _ _ _ _ _ _ _ _ _ _ _ _ _ _ _ _ _ _ _ _ _ _ _ _ _ _ _ _ _ _ _ _ _ _ _ _ _ _ _ _ _ _ _ _ _ _ _ _ _ _ _ _ _ _ _ _ _ _ _ _ _ _ _ _ _ _ _ _] -> w1822
            tunnel: [_ _ _ _ _ _ _ _ _ _ _ _ _ _ _ _ _ _ _ _ _ _ _ _ _ _ _ _ _ _ _ _ _ _ _ _ _ _ _ _ _ _ _ _ _ _ _ _ _ _ _ _ _ _ _ _ _ _ _ _ _ _ _ _ _ _ _ _ _ _ _ _ _ _ w2420 _ _ _ _ _ _ _ _ _ _ _ _ _ _ _ _ _ _ _ _ _ _ _ _ _ _ _ _ _ _ _ _ _ _ _ _ _ _ _ _ _ _ _ _ _ _ _ _ _ _ _ _ _ _ _ _ _ _ _ _ _ _ _ _ _ _ _ _ _ _ _] -> w1821
            tunnel: [_ _ _ _ _ _ _ _ _ _ _ _ _ _ _ _ _ _ _ _ _ _ _ _ _ _ _ _ _ _ _ _ _ _ _ _ _ _ _ _ _ _ _ _ _ _ _ _ _ _ _ _ _ _ _ _ _ _ _ _ _ _ _ _ _ _ _ _ _ _ _ _ _ _ _ w2425 _ _ _ _ _ _ _ _ _ _ _ _ _ _ _ _ _ _ _ _ _ _ _ _ _ _ _ _ _ _ _ _ _ _ _ _ _ _ _ _ _ _ _ _ _ _ _ _ _ _ _ _ _ _ _ _ _ _ _ _ _ _ _ _ _ _ _ _ _ _] -> w1820
            tunnel: [_ _ _ _ _ _ _ _ _ _ _ _ _ _ _ _ _ _ _ _ _ _ _ _ _ _ _ _ _ _ _ _ _ _ _ _ _ _ _ _ _ _ _ _ _ _ _ _ _ _ _ _ _ _ _ _ _ _ _ _ _ _ _ _ _ _ _ _ _ _ _ _ _ _ _ _ w2431 _ _ _ _ _ _ _ _ _ _ _ _ _ _ _ _ _ _ _ _ _ _ _ _ _ _ _ _ _ _ _ _ _ _ _ _ _ _ _ _ _ _ _ _ _ _ _ _ _ _ _ _ _ _ _ _ _ _ _ _ _ _ _ _ _ _ _ _ _] -> w1819
            tunnel: [_ _ _ _ _ _ _ _ _ _ _ _ _ _ _ _ _ _ _ _ _ _ _ _ _ _ _ _ _ _ _ _ _ _ _ _ _ _ _ _ _ _ _ _ _ _ _ _ _ _ _ _ _ _ _ _ _ _ _ _ _ _ _ _ _ _ _ _ _ _ _ _ _ _ _ _ _ w2441 _ _ _ _ _ _ _ _ _ _ _ _ _ _ _ _ _ _ _ _ _ _ _ _ _ _ _ _ _ _ _ _ _ _ _ _ _ _ _ _ _ _ _ _ _ _ _ _ _ _ _ _ _ _ _ _ _ _ _ _ _ _ _ _ _ _ _ _] -> w1818
            tunnel: [_ _ _ _ _ _ _ _ _ _ _ _ _ _ _ _ _ _ _ _ _ _ _ _ _ _ _ _ _ _ _ _ _ _ _ _ _ _ _ _ _ _ _ _ _ _ _ _ _ _ _ _ _ _ _ _ _ _ _ _ _ _ _ _ _ _ _ _ _ _ _ _ _ _ _ _ _ _ w2446 _ _ _ _ _ _ _ _ _ _ _ _ _ _ _ _ _ _ _ _ _ _ _ _ _ _ _ _ _ _ _ _ _ _ _ _ _ _ _ _ _ _ _ _ _ _ _ _ _ _ _ _ _ _ _ _ _ _ _ _ _ _ _ _ _ _ _] -> w1817
            tunnel: [_ _ _ _ _ _ _ _ _ _ _ _ _ _ _ _ _ _ _ _ _ _ _ _ _ _ _ _ _ _ _ _ _ _ _ _ _ _ _ _ _ _ _ _ _ _ _ _ _ _ _ _ _ _ _ _ _ _ _ _ _ _ _ _ _ _ _ _ _ _ _ _ _ _ _ _ _ _ _ w2452 _ _ _ _ _ _ _ _ _ _ _ _ _ _ _ _ _ _ _ _ _ _ _ _ _ _ _ _ _ _ _ _ _ _ _ _ _ _ _ _ _ _ _ _ _ _ _ _ _ _ _ _ _ _ _ _ _ _ _ _ _ _ _ _ _ _] -> w1816
            tunnel: [_ _ _ _ _ _ _ _ _ _ _ _ _ _ _ _ _ _ _ _ _ _ _ _ _ _ _ _ _ _ _ _ _ _ _ _ _ _ _ _ _ _ _ _ _ _ _ _ _ _ _ _ _ _ _ _ _ _ _ _ _ _ _ _ _ _ _ _ _ _ _ _ _ _ _ _ _ _ _ _ w2462 _ _ _ _ _ _ _ _ _ _ _ _ _ _ _ _ _ _ _ _ _ _ _ _ _ _ _ _ _ _ _ _ _ _ _ _ _ _ _ _ _ _ _ _ _ _ _ _ _ _ _ _ _ _ _ _ _ _ _ _ _ _ _ _ _] -> w1815
            tunnel: [_ _ _ _ _ _ _ _ _ _ _ _ _ _ _ _ _ _ _ _ _ _ _ _ _ _ _ _ _ _ _ _ _ _ _ _ _ _ _ _ _ _ _ _ _ _ _ _ _ _ _ _ _ _ _ _ _ _ _ _ _ _ _ _ _ _ _ _ _ _ _ _ _ _ _ _ _ _ _ _ _ w2467 _ _ _ _ _ _ _ _ _ _ _ _ _ _ _ _ _ _ _ _ _ _ _ _ _ _ _ _ _ _ _ _ _ _ _ _ _ _ _ _ _ _ _ _ _ _ _ _ _ _ _ _ _ _ _ _ _ _ _ _ _ _ _ _] -> w1814
            tunnel: [_ _ _ _ _ _ _ _ _ _ _ _ _ _ _ _ _ _ _ _ _ _ _ _ _ _ _ _ _ _ _ _ _ _ _ _ _ _ _ _ _ _ _ _ _ _ _ _ _ _ _ _ _ _ _ _ _ _ _ _ _ _ _ _ _ _ _ _ _ _ _ _ _ _ _ _ _ _ _ _ _ _ w2473 _ _ _ _ _ _ _ _ _ _ _ _ _ _ _ _ _ _ _ _ _ _ _ _ _ _ _ _ _ _ _ _ _ _ _ _ _ _ _ _ _ _ _ _ _ _ _ _ _ _ _ _ _ _ _ _ _ _ _ _ _ _ _] -> w1813
            tunnel: [_ _ _ _ _ _ _ _ _ _ _ _ _ _ _ _ _ _ _ _ _ _ _ _ _ _ _ _ _ _ _ _ _ _ _ _ _ _ _ _ _ _ _ _ _ _ _ _ _ _ _ _ _ _ _ _ _ _ _ _ _ _ _ _ _ _ _ _ _ _ _ _ _ _ _ _ _ _ _ _ _ _ _ w2483 _ _ _ _ _ _ _ _ _ _ _ _ _ _ _ _ _ _ _ _ _ _ _ _ _ _ _ _ _ _ _ _ _ _ _ _ _ _ _ _ _ _ _ _ _ _ _ _ _ _ _ _ _ _ _ _ _ _ _ _ _ _] -> w1812
            tunnel: [_ _ _ _ _ _ _ _ _ _ _ _ _ _ _ _ _ _ _ _ _ _ _ _ _ _ _ _ _ _ _ _ _ _ _ _ _ _ _ _ _ _ _ _ _ _ _ _ _ _ _ _ _ _ _ _ _ _ _ _ _ _ _ _ _ _ _ _ _ _ _ _ _ _ _ _ _ _ _ _ _ _ _ _ w2488 _ _ _ _ _ _ _ _ _ _ _ _ _ _ _ _ _ _ _ _ _ _ _ _ _ _ _ _ _ _ _ _ _ _ _ _ _ _ _ _ _ _ _ _ _ _ _ _ _ _ _ _ _ _ _ _ _ _ _ _ _] -> w1811
            tunnel: [_ _ _ _ _ _ _ _ _ _ _ _ _ _ _ _ _ _ _ _ _ _ _ _ _ _ _ _ _ _ _ _ _ _ _ _ _ _ _ _ _ _ _ _ _ _ _ _ _ _ _ _ _ _ _ _ _ _ _ _ _ _ _ _ _ _ _ _ _ _ _ _ _ _ _ _ _ _ _ _ _ _ _ _ _ w2494 _ _ _ _ _ _ _ _ _ _ _ _ _ _ _ _ _ _ _ _ _ _ _ _ _ _ _ _ _ _ _ _ _ _ _ _ _ _ _ _ _ _ _ _ _ _ _ _ _ _ _ _ _ _ _ _ _ _ _ _] -> w1810
            tunnel: [_ _ _ _ _ _ _ _ _ _ _ _ _ _ _ _ _ _ _ _ _ _ _ _ _ _ _ _ _ _ _ _ _ _ _ _ _ _ _ _ _ _ _ _ _ _ _ _ _ _ _ _ _ _ _ _ _ _ _ _ _ _ _ _ _ _ _ _ _ _ _ _ _ _ _ _ _ _ _ _ _ _ _ _ _ _ w2504 _ _ _ _ _ _ _ _ _ _ _ _ _ _ _ _ _ _ _ _ _ _ _ _ _ _ _ _ _ _ _ _ _ _ _ _ _ _ _ _ _ _ _ _ _ _ _ _ _ _ _ _ _ _ _ _ _ _ _] -> w1809
            tunnel: [_ _ _ _ _ _ _ _ _ _ _ _ _ _ _ _ _ _ _ _ _ _ _ _ _ _ _ _ _ _ _ _ _ _ _ _ _ _ _ _ _ _ _ _ _ _ _ _ _ _ _ _ _ _ _ _ _ _ _ _ _ _ _ _ _ _ _ _ _ _ _ _ _ _ _ _ _ _ _ _ _ _ _ _ _ _ _ w2509 _ _ _ _ _ _ _ _ _ _ _ _ _ _ _ _ _ _ _ _ _ _ _ _ _ _ _ _ _ _ _ _ _ _ _ _ _ _ _ _ _ _ _ _ _ _ _ _ _ _ _ _ _ _ _ _ _ _] -> w1808
            tunnel: [_ _ _ _ _ _ _ _ _ _ _ _ _ _ _ _ _ _ _ _ _ _ _ _ _ _ _ _ _ _ _ _ _ _ _ _ _ _ _ _ _ _ _ _ _ _ _ _ _ _ _ _ _ _ _ _ _ _ _ _ _ _ _ _ _ _ _ _ _ _ _ _ _ _ _ _ _ _ _ _ _ _ _ _ _ _ _ _ w2515 _ _ _ _ _ _ _ _ _ _ _ _ _ _ _ _ _ _ _ _ _ _ _ _ _ _ _ _ _ _ _ _ _ _ _ _ _ _ _ _ _ _ _ _ _ _ _ _ _ _ _ _ _ _ _ _ _] -> w1807
            tunnel: [_ _ _ _ _ _ _ _ _ _ _ _ _ _ _ _ _ _ _ _ _ _ _ _ _ _ _ _ _ _ _ _ _ _ _ _ _ _ _ _ _ _ _ _ _ _ _ _ _ _ _ _ _ _ _ _ _ _ _ _ _ _ _ _ _ _ _ _ _ _ _ _ _ _ _ _ _ _ _ _ _ _ _ _ _ _ _ _ _ w2524 _ _ _ _ _ _ _ _ _ _ _ _ _ _ _ _ _ _ _ _ _ _ _ _ _ _ _ _ _ _ _ _ _ _ _ _ _ _ _ _ _ _ _ _ _ _ _ _ _ _ _ _ _ _ _ _] -> w1806
            tunnel: [_ _ _ _ _ _ _ _ _ _ _ _ _ _ _ _ _ _ _ _ _ _ _ _ _ _ _ _ _ _ _ _ _ _ _ _ _ _ _ _ _ _ _ _ _ _ _ _ _ _ _ _ _ _ _ _ _ _ _ _ _ _ _ _ _ _ _ _ _ _ _ _ _ _ _ _ _ _ _ _ _ _ _ _ _ _ _ _ _ _ w2531 _ _ _ _ _ _ _ _ _ _ _ _ _ _ _ _ _ _ _ _ _ _ _ _ _ _ _ _ _ _ _ _ _ _ _ _ _ _ _ _ _ _ _ _ _ _ _ _ _ _ _ _ _ _ _] -> w1805
            tunnel: [_ _ _ _ _ _ _ _ _ _ _ _ _ _ _ _ _ _ _ _ _ _ _ _ _ _ _ _ _ _ _ _ _ _ _ _ _ _ _ _ _ _ _ _ _ _ _ _ _ _ _ _ _ _ _ _ _ _ _ _ _ _ _ _ _ _ _ _ _ _ _ _ _ _ _ _ _ _ _ _ _ _ _ _ _ _ _ _ _ _ _ w2535 _ _ _ _ _ _ _ _ _ _ _ _ _ _ _ _ _ _ _ _ _ _ _ _ _ _ _ _ _ _ _ _ _ _ _ _ _ _ _ _ _ _ _ _ _ _ _ _ _ _ _ _ _ _] -> w1804
            tunnel: [_ _ _ _ _ _ _ _ _ _ _ _ _ _ _ _ _ _ _ _ _ _ _ _ _ _ _ _ _ _ _ _ _ _ _ _ _ _ _ _ _ _ _ _ _ _ _ _ _ _ _ _ _ _ _ _ _ _ _ _ _ _ _ _ _ _ _ _ _ _ _ _ _ _ _ _ _ _ _ _ _ _ _ _ _ _ _ _ _ _ _ _ w2539 _ _ _ _ _ _ _ _ _ _ _ _ _ _ _ _ _ _ _ _ _ _ _ _ _ _ _ _ _ _ _ _ _ _ _ _ _ _ _ _ _ _ _ _ _ _ _ _ _ _ _ _ _] -> w1803
            tunnel: [_ _ _ _ _ _ _ _ _ _ _ _ _ _ _ _ _ _ _ _ _ _ _ _ _ _ _ _ _ _ _ _ _ _ _ _ _ _ _ _ _ _ _ _ _ _ _ _ _ _ _ _ _ _ _ _ _ _ _ _ _ _ _ _ _ _ _ _ _ _ _ _ _ _ _ _ _ _ _ _ _ _ _ _ _ _ _ _ _ _ _ _ _ w2545 _ _ _ _ _ _ _ _ _ _ _ _ _ _ _ _ _ _ _ _ _ _ _ _ _ _ _ _ _ _ _ _ _ _ _ _ _ _ _ _ _ _ _ _ _ _ _ _ _ _ _ _] -> w1802
            tunnel: [_ _ _ _ _ _ _ _ _ _ _ _ _ _ _ _ _ _ _ _ _ _ _ _ _ _ _ _ _ _ _ _ _ _ _ _ _ _ _ _ _ _ _ _ _ _ _ _ _ _ _ _ _ _ _ _ _ _ _ _ _ _ _ _ _ _ _ _ _ _ _ _ _ _ _ _ _ _ _ _ _ _ _ _ _ _ _ _ _ _ _ _ _ _ w2551 _ _ _ _ _ _ _ _ _ _ _ _ _ _ _ _ _ _ _ _ _ _ _ _ _ _ _ _ _ _ _ _ _ _ _ _ _ _ _ _ _ _ _ _ _ _ _ _ _ _ _] -> w1801
            tunnel: [_ _ _ _ _ _ _ _ _ _ _ _ _ _ _ _ _ _ _ _ _ _ _ _ _ _ _ _ _ _ _ _ _ _ _ _ _ _ _ _ _ _ _ _ _ _ _ _ _ _ _ _ _ _ _ _ _ _ _ _ _ _ _ _ _ _ _ _ _ _ _ _ _ _ _ _ _ _ _ _ _ _ _ _ _ _ _ _ _ _ _ _ _ _ _ w2557 _ _ _ _ _ _ _ _ _ _ _ _ _ _ _ _ _ _ _ _ _ _ _ _ _ _ _ _ _ _ _ _ _ _ _ _ _ _ _ _ _ _ _ _ _ _ _ _ _ _] -> w1800
            tunnel: [_ _ _ _ _ _ _ _ _ _ _ _ _ _ _ _ _ _ _ _ _ _ _ _ _ _ _ _ _ _ _ _ _ _ _ _ _ _ _ _ _ _ _ _ _ _ _ _ _ _ _ _ _ _ _ _ _ _ _ _ _ _ _ _ _ _ _ _ _ _ _ _ _ _ _ _ _ _ _ _ _ _ _ _ _ _ _ _ _ _ _ _ _ _ _ _ w2563 _ _ _ _ _ _ _ _ _ _ _ _ _ _ _ _ _ _ _ _ _ _ _ _ _ _ _ _ _ _ _ _ _ _ _ _ _ _ _ _ _ _ _ _ _ _ _ _ _] -> w1799
            tunnel: [_ _ _ _ _ _ _ _ _ _ _ _ _ _ _ _ _ _ _ _ _ _ _ _ _ _ _ _ _ _ _ _ _ _ _ _ _ _ _ _ _ _ _ _ _ _ _ _ _ _ _ _ _ _ _ _ _ _ _ _ _ _ _ _ _ _ _ _ _ _ _ _ _ _ _ _ _ _ _ _ _ _ _ _ _ _ _ _ _ _ _ _ _ _ _ _ _ w2572 _ _ _ _ _ _ _ _ _ _ _ _ _ _ _ _ _ _ _ _ _ _ _ _ _ _ _ _ _ _ _ _ _ _ _ _ _ _ _ _ _ _ _ _ _ _ _ _] -> w1798
            tunnel: [_ _ _ _ _ _ _ _ _ _ _ _ _ _ _ _ _ _ _ _ _ _ _ _ _ _ _ _ _ _ _ _ _ _ _ _ _ _ _ _ _ _ _ _ _ _ _ _ _ _ _ _ _ _ _ _ _ _ _ _ _ _ _ _ _ _ _ _ _ _ _ _ _ _ _ _ _ _ _ _ _ _ _ _ _ _ _ _ _ _ _ _ _ _ _ _ _ _ w2578 _ _ _ _ _ _ _ _ _ _ _ _ _ _ _ _ _ _ _ _ _ _ _ _ _ _ _ _ _ _ _ _ _ _ _ _ _ _ _ _ _ _ _ _ _ _ _] -> w1797
            tunnel: [_ _ _ _ _ _ _ _ _ _ _ _ _ _ _ _ _ _ _ _ _ _ _ _ _ _ _ _ _ _ _ _ _ _ _ _ _ _ _ _ _ _ _ _ _ _ _ _ _ _ _ _ _ _ _ _ _ _ _ _ _ _ _ _ _ _ _ _ _ _ _ _ _ _ _ _ _ _ _ _ _ _ _ _ _ _ _ _ _ _ _ _ _ _ _ _ _ _ _ w2584 _ _ _ _ _ _ _ _ _ _ _ _ _ _ _ _ _ _ _ _ _ _ _ _ _ _ _ _ _ _ _ _ _ _ _ _ _ _ _ _ _ _ _ _ _ _] -> w1796
            tunnel: [_ _ _ _ _ _ _ _ _ _ _ _ _ _ _ _ _ _ _ _ _ _ _ _ _ _ _ _ _ _ _ _ _ _ _ _ _ _ _ _ _ _ _ _ _ _ _ _ _ _ _ _ _ _ _ _ _ _ _ _ _ _ _ _ _ _ _ _ _ _ _ _ _ _ _ _ _ _ _ _ _ _ _ _ _ _ _ _ _ _ _ _ _ _ _ _ _ _ _ _ w2591 _ _ _ _ _ _ _ _ _ _ _ _ _ _ _ _ _ _ _ _ _ _ _ _ _ _ _ _ _ _ _ _ _ _ _ _ _ _ _ _ _ _ _ _ _] -> w1795
            tunnel: [_ _ _ _ _ _ _ _ _ _ _ _ _ _ _ _ _ _ _ _ _ _ _ _ _ _ _ _ _ _ _ _ _ _ _ _ _ _ _ _ _ _ _ _ _ _ _ _ _ _ _ _ _ _ _ _ _ _ _ _ _ _ _ _ _ _ _ _ _ _ _ _ _ _ _ _ _ _ _ _ _ _ _ _ _ _ _ _ _ _ _ _ _ _ _ _ _ _ _ _ _ w2600 _ _ _ _ _ _ _ _ _ _ _ _ _ _ _ _ _ _ _ _ _ _ _ _ _ _ _ _ _ _ _ _ _ _ _ _ _ _ _ _ _ _ _ _] -> w1794
            tunnel: [_ _ _ _ _ _ _ _ _ _ _ _ _ _ _ _ _ _ _ _ _ _ _ _ _ _ _ _ _ _ _ _ _ _ _ _ _ _ _ _ _ _ _ _ _ _ _ _ _ _ _ _ _ _ _ _ _ _ _ _ _ _ _ _ _ _ _ _ _ _ _ _ _ _ _ _ _ _ _ _ _ _ _ _ _ _ _ _ _ _ _ _ _ _ _ _ _ _ _ _ _ _ w2607 _ _ _ _ _ _ _ _ _ _ _ _ _ _ _ _ _ _ _ _ _ _ _ _ _ _ _ _ _ _ _ _ _ _ _ _ _ _ _ _ _ _ _] -> w1793
            tunnel: [_ _ _ _ _ _ _ _ _ _ _ _ _ _ _ _ _ _ _ _ _ _ _ _ _ _ _ _ _ _ _ _ _ _ _ _ _ _ _ _ _ _ _ _ _ _ _ _ _ _ _ _ _ _ _ _ _ _ _ _ _ _ _ _ _ _ _ _ _ _ _ _ _ _ _ _ _ _ _ _ _ _ _ _ _ _ _ _ _ _ _ _ _ _ _ _ _ _ _ _ _ _ _ w2611 _ _ _ _ _ _ _ _ _ _ _ _ _ _ _ _ _ _ _ _ _ _ _ _ _ _ _ _ _ _ _ _ _ _ _ _ _ _ _ _ _ _] -> w1792
            tunnel: [_ _ _ _ _ _ _ _ _ _ _ _ _ _ _ _ _ _ _ _ _ _ _ _ _ _ _ _ _ _ _ _ _ _ _ _ _ _ _ _ _ _ _ _ _ _ _ _ _ _ _ _ _ _ _ _ _ _ _ _ _ _ _ _ _ _ _ _ _ _ _ _ _ _ _ _ _ _ _ _ _ _ _ _ _ _ _ _ _ _ _ _ _ _ _ _ _ _ _ _ _ _ _ _ w2617 _ _ _ _ _ _ _ _ _ _ _ _ _ _ _ _ _ _ _ _ _ _ _ _ _ _ _ _ _ _ _ _ _ _ _ _ _ _ _ _ _] -> w1791
            tunnel: [_ _ _ _ _ _ _ _ _ _ _ _ _ _ _ _ _ _ _ _ _ _ _ _ _ _ _ _ _ _ _ _ _ _ _ _ _ _ _ _ _ _ _ _ _ _ _ _ _ _ _ _ _ _ _ _ _ _ _ _ _ _ _ _ _ _ _ _ _ _ _ _ _ _ _ _ _ _ _ _ _ _ _ _ _ _ _ _ _ _ _ _ _ _ _ _ _ _ _ _ _ _ _ _ _ w2628 _ _ _ _ _ _ _ _ _ _ _ _ _ _ _ _ _ _ _ _ _ _ _ _ _ _ _ _ _ _ _ _ _ _ _ _ _ _ _ _] -> w1790
            tunnel: [_ _ _ _ _ _ _ _ _ _ _ _ _ _ _ _ _ _ _ _ _ _ _ _ _ _ _ _ _ _ _ _ _ _ _ _ _ _ _ _ _ _ _ _ _ _ _ _ _ _ _ _ _ _ _ _ _ _ _ _ _ _ _ _ _ _ _ _ _ _ _ _ _ _ _ _ _ _ _ _ _ _ _ _ _ _ _ _ _ _ _ _ _ _ _ _ _ _ _ _ _ _ _ _ _ _ w2634 _ _ _ _ _ _ _ _ _ _ _ _ _ _ _ _ _ _ _ _ _ _ _ _ _ _ _ _ _ _ _ _ _ _ _ _ _ _ _] -> w1789
            tunnel: [_ _ _ _ _ _ _ _ _ _ _ _ _ _ _ _ _ _ _ _ _ _ _ _ _ _ _ _ _ _ _ _ _ _ _ _ _ _ _ _ _ _ _ _ _ _ _ _ _ _ _ _ _ _ _ _ _ _ _ _ _ _ _ _ _ _ _ _ _ _ _ _ _ _ _ _ _ _ _ _ _ _ _ _ _ _ _ _ _ _ _ _ _ _ _ _ _ _ _ _ _ _ _ _ _ _ _ w2638 _ _ _ _ _ _ _ _ _ _ _ _ _ _ _ _ _ _ _ _ _ _ _ _ _ _ _ _ _ _ _ _ _ _ _ _ _ _] -> w1788
            tunnel: [_ _ _ _ _ _ _ _ _ _ _ _ _ _ _ _ _ _ _ _ _ _ _ _ _ _ _ _ _ _ _ _ _ _ _ _ _ _ _ _ _ _ _ _ _ _ _ _ _ _ _ _ _ _ _ _ _ _ _ _ _ _ _ _ _ _ _ _ _ _ _ _ _ _ _ _ _ _ _ _ _ _ _ _ _ _ _ _ _ _ _ _ _ _ _ _ _ _ _ _ _ _ _ _ _ _ _ _ w2644 _ _ _ _ _ _ _ _ _ _ _ _ _ _ _ _ _ _ _ _ _ _ _ _ _ _ _ _ _ _ _ _ _ _ _ _ _] -> w1787
            tunnel: [_ _ _ _ _ _ _ _ _ _ _ _ _ _ _ _ _ _ _ _ _ _ _ _ _ _ _ _ _ _ _ _ _ _ _ _ _ _ _ _ _ _ _ _ _ _ _ _ _ _ _ _ _ _ _ _ _ _ _ _ _ _ _ _ _ _ _ _ _ _ _ _ _ _ _ _ _ _ _ _ _ _ _ _ _ _ _ _ _ _ _ _ _ _ _ _ _ _ _ _ _ _ _ _ _ _ _ _ _ w2655 _ _ _ _ _ _ _ _ _ _ _ _ _ _ _ _ _ _ _ _ _ _ _ _ _ _ _ _ _ _ _ _ _ _ _ _] -> w1786
            tunnel: [_ _ _ _ _ _ _ _ _ _ _ _ _ _ _ _ _ _ _ _ _ _ _ _ _ _ _ _ _ _ _ _ _ _ _ _ _ _ _ _ _ _ _ _ _ _ _ _ _ _ _ _ _ _ _ _ _ _ _ _ _ _ _ _ _ _ _ _ _ _ _ _ _ _ _ _ _ _ _ _ _ _ _ _ _ _ _ _ _ _ _ _ _ _ _ _ _ _ _ _ _ _ _ _ _ _ _ _ _ _ w2661 _ _ _ _ _ _ _ _ _ _ _ _ _ _ _ _ _ _ _ _ _ _ _ _ _ _ _ _ _ _ _ _ _ _ _] -> w1785
            tunnel: [_ _ _ _ _ _ _ _ _ _ _ _ _ _ _ _ _ _ _ _ _ _ _ _ _ _ _ _ _ _ _ _ _ _ _ _ _ _ _ _ _ _ _ _ _ _ _ _ _ _ _ _ _ _ _ _ _ _ _ _ _ _ _ _ _ _ _ _ _ _ _ _ _ _ _ _ _ _ _ _ _ _ _ _ _ _ _ _ _ _ _ _ _ _ _ _ _ _ _ _ _ _ _ _ _ _ _ _ _ _ _ w2665 _ _ _ _ _ _ _ _ _ _ _ _ _ _ _ _ _ _ _ _ _ _ _ _ _ _ _ _ _ _ _ _ _ _] -> w1784
            tunnel: [_ _ _ _ _ _ _ _ _ _ _ _ _ _ _ _ _ _ _ _ _ _ _ _ _ _ _ _ _ _ _ _ _ _ _ _ _ _ _ _ _ _ _ _ _ _ _ _ _ _ _ _ _ _ _ _ _ _ _ _ _ _ _ _ _ _ _ _ _ _ _ _ _ _ _ _ _ _ _ _ _ _ _ _ _ _ _ _ _ _ _ _ _ _ _ _ _ _ _ _ _ _ _ _ _ _ _ _ _ _ _ _ w2671 _ _ _ _ _ _ _ _ _ _ _ _ _ _ _ _ _ _ _ _ _ _ _ _ _ _ _ _ _ _ _ _ _] -> w1783
            tunnel: [_ _ _ _ _ _ _ _ _ _ _ _ _ _ _ _ _ _ _ _ _ _ _ _ _ _ _ _ _ _ _ _ _ _ _ _ _ _ _ _ _ _ _ _ _ _ _ _ _ _ _ _ _ _ _ _ _ _ _ _ _ _ _ _ _ _ _ _ _ _ _ _ _ _ _ _ _ _ _ _ _ _ _ _ _ _ _ _ _ _ _ _ _ _ _ _ _ _ _ _ _ _ _ _ _ _ _ _ _ _ _ _ _ w2682 _ _ _ _ _ _ _ _ _ _ _ _ _ _ _ _ _ _ _ _ _ _ _ _ _ _ _ _ _ _ _ _] -> w1782
            tunnel: [_ _ _ _ _ _ _ _ _ _ _ _ _ _ _ _ _ _ _ _ _ _ _ _ _ _ _ _ _ _ _ _ _ _ _ _ _ _ _ _ _ _ _ _ _ _ _ _ _ _ _ _ _ _ _ _ _ _ _ _ _ _ _ _ _ _ _ _ _ _ _ _ _ _ _ _ _ _ _ _ _ _ _ _ _ _ _ _ _ _ _ _ _ _ _ _ _ _ _ _ _ _ _ _ _ _ _ _ _ _ _ _ _ _ w2688 _ _ _ _ _ _ _ _ _ _ _ _ _ _ _ _ _ _ _ _ _ _ _ _ _ _ _ _ _ _ _] -> w1781
            tunnel: [_ _ _ _ _ _ _ _ _ _ _ _ _ _ _ _ _ _ _ _ _ _ _ _ _ _ _ _ _ _ _ _ _ _ _ _ _ _ _ _ _ _ _ _ _ _ _ _ _ _ _ _ _ _ _ _ _ _ _ _ _ _ _ _ _ _ _ _ _ _ _ _ _ _ _ _ _ _ _ _ _ _ _ _ _ _ _ _ _ _ _ _ _ _ _ _ _ _ _ _ _ _ _ _ _ _ _ _ _ _ _ _ _ _ _ w2692 _ _ _ _ _ _ _ _ _ _ _ _ _ _ _ _ _ _ _ _ _ _ _ _ _ _ _ _ _ _] -> w1780
            tunnel: [_ _ _ _ _ _ _ _ _ _ _ _ _ _ _ _ _ _ _ _ _ _ _ _ _ _ _ _ _ _ _ _ _ _ _ _ _ _ _ _ _ _ _ _ _ _ _ _ _ _ _ _ _ _ _ _ _ _ _ _ _ _ _ _ _ _ _ _ _ _ _ _ _ _ _ _ _ _ _ _ _ _ _ _ _ _ _ _ _ _ _ _ _ _ _ _ _ _ _ _ _ _ _ _ _ _ _ _ _ _ _ _ _ _ _ _ w2698 _ _ _ _ _ _ _ _ _ _ _ _ _ _ _ _ _ _ _ _ _ _ _ _ _ _ _ _ _] -> w1779
            tunnel: [_ _ _ _ _ _ _ _ _ _ _ _ _ _ _ _ _ _ _ _ _ _ _ _ _ _ _ _ _ _ _ _ _ _ _ _ _ _ _ _ _ _ _ _ _ _ _ _ _ _ _ _ _ _ _ _ _ _ _ _ _ _ _ _ _ _ _ _ _ _ _ _ _ _ _ _ _ _ _ _ _ _ _ _ _ _ _ _ _ _ _ _ _ _ _ _ _ _ _ _ _ _ _ _ _ _ _ _ _ _ _ _ _ _ _ _ _ w2710 _ _ _ _ _ _ _ _ _ _ _ _ _ _ _ _ _ _ _ _ _ _ _ _ _ _ _ _] -> w1778
            tunnel: [_ _ _ _ _ _ _ _ _ _ _ _ _ _ _ _ _ _ _ _ _ _ _ _ _ _ _ _ _ _ _ _ _ _ _ _ _ _ _ _ _ _ _ _ _ _ _ _ _ _ _ _ _ _ _ _ _ _ _ _ _ _ _ _ _ _ _ _ _ _ _ _ _ _ _ _ _ _ _ _ _ _ _ _ _ _ _ _ _ _ _ _ _ _ _ _ _ _ _ _ _ _ _ _ _ _ _ _ _ _ _ _ _ _ _ _ _ _ w2715 _ _ _ _ _ _ _ _ _ _ _ _ _ _ _ _ _ _ _ _ _ _ _ _ _ _ _] -> w1777
            tunnel: [_ _ _ _ _ _ _ _ _ _ _ _ _ _ _ _ _ _ _ _ _ _ _ _ _ _ _ _ _ _ _ _ _ _ _ _ _ _ _ _ _ _ _ _ _ _ _ _ _ _ _ _ _ _ _ _ _ _ _ _ _ _ _ _ _ _ _ _ _ _ _ _ _ _ _ _ _ _ _ _ _ _ _ _ _ _ _ _ _ _ _ _ _ _ _ _ _ _ _ _ _ _ _ _ _ _ _ _ _ _ _ _ _ _ _ _ _ _ _ w2719 _ _ _ _ _ _ _ _ _ _ _ _ _ _ _ _ _ _ _ _ _ _ _ _ _ _] -> w1776
            tunnel: [_ _ _ _ _ _ _ _ _ _ _ _ _ _ _ _ _ _ _ _ _ _ _ _ _ _ _ _ _ _ _ _ _ _ _ _ _ _ _ _ _ _ _ _ _ _ _ _ _ _ _ _ _ _ _ _ _ _ _ _ _ _ _ _ _ _ _ _ _ _ _ _ _ _ _ _ _ _ _ _ _ _ _ _ _ _ _ _ _ _ _ _ _ _ _ _ _ _ _ _ _ _ _ _ _ _ _ _ _ _ _ _ _ _ _ _ _ _ _ _ w2725 _ _ _ _ _ _ _ _ _ _ _ _ _ _ _ _ _ _ _ _ _ _ _ _ _] -> w1775
            tunnel: [_ _ _ _ _ _ _ _ _ _ _ _ _ _ _ _ _ _ _ _ _ _ _ _ _ _ _ _ _ _ _ _ _ _ _ _ _ _ _ _ _ _ _ _ _ _ _ _ _ _ _ _ _ _ _ _ _ _ _ _ _ _ _ _ _ _ _ _ _ _ _ _ _ _ _ _ _ _ _ _ _ _ _ _ _ _ _ _ _ _ _ _ _ _ _ _ _ _ _ _ _ _ _ _ _ _ _ _ _ _ _ _ _ _ _ _ _ _ _ _ _ w2736 _ _ _ _ _ _ _ _ _ _ _ _ _ _ _ _ _ _ _ _ _ _ _ _] -> w1774
            tunnel: [_ _ _ _ _ _ _ _ _ _ _ _ _ _ _ _ _ _ _ _ _ _ _ _ _ _ _ _ _ _ _ _ _ _ _ _ _ _ _ _ _ _ _ _ _ _ _ _ _ _ _ _ _ _ _ _ _ _ _ _ _ _ _ _ _ _ _ _ _ _ _ _ _ _ _ _ _ _ _ _ _ _ _ _ _ _ _ _ _ _ _ _ _ _ _ _ _ _ _ _ _ _ _ _ _ _ _ _ _ _ _ _ _ _ _ _ _ _ _ _ _ _ w2742 _ _ _ _ _ _ _ _ _ _ _ _ _ _ _ _ _ _ _ _ _ _ _] -> w1773
            tunnel: [_ _ _ _ _ _ _ _ _ _ _ _ _ _ _ _ _ _ _ _ _ _ _ _ _ _ _ _ _ _ _ _ _ _ _ _ _ _ _ _ _ _ _ _ _ _ _ _ _ _ _ _ _ _ _ _ _ _ _ _ _ _ _ _ _ _ _ _ _ _ _ _ _ _ _ _ _ _ _ _ _ _ _ _ _ _ _ _ _ _ _ _ _ _ _ _ _ _ _ _ _ _ _ _ _ _ _ _ _ _ _ _ _ _ _ _ _ _ _ _ _ _ _ w2746 _ _ _ _ _ _ _ _ _ _ _ _ _ _ _ _ _ _ _ _ _ _] -> w1772
            tunnel: [_ _ _ _ _ _ _ _ _ _ _ _ _ _ _ _ _ _ _ _ _ _ _ _ _ _ _ _ _ _ _ _ _ _ _ _ _ _ _ _ _ _ _ _ _ _ _ _ _ _ _ _ _ _ _ _ _ _ _ _ _ _ _ _ _ _ _ _ _ _ _ _ _ _ _ _ _ _ _ _ _ _ _ _ _ _ _ _ _ _ _ _ _ _ _ _ _ _ _ _ _ _ _ _ _ _ _ _ _ _ _ _ _ _ _ _ _ _ _ _ _ _ _ _ w2752 _ _ _ _ _ _ _ _ _ _ _ _ _ _ _ _ _ _ _ _ _] -> w1771
            tunnel: [_ _ _ _ _ _ _ _ _ _ _ _ _ _ _ _ _ _ _ _ _ _ _ _ _ _ _ _ _ _ _ _ _ _ _ _ _ _ _ _ _ _ _ _ _ _ _ _ _ _ _ _ _ _ _ _ _ _ _ _ _ _ _ _ _ _ _ _ _ _ _ _ _ _ _ _ _ _ _ _ _ _ _ _ _ _ _ _ _ _ _ _ _ _ _ _ _ _ _ _ _ _ _ _ _ _ _ _ _ _ _ _ _ _ _ _ _ _ _ _ _ _ _ _ _ w2763 _ _ _ _ _ _ _ _ _ _ _ _ _ _ _ _ _ _ _ _] -> w1770
            tunnel: [_ _ _ _ _ _ _ _ _ _ _ _ _ _ _ _ _ _ _ _ _ _ _ _ _ _ _ _ _ _ _ _ _ _ _ _ _ _ _ _ _ _ _ _ _ _ _ _ _ _ _ _ _ _ _ _ _ _ _ _ _ _ _ _ _ _ _ _ _ _ _ _ _ _ _ _ _ _ _ _ _ _ _ _ _ _ _ _ _ _ _ _ _ _ _ _ _ _ _ _ _ _ _ _ _ _ _ _ _ _ _ _ _ _ _ _ _ _ _ _ _ _ _ _ _ _ w2769 _ _ _ _ _ _ _ _ _ _ _ _ _ _ _ _ _ _ _] -> w1769
            tunnel: [_ _ _ _ _ _ _ _ _ _ _ _ _ _ _ _ _ _ _ _ _ _ _ _ _ _ _ _ _ _ _ _ _ _ _ _ _ _ _ _ _ _ _ _ _ _ _ _ _ _ _ _ _ _ _ _ _ _ _ _ _ _ _ _ _ _ _ _ _ _ _ _ _ _ _ _ _ _ _ _ _ _ _ _ _ _ _ _ _ _ _ _ _ _ _ _ _ _ _ _ _ _ _ _ _ _ _ _ _ _ _ _ _ _ _ _ _ _ _ _ _ _ _ _ _ _ _ w2773 _ _ _ _ _ _ _ _ _ _ _ _ _ _ _ _ _ _] -> w1768
            tunnel: [_ _ _ _ _ _ _ _ _ _ _ _ _ _ _ _ _ _ _ _ _ _ _ _ _ _ _ _ _ _ _ _ _ _ _ _ _ _ _ _ _ _ _ _ _ _ _ _ _ _ _ _ _ _ _ _ _ _ _ _ _ _ _ _ _ _ _ _ _ _ _ _ _ _ _ _ _ _ _ _ _ _ _ _ _ _ _ _ _ _ _ _ _ _ _ _ _ _ _ _ _ _ _ _ _ _ _ _ _ _ _ _ _ _ _ _ _ _ _ _ _ _ _ _ _ _ _ _ w2779 _ _ _ _ _ _ _ _ _ _ _ _ _ _ _ _ _] -> w1767
            tunnel: [_ _ _ _ _ _ _ _ _ _ _ _ _ _ _ _ _ _ _ _ _ _ _ _ _ _ _ _ _ _ _ _ _ _ _ _ _ _ _ _ _ _ _ _ _ _ _ _ _ _ _ _ _ _ _ _ _ _ _ _ _ _ _ _ _ _ _ _ _ _ _ _ _ _ _ _ _ _ _ _ _ _ _ _ _ _ _ _ _ _ _ _ _ _ _ _ _ _ _ _ _ _ _ _ _ _ _ _ _ _ _ _ _ _ _ _ _ _ _ _ _ _ _ _ _ _ _ _ _ w2790 _ _ _ _ _ _ _ _ _ _ _ _ _ _ _ _] -> w1766
            tunnel: [_ _ _ _ _ _ _ _ _ _ _ _ _ _ _ _ _ _ _ _ _ _ _ _ _ _ _ _ _ _ _ _ _ _ _ _ _ _ _ _ _ _ _ _ _ _ _ _ _ _ _ _ _ _ _ _ _ _ _ _ _ _ _ _ _ _ _ _ _ _ _ _ _ _ _ _ _ _ _ _ _ _ _ _ _ _ _ _ _ _ _ _ _ _ _ _ _ _ _ _ _ _ _ _ _ _ _ _ _ _ _ _ _ _ _ _ _ _ _ _ _ _ _ _ _ _ _ _ _ _ w2796 _ _ _ _ _ _ _ _ _ _ _ _ _ _ _] -> w1765
            tunnel: [_ _ _ _ _ _ _ _ _ _ _ _ _ _ _ _ _ _ _ _ _ _ _ _ _ _ _ _ _ _ _ _ _ _ _ _ _ _ _ _ _ _ _ _ _ _ _ _ _ _ _ _ _ _ _ _ _ _ _ _ _ _ _ _ _ _ _ _ _ _ _ _ _ _ _ _ _ _ _ _ _ _ _ _ _ _ _ _ _ _ _ _ _ _ _ _ _ _ _ _ _ _ _ _ _ _ _ _ _ _ _ _ _ _ _ _ _ _ _ _ _ _ _ _ _ _ _ _ _ _ _ w2800 _ _ _ _ _ _ _ _ _ _ _ _ _ _] -> w1764
            tunnel: [_ _ _ _ _ _ _ _ _ _ _ _ _ _ _ _ _ _ _ _ _ _ _ _ _ _ _ _ _ _ _ _ _ _ _ _ _ _ _ _ _ _ _ _ _ _ _ _ _ _ _ _ _ _ _ _ _ _ _ _ _ _ _ _ _ _ _ _ _ _ _ _ _ _ _ _ _ _ _ _ _ _ _ _ _ _ _ _ _ _ _ _ _ _ _ _ _ _ _ _ _ _ _ _ _ _ _ _ _ _ _ _ _ _ _ _ _ _ _ _ _ _ _ _ _ _ _ _ _ _ _ _ w2806 _ _ _ _ _ _ _ _ _ _ _ _ _] -> w1763
            tunnel: [_ _ _ _ _ _ _ _ _ _ _ _ _ _ _ _ _ _ _ _ _ _ _ _ _ _ _ _ _ _ _ _ _ _ _ _ _ _ _ _ _ _ _ _ _ _ _ _ _ _ _ _ _ _ _ _ _ _ _ _ _ _ _ _ _ _ _ _ _ _ _ _ _ _ _ _ _ _ _ _ _ _ _ _ _ _ _ _ _ _ _ _ _ _ _ _ _ _ _ _ _ _ _ _ _ _ _ _ _ _ _ _ _ _ _ _ _ _ _ _ _ _ _ _ _ _ _ _ _ _ _ _ _ w2817 _ _ _ _ _ _ _ _ _ _ _ _] -> w1762
            tunnel: [_ _ _ _ _ _ _ _ _ _ _ _ _ _ _ _ _ _ _ _ _ _ _ _ _ _ _ _ _ _ _ _ _ _ _ _ _ _ _ _ _ _ _ _ _ _ _ _ _ _ _ _ _ _ _ _ _ _ _ _ _ _ _ _ _ _ _ _ _ _ _ _ _ _ _ _ _ _ _ _ _ _ _ _ _ _ _ _ _ _ _ _ _ _ _ _ _ _ _ _ _ _ _ _ _ _ _ _ _ _ _ _ _ _ _ _ _ _ _ _ _ _ _ _ _ _ _ _ _ _ _ _ _ _ w2823 _ _ _ _ _ _ _ _ _ _ _] -> w1761
            tunnel: [_ _ _ _ _ _ _ _ _ _ _ _ _ _ _ _ _ _ _ _ _ _ _ _ _ _ _ _ _ _ _ _ _ _ _ _ _ _ _ _ _ _ _ _ _ _ _ _ _ _ _ _ _ _ _ _ _ _ _ _ _ _ _ _ _ _ _ _ _ _ _ _ _ _ _ _ _ _ _ _ _ _ _ _ _ _ _ _ _ _ _ _ _ _ _ _ _ _ _ _ _ _ _ _ _ _ _ _ _ _ _ _ _ _ _ _ _ _ _ _ _ _ _ _ _ _ _ _ _ _ _ _ _ _ _ w2828 _ _ _ _ _ _ _ _ _ _] -> w1760
            tunnel: [_ _ _ _ _ _ _ _ _ _ _ _ _ _ _ _ _ _ _ _ _ _ _ _ _ _ _ _ _ _ _ _ _ _ _ _ _ _ _ _ _ _ _ _ _ _ _ _ _ _ _ _ _ _ _ _ _ _ _ _ _ _ _ _ _ _ _ _ _ _ _ _ _ _ _ _ _ _ _ _ _ _ _ _ _ _ _ _ _ _ _ _ _ _ _ _ _ _ _ _ _ _ _ _ _ _ _ _ _ _ _ _ _ _ _ _ _ _ _ _ _ _ _ _ _ _ _ _ _ _ _ _ _ _ _ _ w2835 _ _ _ _ _ _ _ _ _] -> w1759
            tunnel: [_ _ _ _ _ _ _ _ _ _ _ _ _ _ _ _ _ _ _ _ _ _ _ _ _ _ _ _ _ _ _ _ _ _ _ _ _ _ _ _ _ _ _ _ _ _ _ _ _ _ _ _ _ _ _ _ _ _ _ _ _ _ _ _ _ _ _ _ _ _ _ _ _ _ _ _ _ _ _ _ _ _ _ _ _ _ _ _ _ _ _ _ _ _ _ _ _ _ _ _ _ _ _ _ _ _ _ _ _ _ _ _ _ _ _ _ _ _ _ _ _ _ _ _ _ _ _ _ _ _ _ _ _ _ _ _ _ w2842 _ _ _ _ _ _ _ _] -> w1758
            tunnel: [_ _ _ _ _ _ _ _ _ _ _ _ _ _ _ _ _ _ _ _ _ _ _ _ _ _ _ _ _ _ _ _ _ _ _ _ _ _ _ _ _ _ _ _ _ _ _ _ _ _ _ _ _ _ _ _ _ _ _ _ _ _ _ _ _ _ _ _ _ _ _ _ _ _ _ _ _ _ _ _ _ _ _ _ _ _ _ _ _ _ _ _ _ _ _ _ _ _ _ _ _ _ _ _ _ _ _ _ _ _ _ _ _ _ _ _ _ _ _ _ _ _ _ _ _ _ _ _ _ _ _ _ _ _ _ _ _ _ w2849 _ _ _ _ _ _ _] -> w1757
            tunnel: [_ _ _ _ _ _ _ _ _ _ _ _ _ _ _ _ _ _ _ _ _ _ _ _ _ _ _ _ _ _ _ _ _ _ _ _ _ _ _ _ _ _ _ _ _ _ _ _ _ _ _ _ _ _ _ _ _ _ _ _ _ _ _ _ _ _ _ _ _ _ _ _ _ _ _ _ _ _ _ _ _ _ _ _ _ _ _ _ _ _ _ _ _ _ _ _ _ _ _ _ _ _ _ _ _ _ _ _ _ _ _ _ _ _ _ _ _ _ _ _ _ _ _ _ _ _ _ _ _ _ _ _ _ _ _ _ _ _ _ w2854 _ _ _ _ _ _] -> w1756
            tunnel: [_ _ _ _ _ _ _ _ _ _ _ _ _ _ _ _ _ _ _ _ _ _ _ _ _ _ _ _ _ _ _ _ _ _ _ _ _ _ _ _ _ _ _ _ _ _ _ _ _ _ _ _ _ _ _ _ _ _ _ _ _ _ _ _ _ _ _ _ _ _ _ _ _ _ _ _ _ _ _ _ _ _ _ _ _ _ _ _ _ _ _ _ _ _ _ _ _ _ _ _ _ _ _ _ _ _ _ _ _ _ _ _ _ _ _ _ _ _ _ _ _ _ _ _ _ _ _ _ _ _ _ _ _ _ _ _ _ _ _ _ w2860 _ _ _ _ _] -> w1755
            tunnel: [_ _ _ _ _ _ _ _ _ _ _ _ _ _ _ _ _ _ _ _ _ _ _ _ _ _ _ _ _ _ _ _ _ _ _ _ _ _ _ _ _ _ _ _ _ _ _ _ _ _ _ _ _ _ _ _ _ _ _ _ _ _ _ _ _ _ _ _ _ _ _ _ _ _ _ _ _ _ _ _ _ _ _ _ _ _ _ _ _ _ _ _ _ _ _ _ _ _ _ _ _ _ _ _ _ _ _ _ _ _ _ _ _ _ _ _ _ _ _ _ _ _ _ _ _ _ _ _ _ _ _ _ _ _ _ _ _ _ _ _ _ w2867 _ _ _ _] -> w1754
            tunnel: [_ _ _ _ _ _ _ _ _ _ _ _ _ _ _ _ _ _ _ _ _ _ _ _ _ _ _ _ _ _ _ _ _ _ _ _ _ _ _ _ _ _ _ _ _ _ _ _ _ _ _ _ _ _ _ _ _ _ _ _ _ _ _ _ _ _ _ _ _ _ _ _ _ _ _ _ _ _ _ _ _ _ _ _ _ _ _ _ _ _ _ _ _ _ _ _ _ _ _ _ _ _ _ _ _ _ _ _ _ _ _ _ _ _ _ _ _ _ _ _ _ _ _ _ _ _ _ _ _ _ _ _ _ _ _ _ _ _ _ _ _ _ w2872 _ _ _] -> w1753
            tunnel: [_ _ _ _ _ _ _ _ _ _ _ _ _ _ _ _ _ _ _ _ _ _ _ _ _ _ _ _ _ _ _ _ _ _ _ _ _ _ _ _ _ _ _ _ _ _ _ _ _ _ _ _ _ _ _ _ _ _ _ _ _ _ _ _ _ _ _ _ _ _ _ _ _ _ _ _ _ _ _ _ _ _ _ _ _ _ _ _ _ _ _ _ _ _ _ _ _ _ _ _ _ _ _ _ _ _ _ _ _ _ _ _ _ _ _ _ _ _ _ _ _ _ _ _ _ _ _ _ _ _ _ _ _ _ _ _ _ _ _ _ _ _ _ w2881 _ _] -> w1752
            tunnel: [_ _ _ _ _ _ _ _ _ _ _ _ _ _ _ _ _ _ _ _ _ _ _ _ _ _ _ _ _ _ _ _ _ _ _ _ _ _ _ _ _ _ _ _ _ _ _ _ _ _ _ _ _ _ _ _ _ _ _ _ _ _ _ _ _ _ _ _ _ _ _ _ _ _ _ _ _ _ _ _ _ _ _ _ _ _ _ _ _ _ _ _ _ _ _ _ _ _ _ _ _ _ _ _ _ _ _ _ _ _ _ _ _ _ _ _ _ _ _ _ _ _ _ _ _ _ _ _ _ _ _ _ _ _ _ _ _ _ _ _ _ _ _ _ w2887 _] -> w1751
            tunnel: [_ _ _ _ _ _ _ _ _ _ _ _ _ _ _ _ _ _ _ _ _ _ _ _ _ _ _ _ _ _ _ _ _ _ _ _ _ _ _ _ _ _ _ _ _ _ _ _ _ _ _ _ _ _ _ _ _ _ _ _ _ _ _ _ _ _ _ _ _ _ _ _ _ _ _ _ _ _ _ _ _ _ _ _ _ _ _ _ _ _ _ _ _ _ _ _ _ _ _ _ _ _ _ _ _ _ _ _ _ _ _ _ _ _ _ _ _ _ _ _ _ _ _ _ _ _ _ _ _ _ _ _ _ _ _ _ _ _ _ _ _ _ _ _ _ w2893] -> w1750
            frame #0 {
              w1915 = "\r"
              w1913 = "\t"
              n1937 = local read "Recipe Name"() -> (w1914:string)
              n1938 = Format Into String(format string="%s%s%s%s%s%s%s%s", "\r", "Recipe Name:" ("string"), w1913, w1913, w1913, w1914, w1915, w1915) -> (resulting string=w1912:string)  [unwired: 2 in, 1 out]
            }
            frame #1 {
              w1922 = "\r"
              w1920 = "\t"
              n1939 = local read "Substrate Material"() -> (w1921:string)
              n1940 = Format Into String(format string="%s%s%s%s%s%s%s%s", "\r", "Substrate Material:" ("string"), w1920, w1920, w1921, w1922, w1922, w1922) -> (resulting string=w1919:string)  [unwired: 2 in, 1 out]
            }
            frame #2 {
              w1927 = "\r"
              w1929 = "\t"
              n1941 = local read "Recipe_selection tab"() -> (w1930:T1)
              n1942 = case shown="\"Multilayer Recipe                                                                  \"" w1930 {
                tunnel: ["Single" ("string") "Multilayer" ("string")] -> w1928
                frame #0 {
                }
                frame #1 {
                }
              }
              n1943 = Format Into String(format string="%s%s%s%s%s%s", "Recipe Selection:" ("input 1"), w1929, w1929, w1928, w1927, w1927) -> (resulting string=w1926:string)  [unwired: 2 in, 1 out]
            }
            frame #3 {
              w1938 = "\r"
              w1936 = "\t"
              n1944 = local read "R_Web_selection"() -> (w1939:enum32{"Web", "Other"})
              n1945 = case shown="\"Web\", Default" w1939 {
                tunnel: ["Web" ("string") "Other" ("string")] -> w1937
                frame #0 {
                }
                frame #1 {
                }
              }
              n1946 = Format Into String(format string="%s%s%s%s%s%s%s", "Web Selection:" ("input 1"), w1936, w1936, w1936, w1937, w1938, w1938) -> (resulting string=w1935:string)  [unwired: 2 in, 1 out]
            }
            frame #4 {
              w1945 = "\t"
              n1947 = Format Into String(format string="%s%s%s", "Web Parameters" ("input 1"), w1945, w1945) -> (resulting string=w1944:string)  [unwired: 2 in, 1 out]
            }
            frame #5 {
              w1950 = "\t"
              n1948 = local read "R Minimum diameter"() -> (w1949:dbl)
              n1949 = Format Into String(format string="%s%s%s%s%.1f", "\r", "Minimum Diameter(mm):" ("input 2"), w1950, w1950, w1949) -> (resulting string=w1948:string)  [unwired: 2 in, 1 out]
            }
            frame #6 {
              w1956 = "\t"
              n1950 = local read "R Maximum diameter"() -> (w1955:dbl)
              n1951 = Format Into String(format string="%s%s%s%s%.1f", "\r", "Maximum Diameter(mm):" ("input 2"), w1956, w1956, w1955) -> (resulting string=w1954:string)  [unwired: 2 in, 1 out]
            }
            frame #7 {
              w1962 = "\t"
              n1952 = local read "R Web thickness"() -> (w1961:dbl)
              n1953 = Format Into String(format string="%s%s%s%s%d", "\r", "Web Thickness(µm):" ("input 2"), w1962, w1962, w1961) -> (resulting string=w1960:string)  [unwired: 2 in, 1 out]
            }
            frame #8 {
              w1968 = "\t"
              n1954 = local read "R Web speed(cm/min)"() -> (w1967:dbl)
              n1955 = Format Into String(format string="%s%s%s%s%d", "\r", "Web Speed(cm/min):" ("input 2"), w1968, w1968, w1967) -> (resulting string=w1966:string)  [unwired: 2 in, 1 out]
            }
            frame #9 {
              w1974 = "\t"
              n1956 = local read "R Tension Value"() -> (w1973:dbl)
              n1957 = Format Into String(format string="%s%s%s%s%d", "\r", "Tension Value(N):" ("input 2"), w1974, w1974, w1973) -> (resulting string=w1972:string)  [unwired: 2 in, 1 out]
            }
            frame #10 {
              w1980 = "\r"
              w1981 = "\t"
              n1958 = local read "R  Total length"() -> (w1979:dbl)
              n1959 = Format Into String(format string="%s%s%s%s%s%.1f%s%s", "\r", "Total Length:" ("input 2"), w1981, w1981, w1981, w1979, w1980, w1980) -> (resulting string=w1978:string)  [unwired: 2 in, 1 out]
            }
            frame #11 {
              w1987 = "\t"
              n1960 = Format Into String(format string="%s%s%s%s", "Other Parameters" ("input 1"), w1987, w1987, "\r") -> (resulting string=w1985:string)  [unwired: 2 in, 1 out]
            }
            frame #12 {
              w1991 = "\t"
              n1961 = local read "R_Thickness Selection"() -> (w1995:enum32{"Thickness", "Time"})
              n1962 = case shown="\"Thickness\", Default" w1995 {
                tunnel: ["Thickness" ("input 3") "Time" ("input 3")] -> w1992
                frame #0 {
                }
                frame #1 {
                }
              }
              n1963 = Format Into String(format string="%s%s%s%s", "Thickness Selection:" ("input 1"), w1991, w1991, w1992) -> (resulting string=w1990:string)  [unwired: 2 in, 1 out]
            }
            frame #13 {
              n1964 = local read "R_Target Thickness Value"() -> (w1999:dbl)
              n1965 = Format Into String(format string="%s%s%s%d", "\r", "Target Thicness Value(nm):" ("input 2"), "\t", w1999) -> (resulting string=w1998:string)  [unwired: 2 in, 1 out]
            }
            frame #14 {
              w2005 = "\r"
              w2007 = "\t"
              n1966 = local read "R_Duration"() -> (w2006:dbl)
              n1967 = Format Into String(format string="%s%s%s%s%s%d%s%s", "\r", "Time(s):" ("input 2"), w2007, w2007, w2007, w2006, w2005, w2005) -> (resulting string=w2004:string)  [unwired: 2 in, 1 out]
            }
            frame #15 {
              w2013 = "\t"
              n1968 = Format Into String(format string="%s%s%s%s", "Single Recipe Parameters" ("input 1"), w2013, w2013, "\r") -> (resulting string=w2011:string)  [unwired: 2 in, 1 out]
            }
            frame #16 {
              n1969 = local read "R_Simple_Coating Type Selection"() -> (w2019:T2)
              n1970 = case shown="\"Microwave Plasma\", Default" w2019 {
                tunnel: ["Microwave Plasma" ("string") "DC Sputter" ("string") "RF Sputter" ("string")] -> w2017
                frame #0 {
                }
                frame #1 {
                }
                frame #2 {
                }
              }
              n1971 = Format Into String(format string="%s%s%s%s", "Single  Process Selection:" ("input 1"), "\t", w2017, "\r") -> (resulting string=w2018:string)  [unwired: 2 in, 1 out]
            }
            frame #17 {
              w2027 = "\t"
              n1972 = Format Into String(format string="%s%s%s", "Microwave Plasma Parameters" ("input 1"), w2027, w2027) -> (resulting string=w2026:string)  [unwired: 2 in, 1 out]
            }
            frame #18 {
              n1973 = local read "R_Single Microwave Power"() -> (w2031:dbl)
              n1974 = Format Into String(format string="%s%s%s%d", "\r", "Microwave Plasma Power(W):" ("input 2"), "\t", w2031) -> (resulting string=w2030:string)  [unwired: 2 in, 1 out]
            }
            frame #19 {
              n1975 = local read "R_Single Microwave Time"() -> (w2037:dbl)
              n1976 = Format Into String(format string="%s%s%s%d", "\r", "Microwave Plasma Time(s):" ("input 2"), "\t", w2037) -> (resulting string=w2036:string)  [unwired: 2 in, 1 out]
            }
            frame #20 {
              w2042 = "\r"
              w2045 = "\t"
              n1977 = local read "R Single Pass Number"() -> (w2043:dbl)
              n1978 = Format Into String(format string="%s%s%s%s%s%d%s%s", "\r", "Pass Number:" ("input 2"), w2045, w2045, w2045, w2043, w2042, w2042) -> (resulting string=w2044:string)  [unwired: 2 in, 1 out]
            }
            frame #21 {
              w2050 = "\r"
              w2051 = "\t"
              n1979 = Format Into String(format string="%s%s%s%s%s", "DC Sputter Parameters" ("input 1"), w2051, w2051, w2050, w2050) -> (resulting string=w2049:string)  [unwired: 2 in, 1 out]
            }
            frame #22 {
              w2058 = "\t"
              n1980 = local read "R_DC_Chamber_selection"() -> (w2056:enum32{"Chamber II", "Chamber III"})
              n1981 = case shown="\"Chamber II\", Default" w2056 {
                tunnel: ["Chamber II" ("string") "Chamber III" ("string")] -> w2057
                frame #0 {
                }
                frame #1 {
                }
              }
              n1982 = Format Into String(format string="%s%s%s%s%s%s", "\r", "DC Chamber Selection :" ("input 2"), w2058, w2058, w2057, "\r") -> (resulting string=w2054:string)  [unwired: 2 in, 1 out]
            }
            frame #23 {
              w2066 = "\t"
              n1983 = local read "R Single DC Target material"() -> (w2065:string)
              n1984 = Format Into String(format string="%s%s%s%s", "Target Material:" ("string"), w2066, w2066, w2065) -> (resulting string=w2064:string)  [unwired: 2 in, 1 out]
            }
            frame #24 {
              w2071 = "\t"
              n1985 = local read "R Single DC Step1 Coating Power Active"() -> (w2072:bool)
              n1986 = case shown="True" w2072 {
                tunnel: ["Deactive" ("input 4") "Active" ("input 4")] -> w2070
                frame #0 {
                }
                frame #1 {
                }
              }
              n1987 = Format Into String(format string="%s%s%s%s%s%s", "\r", "Region 1:" ("input 2"), w2071, w2071, w2071, w2070) -> (resulting string=w2069:string)  [unwired: 2 in, 1 out]
            }
            frame #25 {
              w2083 = "\t"
              n1988 = local read "R Single DC Step1 Coating Power"() -> (w2079:dbl)
              n1989 = Format Into String(format string="%s%s%s%s%s%d", "\r", "Power(W):" ("input 2"), w2083, w2083, w2083, w2079) -> (resulting string=w2078:string)  [unwired: 2 in, 1 out]
            }
            frame #26 {
              w2086 = "\t"
              n1990 = local read "R Single DC Interval length1"() -> (w2085:dbl)
              n1991 = Format Into String(format string="%s%s%s%s%d", "\r", "Interval Length(m):" ("input 2"), w2086, w2086, w2085) -> (resulting string=w2084:string)  [unwired: 2 in, 1 out]
            }
            frame #27 {
              w2091 = "\t"
              n1992 = local read "R Single DC Step2 Coating Power Active"() -> (w2093:bool)
              n1993 = case shown="True" w2093 {
                tunnel: ["Deactive" ("input 4") "Active" ("input 4")] -> w2092
                frame #0 {
                }
                frame #1 {
                }
              }
              n1994 = Format Into String(format string="%s%s%s%s%s%s", "\r", "Region 2:" ("input 2"), w2091, w2091, w2091, w2092) -> (resulting string=w2090:string)  [unwired: 2 in, 1 out]
            }
            frame #28 {
              w2104 = "\t"
              n1995 = local read "R Single DC Step2 Coating Power"() -> (w2100:dbl)
              n1996 = Format Into String(format string="%s%s%s%s%s%d", "\r", "Power(W):" ("input 2"), w2104, w2104, w2104, w2100) -> (resulting string=w2099:string)  [unwired: 2 in, 1 out]
            }
            frame #29 {
              w2107 = "\t"
              n1997 = local read "R Single DC Interval length2"() -> (w2106:dbl)
              n1998 = Format Into String(format string="%s%s%s%s%d", "\r", "Interval Length(m):" ("input 2"), w2107, w2107, w2106) -> (resulting string=w2105:string)  [unwired: 2 in, 1 out]
            }
            frame #30 {
              w2113 = "\t"
              n1999 = local read "R Single DC Step3 Coating Power Active"() -> (w2114:bool)
              n2000 = case shown="True" w2114 {
                tunnel: ["Deactive" ("input 4") "Active" ("input 4")] -> w2112
                frame #0 {
                }
                frame #1 {
                }
              }
              n2001 = Format Into String(format string="%s%s%s%s%s%s", "\r", "Region 3:" ("input 2"), w2113, w2113, w2113, w2112) -> (resulting string=w2111:string)  [unwired: 2 in, 1 out]
            }
            frame #31 {
              w2125 = "\t"
              n2002 = local read "R Single DC Step3 Coating Power"() -> (w2120:dbl)
              n2003 = Format Into String(format string="%s%s%s%s%s%d", "\r", "Power(W):" ("input 2"), w2125, w2125, w2125, w2120) -> (resulting string=w2121:string)  [unwired: 2 in, 1 out]
            }
            frame #32 {
              w2128 = "\t"
              n2004 = local read "R Single DC Interval length3"() -> (w2127:dbl)
              n2005 = Format Into String(format string="%s%s%s%s%d", "\r", "Interval Length(m):" ("input 2"), w2128, w2128, w2127) -> (resulting string=w2126:string)  [unwired: 2 in, 1 out]
            }
            frame #33 {
              w2133 = "\t"
              n2006 = local read "R Single DC Step4 Coating Power Active"() -> (w2135:bool)
              n2007 = case shown="True" w2135 {
                tunnel: ["Deactive" ("input 4") "Active" ("input 4")] -> w2134
                frame #0 {
                }
                frame #1 {
                }
              }
              n2008 = Format Into String(format string="%s%s%s%s%s%s", "\r", "Region 4:" ("input 2"), w2133, w2133, w2133, w2134) -> (resulting string=w2132:string)  [unwired: 2 in, 1 out]
            }
            frame #34 {
              w2146 = "\t"
              n2009 = local read "R Single DC Step4 Coating Power"() -> (w2141:dbl)
              n2010 = Format Into String(format string="%s%s%s%s%s%d", "\r", "Power(W):" ("input 2"), w2146, w2146, w2146, w2141) -> (resulting string=w2142:string)  [unwired: 2 in, 1 out]
            }
            frame #35 {
              w2149 = "\t"
              n2011 = local read "R Single DC Interval length4"() -> (w2148:dbl)
              n2012 = Format Into String(format string="%s%s%s%s%d", "\r", "Interval Length(m):" ("input 2"), w2149, w2149, w2148) -> (resulting string=w2147:string)  [unwired: 2 in, 1 out]
            }
            frame #36 {
              w2154 = "\t"
              n2013 = local read "R Single DC Step5 Coating Power Active"() -> (w2156:bool)
              n2014 = case shown="True" w2156 {
                tunnel: ["Deactive" ("input 4") "Active" ("input 4")] -> w2155
                frame #0 {
                }
                frame #1 {
                }
              }
              n2015 = Format Into String(format string="%s%s%s%s%s%s", "\r", "Region 5:" ("input 2"), w2154, w2154, w2154, w2155) -> (resulting string=w2153:string)  [unwired: 2 in, 1 out]
            }
            frame #37 {
              w2167 = "\t"
              n2016 = local read "R Single DC Step5 Coating Power"() -> (w2162:dbl)
              n2017 = Format Into String(format string="%s%s%s%s%s%d", "\r", "Power(W):" ("input 2"), w2167, w2167, w2167, w2162) -> (resulting string=w2163:string)  [unwired: 2 in, 1 out]
            }
            frame #38 {
              w2170 = "\t"
              n2018 = local read "R Single DC Interval length5"() -> (w2169:dbl)
              n2019 = Format Into String(format string="%s%s%s%s%d", "\r", "Interval Length(m):" ("input 2"), w2170, w2170, w2169) -> (resulting string=w2168:string)  [unwired: 2 in, 1 out]
            }
            frame #39 {
              w2175 = "\t"
              n2020 = local read "R Single DC Step6 Coating Power Active"() -> (w2177:bool)
              n2021 = case shown="True" w2177 {
                tunnel: ["Deactive" ("input 4") "Active" ("input 4")] -> w2176
                frame #0 {
                }
                frame #1 {
                }
              }
              n2022 = Format Into String(format string="%s%s%s%s%s%s", "\r", "Region 6:" ("input 2"), w2175, w2175, w2175, w2176) -> (resulting string=w2174:string)  [unwired: 2 in, 1 out]
            }
            frame #40 {
              w2188 = "\t"
              n2023 = local read "R Single DC Step6 Coating Power"() -> (w2183:dbl)
              n2024 = Format Into String(format string="%s%s%s%s%s%d", "\r", "Power(W):" ("input 2"), w2188, w2188, w2188, w2183) -> (resulting string=w2184:string)  [unwired: 2 in, 1 out]
            }
            frame #41 {
              w2191 = "\t"
              n2025 = local read "R Single DC Interval length6"() -> (w2190:dbl)
              n2026 = Format Into String(format string="%s%s%s%s%d", "\r", "Interval Length(m):" ("input 2"), w2191, w2191, w2190) -> (resulting string=w2189:string)  [unwired: 2 in, 1 out]
            }
            frame #42 {
              w2196 = "\t"
              n2027 = local read "R Single DC Step7 Coating Power Active"() -> (w2198:bool)
              n2028 = case shown="True" w2198 {
                tunnel: ["Deactive" ("input 4") "Active" ("input 4")] -> w2197
                frame #0 {
                }
                frame #1 {
                }
              }
              n2029 = Format Into String(format string="%s%s%s%s%s%s", "\r", "Region 7:" ("input 2"), w2196, w2196, w2196, w2197) -> (resulting string=w2195:string)  [unwired: 2 in, 1 out]
            }
            frame #43 {
              w2209 = "\t"
              n2030 = local read "R Single DC Step7 Coating Power"() -> (w2204:dbl)
              n2031 = Format Into String(format string="%s%s%s%s%s%d", "\r", "Power(W):" ("input 2"), w2209, w2209, w2209, w2204) -> (resulting string=w2205:string)  [unwired: 2 in, 1 out]
            }
            frame #44 {
              w2212 = "\t"
              n2032 = local read "R Single DC Interval length7"() -> (w2211:dbl)
              n2033 = Format Into String(format string="%s%s%s%s%d", "\r", "Interval Length(m):" ("input 2"), w2212, w2212, w2211) -> (resulting string=w2210:string)  [unwired: 2 in, 1 out]
            }
            frame #45 {
              w2217 = "\t"
              n2034 = local read "R Single DC Step8 Coating Power Active"() -> (w2219:bool)
              n2035 = case shown="True" w2219 {
                tunnel: ["Deactive" ("input 4") "Active" ("input 4")] -> w2218
                frame #0 {
                }
                frame #1 {
                }
              }
              n2036 = Format Into String(format string="%s%s%s%s%s%s", "\r", "Region 8:" ("input 2"), w2217, w2217, w2217, w2218) -> (resulting string=w2216:string)  [unwired: 2 in, 1 out]
            }
            frame #46 {
              w2230 = "\t"
              n2037 = local read "R Single DC Step8 Coating Power"() -> (w2225:dbl)
              n2038 = Format Into String(format string="%s%s%s%s%s%d", "\r", "Power(W):" ("input 2"), w2230, w2230, w2230, w2225) -> (resulting string=w2226:string)  [unwired: 2 in, 1 out]
            }
            frame #47 {
              w2233 = "\t"
              n2039 = local read "R Single DC Interval length8"() -> (w2232:dbl)
              n2040 = Format Into String(format string="%s%s%s%s%d", "\r", "Interval Length(m):" ("input 2"), w2233, w2233, w2232) -> (resulting string=w2231:string)  [unwired: 2 in, 1 out]
            }
            frame #48 {
              w2238 = "\t"
              n2041 = local read "R Single DC Step9 Coating Power Active"() -> (w2240:bool)
              n2042 = case shown="True" w2240 {
                tunnel: ["Deactive" ("input 4") "Active" ("input 4")] -> w2239
                frame #0 {
                }
                frame #1 {
                }
              }
              n2043 = Format Into String(format string="%s%s%s%s%s%s", "\r", "Region 9:" ("input 2"), w2238, w2238, w2238, w2239) -> (resulting string=w2237:string)  [unwired: 2 in, 1 out]
            }
            frame #49 {
              w2251 = "\t"
              n2044 = local read "R Single DC Step9 Coating Power"() -> (w2247:dbl)
              n2045 = Format Into String(format string="%s%s%s%s%s%d", "\r", "Power(W):" ("input 2"), w2251, w2251, w2251, w2247) -> (resulting string=w2246:string)  [unwired: 2 in, 1 out]
            }
            frame #50 {
              w2254 = "\t"
              n2046 = local read "R Single DC Interval length9"() -> (w2253:dbl)
              n2047 = Format Into String(format string="%s%s%s%s%d", "\r", "Interval Length(m):" ("input 2"), w2254, w2254, w2253) -> (resulting string=w2252:string)  [unwired: 2 in, 1 out]
            }
            frame #51 {
              w2259 = "\t"
              n2048 = local read "R Single DC Step10 Coating Power Active"() -> (w2261:bool)
              n2049 = case shown="True" w2261 {
                tunnel: ["Deactive" ("input 4") "Active" ("input 4")] -> w2260
                frame #0 {
                }
                frame #1 {
                }
              }
              n2050 = Format Into String(format string="%s%s%s%s%s%s", "\r", "Region 10:" ("input 2"), w2259, w2259, w2259, w2260) -> (resulting string=w2258:string)  [unwired: 2 in, 1 out]
            }
            frame #52 {
              w2272 = "\t"
              n2051 = local read "R Single DC Step10 Coating Power"() -> (w2267:dbl)
              n2052 = Format Into String(format string="%s%s%s%s%s%d", "\r", "Power(W):" ("input 2"), w2272, w2272, w2272, w2267) -> (resulting string=w2268:string)  [unwired: 2 in, 1 out]
            }
            frame #53 {
              w2274 = "\r"
              w2276 = "\t"
              n2053 = local read "R Single DC Interval length10"() -> (w2275:dbl)
              n2054 = Format Into String(format string="%s%s%s%s%d%s%s", "\r", "Interval Length(m):" ("input 2"), w2276, w2276, w2275, w2274, w2274) -> (resulting string=w2273:string)  [unwired: 2 in, 1 out]
            }
            frame #54 {
              w2281 = "\t"
              n2055 = Format Into String(format string="%s%s%s", "RF Sputter Parameters" ("input 1"), w2281, w2281) -> (resulting string=w2280:string)  [unwired: 2 in, 1 out]
            }
            frame #55 {
              w2286 = "\t"
              n2056 = local read "R Single RF Target material"() -> (w2285:string)
              n2057 = Format Into String(format string="%s%s%s%s%s", "\r", "Target Material:" ("input 2"), w2286, w2286, w2285) -> (resulting string=w2284:string)  [unwired: 2 in, 1 out]
            }
            frame #56 {
              w2293 = "\t"
              n2058 = local read "R Single RF Ramp up"() -> (w2291:bool)
              n2059 = case shown="True" w2291 {
                tunnel: ["Deactive" ("input 4") "Active" ("input 4")] -> w2292
                frame #0 {
                }
                frame #1 {
                }
              }
              n2060 = Format Into String(format string="%s%s%s%s%s", "\r", "Ramp Up Time(s):" ("input 2"), w2293, w2293, w2292) -> (resulting string=w2290:string)  [unwired: 2 in, 1 out]
            }
            frame #57 {
              w2301 = "\t"
              n2061 = local read "R Single RF Ramp up Time"() -> (w2300:dbl)
              n2062 = Format Into String(format string="%s%s%s%s%d", "\r", "Ramp Up Time(s):" ("input 2"), w2301, w2301, w2300) -> (resulting string=w2299:string)  [unwired: 2 in, 1 out]
            }
            frame #58 {
              w2306 = "\t"
              n2063 = local read "R Single RF Step1 Coating Power Active"() -> (w2308:bool)
              n2064 = case shown="False" w2308 {
                tunnel: ["Deactive" ("input 4") "Active" ("input 4")] -> w2307
                frame #0 {
                }
                frame #1 {
                }
              }
              n2065 = Format Into String(format string="%s%s%s%s%s%s", "\r", "Region 1:" ("input 2"), w2306, w2306, w2306, w2307) -> (resulting string=w2305:string)  [unwired: 2 in, 1 out]
            }
            frame #59 {
              w2319 = "\t"
              n2066 = local read "R Single RF  Step1 Coating Power"() -> (w2315:dbl)
              n2067 = Format Into String(format string="%s%s%s%s%s%d", "\r", "Power(W):" ("input 2"), w2319, w2319, w2319, w2315) -> (resulting string=w2314:string)  [unwired: 2 in, 1 out]
            }
            frame #60 {
              w2322 = "\t"
              n2068 = local read "R Single RF Interval length"() -> (w2321:dbl)
              n2069 = Format Into String(format string="%s%s%s%s%d", "\r", "Interval Length(m):" ("input 2"), w2322, w2322, w2321) -> (resulting string=w2320:string)  [unwired: 2 in, 1 out]
            }
            frame #61 {
              w2327 = "\t"
              n2070 = local read "R Single RF Step2 Coating Power Active"() -> (w2329:bool)
              n2071 = case shown="False" w2329 {
                tunnel: ["Deactive" ("input 4") "Active" ("input 4")] -> w2328
                frame #0 {
                }
                frame #1 {
                }
              }
              n2072 = Format Into String(format string="%s%s%s%s%s%s", "\r", "Region 2:" ("input 2"), w2327, w2327, w2327, w2328) -> (resulting string=w2326:string)  [unwired: 2 in, 1 out]
            }
            frame #62 {
              w2340 = "\t"
              n2073 = local read "R Single RF Step2 Coating Power"() -> (w2335:dbl)
              n2074 = Format Into String(format string="%s%s%s%s%s%d", "\r", "Power(W):" ("input 2"), w2340, w2340, w2340, w2335) -> (resulting string=w2336:string)  [unwired: 2 in, 1 out]
            }
            frame #63 {
              w2343 = "\t"
              n2075 = local read "R Single RF Interval length2"() -> (w2342:dbl)
              n2076 = Format Into String(format string="%s%s%s%s%d", "\r", "Interval Length(m):" ("input 2"), w2343, w2343, w2342) -> (resulting string=w2341:string)  [unwired: 2 in, 1 out]
            }
            frame #64 {
              w2348 = "\t"
              n2077 = local read "R Single RF Step3 Coating Power Active"() -> (w2350:bool)
              n2078 = case shown="False" w2350 {
                tunnel: ["Deactive" ("input 4") "Active" ("input 4")] -> w2349
                frame #0 {
                }
                frame #1 {
                }
              }
              n2079 = Format Into String(format string="%s%s%s%s%s%s", "\r", "Region 3:" ("input 2"), w2348, w2348, w2348, w2349) -> (resulting string=w2347:string)  [unwired: 2 in, 1 out]
            }
            frame #65 {
              w2361 = "\t"
              n2080 = local read "R Single RF Step3 Coating Power"() -> (w2356:dbl)
              n2081 = Format Into String(format string="%s%s%s%s%s%d", "\r", "Power(W):" ("input 2"), w2361, w2361, w2361, w2356) -> (resulting string=w2357:string)  [unwired: 2 in, 1 out]
            }
            frame #66 {
              w2364 = "\t"
              n2082 = local read "R Single RF Interval length3"() -> (w2363:dbl)
              n2083 = Format Into String(format string="%s%s%s%s%d", "\r", "Interval Length(m):" ("input 2"), w2364, w2364, w2363) -> (resulting string=w2362:string)  [unwired: 2 in, 1 out]
            }
            frame #67 {
              w2369 = "\t"
              n2084 = local read "R Single RF Step4 Coating Power Active"() -> (w2371:bool)
              n2085 = case shown="False" w2371 {
                tunnel: ["Deactive" ("input 4") "Active" ("input 4")] -> w2370
                frame #0 {
                }
                frame #1 {
                }
              }
              n2086 = Format Into String(format string="%s%s%s%s%s%s", "\r", "Region 4:" ("input 2"), w2369, w2369, w2369, w2370) -> (resulting string=w2368:string)  [unwired: 2 in, 1 out]
            }
            frame #68 {
              w2382 = "\t"
              n2087 = local read "R Single RF Step4 Coating Power"() -> (w2377:dbl)
              n2088 = Format Into String(format string="%s%s%s%s%s%d", "\r", "Power(W):" ("input 2"), w2382, w2382, w2382, w2377) -> (resulting string=w2378:string)  [unwired: 2 in, 1 out]
            }
            frame #69 {
              w2385 = "\t"
              n2089 = local read "R Single RF Interval length4"() -> (w2384:dbl)
              n2090 = Format Into String(format string="%s%s%s%s%d", "\r", "Interval Length(m):" ("input 2"), w2385, w2385, w2384) -> (resulting string=w2383:string)  [unwired: 2 in, 1 out]
            }
            frame #70 {
              w2391 = "\t"
              n2091 = local read "R Single RF Step5 Coating Power Active"() -> (w2392:bool)
              n2092 = case shown="False" w2392 {
                tunnel: ["Deactive" ("input 4") "Active" ("input 4")] -> w2390
                frame #0 {
                }
                frame #1 {
                }
              }
              n2093 = Format Into String(format string="%s%s%s%s%s%s", "\r", "Region 5:" ("input 2"), w2391, w2391, w2391, w2390) -> (resulting string=w2389:string)  [unwired: 2 in, 1 out]
            }
            frame #71 {
              w2403 = "\t"
              n2094 = local read "R Single RF Step5 Coating Power"() -> (w2398:dbl)
              n2095 = Format Into String(format string="%s%s%s%s%s%d", "\r", "Power(W):" ("input 2"), w2403, w2403, w2403, w2398) -> (resulting string=w2399:string)  [unwired: 2 in, 1 out]
            }
            frame #72 {
              w2406 = "\t"
              n2096 = local read "R Single RF Interval length5"() -> (w2405:dbl)
              n2097 = Format Into String(format string="%s%s%s%s%d", "\r", "Interval Length(m):" ("input 2"), w2406, w2406, w2405) -> (resulting string=w2404:string)  [unwired: 2 in, 1 out]
            }
            frame #73 {
              w2412 = "\t"
              n2098 = local read "R Single RF Step6 Coating Power Active"() -> (w2413:bool)
              n2099 = case shown="False" w2413 {
                tunnel: ["Deactive" ("input 4") "Active" ("input 4")] -> w2411
                frame #0 {
                }
                frame #1 {
                }
              }
              n2100 = Format Into String(format string="%s%s%s%s%s%s", "\r", "Region 6:" ("input 2"), w2412, w2412, w2412, w2411) -> (resulting string=w2410:string)  [unwired: 2 in, 1 out]
            }
            frame #74 {
              w2424 = "\t"
              n2101 = local read "R Single RF Step6 Coating Power"() -> (w2419:dbl)
              n2102 = Format Into String(format string="%s%s%s%s%s%d", "\r", "Power(W):" ("input 2"), w2424, w2424, w2424, w2419) -> (resulting string=w2420:string)  [unwired: 2 in, 1 out]
            }
            frame #75 {
              w2427 = "\t"
              n2103 = local read "R Single RF Interval length6"() -> (w2426:dbl)
              n2104 = Format Into String(format string="%s%s%s%s%d", "\r", "Interval Length(m):" ("input 2"), w2427, w2427, w2426) -> (resulting string=w2425:string)  [unwired: 2 in, 1 out]
            }
            frame #76 {
              w2433 = "\t"
              n2105 = local read "R Single RF Step7 Coating Power Active"() -> (w2434:bool)
              n2106 = case shown="False" w2434 {
                tunnel: ["Deactive" ("input 4") "Active" ("input 4")] -> w2432
                frame #0 {
                }
                frame #1 {
                }
              }
              n2107 = Format Into String(format string="%s%s%s%s%s%s", "\r", "Region 7:" ("input 2"), w2433, w2433, w2433, w2432) -> (resulting string=w2431:string)  [unwired: 2 in, 1 out]
            }
            frame #77 {
              w2445 = "\t"
              n2108 = local read "R Single RF Step7 Coating Power"() -> (w2440:dbl)
              n2109 = Format Into String(format string="%s%s%s%s%s%d", "\r", "Power(W):" ("input 2"), w2445, w2445, w2445, w2440) -> (resulting string=w2441:string)  [unwired: 2 in, 1 out]
            }
            frame #78 {
              w2448 = "\t"
              n2110 = local read "R Single RF Interval length7"() -> (w2447:dbl)
              n2111 = Format Into String(format string="%s%s%s%s%d", "\r", "Interval Length(m):" ("input 2"), w2448, w2448, w2447) -> (resulting string=w2446:string)  [unwired: 2 in, 1 out]
            }
            frame #79 {
              w2454 = "\t"
              n2112 = local read "R Single RF Step8 Coating Power Active"() -> (w2455:bool)
              n2113 = case shown="False" w2455 {
                tunnel: ["Deactive" ("input 4") "Active" ("input 4")] -> w2453
                frame #0 {
                }
                frame #1 {
                }
              }
              n2114 = Format Into String(format string="%s%s%s%s%s%s", "\r", "Region 8:" ("input 2"), w2454, w2454, w2454, w2453) -> (resulting string=w2452:string)  [unwired: 2 in, 1 out]
            }
            frame #80 {
              w2466 = "\t"
              n2115 = local read "R Single RF Step8 Coating Power"() -> (w2461:dbl)
              n2116 = Format Into String(format string="%s%s%s%s%s%d", "\r", "Power(W):" ("input 2"), w2466, w2466, w2466, w2461) -> (resulting string=w2462:string)  [unwired: 2 in, 1 out]
            }
            frame #81 {
              w2469 = "\t"
              n2117 = local read "R Single RF Interval length8"() -> (w2468:dbl)
              n2118 = Format Into String(format string="%s%s%s%s%d", "\r", "Interval Length(m):" ("input 2"), w2469, w2469, w2468) -> (resulting string=w2467:string)  [unwired: 2 in, 1 out]
            }
            frame #82 {
              w2475 = "\t"
              n2119 = local read "R Single RF Step9 Coating Power Active"() -> (w2476:bool)
              n2120 = case shown="False" w2476 {
                tunnel: ["Deactive" ("input 4") "Active" ("input 4")] -> w2474
                frame #0 {
                }
                frame #1 {
                }
              }
              n2121 = Format Into String(format string="%s%s%s%s%s%s", "\r", "Region 9:" ("input 2"), w2475, w2475, w2475, w2474) -> (resulting string=w2473:string)  [unwired: 2 in, 1 out]
            }
            frame #83 {
              w2487 = "\t"
              n2122 = local read "R Single RF Step9 Coating Power"() -> (w2482:dbl)
              n2123 = Format Into String(format string="%s%s%s%s%s%d", "\r", "Power(W):" ("input 2"), w2487, w2487, w2487, w2482) -> (resulting string=w2483:string)  [unwired: 2 in, 1 out]
            }
            frame #84 {
              w2490 = "\t"
              n2124 = local read "R Single RF Interval length9"() -> (w2489:dbl)
              n2125 = Format Into String(format string="%s%s%s%s%d", "\r", "Interval Length(m):" ("input 2"), w2490, w2490, w2489) -> (resulting string=w2488:string)  [unwired: 2 in, 1 out]
            }
            frame #85 {
              w2496 = "\t"
              n2126 = local read "R Single RF Step10 Coating Power Active"() -> (w2497:bool)
              n2127 = case shown="False" w2497 {
                tunnel: ["Deactive" ("input 4") "Active" ("input 4")] -> w2495
                frame #0 {
                }
                frame #1 {
                }
              }
              n2128 = Format Into String(format string="%s%s%s%s%s%s", "\r", "Region 10:" ("input 2"), w2496, w2496, w2496, w2495) -> (resulting string=w2494:string)  [unwired: 2 in, 1 out]
            }
            frame #86 {
              w2508 = "\t"
              n2129 = local read "R Single RF Step10 Coating Power"() -> (w2503:dbl)
              n2130 = Format Into String(format string="%s%s%s%s%s%d", "\r", "Power(W):" ("input 2"), w2508, w2508, w2508, w2503) -> (resulting string=w2504:string)  [unwired: 2 in, 1 out]
            }
            frame #87 {
              w2511 = "\t"
              n2131 = local read "R Single RF Interval length10"() -> (w2510:dbl)
              n2132 = Format Into String(format string="%s%s%s%s%d", "\r", "Interval Length(m):" ("input 2"), w2511, w2511, w2510) -> (resulting string=w2509:string)  [unwired: 2 in, 1 out]
            }
            frame #88 {
              w2518 = "\t"
              n2133 = local read "R Single RF Ramp down"() -> (w2517:bool)
              n2134 = case shown="False" w2517 {
                tunnel: ["Deactive" ("input 4") "Active" ("input 4")] -> w2516
                frame #0 {
                }
                frame #1 {
                }
              }
              n2135 = Format Into String(format string="%s%s%s%s%s", "\r", "Ramp Down Time(s):" ("input 2"), w2518, w2518, w2516) -> (resulting string=w2515:string)  [unwired: 2 in, 1 out]
            }
            frame #89 {
              w2526 = "\r"
              w2527 = "\t"
              n2136 = local read "R Single RF Ramp down Time"() -> (w2525:dbl)
              n2137 = Format Into String(format string="%s%s%s%s%d%s%s", "\r", "Ramp Down Time(s):" ("input 2"), w2527, w2527, w2525, w2526, w2526) -> (resulting string=w2524:string)  [unwired: 2 in, 1 out]
            }
            frame #90 {
              w2532 = "\r"
              n2138 = Format Into String(format string="%s%s%s", "Multilayer Recipe Parameters" ("input 1"), w2532, w2532) -> (resulting string=w2531:string)  [unwired: 2 in, 1 out]
            }
            frame #91 {
              n2139 = Format Into String(format string="%s%s", "DC Parameters" ("input 1"), "\r") -> (resulting string=w2535:string)  [unwired: 2 in, 1 out]
            }
            frame #92 {
              w2541 = "\t"
              n2140 = local read "R Cmb Ch2 Target material"() -> (w2540:string)
              n2141 = Format Into String(format string="%s%s%s%s%s", "\r", "Target Material:" ("input 2"), w2541, w2541, w2540) -> (resulting string=w2539:string)  [unwired: 2 in, 1 out]
            }
            frame #93 {
              w2547 = "\t"
              n2142 = local read "R_Cmb_Ch2_Web_speed"() -> (w2546:dbl)
              n2143 = Format Into String(format string="%s%s%s%s%d", "\r", "Web Speed(cm/sec):" ("input 2"), w2547, w2547, w2546) -> (resulting string=w2545:string)  [unwired: 2 in, 1 out]
            }
            frame #94 {
              w2553 = "\t"
              n2144 = local read "R Cmb Ch3 Target material"() -> (w2552:string)
              n2145 = Format Into String(format string="%s%s%s%s%s", "\r", "Target Material:" ("input 2"), w2553, w2553, w2552) -> (resulting string=w2551:string)  [unwired: 2 in, 1 out]
            }
            frame #95 {
              w2559 = "\t"
              n2146 = local read "R_Cmb_Ch3_Web_speed"() -> (w2558:dbl)
              n2147 = Format Into String(format string="%s%s%s%s%d", "\r", "Web Speed(cm/sec):" ("input 2"), w2559, w2559, w2558) -> (resulting string=w2557:string)  [unwired: 2 in, 1 out]
            }
            frame #96 {
              w2566 = "\t"
              n2148 = local read "R Cmb Step1 Coating Power Active"() -> (w2564:bool)
              n2149 = case shown="False" w2564 {
                tunnel: ["Deactive" ("input 4") "Active" ("input 4")] -> w2565
                frame #0 {
                }
                frame #1 {
                }
              }
              n2150 = Format Into String(format string="%s%s%s%s%s%s", "\r", "Region 1:" ("input 2"), w2566, w2566, w2566, w2565) -> (resulting string=w2563:string)  [unwired: 2 in, 1 out]
            }
            frame #97 {
              w2577 = "\t"
              n2151 = local read "R Cmb Ch2 Step1 Coating Power"() -> (w2573:dbl)
              n2152 = Format Into String(format string="%s%s%s%s%s%d", "\r", "CH2-Power(W):" ("input 2"), w2577, w2577, w2577, w2573) -> (resulting string=w2572:string)  [unwired: 2 in, 1 out]
            }
            frame #98 {
              w2580 = "\t"
              n2153 = local read "R Cmb Ch3 Step1 Coating Power"() -> (w2579:dbl)
              n2154 = Format Into String(format string="%s%s%s%s%s%d", "\r", "CH3-Power(W):" ("input 2"), w2580, w2580, w2580, w2579) -> (resulting string=w2578:string)  [unwired: 2 in, 1 out]
            }
            frame #99 {
              w2586 = "\t"
              n2155 = local read "R Cmb Interval length 1"() -> (w2585:dbl)
              n2156 = Format Into String(format string="%s%s%s%s%d", "\r", "Interval Length(m):" ("input 2"), w2586, w2586, w2585) -> (resulting string=w2584:string)  [unwired: 2 in, 1 out]
            }
            frame #100 {
              w2592 = "\t"
              n2157 = local read "R Cmb Step2 Coating Power Active"() -> (w2590:bool)
              n2158 = case shown="True" w2590 {
                tunnel: ["Deactive" ("input 4") "Active" ("input 4")] -> w2593
                frame #0 {
                }
                frame #1 {
                }
              }
              n2159 = Format Into String(format string="%s%s%s%s%s%s", "\r", "Region 2:" ("input 2"), w2592, w2592, w2592, w2593) -> (resulting string=w2591:string)  [unwired: 2 in, 1 out]
            }
            frame #101 {
              w2604 = "\t"
              n2160 = local read "R Cmb Ch2 Step2 Coating Power"() -> (w2599:dbl)
              n2161 = Format Into String(format string="%s%s%s%s%s%d", "\r", "CH2-Power(W):" ("input 2"), w2604, w2604, w2604, w2599) -> (resulting string=w2600:string)  [unwired: 2 in, 1 out]
            }
            frame #102 {
              w2610 = "\t"
              n2162 = local read "R Cmb Ch3 Step2 Coating Power"() -> (w2605:dbl)
              n2163 = Format Into String(format string="%s%s%s%s%s%d", "\r", "CH3-Power(W):" ("input 2"), w2610, w2610, w2610, w2605) -> (resulting string=w2607:string)  [unwired: 2 in, 1 out]
            }
            frame #103 {
              w2613 = "\t"
              n2164 = local read "R Cmb Interval length 2"() -> (w2612:dbl)
              n2165 = Format Into String(format string="%s%s%s%s%d", "\r", "Interval Length(m):" ("input 2"), w2613, w2613, w2612) -> (resulting string=w2611:string)  [unwired: 2 in, 1 out]
            }
            frame #104 {
              w2619 = "\t"
              n2166 = local read "R Cmb Step3 Coating Power Active"() -> (w2618:bool)
              n2167 = case shown="False" w2618 {
                tunnel: ["Deactive" ("input 4") "Active" ("input 4")] -> w2620
                frame #0 {
                }
                frame #1 {
                }
              }
              n2168 = Format Into String(format string="%s%s%s%s%s%s", "\r", "Region 3:" ("input 2"), w2619, w2619, w2619, w2620) -> (resulting string=w2617:string)  [unwired: 2 in, 1 out]
            }
            frame #105 {
              w2631 = "\t"
              n2169 = local read "R Cmb Ch2 Step3 Coating Power"() -> (w2626:dbl)
              n2170 = Format Into String(format string="%s%s%s%s%s%d", "\r", "CH2-Power(W):" ("input 2"), w2631, w2631, w2631, w2626) -> (resulting string=w2628:string)  [unwired: 2 in, 1 out]
            }
            frame #106 {
              w2637 = "\t"
              n2171 = local read "R Cmb Ch3 Step3 Coating Power"() -> (w2632:dbl)
              n2172 = Format Into String(format string="%s%s%s%s%s%d", "\r", "CH3-Power(W):" ("input 2"), w2637, w2637, w2637, w2632) -> (resulting string=w2634:string)  [unwired: 2 in, 1 out]
            }
            frame #107 {
              w2640 = "\t"
              n2173 = local read "R Cmb Interval length 3"() -> (w2639:dbl)
              n2174 = Format Into String(format string="%s%s%s%s%d", "\r", "Interval Length(m):" ("input 2"), w2640, w2640, w2639) -> (resulting string=w2638:string)  [unwired: 2 in, 1 out]
            }
            frame #108 {
              w2646 = "\t"
              n2175 = local read "R Cmb Step4 Coating Power Active"() -> (w2645:bool)
              n2176 = case shown="False" w2645 {
                tunnel: ["Deactive" ("input 4") "Active" ("input 4")] -> w2647
                frame #0 {
                }
                frame #1 {
                }
              }
              n2177 = Format Into String(format string="%s%s%s%s%s%s", "\r", "Region 4:" ("input 2"), w2646, w2646, w2646, w2647) -> (resulting string=w2644:string)  [unwired: 2 in, 1 out]
            }
            frame #109 {
              w2658 = "\t"
              n2178 = local read "R Cmb Ch2 Step4 Coating Power"() -> (w2654:dbl)
              n2179 = Format Into String(format string="%s%s%s%s%s%d", "\r", "CH2-Power(W):" ("input 2"), w2658, w2658, w2658, w2654) -> (resulting string=w2655:string)  [unwired: 2 in, 1 out]
            }
            frame #110 {
              w2664 = "\t"
              n2180 = local read "R Cmb Ch3 Step4 Coating Power"() -> (w2660:dbl)
              n2181 = Format Into String(format string="%s%s%s%s%s%d", "\r", "CH3-Power(W):" ("input 2"), w2664, w2664, w2664, w2660) -> (resulting string=w2661:string)  [unwired: 2 in, 1 out]
            }
            frame #111 {
              w2667 = "\t"
              n2182 = local read "R Cmb Interval length 4"() -> (w2666:dbl)
              n2183 = Format Into String(format string="%s%s%s%s%d", "\r", "Interval Length(m):" ("input 2"), w2667, w2667, w2666) -> (resulting string=w2665:string)  [unwired: 2 in, 1 out]
            }
            frame #112 {
              w2673 = "\t"
              n2184 = local read "R Cmb Step5 Coating Power Active"() -> (w2672:bool)
              n2185 = case shown="False" w2672 {
                tunnel: ["Deactive" ("input 4") "Active" ("input 4")] -> w2674
                frame #0 {
                }
                frame #1 {
                }
              }
              n2186 = Format Into String(format string="%s%s%s%s%s%s", "\r", "Region 5:" ("input 2"), w2673, w2673, w2673, w2674) -> (resulting string=w2671:string)  [unwired: 2 in, 1 out]
            }
            frame #113 {
              w2685 = "\t"
              n2187 = local read "R Cmb Ch2 Step5 Coating Power"() -> (w2680:dbl)
              n2188 = Format Into String(format string="%s%s%s%s%s%d", "\r", "CH2-Power(W):" ("input 2"), w2685, w2685, w2685, w2680) -> (resulting string=w2682:string)  [unwired: 2 in, 1 out]
            }
            frame #114 {
              w2691 = "\t"
              n2189 = local read "R Cmb Ch3 Step5 Coating Power"() -> (w2686:dbl)
              n2190 = Format Into String(format string="%s%s%s%s%s%d", "\r", "CH3-Power(W):" ("input 2"), w2691, w2691, w2691, w2686) -> (resulting string=w2688:string)  [unwired: 2 in, 1 out]
            }
            frame #115 {
              w2694 = "\t"
              n2191 = local read "R Cmb Interval length 5"() -> (w2693:dbl)
              n2192 = Format Into String(format string="%s%s%s%s%d", "\r", "Interval Length(m):" ("input 2"), w2694, w2694, w2693) -> (resulting string=w2692:string)  [unwired: 2 in, 1 out]
            }
            frame #116 {
              w2700 = "\t"
              n2193 = local read "R Cmb Step6 Coating Power Active"() -> (w2699:bool)
              n2194 = case shown="False" w2699 {
                tunnel: ["Deactive" ("input 4") "Active" ("input 4")] -> w2701
                frame #0 {
                }
                frame #1 {
                }
              }
              n2195 = Format Into String(format string="%s%s%s%s%s%s", "\r", "Region 6:" ("input 2"), w2700, w2700, w2700, w2701) -> (resulting string=w2698:string)  [unwired: 2 in, 1 out]
            }
            frame #117 {
              w2709 = "\t"
              n2196 = local read "R Cmb Ch2 Step6 Coating Power"() -> (w2707:dbl)
              n2197 = Format Into String(format string="%s%s%s%s%s%d", "\r", "CH2-Power(W):" ("input 2"), w2709, w2709, w2709, w2707) -> (resulting string=w2710:string)  [unwired: 2 in, 1 out]
            }
            frame #118 {
              w2718 = "\t"
              n2198 = local read "R Cmb Ch3 Step6 Coating Power"() -> (w2713:dbl)
              n2199 = Format Into String(format string="%s%s%s%s%s%d", "\r", "CH3-Power(W):" ("input 2"), w2718, w2718, w2718, w2713) -> (resulting string=w2715:string)  [unwired: 2 in, 1 out]
            }
            frame #119 {
              w2721 = "\t"
              n2200 = local read "R Cmb Interval length 6"() -> (w2720:dbl)
              n2201 = Format Into String(format string="%s%s%s%s%d", "\r", "Interval Length(m):" ("input 2"), w2721, w2721, w2720) -> (resulting string=w2719:string)  [unwired: 2 in, 1 out]
            }
            frame #120 {
              w2727 = "\t"
              n2202 = local read "R Cmb Step7 Coating Power Active"() -> (w2726:bool)
              n2203 = case shown="False" w2726 {
                tunnel: ["Deactive" ("input 4") "Active" ("input 4")] -> w2728
                frame #0 {
                }
                frame #1 {
                }
              }
              n2204 = Format Into String(format string="%s%s%s%s%s%s", "\r", "Region 7:" ("input 2"), w2727, w2727, w2727, w2728) -> (resulting string=w2725:string)  [unwired: 2 in, 1 out]
            }
            frame #121 {
              w2739 = "\t"
              n2205 = local read "R Cmb Ch2 Step7 Coating Power"() -> (w2735:dbl)
              n2206 = Format Into String(format string="%s%s%s%s%s%d", "\r", "CH2-Power(W):" ("input 2"), w2739, w2739, w2739, w2735) -> (resulting string=w2736:string)  [unwired: 2 in, 1 out]
            }
            frame #122 {
              w2745 = "\t"
              n2207 = local read "R Cmb Ch3 Step7 Coating Power"() -> (w2740:dbl)
              n2208 = Format Into String(format string="%s%s%s%s%s%d", "\r", "CH3-Power(W):" ("input 2"), w2745, w2745, w2745, w2740) -> (resulting string=w2742:string)  [unwired: 2 in, 1 out]
            }
            frame #123 {
              w2748 = "\t"
              n2209 = local read "R Cmb Interval length 7"() -> (w2747:dbl)
              n2210 = Format Into String(format string="%s%s%s%s%d", "\r", "Interval Length(m):" ("input 2"), w2748, w2748, w2747) -> (resulting string=w2746:string)  [unwired: 2 in, 1 out]
            }
            frame #124 {
              w2754 = "\t"
              n2211 = local read "R Cmb Step8 Coating Power Active"() -> (w2753:bool)
              n2212 = case shown="False" w2753 {
                tunnel: ["Deactive" ("input 4") "Active" ("input 4")] -> w2755
                frame #0 {
                }
                frame #1 {
                }
              }
              n2213 = Format Into String(format string="%s%s%s%s%s%s", "\r", "Region 8:" ("input 2"), w2754, w2754, w2754, w2755) -> (resulting string=w2752:string)  [unwired: 2 in, 1 out]
            }
            frame #125 {
              w2766 = "\t"
              n2214 = local read "R Cmb Ch3 Step8 Coating Power"() -> (w2761:dbl)
              n2215 = Format Into String(format string="%s%s%s%s%s%d", "\r", "CH2-Power(W):" ("input 2"), w2766, w2766, w2766, w2761) -> (resulting string=w2763:string)  [unwired: 2 in, 1 out]
            }
            frame #126 {
              w2772 = "\t"
              n2216 = local read "R Cmb Ch3 Step8 Coating Power"() -> (w2768:dbl)
              n2217 = Format Into String(format string="%s%s%s%s%s%d", "\r", "CH3-Power(W):" ("input 2"), w2772, w2772, w2772, w2768) -> (resulting string=w2769:string)  [unwired: 2 in, 1 out]
            }
            frame #127 {
              w2775 = "\t"
              n2218 = local read "R Cmb Interval length 8"() -> (w2774:dbl)
              n2219 = Format Into String(format string="%s%s%s%s%d", "\r", "Interval Length(m):" ("input 2"), w2775, w2775, w2774) -> (resulting string=w2773:string)  [unwired: 2 in, 1 out]
            }
            frame #128 {
              w2781 = "\t"
              n2220 = local read "R Cmb Step9 Coating Power Active"() -> (w2780:bool)
              n2221 = case shown="False" w2780 {
                tunnel: ["Deactive" ("input 4") "Active" ("input 4")] -> w2782
                frame #0 {
                }
                frame #1 {
                }
              }
              n2222 = Format Into String(format string="%s%s%s%s%s%s", "\r", "Region 9:" ("input 2"), w2781, w2781, w2781, w2782) -> (resulting string=w2779:string)  [unwired: 2 in, 1 out]
            }
            frame #129 {
              w2793 = "\t"
              n2223 = local read "R Cmb Ch2 Step9 Coating Power"() -> (w2789:dbl)
              n2224 = Format Into String(format string="%s%s%s%s%s%d", "\r", "CH2-Power(W):" ("input 2"), w2793, w2793, w2793, w2789) -> (resulting string=w2790:string)  [unwired: 2 in, 1 out]
            }
            frame #130 {
              w2799 = "\t"
              n2225 = local read "R Cmb Ch3 Step9 Coating Power"() -> (w2794:dbl)
              n2226 = Format Into String(format string="%s%s%s%s%s%d", "\r", "CH3-Power(W):" ("input 2"), w2799, w2799, w2799, w2794) -> (resulting string=w2796:string)  [unwired: 2 in, 1 out]
            }
            frame #131 {
              w2802 = "\t"
              n2227 = local read "R Cmb Interval length 9"() -> (w2801:dbl)
              n2228 = Format Into String(format string="%s%s%s%s%d", "\r", "Interval Length(m):" ("input 2"), w2802, w2802, w2801) -> (resulting string=w2800:string)  [unwired: 2 in, 1 out]
            }
            frame #132 {
              w2808 = "\t"
              n2229 = local read "R Cmb Step10 Coating Power Active"() -> (w2807:bool)
              n2230 = case shown="False" w2807 {
                tunnel: ["Deactive" ("input 4") "Active" ("input 4")] -> w2809
                frame #0 {
                }
                frame #1 {
                }
              }
              n2231 = Format Into String(format string="%s%s%s%s%s%s", "\r", "Region 10:" ("input 2"), w2808, w2808, w2808, w2809) -> (resulting string=w2806:string)  [unwired: 2 in, 1 out]
            }
            frame #133 {
              w2820 = "\t"
              n2232 = local read "R Cmb Ch2 Step10 Coating Power"() -> (w2815:dbl)
              n2233 = Format Into String(format string="%s%s%s%s%s%d", "\r", "CH2-Power(W):" ("input 2"), w2820, w2820, w2820, w2815) -> (resulting string=w2817:string)  [unwired: 2 in, 1 out]
            }
            frame #134 {
              w2826 = "\t"
              n2234 = local read "R Cmb Ch3 Step10 Coating Power"() -> (w2822:dbl)
              n2235 = Format Into String(format string="%s%s%s%s%s%d", "\r", "CH3-Power(W):" ("input 2"), w2826, w2826, w2826, w2822) -> (resulting string=w2823:string)  [unwired: 2 in, 1 out]
            }
            frame #135 {
              w2830 = "\t"
              n2236 = local read "R Cmb Interval length 10"() -> (w2829:dbl)
              n2237 = Format Into String(format string="%s%s%s%s%d%s", "\r", "Interval Length(m):" ("input 2"), w2830, w2830, w2829, "\r") -> (resulting string=w2828:string)  [unwired: 2 in, 1 out]
            }
            frame #136 {
              w2837 = "\t"
              n2238 = local read "R_First_stop_selection"() -> (w2836:enum32{"Chamber II", "Chamber III"})
              n2239 = case shown="\"Chamber III\"" w2836 {
                tunnel: ["Chamber II" ("string") "Chamber III" ("string")] -> w2834
                frame #0 {
                }
                frame #1 {
                }
              }
              n2240 = Format Into String(format string="%s%s%s%s", "First Stop Selection:" ("input 1"), w2837, w2837, w2834) -> (resulting string=w2835:string)  [unwired: 2 in, 1 out]
            }
            frame #137 {
              w2844 = "\r"
              w2845 = "\t"
              n2241 = local read "R Cmb Number of cycle"() -> (w2843:dbl)
              n2242 = Format Into String(format string="%s%s%s%s%d%s%s", "\r", "Number of cycle:" ("input 2"), w2845, w2845, w2843, w2844, w2844) -> (resulting string=w2842:string)  [unwired: 2 in, 1 out]
            }
            frame #138 {
              w2851 = "\t"
              n2243 = Format Into String(format string="%s%s%s%s", "Pressure Control Parameters" ("input 1"), w2851, w2851, "\r") -> (resulting string=w2849:string)  [unwired: 2 in, 1 out]
            }
            frame #139 {
              w2856 = "\t"
              n2244 = local read "R Argon Flow sccm"() -> (w2855:dbl)
              n2245 = Format Into String(format string="%s%s%s%s%d", "\r", "Argon Flow(sccm) :" ("input 2"), w2856, w2856, w2855) -> (resulting string=w2854:string)  [unwired: 2 in, 1 out]
            }
            frame #140 {
              w2861 = "\r"
              w2863 = "\t"
              n2246 = local read "R Set Pressure mtorr"() -> (w2862:dbl)
              n2247 = Format Into String(format string="%s%s%s%s%.1f%s%s", "\r", "Set Pressure(mTorr):" ("input 2"), w2863, w2863, w2862, w2861, w2861) -> (resulting string=w2860:string)  [unwired: 2 in, 1 out]
            }
            frame #141 {
              w2869 = "\t"
              n2248 = Format Into String(format string="%s%s%s%s", "Thickness Monitor Parameters" ("input 1"), w2869, w2869, "\r") -> (resulting string=w2867:string)  [unwired: 2 in, 1 out]
            }
            frame #142 {
              w2875 = "\t"
              n2249 = local read "Thickness_Monitor_Active"() -> (w2874:bool)
              n2250 = case shown="False" w2874 {
                tunnel: ["Deactive" ("input 4") "Active" ("input 4")] -> w2873
                frame #0 {
                }
                frame #1 {
                }
              }
              n2251 = Format Into String(format string="%s%s%s%s%s", "\r", "Thickness Monitor:" ("input 2"), w2875, w2875, w2873) -> (resulting string=w2872:string)  [unwired: 2 in, 1 out]
            }
            frame #143 {
              n2252 = local read "R Material_density"() -> (w2882:dbl)
              n2253 = Format Into String(format string="%s%s%s%.2f", "\r", "Material Density(g/cm3) :" ("input 2"), "\t", w2882) -> (resulting string=w2881:string)  [unwired: 2 in, 1 out]
            }
            frame #144 {
              w2889 = "\t"
              n2254 = local read "R Z_factor"() -> (w2888:dbl)
              n2255 = Format Into String(format string="%s%s%s%s%s%.2f", "\r", "Z Factor:" ("input 2"), w2889, w2889, w2889, w2888) -> (resulting string=w2887:string)  [unwired: 2 in, 1 out]
            }
            frame #145 {
              w2895 = "\t"
              n2256 = local read "R Toooling_factor"() -> (w2894:dbl)
              n2257 = Format Into String(format string="%s%s%s%s%d", "\r", "Tooling Factor (%):" ("input 2"), w2895, w2895, w2894) -> (resulting string=w2893:string)  [unwired: 2 in, 1 out]
            }
          }
          n2258 = Concatenate Strings(w1895, w1894, w1893, w1892, w1891, w1890, w1889, w1888, w1887, w1886, w1885, w1884, w1883, w1882, w1881, w1880, w1879, w1878, w1877, w1876, w1875, w1874, w1873, w1872, w1871, w1870, w1869, w1868, w1867, w1866, w1865, w1864, w1863, w1862, w1861, w1860, w1859, w1858, w1857, w1856, w1855, w1854, w1853, w1852, w1851, w1850, w1849, w1848, w1847, w1846, w1845, w1844, w1843, w1842, w1841, w1840, w1839, w1838, w1837, w1836, w1835, w1834, w1833, w1832, w1831, w1830, w1829, w1828, w1827, w1826, w1825, w1824, w1823, w1822, w1821, w1820, w1819, w1818, w1817, w1816, w1815, w1814, w1813, w1812, w1811, w1810, w1809, w1808, w1807, w1806, w1805, w1804, w1803, w1802, w1801, w1800, w1799, w1798, w1797, w1796, w1795, w1794, w1793, w1792, w1791, w1790, w1789, w1788, w1787, w1786, w1785, w1784, w1783, w1782, w1781, w1780, w1779, w1778, w1777, w1776, w1775, w1774, w1773, w1772, w1771, w1770, w1769, w1768, w1767, w1766, w1765, w1764, w1763, w1762, w1761, w1760, w1759, w1758, w1757, w1756, w1755, w1754, w1753, w1752, w1751, w1750) -> (w1898:string)
          n2259 = Write to Text File(file (use dialog)=w1897, text=w1898, error in=w1900) -> (refnum out=w1896:refnum<file>, error out=w1901:errorcluster)  [unwired: 1 in, 1 out]
          n2260 = Write to Text File(file (use dialog)=w1909, text=w1898, error in=w1907) -> (refnum out=w1910:refnum<file>, error out=w1911:errorcluster)  [unwired: 1 in, 1 out]
          n2261 = Write to Text File(file (use dialog)=w1904, text=w1898, error in=w1903) -> (refnum out=w1905:refnum<file>, error out=w1906:errorcluster)  [unwired: 1 in, 1 out]
          n2262 = Close File(refnum=w1896, error in=w1901) -> (error out=w1899:errorcluster)  [unwired: 1 out]
          n2263 = Close File(refnum=w1910, error in=w1911) -> (error out=w1908:errorcluster)  [unwired: 1 out]
          n2264 = Close File(refnum=w1905, error in=w1906) -> (error out=w1902:errorcluster)  [unwired: 1 out]
        }
      }
    }
  }
  "error out" <- w1
  n2265 = Not(x=w2) -> (.not. x?=w3:bool)
  n2266 = property class="VI"("Front Panel Window:Open"=w3) -> ()  [unwired: 2 in, 2 out]
